vi "TLB Native Dynamic Events ver 0.27.vi"() -> ()   [LabVIEW 2018]
uses:
  TLB Type Definitions/Intruction Type Definitions.ctl
  TLB Type Definitions/State Type Definitions, for 0.26g versions and later 3.ctl
  <vilib>/Studica/Studica Toolkit/NavX/TypeDefs/Flags/Z900_navX_Flags_OpStatusTypeDef.ctl
  <vilib>/Studica/Studica Toolkit/NavX/TypeDefs/Flags/Z900_navX_Flags_CalibrationStatusTypeDef.ctl
  TLB Type Definitions/Vision cluster.ctl
  TLB Type Definitions/PING CLUSTER.ctl
  TLB Type Definitions/Encoder cluster.ctl
  TLB Type Definitions/Stepper cluster.ctl
  TLB Type Definitions/Yaw Cluster.ctl
  TLB Type Definitions/IR Sensor Type Def.ctl
  TLB Type Definitions/Line Sensor Cluster.ctl
  TLB Type Definitions/Time cluster.ctl
  TLB Type Definitions/Box Colour Detection Cluster (0.26d and above).ctl
  Underlying VI's/FGV's/Box FGV/Box Colour FGV Colours.ctl
  <vilib>/Studica/Studica Toolkit/Background/DIO Channel.ctl
  TLB Type Definitions/Y Stepper cluster.ctl
  TLB Type Definitions/Motor Speed Cluster.ctl
  <vilib>/Studica/Studica Toolkit/Background/PWM Channel.ctl
  Underlying VI's/NavX VI/navX type def.ctl
  <vilib>/Studica/Studica Toolkit/Background/I2C Channel.ctl
  Underlying VI's/I2C Master VI/Arduino_Interfacing.ctl
  Labview Training Phase 2/Enum Controls/States for Action Engine.ctl
  Underlying VI's/Motor Control VI with PID/MOTOR CONTROL WITH PID AE DATA MODE TYPE DEF.ctl
  Underlying VI's/Motor Control VI with PID/MOTOR CONTROL WITH PID AE DIRECTION TYPE DEF.ctl
  Experimental VI's/Archived VI's/MOTOR CONTROL NO PID Type Def.ctl
  <vilib>/myRIO/Common/Instrument Driver Framework/myRIO v1.0/AI/typedefs/AI Channels List.ctl
  <vilib>/myRIO/Common/Instrument Driver Framework/myRIO v1.0/AI/typedefs/AI Channels Enum.ctl
  Underlying VI's/Line Sensor AE/Line Sensor AE Type Def.ctl
  Underlying VI's/I2C Master VI/I2C MASTER Type Def.ctl
  Underlying VI's/Elasped Timer/Elapsed timer control.ctl
  Underlying VI's/IMAQ Create Reference AE/IMAQ Reference AE.ctl
  Underlying VI's/FGV's/Box FGV/Box Colour FGV States.ctl
  Underlying VI's/I2C Master VI/I2C_MASTER_WRITE_NEW Type Def.ctl
  Underlying VI's/FGV's/Servo State FGV/Servo States FGV Enum.ctl
  Underlying VI's/Modified webcam FGV/Webcam AE.ctl
  <vilib>/userdefined/High Color/IMAQdx.ctl
  <vilib>/Studica/Studica Toolkit/NavX/NavX.lvlib
  <vilib>/NI_Real-Time Target Support.lvlib
panel:
  out "Distance to move":dbl
  out "Same colour?":bool
  out "Box Colour Detection":T1
  out "Errors detected":bool
  out "Robot ready":bool
  out "Time cluster":T3
  out "Table IR obstruct":bool
  out "Front IR obstruct":bool
  out "CPU 1 Usage":dbl
  out "CPU 0 Usage":dbl
  out "Line sensors":T4
  out "IR Sensors":T5
  out "NAVX Values":T6
  out "Stepper position values":T7
  out "Encoder values":T8
  out "Ultrasonic sensors":T9
  out "Selected Task":T10=enum."Start Task 9"
  out "Object recognition mode":enum16{"Ball", "Soap", "Gel", "Pipe", "None"}(ring)
  out "Image Processing Error":errorcluster
  out "Object Detection":T11
  out "Status":T14 {"OP Status" items=["INITIALIZING", "SELFTEST_IN_PROGRESS", "ERROR", "IMU_AUTOCAL_IN_PROGRESS", "NORMAL"]; "Calibration Status" items=["IMU_CAL_STATE_MASK"=3, "IMU_CAL_STATE_INPROGRESS"=0, "IMU_CAL_STATE_ACCUMULATE"=1, "IMU_CAL_STATE_COMPLETE"=2]}
  out "General Errors":errorcluster
  in  "Red LED":bool
  out "Front Ultrasonic obstruct":bool
  out "Speed & distance":T15
  out "Task selection":u8
  out "NavX Readings":T16
  out "Arduino Data":T17
  out "TASK ENABLE":bool
  out "Rising Edge":bool
  in  "Green LED":bool
  out "State Logic":T18=enum."Startup"
  out "elements":T10[](array[typedef])
  in  "STOP TASK":bool
  in  "OK Button":bool
  in  "STOP":bool
  out "Queue Errors":errorcluster
  out "Action Queue Items":i32
  out "State Logic Queue Items":i32
  out "Action Queues items":string[](array[string])=["Hardware reset", "Software reset", ""]
  out "Action State":string
  # "VISION"
  # "TLB FRAMEWORK STATUS"
  # "System Health Status Update"
  # "Test Programme written by Calvin Loke    Dated: 28 Aug 2019\nTest Programme revised by Dr Alex See   Dated 30 Aug 2019\n\nRevision date: 20/03/2020\nProgramme version:   TLB Native Dynamic Events ver 0.19a"
  # "0: Task 1\n1: Task 2\n2: Task 3\n3: Task 4\n4: Task 5\n5: Task 6\n6: Task 7\n7: Task 8 Ball\n8: Task 8 Soap\n9: Task 8 Gel\n10: Task 8 Pipe\n11: Task 9 Blue\n12: Task 9 Black\n13: Task 9 Green\n14: Task 9 Red\n15: Task 9 Yellow"
  # "Ball: Right\nSoap: Left\nGel: Reverse\nPipe: Forward"
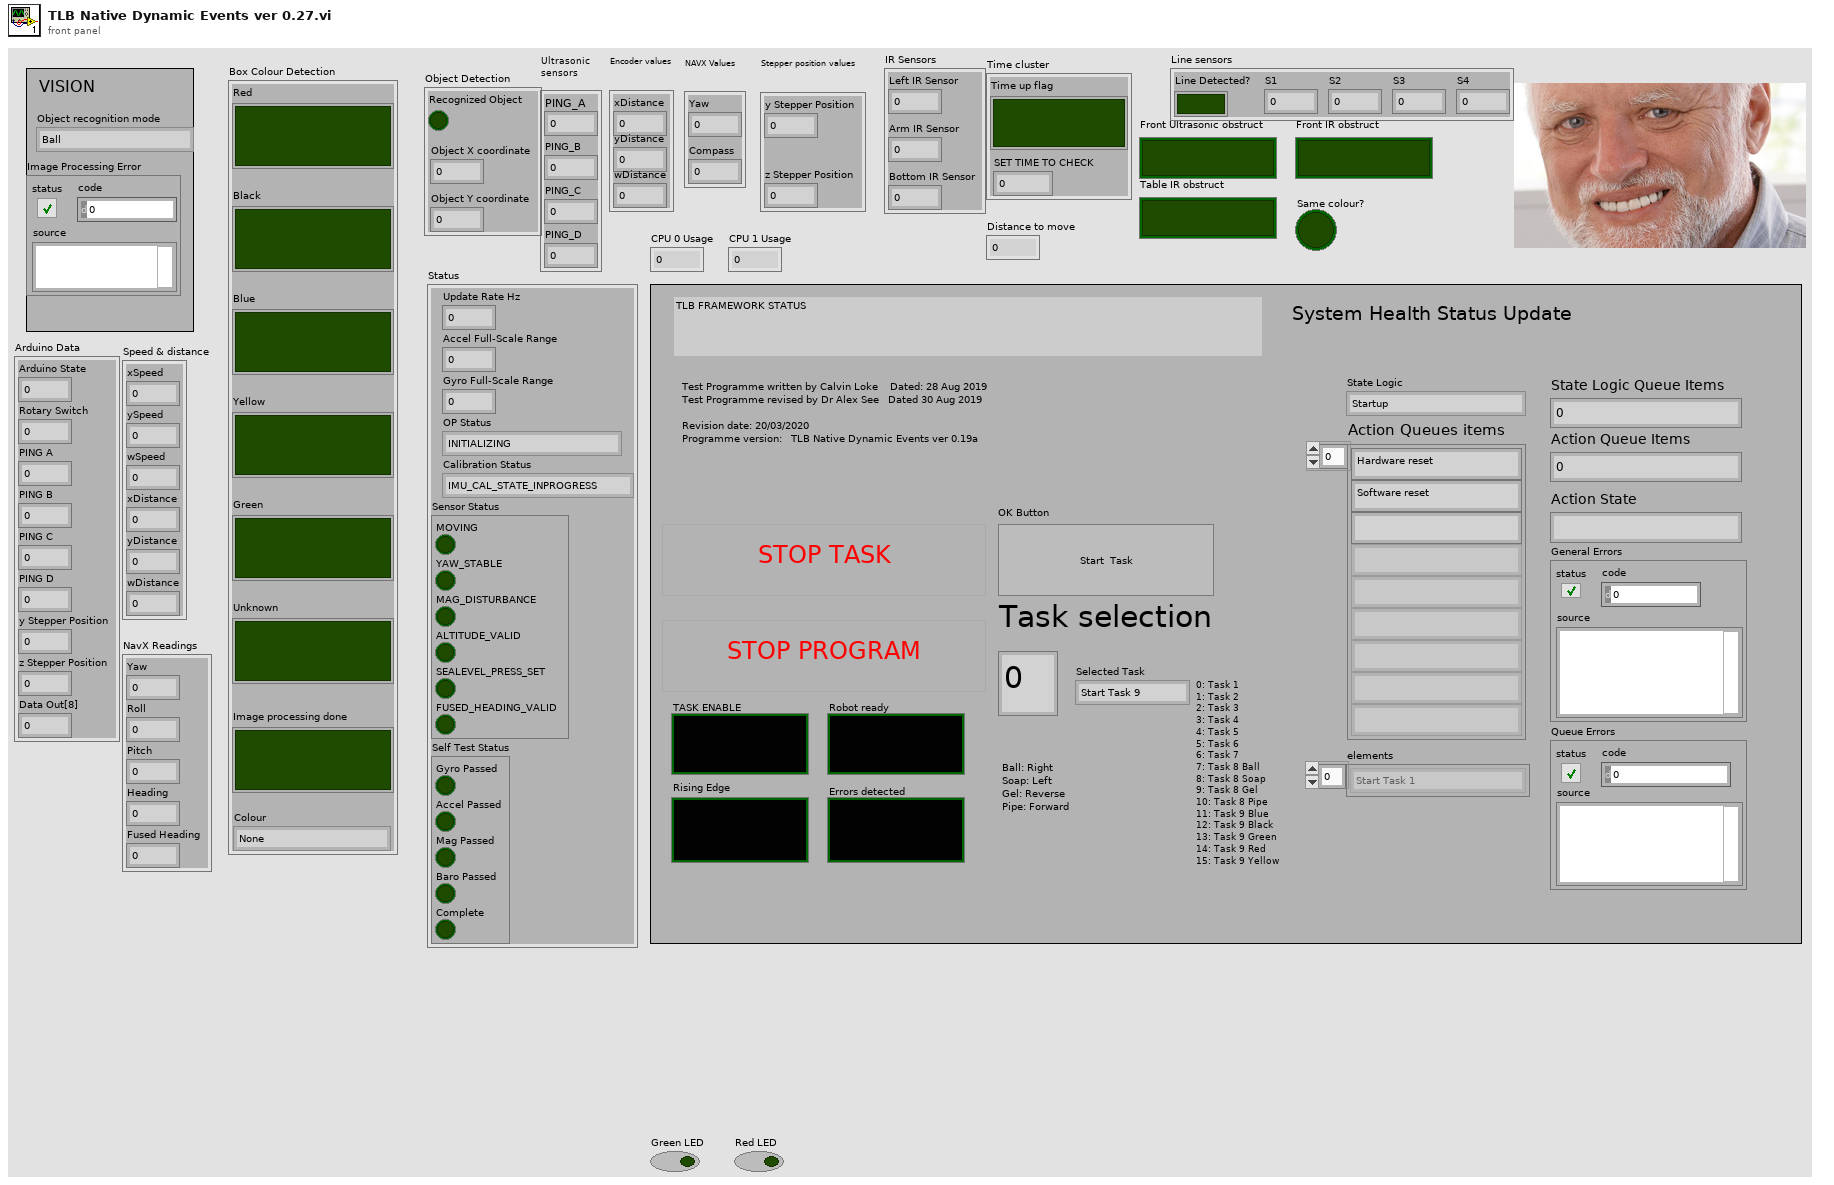
[diagram p1: front panel]
types:
  T1 = typedef "Box Colour Detection Cluster (0.26d and above).ctl" = cluster{"Red":bool, "Black":bool, "Blue":bool, "Yellow":bool, "Green":bool, "Unknown":bool, "Image processing done":bool, "Colour":T2}
  T2 = typedef "Box Colour FGV Colours.ctl" = enum16{"None", "Black", "Blue", "Green", "Red", "Yellow"}
  T3 = typedef "Time cluster.ctl" = cluster{"Time up flag":bool, "SET TIME TO CHECK":dbl}
  T4 = typedef "Line Sensor Cluster.ctl" = cluster{"Line Detected?":bool, "S1":dbl, "S2":dbl, "S3":dbl, "S4":dbl}
  T5 = typedef "IR Sensor Type Def.ctl" = cluster{"Left IR Sensor":dbl, "Arm IR Sensor":dbl, "Bottom IR Sensor":dbl}
  T6 = typedef "Yaw Cluster.ctl" = cluster{"Yaw":dbl, "Compass":dbl}
  T7 = typedef "Stepper cluster.ctl" = cluster{"y Stepper Position":u8, "z Stepper Position":u8}
  T8 = typedef "Encoder cluster.ctl" = cluster{"xDistance":dbl, "yDistance":dbl, "wDistance":dbl}
  T9 = typedef "PING CLUSTER.ctl" = cluster{"PING_A":u8, "PING_B":u8, "PING_C":u8, "PING_D":u8}
  T10 = typedef "Intruction Type Definitions.ctl" = enum16{"None", "Start Task 1", "Start Task 2", "Start Task 3", "Start Task 4", "Start Task 5", "Start Task 6", "Start Task 7", "Start Task 8 - BALL", "Start Task 8 - Gel", "Start Task 8 - Pipe", "Start Task 8 - Soap", "Start Task 9", "Start Task A", "Start Task B", "Exit"}
  T11 = typedef "Vision cluster.ctl" = cluster{"Recognized Object":bool, "Object X coordinate":dbl, "Object Y coordinate":dbl}
  T12 = typedef "NavX.lvlib/Z900_navX_Flags_OpStatusTypeDef.ctl" = u8
  T13 = typedef "NavX.lvlib/Z900_navX_Flags_CalibrationStatusTypeDef.ctl" = u8
  T14 = cluster{"Update Rate Hz":u8, "Accel Full-Scale Range":u8, "Gyro Full-Scale Range":u16, "OP Status":T12, "Calibration Status":T13, "Sensor Status":cluster{"MOVING":bool, "YAW_STABLE":bool, "MAG_DISTURBANCE":bool, "ALTITUDE_VALID":bool, "SEALEVEL_PRESS_SET":bool, "FUSED_HEADING_VALID":bool}, "Self Test Status":cluster{"Gyro Passed":bool, "Accel Passed":bool, "Mag Passed":bool, "Baro Passed":bool, "Complete":bool}}
  T15 = cluster{"xSpeed":dbl, "ySpeed":dbl, "wSpeed":dbl, "xDistance":dbl, "yDistance":dbl, "wDistance":dbl}
  T16 = cluster{"Yaw":dbl, "Roll":dbl, "Pitch":dbl, "Heading":dbl, "Fused Heading":dbl}
  T17 = cluster{"Arduino State":u8, "Rotary Switch":u8, "PING A":u8, "PING B":u8, "PING C":u8, "PING D":u8, "y Stepper Position":u8, "z Stepper Position":u8, "Data Out[8]":u8}
  T18 = typedef "State Type Definitions, for 0.26g versions and later 3.ctl" = enum16{"None", "Startup", "Move to Angle", "True Stop", "Idle", "Shutdown", "Task 1A", "Task 1B", "Task 2:Raise Arm", "Task 2:Sensor Mode", "Task 2:Reverse Mode", "Task 3", "Task 4_A", "Task 4_B", "Task 4_C", "Task 4_D", "Task 5A: RAISING ARM", "Task 5B: STILL WAITING", "Task 5C: GOING DOWN", "Task 5D: GRAB", "Task 5E: GOING UP", "Task 5F: ARM GRAB HEIGHT", "Task 5G: CLOSE CLAW", "Task 5H: RAISE ARM", "Task 6A: RAISE ARM", "Task 6B: CAM BURST", "Task 6C: PROCESS IMAGE", "Task 6D: BALL BUSTER", "Task 6E: STILL WAITING", "Task 6F: CAM BURST 2", "Task 6G: PROCESS IMAGE 2", "Task 6H: SKADI SOAPS", "Task 6I: STILL WAITING 2", "Task 6J: CAM BURST 3", "Task 6K: PROCESS IMAGE 3", "Task 6L: JAM IT IN", "Task 6M: STILL WAITING 3", "Task 6N: CAM BURST 4", "Task 6O: PROCESS IMAGE 4", "Task 6P: PIPE BOMB", "Task 7", "Task 8A: RAISE ARM", "Task 8B: MOVE TO BOX", "Task 8C: CAM BURST", "Task 8D: PROCESS IMAGE", "Task 8E: ROBOT ADJUST", "Task 8F: CAM BURST 2", "Task 8G: PROCESS IMAGE 2", "Task 8H: ARM ADJUST", "Task 8I: ARM GRAB HEIGHT", "Task 8J: CLOSE CLAW", "Task 8K: RAISE MY SWORD", "Task 8I: STILL WAITING", "Task 8L: Return to position", "Task 9A: Raise Arm", "Task 9B: Rotate to Angle", "Task 9C: Detect Box", "Task 9D: MOVE FORWARD", "Task 9E: MOVE LEFT", "Task 9E2: MOVE RIGHT", "Task 9F: SCAN BOX", "Task 9G: MOVE RIGHT", "Task 9H: SCAN BOX 2", "Task 9I: ROTATE 90 CW", "Task 9J: FORWARD", "Task 9K: RAM WALL", "Task 9L: MOVE RIGHT", "Task 9M: SCAN BOX 3", "Task 9N: MOVE RIGHT", "Task 9O: SCAN BOX 4", "Task A1: RAISE ARM", "Task A2: ROTATE TO ANGLE", "Task A3: MOVE TO BL BOX", "Task A4: MOVE FORWARD", "Task A5: ROTATE CW 90"}
  T19 = typedef "PWM Channel.ctl" = enum16{"Not Connected", "A/PWM0", "A/PWM1", "A/PWM2", "A/PWM3", "A/PWM4", "B/PWM0", "B/PWM1", "B/PWM2", "B/PWM3", "B/PWM4", "C/PWM0", "C/PWM1"}
  T20 = typedef "Motor Speed Cluster.ctl" = cluster{"ySpeed":dbl, "xSpeed":dbl, "wSpeed":dbl}
  T21 = typedef "Y Stepper cluster.ctl" = cluster{"yStepper desired":u8}
  T22 = typedef "DIO Channel.ctl" = enum16{"Not Connected", "A/DIO1", "A/DIO2", "A/DIO3", "A/DIO4", "A/DIO5", "A/DIO6", "A/DIO7", "A/DIO13", "B/DIO1", "B/DIO2", "B/DIO3", "B/DIO4", "B/DIO5", "B/DIO6", "B/DIO7", "B/DIO13", "C/DIO0", "C/DIO1", "C/DIO2", "C/DIO3", "C/DIO4", "C/DIO5", "C/DIO6", "C/DIO7"}
  T23 = cluster{"PWM Channel":T19, "FPGA VI Reference Out":refnum<k20>}
  T24 = cluster{"DIO Channel":T22, "FPGA VI Reference Out":refnum<k20>}
  T25 = typedef "States for Action Engine.ctl" = enum16{"Initialize", "Write", "Read"}
  T26 = typedef "NI_Real-Time Target Support.lvlib/RT CPU Load.ctl" = cluster{"Total (%)":dbl, "Time Critical (%)":dbl, "Timed Structures (%)":dbl, "High (%)":dbl, "Above Normal (%)":dbl, "Normal (%)":dbl, "Background (%)":dbl, "Idle (%)":dbl, "ISR (%)":dbl}
  T27 = cluster{"CPU loads[0]":T26, "CPU loads[1]":T26, "CPU loads[2]":T26, "CPU loads[3]":T26, "CPU loads[4]":T26, "CPU loads[5]":T26, "CPU loads[6]":T26, "CPU loads[7]":T26, "CPU loads[8]":T26}
  T28 = typedef "navX type def.ctl" = enum16{"Get i2C reference", "Read Values", "Zero Yaw"}
  T29 = typedef "Arduino_Interfacing.ctl" = enum16{"Initialize", "Write to Arduino", "Read From Arduino"}
  T30 = typedef "I2C Channel.ctl" = enum16{"Not Connected", "A", "B"}
  T31 = cluster{"I2C Ref Out":cluster{"I2C Channel":T30, "FPGA VI Reference Out":refnum<k20>}, "Connected":bool, "Slave Address (7-bit)":u8, "Registry":u8[]}
  T32 = typedef "Box Colour FGV States.ctl" = enum16{"Initialize", "Read", "Write"}
  T33 = typedef "MOTOR CONTROL WITH PID AE DIRECTION TYPE DEF.ctl" = enum16{"y-axis movement", "x-axis movement", "rotation", "stop", "reset encoders"}
  T34 = typedef "MOTOR CONTROL WITH PID AE DATA MODE TYPE DEF.ctl" = enum16{"Init AE", "Write to AE", "Read from AE"}
  T35 = typedef "Line Sensor AE Type Def.ctl" = enum16{"INIT AE", "READ FROM LINE SENSORS"}
  T36 = typedef "IMAQ Reference AE.ctl" = enum16{"Initialize AE", "Get IMAQ Reference", "Dispose Processing Buffer"}
  T37 = typedef "Elapsed timer control.ctl" = enum16{"Start", "Pause", "Initialize"}
  T38 = typedef "I2C_MASTER_WRITE_NEW Type Def.ctl" = enum16{"Ultrasonic sensors", "Stepper origin", "zStepper 13.3k", "zStepper 13k", "zStepper 12k", "zStepper 11k", "zStepper 10k", "zStepper 9k", "zStepper 8k", "zStepper 7k", "zStepper 6k", "zStepper 5k", "zStepper 4k", "zStepper 3k", "zStepper 2k", "zStepper 1k", "zStepper 900", "zStepper 800", "zStepper 700", "zStepper 600", "zStepper 500", "zStepper 400", "zStepper 300", "zStepper 200", "zStepper 100", "zStepper 0", "yStepper control", "Open Claw", "Close Claw", "Soft Reset"}
  T39 = typedef "Servo States FGV Enum.ctl" = enum16{"Open Claw", "Close claw"}
  T40 = typedef "Webcam AE.ctl" = enum16{"Initialize Camera", "Open Camera", "Continuous Acquisition", "Close Camera", "Retrieve Image", "Dispose Camera Image Buffer"}
  T41 = typedef "IMAQdx.ctl" = refnum<k21>
  T42 = typedef "MOTOR CONTROL NO PID Type Def.ctl" = enum16{"Init", "Front Back", "Left Right", "Rotate", "Stop", "Latch"}
  T43 = typedef "AI Channels List.ctl" = T44[]
  T44 = typedef "AI Channels Enum.ctl" = enum16{"Not Connected", "AudioIn/Left", "AudioIn/Right", "C/AI0", "C/AI1", "A/AI0", "A/AI1", "A/AI2", "A/AI3", "A/AI4", "A/AI5", "A/AI6", "A/AI7", "B/AI0", "B/AI1", "B/AI2", "B/AI3", "B/AI4", "B/AI5", "B/AI6", "B/AI7", "AI/AI0", "AI/AI1", "AI/AI2", "AI/AI3", "A/AI0 (DIFF)", "A/AI1 (DIFF)", "A/AI2 (DIFF)", "A/AI3 (DIFF)", "B/AI0 (DIFF)", "B/AI1 (DIFF)", "B/AI2 (DIFF)", "B/AI3 (DIFF)"}
  T45 = cluster{"S1":dbl, "S2":dbl, "S3":dbl, "S4":dbl, "Array[4]":dbl, "Array[5]":dbl, "Array[6]":dbl, "Array[7]":dbl, "Array[8]":dbl}
  T46 = typedef "I2C MASTER Type Def.ctl" = enum16{"Last State", "Mode 0", "Mode 1", "Mode 2", "Mode 3", "Mode 4", "Mode 5", "Mode 6", "Mode 7", "Mode 8", "Mode 9", "Mode 10"}
  T47 = typedef "IMAQ Image.ctl" = refnum<image>
  T48 = cluster{"Number of Matches":i32, "Object detected?":bool}
  T49 = cluster{"Red":bool, "Black":bool, "Blue":bool, "Yellow":bool, "Green":bool, "No recognizable coolour":bool}
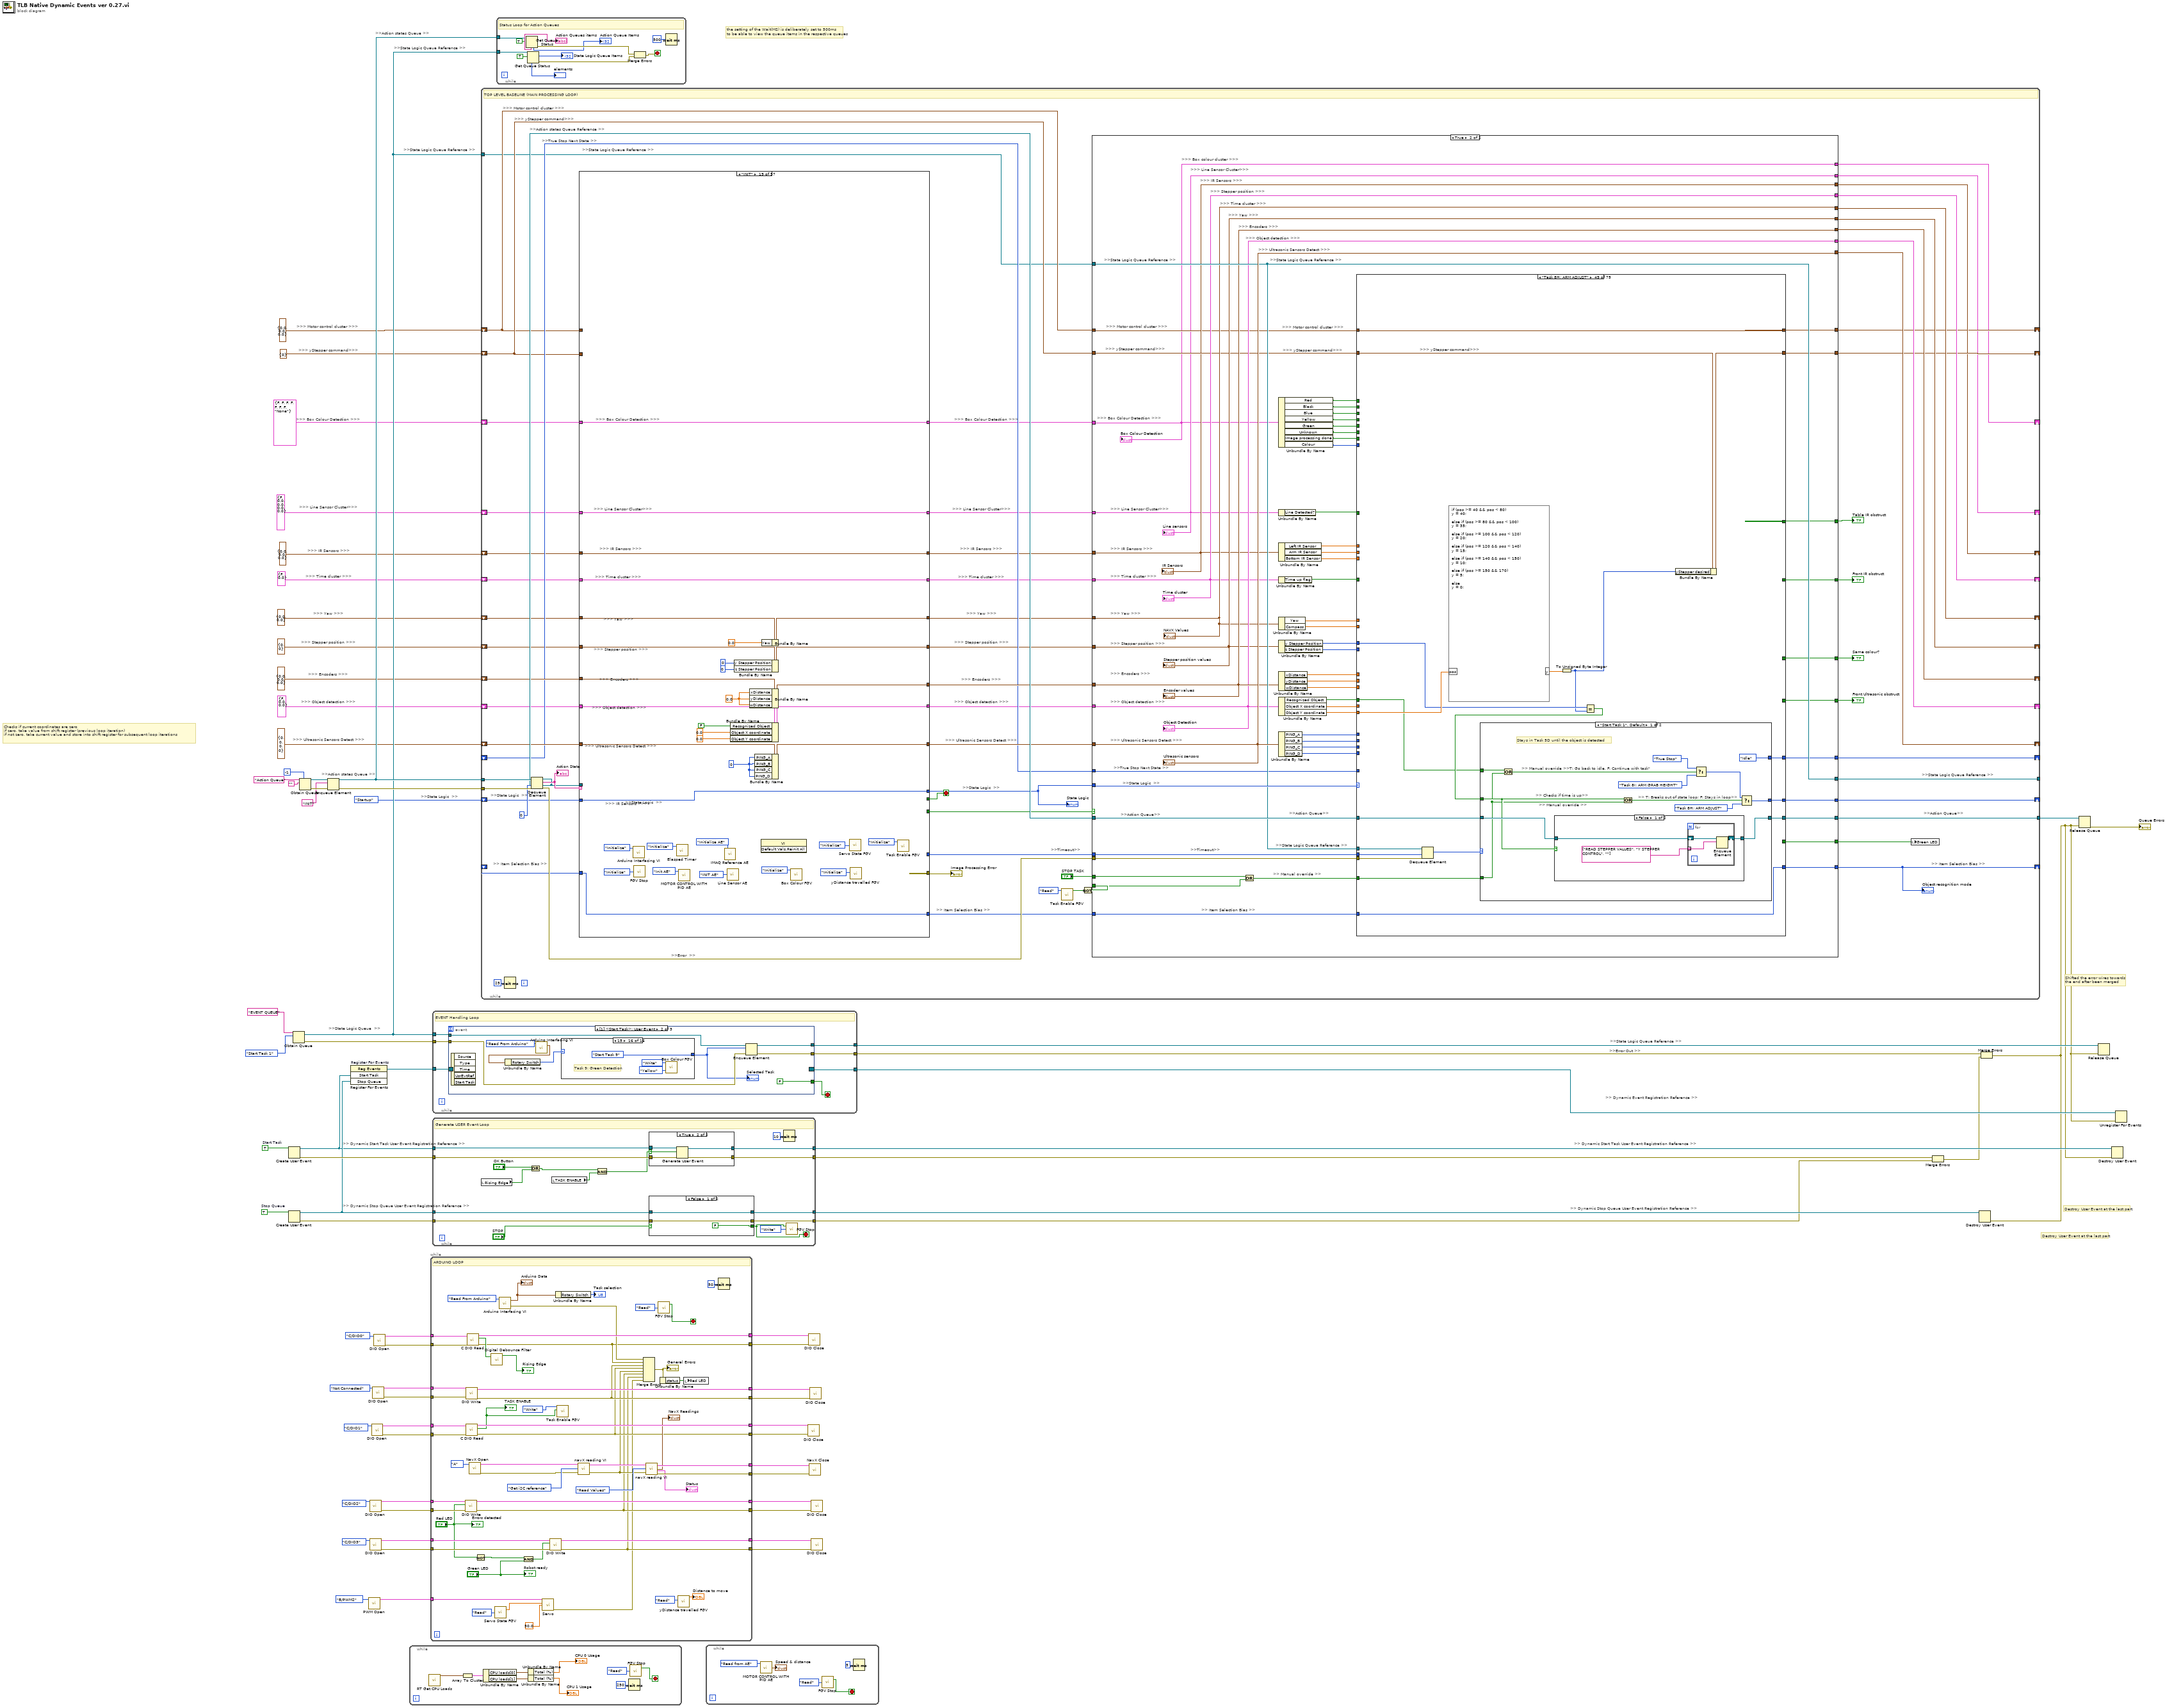
[diagram p0: block diagram]
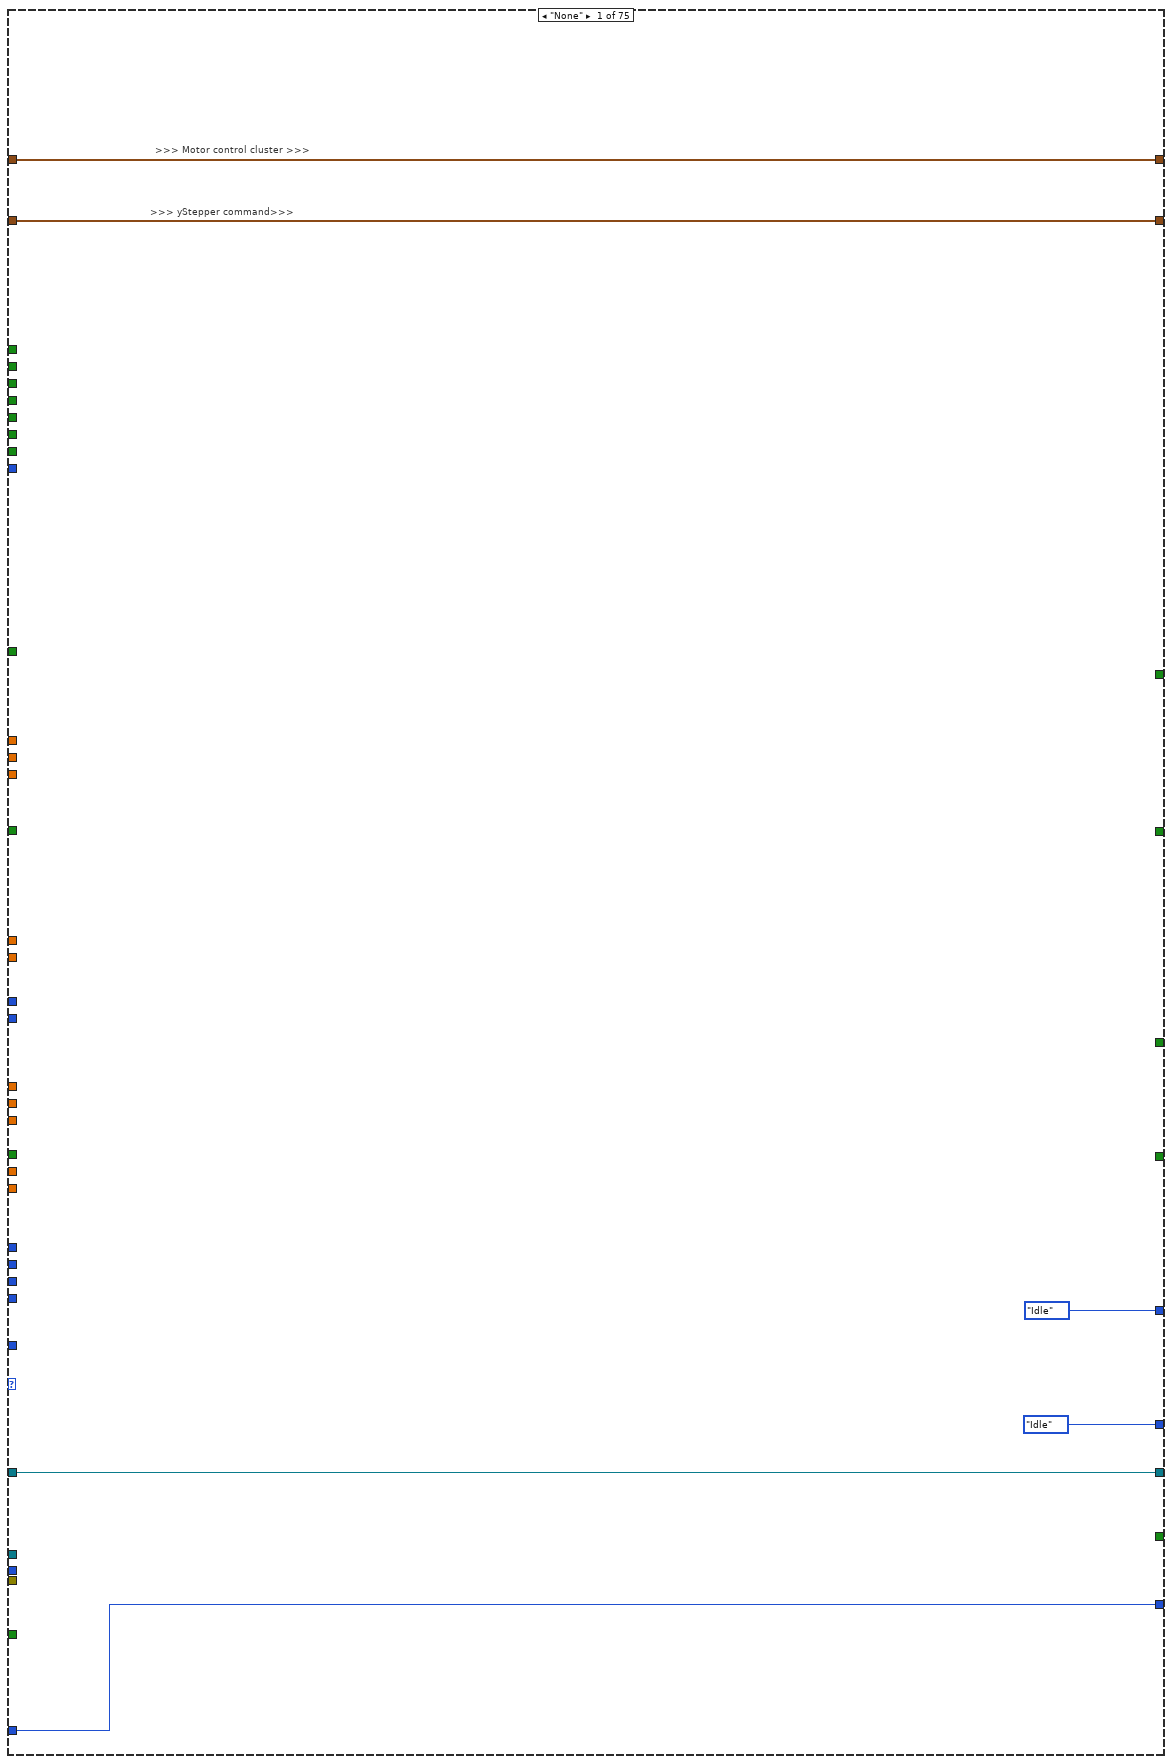
[diagram p3: hidden frame]
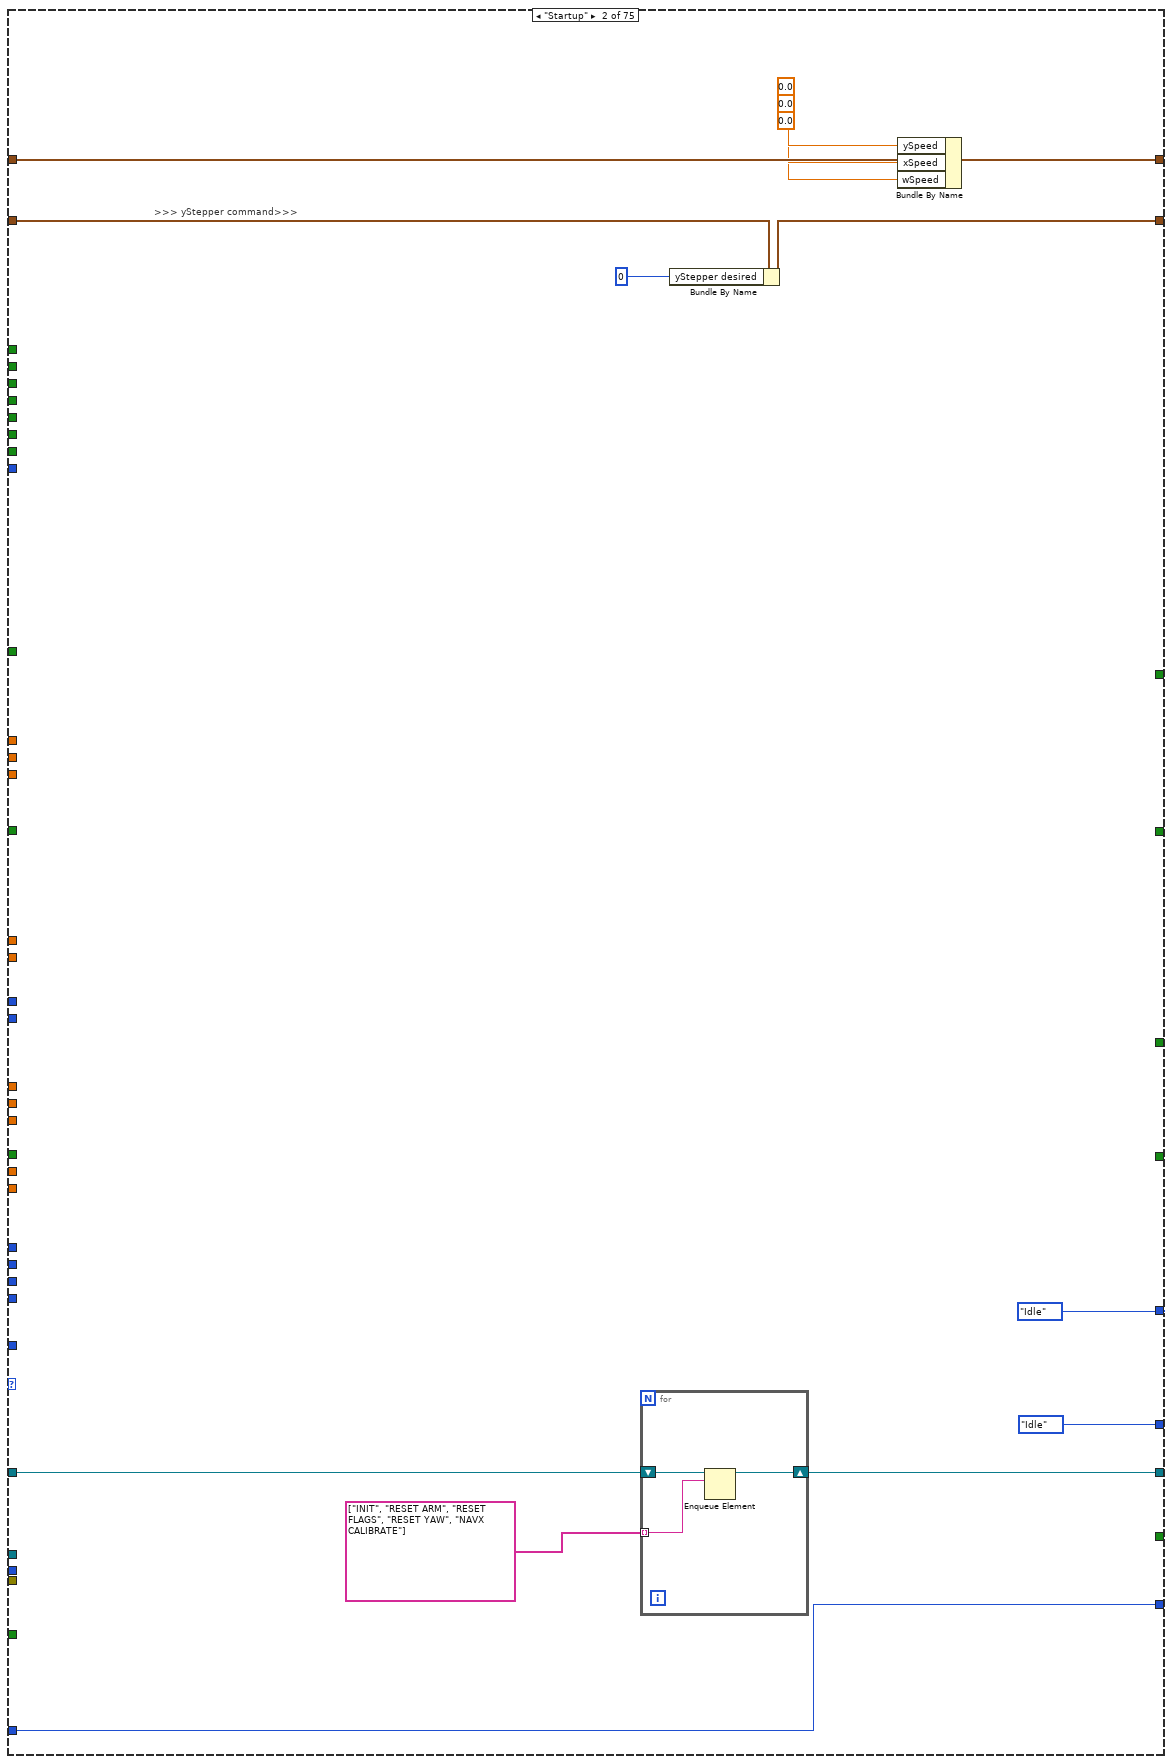
[diagram p4: hidden frame]
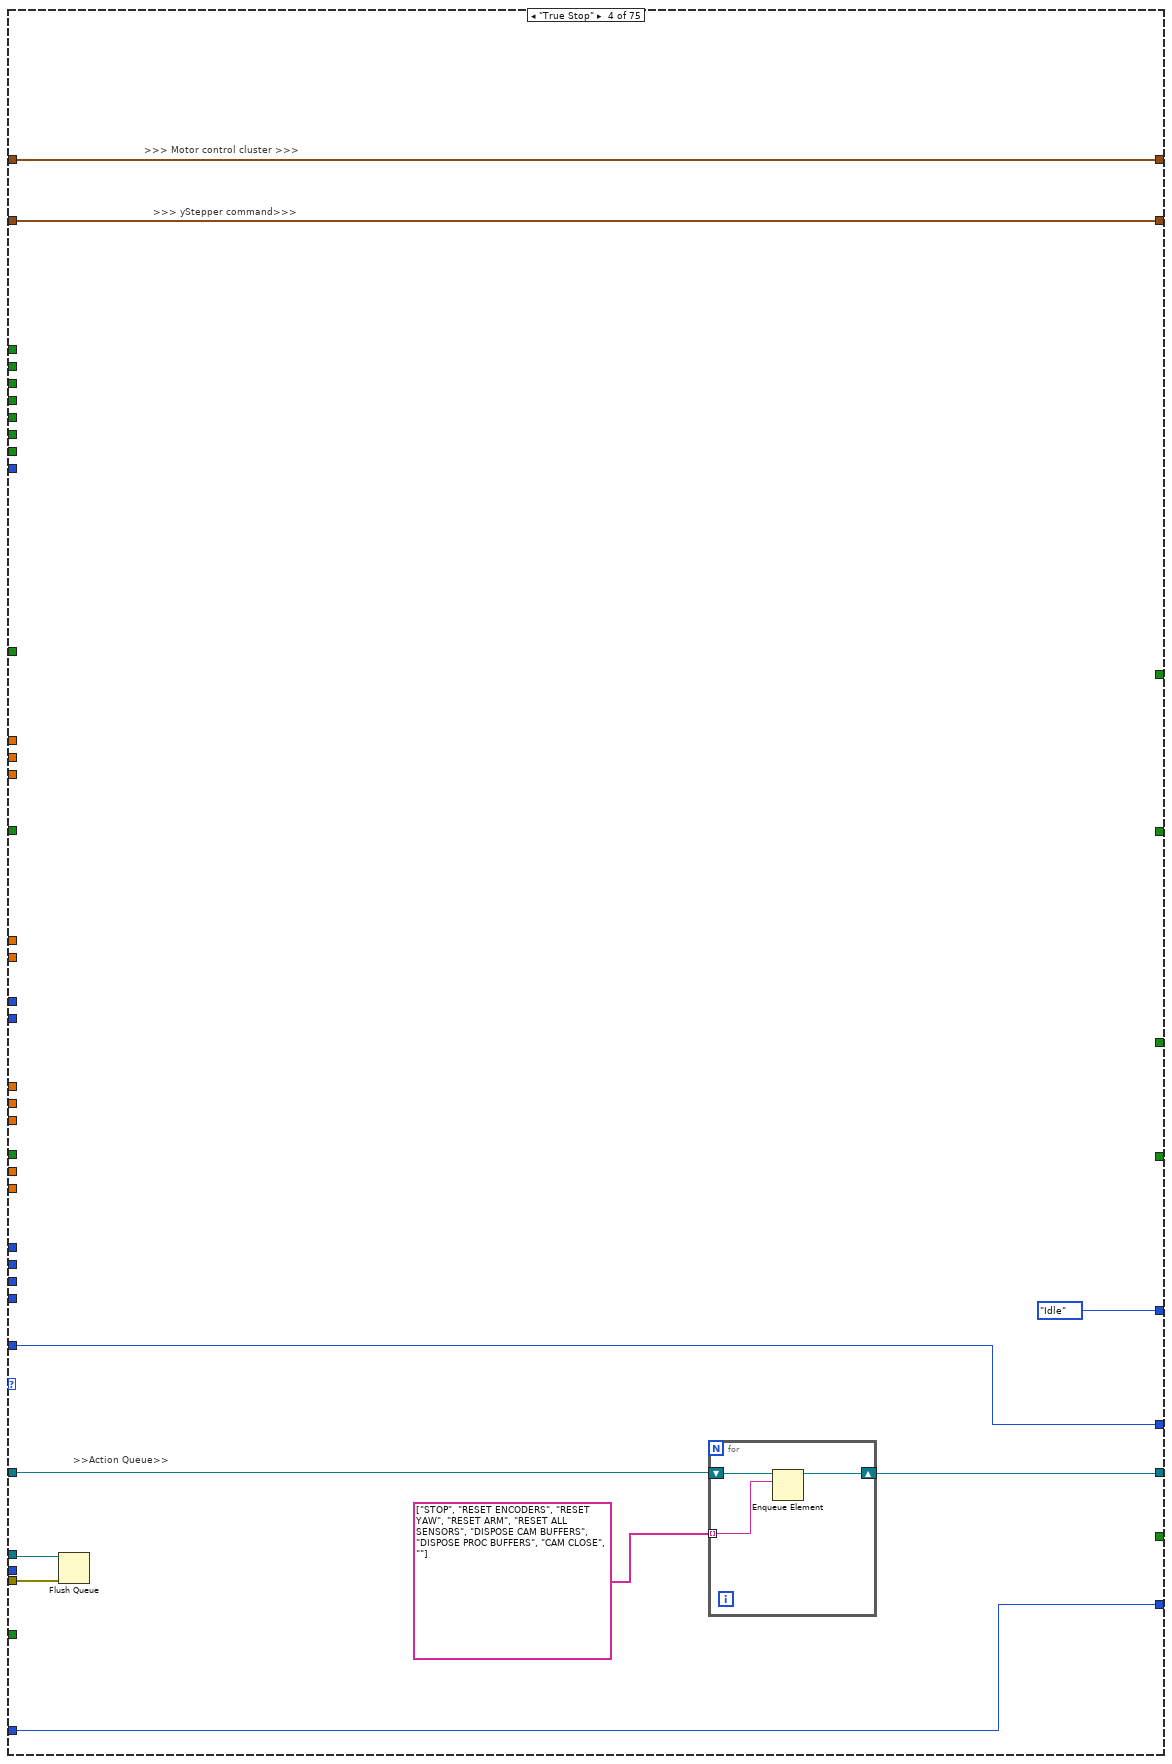
[diagram p6: hidden frame]
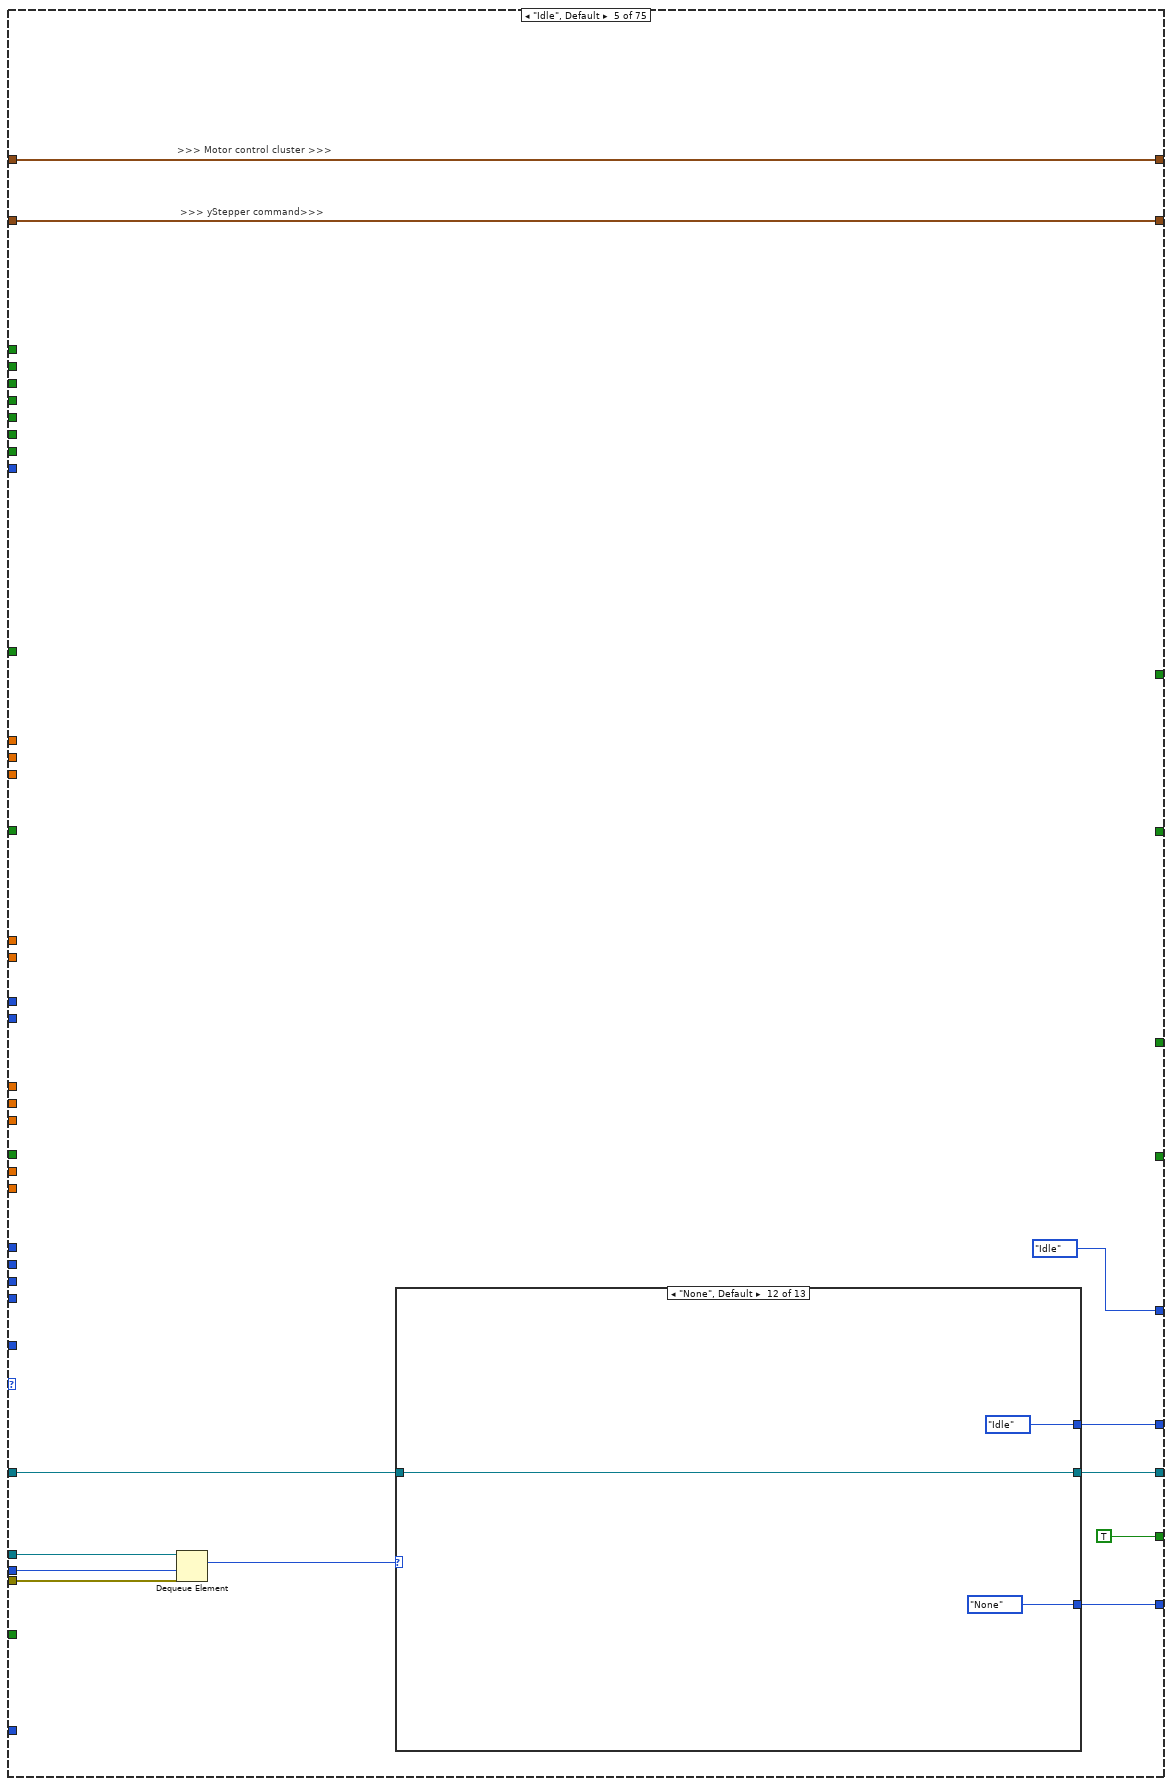
[diagram p7: hidden frame]
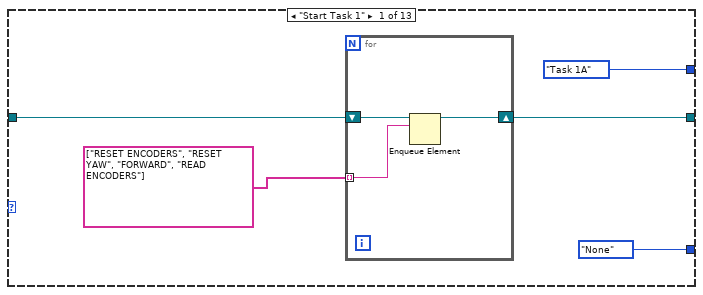
[diagram p8: hidden frame]
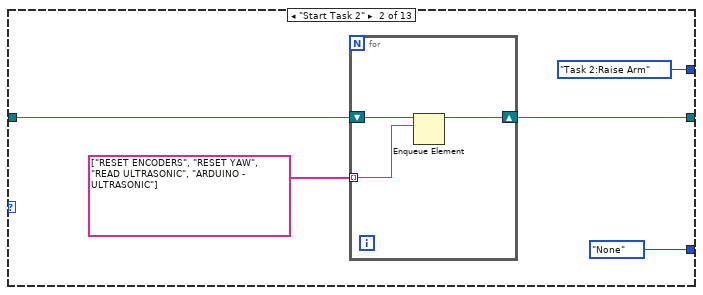
[diagram p9: hidden frame]
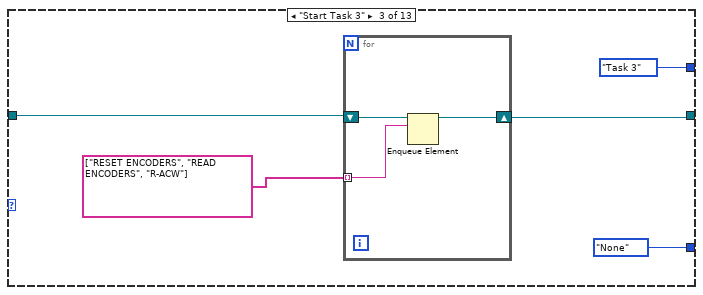
[diagram p10: hidden frame]
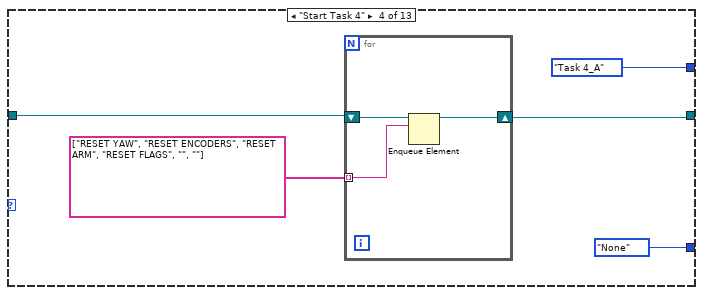
[diagram p11: hidden frame]
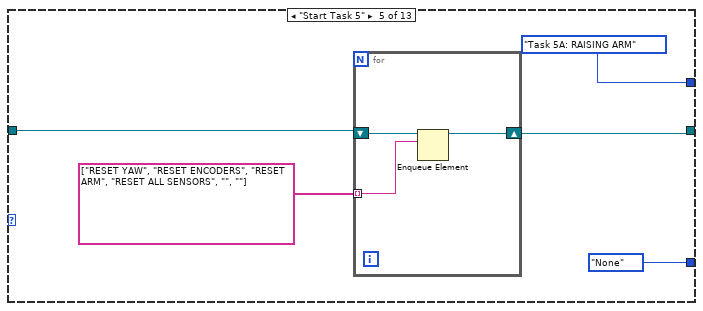
[diagram p12: hidden frame]
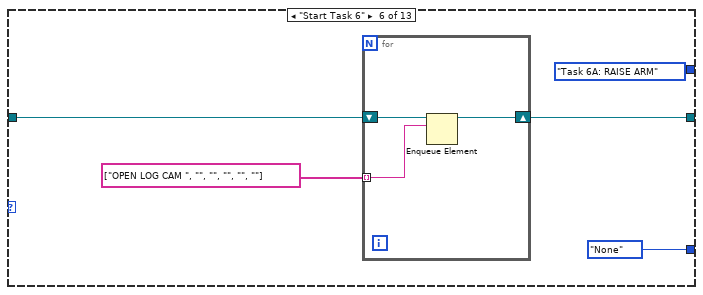
[diagram p13: hidden frame]
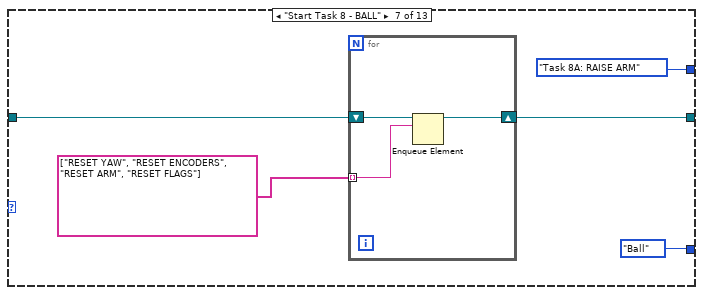
[diagram p14: hidden frame]
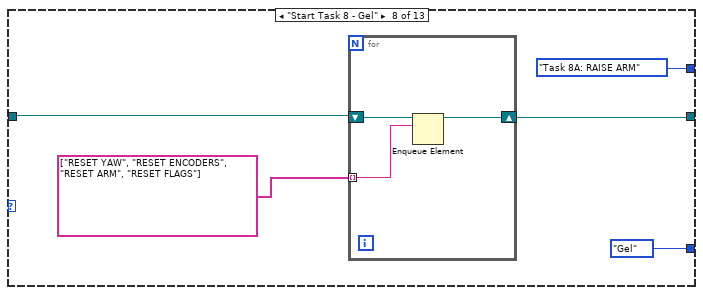
[diagram p15: hidden frame]
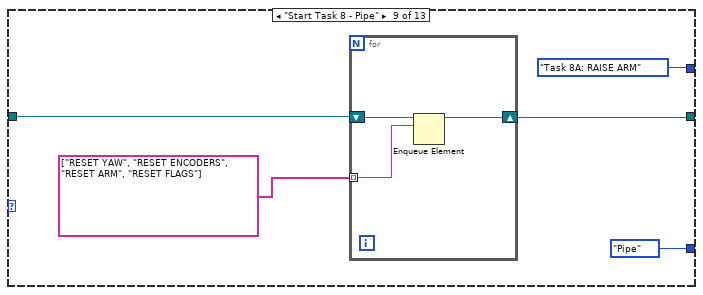
[diagram p16: hidden frame]
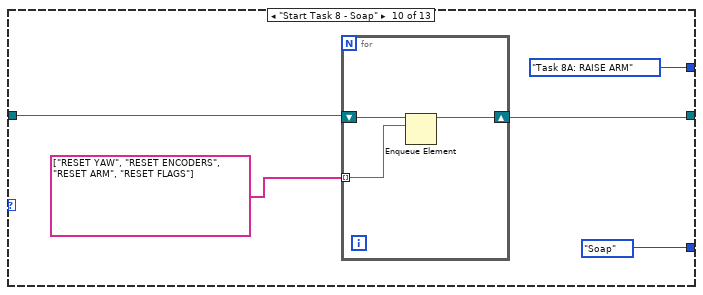
[diagram p17: hidden frame]
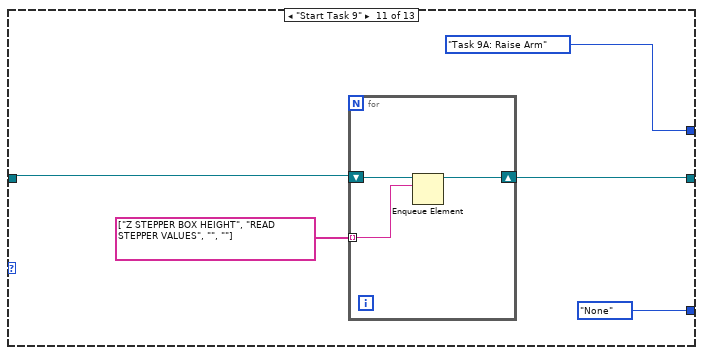
[diagram p18: hidden frame]
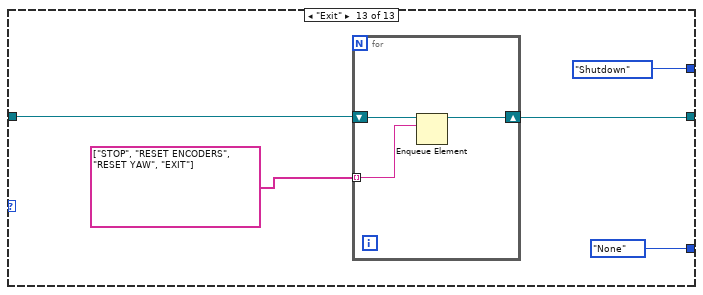
[diagram p19: hidden frame]
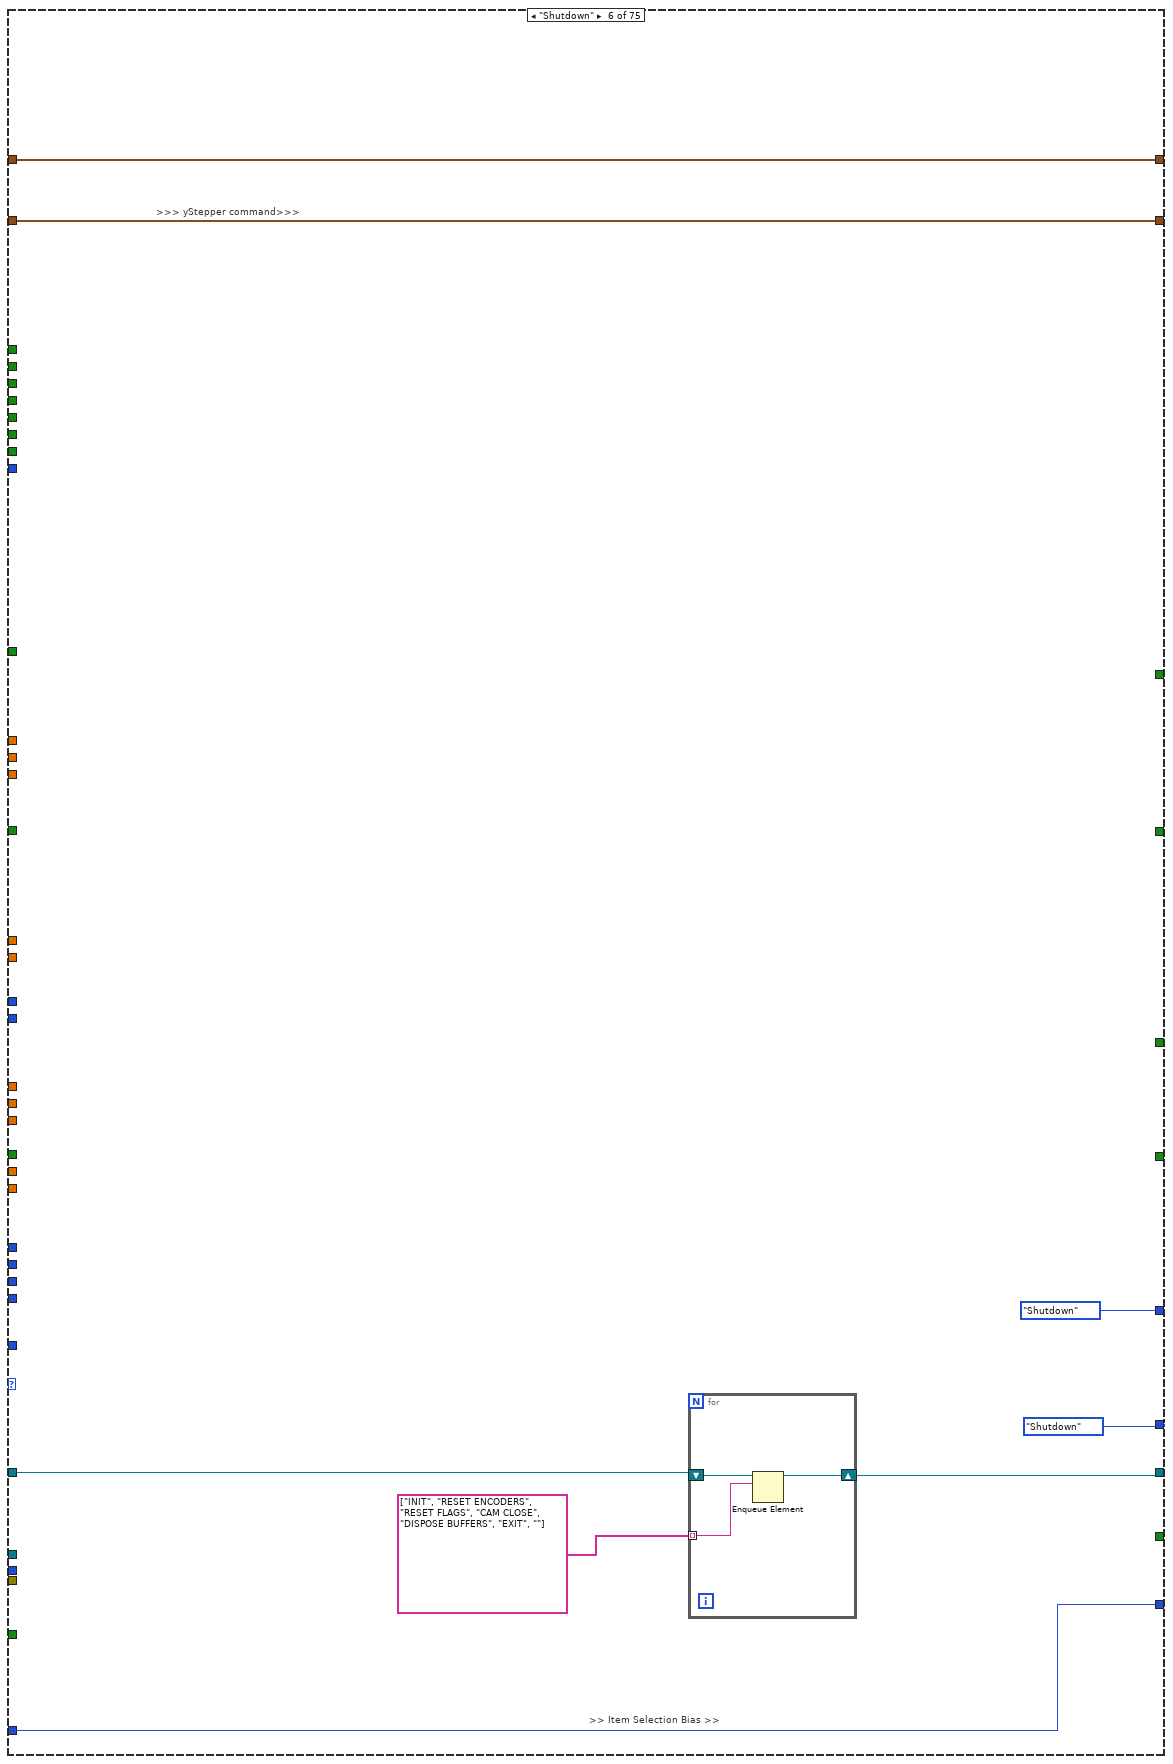
[diagram p20: hidden frame]
diagram:
  w71 = TRUE  # Stop Queue
  w70 = TRUE  # Start Task
  # ">>State Logic Queue Reference >>"
  # ">>Action states Queue >>"
  # ">>> Box Colour Detection >>>"
  # ">>State Logic Queue Reference >>"
  # ">>State Logic  >>"
  # ">>> Line Sensor Cluster>>>"
  # ">>> Motor control cluster >>>"
  # ">>> IR Sensors >>>"
  # "Checks if current coordinates are zero\nif zero, take value from shift register (previous loop iteration)\nif not zero, take current value and store into shift register for subsequent loop iterations"
  # ">>> yStepper command>>>"
  # ">>> Time cluster >>>"
  # ">>> Yaw >>>"
  # ">>> Stepper position >>>"
  # ">>> Encoders >>>"
  # ">>> Object detection >>>"
  # ">>> Ultrasonic Sensors Detect >>>"
  # "the setting of the Wait(MS) is deliberately set to 500ms\nto be able to view the queue items in the respective queues"
  # ">>Error Out >>"
  # ">> Dynamic Stop Queue User Event Registration Reference >>"
  # ">> Dynamic Start Task User Event Registration Reference >>"
  # ">> Dynamic Stop Queue User Event Registration Reference >>"
  # ">> Dynamic Start Task User Event Registration Reference >>"
  # ">> Dynamic Event Registration Reference >>"
  # ">>Action states Queue >>"
  # ">>State Logic Queue  >>"
  # ">>State Logic Queue Reference >>"
  # "Destroy User Event at the last part"
  # "Destroy User Event at the last part"
  # "Shifted the error wires towards\nthe end after been merged"
  n1 = Create User Event(user event datatype=w70) -> (user event=w62:refnum<user-event>, error out=w67:errorcluster)  [unwired: 1 in]
  n2 = Create User Event(user event datatype=w71) -> (user event=w63:refnum<user-event>, error out=w66:errorcluster)  [unwired: 1 in]
  n3 = Obtain Queue(name (unnamed)="EVENT QUEUE", element data type=Intruction_Type_Definitions."Start Task 1" ("Enum")) -> (queue out=w48:refnum<queue>, error out=w54:errorcluster)  [unwired: 3 in, 1 out]
  n4 = Obtain Queue(max queue size (-1, unlimited)=-1, name (unnamed)="Action Queue", element data type="") -> (queue out=w57:refnum<queue>, error out=w53:errorcluster)  [unwired: 2 in, 1 out]
  n5 = Enqueue Element(queue=w57, element="INIT", error in (no error)=w53) -> (queue out=w49:refnum<queue>, error out=w52:errorcluster)  [unwired: 1 in, 1 out]
  n6 = register-events "Register For Events"(w62, w63) -> (reference out=w61:refnum<event-registration>)  [unwired: 2 in, 1 out]
  n7 = call <vilib>:"PWM Open.vi"("PWM Channel"=PWM_Channel."B/PWM2") -> ("PWM Info Out"=w1:T23)  [unwired: 9 in, 1 out]
  n8 = call <vilib>:"DIO Open.vi"("DIO Channel"=DIO_Channel."C/DIO2") -> ("error out"=w21:errorcluster, "DIO Info Out"=w22:T24)  [unwired: 9 in]
  n9 = call <vilib>:"DIO Open.vi"("DIO Channel"=DIO_Channel."C/DIO3") -> ("error out"=w16:errorcluster, "DIO Info Out"=w17:T24)  [unwired: 9 in]
  n10 = call <vilib>:"DIO Open.vi"("DIO Channel"=DIO_Channel."C/DIO1") -> ("error out"=w26:errorcluster, "DIO Info Out"=w27:T24)  [unwired: 9 in]
  n11 = call <vilib>:"DIO Open.vi"("DIO Channel"=DIO_Channel."Not Connected") -> ("error out"=w31:errorcluster, "DIO Info Out"=w33:T24)  [unwired: 9 in]
  n12 = call <vilib>:"DIO Open.vi"("DIO Channel"=DIO_Channel."C/DIO0") -> ("error out"=w36:errorcluster, "DIO Info Out"=w39:T24)  [unwired: 9 in]
  n13 = while {
    stop <- w78 stop-if-true
    n14 = call <vilib>:"RT Get CPU Loads.vi"() -> ("CPU loads"=w77:T26[])  [unwired: 10 in, 1 out]
    n15 = Array To Cluster(array=w77) -> (cluster=w76:T27)
    n16 = Unbundle By Name(w76) -> ("CPU loads[0]"=w75:T26, "CPU loads[1]"=w74:T26)
    n17 = Unbundle By Name(w75) -> ("Total (%)"=→"CPU 0 Usage":dbl)
    n18 = Unbundle By Name(w74) -> ("Total (%)"=→"CPU 1 Usage":dbl)
    n19 = Wait (ms)(milliseconds to wait=u32 250) -> ()  [unwired: 1 out]
    n20 = call "FGV Stop.vi"("Init/Read/Write State"=States_for_Action_Engine."Read") -> ("Output node"=w78:bool)  [unwired: 2 in, 1 out]
  }
  n21 = while {
    tunnel: w39 -> [w132]
    tunnel: [w131] -> w37
    tunnel: w36 -> [w130]
    tunnel: [w102] -> w35
    tunnel: w33 -> [w127]
    tunnel: [w126] -> w32
    tunnel: w31 -> [w125]
    tunnel: [w101] -> w30
    tunnel: [w124] -> w28
    tunnel: w27 -> [w123]
    tunnel: w26 -> [w122]
    tunnel: [w100] -> w25
    tunnel: w22 -> [w117]
    tunnel: w21 -> [w116]
    tunnel: [w115] -> w20
    tunnel: [w98] -> w19
    tunnel: w17 -> [w114]
    tunnel: w16 -> [w113]
    tunnel: [w112] -> w15
    tunnel: [w97] -> w14
    tunnel: [w109] -> w11
    tunnel: [w108] -> w12
    tunnel: w1 -> [w89]
    stop <- w134 stop-if-true
    # "ARDUINO LOOP"
    n22 = call <vilib>:"DIO Write.vi"("error in (no error)"=w116, "Input"="Red LED", "DIO Info In"=w117) -> ("error out"=w98:errorcluster, "DIO Info Out"=w115:T24)  [unwired: 7 in]
    n23 = call <vilib>:"DIO Write.vi"("error in (no error)"=w125, "DIO Info In"=w127) -> ("error out"=w101:errorcluster, "DIO Info Out"=w126:T24)  [unwired: 8 in]
    n24 = call <vilib>:"C DIO Read.vi"("error in (no error)"=w122, "DIO Info In in"=w123) -> ("error out"=w100:errorcluster, "IN"=w81:bool, "DIO Info In out"=w124:T24)  [unwired: 7 in]
    "TASK ENABLE" <- w81
    n25 = call <vilib>:"C DIO Read.vi"("error in (no error)"=w130, "DIO Info In in"=w132) -> ("error out"=w102:errorcluster, "IN"=w129:bool, "DIO Info In out"=w131:T24)  [unwired: 7 in]
    n26 = call <vilib>:"NavX Open.vi"("I2C Channel"=I2C_Channel."A") -> ("error out"=w119:errorcluster, "NavX Info"=w121:T31)  [unwired: 9 in]
    n27 = Not(x="Red LED") -> (.not. x?=w92:bool)
    n28 = call "Digital Debounce Filter.vi"("Boolean input"=w129) -> ("Rising Edge"=→"Rising Edge":bool)  [unwired: 1 in, 2 out]
    n29 = call "Servo State FGV.vi"("Init/Read/Write State"=States_for_Action_Engine."Read") -> ("Output"=w85:dbl)  [unwired: 2 in, 1 out]
    n30 = call "Arduino Interfacing VI.vi"("AE Mode"=Arduino_Interfacing."Read From Arduino") -> ("error out"=w103:errorcluster, "Arduino Data"=w105:T17)  [unwired: 3 in]
    "Arduino Data" <- w105
    n31 = And(x=w92, y="Green LED") -> (x .and. y?=w94:bool)
    n32 = call <vilib>:"Servo.vi"("PWM Info In"=w89, "Position"=w85, "Frequency [Hz]"=50.0) -> ("error out"=w88:errorcluster)  [unwired: 11 in, 1 out]
    n33 = call <vilib>:"DIO Write.vi"("error in (no error)"=w113, "Input"=w94, "DIO Info In"=w114) -> ("error out"=w97:errorcluster, "DIO Info Out"=w112:T24)  [unwired: 7 in]
    n34 = Unbundle By Name(w105) -> ("Rotary Switch"=→"Task selection":u8)
    n35 = call "Task Enable FGV.vi"("Task Enable Input"=w81, "Init/Read/Write State"=States_for_Action_Engine."Write") -> ()  [unwired: 8 in, 2 out]
    n36 = call "navX reading VI.vi"("NavX Info In"=w121, "Mode"=navX_type_def."Get i2C reference", "error in (no error)"=w119) -> ("NavX Info Out"=w110:T31, "Error Out"=w99:errorcluster)  [unwired: 2 out]
    n37 = Merge Errors(w103, w102, w101, w100, w99, w98, w97, w88) -> (w95:errorcluster)
    "General Errors" <- w95
    n38 = call "navX reading VI.vi"("NavX Info In"=w110, "Mode"=navX_type_def."Read Values", "error in (no error)"=w99) -> ("NavX Info Out"=w109:T31, "NavX Readings"=→"NavX Readings":T16, "Status"=→"Status":T14, "Error Out"=w108:errorcluster)
    n39 = call "FGV Stop.vi"("Init/Read/Write State"=States_for_Action_Engine."Read") -> ("Output node"=w134:bool)  [unwired: 2 in, 1 out]
    n40 = Unbundle By Name(w95) -> ("status"=w93:bool)
    n41 = call "yDistance travelled FGV.vi"("Init/Read/Write State"=States_for_Action_Engine."Read") -> ("Output"=→"Distance to move":dbl)  [unwired: 9 in, 1 out]
    n42 = local write "Red LED"(w93) -> ()
    n43 = Wait (ms)(milliseconds to wait=u32 50) -> ()  [unwired: 1 out]
    "Robot ready" <- "Green LED"
    "Errors detected" <- "Red LED"
  }
  n44 = while {
    tunnel: w62 -> [w152]
    tunnel: w63 -> [w151]
    tunnel: [w150] -> w69
    tunnel: [w149] -> w68
    tunnel: w67 -> [w148]
    tunnel: [w147] -> w65
    tunnel: w66 -> [w146]
    tunnel: [w145] -> w64
    stop <- w143 stop-if-true
    # "Generate USER Event Loop"
    n45 = local read "Rising Edge"() -> (w140:bool)
    n46 = Or(x="OK Button", y=w140) -> (x .or. y?=w139:bool)
    n47 = local read "TASK ENABLE"() -> (w138:bool)
    n48 = And(x=w139, y=w138) -> (x .and. y?=w137:bool)
    n49 = case shown="True" w137 {
      selector: w137 -> [_ w163]
      tunnel: w152 -> [w162 w167]
      tunnel: [w162 w166] -> w149
      tunnel: w148 -> [w161 w165]
      tunnel: [w161 w164] -> w147
      frame False {
      }
      frame True {
        n50 = Generate User Event(user event=w167, event data cluster=w163, error in=w165) -> (user event out=w166:refnum<user-event>, error out=w164:errorcluster)  [unwired: 1 in]
      }
    }
    n51 = case shown="False" "STOP" {
      selector: "STOP" -> [_ w156]
      tunnel: w151 -> [w155 w160]
      tunnel: [w155 w159] -> w150
      tunnel: w146 -> [w154 w158]
      tunnel: [w154 w157] -> w145
      tunnel: [FALSE w156] -> w143
      frame False {
      }
      frame True {
        n52 = Generate User Event(user event=w160, event data cluster=w156, error in=w158) -> (user event out=w159:refnum<user-event>, error out=w157:errorcluster)  [unwired: 1 in]
      }
    }
    n53 = Wait (ms)(milliseconds to wait=u32 10) -> ()  [unwired: 1 out]
    n54 = call "FGV Stop.vi"("Init/Read/Write State"=States_for_Action_Engine."Write", "Input Node"=w143) -> ()  [unwired: 1 in, 2 out]
  }
  n55 = while {
    tunnel: w61 -> [w174]
    tunnel: [w173] -> w60
    tunnel: w48 -> [w171]
    tunnel: [w170] -> w59
    tunnel: w54 -> [w169]
    tunnel: [w168] -> w51
    stop <- w172 stop-if-true
    # "EVENT Handling Loop"
    n56 = event shown="[1] <Start Task>: User Event" {
      selector: w174 -> [_ _ _]
      dyn-events: [_ _ _] -> w173
      timeout: _ -> [_ _ _]
      tunnel: [FALSE FALSE w221] -> w172
      tunnel: w171 -> [w179 w188 w219]
      tunnel: [w178 w187 w220] -> w170
      tunnel: w169 -> [w177 w186 w218]
      tunnel: [w176 w185 w217] -> w168
      event Timeout {
        n57 = event-data() -> ()  [unwired: 1 in, 3 out]
        n58 = Enqueue Element(queue=w179, element=Intruction_Type_Definitions."Start Task 1" ("Enum"), error in (no error)=w177) -> (queue out=w178:refnum<queue>, error out=w176:errorcluster)  [unwired: 1 in, 1 out]
      }
      event User Event {
        n59 = event-data() -> ()  [unwired: 1 in, 5 out]
        n60 = call "Arduino Interfacing VI.vi"("AE Mode"=Arduino_Interfacing."Read From Arduino") -> ("Arduino Data"=w182:T17)  [unwired: 3 in, 1 out]
        n61 = Unbundle By Name(w182) -> ("Rotary Switch"=w181:u8)
        n62 = case shown="15" w181 {
          tunnel: [Intruction_Type_Definitions."Start Task 1" ("Enum") Intruction_Type_Definitions."Start Task 2" ("Enum") Intruction_Type_Definitions."Start Task 3" ("Enum") Intruction_Type_Definitions."Start Task 4" ("Enum") Intruction_Type_Definitions."Start Task 5" ("Enum") Intruction_Type_Definitions."Start Task 6" ("Enum") Intruction_Type_Definitions."Start Task 7" ("Enum") Intruction_Type_Definitions."Start Task 8 - BALL" ("Enum") Intruction_Type_Definitions."Start Task 8 - Soap" ("Enum") Intruction_Type_Definitions."Start Task 8 - Gel" ("Enum") Intruction_Type_Definitions."Start Task 8 - Pipe" ("Enum") Intruction_Type_Definitions."Start Task 9" ("Enum") Intruction_Type_Definitions."Start Task 9" ("Enum") Intruction_Type_Definitions."Start Task 9" ("Enum") Intruction_Type_Definitions."Start Task 9" ("Enum") Intruction_Type_Definitions."Start Task 9" ("Enum")] -> w184
          frame 0, Default {
          }
          frame 1 {
          }
          frame 2 {
          }
          frame 3 {
          }
          frame 4 {
          }
          frame 5 {
          }
          frame 6 {
          }
          frame 7 {
          }
          frame 8 {
          }
          frame 9 {
          }
          frame 10 {
          }
          frame 11 {
            # "Task 9: Red Detection"
            n63 = call "Box Colour FGV.vi"("Colour to detect"=Box_Colour_FGV_Colours."Blue", "Init/R/W State"=Box_Colour_FGV_States."Write") -> ()  [unwired: 8 in, 2 out]
          }
          frame 12 {
            # "Task 9: Black Detection"
            n64 = call "Box Colour FGV.vi"("Colour to detect"=Box_Colour_FGV_Colours."Black", "Init/R/W State"=Box_Colour_FGV_States."Write") -> ()  [unwired: 8 in, 2 out]
          }
          frame 13 {
            # "Task 9: Blue Detection"
            n65 = call "Box Colour FGV.vi"("Colour to detect"=Box_Colour_FGV_Colours."Green", "Init/R/W State"=Box_Colour_FGV_States."Write") -> ()  [unwired: 8 in, 2 out]
          }
          frame 14 {
            # "Task 9: Yellow Detection"
            n66 = call "Box Colour FGV.vi"("Colour to detect"=Box_Colour_FGV_Colours."Red", "Init/R/W State"=Box_Colour_FGV_States."Write") -> ()  [unwired: 8 in, 2 out]
          }
          frame 15 {
            # "Task 9: Green Detection"
            n67 = call "Box Colour FGV.vi"("Colour to detect"=Box_Colour_FGV_Colours."Yellow", "Init/R/W State"=Box_Colour_FGV_States."Write") -> ()  [unwired: 8 in, 2 out]
          }
        }
        "Selected Task" <- w184
        n68 = Enqueue Element(queue=w188, element=w184, error in (no error)=w186) -> (queue out=w187:refnum<queue>, error out=w185:errorcluster)  [unwired: 1 in, 1 out]
      }
      event User Event {
        n69 = event-data() -> ("Stop Queue"=w221:bool)  [unwired: 1 in, 4 out]
        n70 = Enqueue Element At Opposite End(queue=w219, element=Intruction_Type_Definitions."Exit" ("Enum"), error in (no error)=w218) -> (queue out=w220:refnum<queue>, error out=w217:errorcluster)  [unwired: 1 in, 1 out]
      }
    }
  }
  n71 = while {
    tunnel: w48 -> [w226]
    tunnel: w49 -> [w283]
    tunnel: w52 -> [w281]
    tunnel: [w280] -> _
    tunnel: [w279] -> w42
    shift-right: [w272] -> _
    shift-left: T9 {"PING_A"=0, "PING_B"=0, "PING_C"=0, "PING_D"=0} -> [w274]
    shift-right: [w266] -> _
    shift-left: State_Type_Definitions,_for_0.26g_versions_and_later_3."Startup" ("Enum") -> [w269]
    shift-right: [w262] -> _
    shift-left: T8 {"xDistance"=0.0, "yDistance"=0.0, "wDistance"=0.0} -> [w264]
    shift-right: [w260] -> _
    shift-left: _ -> [w259]
    shift-right: [w256] -> _
    shift-left: T11 {"Recognized Object"=FALSE, "Object X coordinate"=0.0, "Object Y coordinate"=0.0} -> [w258]
    shift-right: [w253] -> _
    shift-left: T7 {"y Stepper Position"=0, "z Stepper Position"=0} -> [w255]
    shift-right: [w250] -> _
    shift-left: T6 {"Yaw"=0.0, "Compass"=0.0} -> [w252]
    shift-right: [w247] -> _
    shift-left: T3 {"Time up flag"=FALSE, "SET TIME TO CHECK"=0.0} -> [w249]
    shift-right: [w245] -> _
    shift-left: T21 {"yStepper desired"=0} -> [w246]
    shift-right: [w241] -> _
    shift-left: T5 {"Left IR Sensor"=0.0, "Arm IR Sensor"=0.0, "Bottom IR Sensor"=0.0} -> [w243]
    shift-right: [w239] -> _
    shift-left: T20 {"ySpeed"=0.0, "xSpeed"=0.0, "wSpeed"=0.0} -> [w240]
    shift-right: [w236] -> _
    shift-left: T4 {"Line Detected?"=FALSE, "S1"=0.0, "S2"=0.0, "S3"=0.0, "S4"=0.0} -> [w238]
    shift-right: [w234] -> _
    shift-left: _ -> [w233]
    shift-right: [w225] -> _
    shift-left: T1 {"Red"=FALSE, "Black"=FALSE, "Blue"=FALSE, "Yellow"=FALSE, "Green"=FALSE, "Unknown"=FALSE, "Image processing done"=FALSE, "Colour"=enum."None"} -> [w228]
    stop <- w271 stop-if-true
    # ">>> Box Colour Detection >>>"
    # ">>State Logic Queue Reference >>"
    # ">>Action Queue>>"
    # ">>State Logic Queue Reference >>"
    # ">>> Line Sensor Cluster>>>"
    # ">>> IR Sensors >>>"
    # ">>> Time cluster >>>"
    # ">>> Object detection >>>"
    # ">>> Yaw >>>"
    # ">>> Ultrasonic Sensors Detect >>>"
    # ">>> Encoders >>>"
    # ">>> Stepper position >>>"
    # ">>State Logic  >>"
    # ">> Item Selection Bias >>"
    # ">> Item Selection Bias >>"
    # ">> Item Selection Bias >>"
    # ">>State Logic  >>"
    # ">>> Motor control cluster >>>"
    # ">>> yStepper command>>>"
    # ">>True Stop Next State >>"
    # ">>Error  >>"
    # ">>Timeout>>"
    # ">>Action states Queue Reference >>"
    # "TOP LEVEL BASELINE (MAIN PROCESSING LOOP)"
    n72 = Wait (ms)(milliseconds to wait=u32 25) -> ()  [unwired: 1 out]
    n73 = Dequeue Element(queue=w283, timeout in ms (-1)=0, error in (no error)=w281) -> (queue out=w275:refnum<queue>, element=w282:string, error out=w276:errorcluster)  [unwired: 1 out]
    "Action State" <- w282
    n74 = case shown="\"INIT\"" w282 {
      tunnel: [_ _ _ _ _ _ _ _ _ _ _ _ _ _ _ _ _ _ _ _ 0 w3856 _ _ _ _ _ _ _ _ _ _ _ _ _ _ _ _ _ _ _ _ _ _ _ _ _ _ _ _ _ _ _ _ _ _ _] -> w278
      tunnel: w275 -> [_ _ _ _ _ _ _ _ _ _ _ _ _ _ _ _ _ _ _ _ _ _ _ _ _ _ _ _ _ _ _ _ _ _ _ _ _ _ _ _ _ _ _ _ _ _ _ _ _ _ _ _ _ _ _ _ _]
      tunnel: w274 -> [w3525 w3537 w3552 w3566 w3586 w3601 w3615 w3629 w3645 w3660 w3674 w3684 w3702 w3719 w3734 w3749 w3773 w3783 w3817 w3830 w3844 w3857 w3869 w3882 w3902 w3937 w3974 w3988 w4001 w4013 w4026 w4041 w4057 w4069 w4081 w4101 w4124 w4135 w4151 w4182 w4192 w4205 w4218 w4231 w4241 w4259 w4269 w4288 w4297 w4313 w4329 w4345 w4361 w4377 w4391 w4406 w4426]
      tunnel: [w3525 w3537 w3552 w3566 w3586 w3601 w3615 w3629 w3645 w3660 w3674 w3684 w3702 w3720 w3734 w3749 w3773 w3783 w3818 w3830 w3844 w3857 w3869 w3882 w3902 w3936 w3973 w3988 w4001 w4013 w4026 w4041 w4057 w4069 w4081 w4101 w4124 w4135 w4151 w4182 w4192 w4205 w4218 w4231 w4241 w4259 w4269 w4288 w4297 w4313 w4329 w4345 w4361 w4377 w4391 w4406 w4426] -> w273
      tunnel: [TRUE TRUE _ _ _ _ _ _ _ _ _ _ _ _ _ _ _ _ _ _ _ _ _ _ _ _ _ _ _ _ _ _ _ _ _ _ _ _ _ _ _ _ _ _ _ _ _ _ _ _ _ _ _ _ _ _ _] -> w271
      tunnel: w269 -> [w3523 w3535 w3551 w3565 w3585 w3600 w3614 w3628 w3644 w3659 w3673 w3683 w3701 w3718 w3733 w3747 w3766 w3782 w3816 w3829 w3841 w3854 w3868 w3881 w3901 w3935 w3972 w3987 w4000 w4012 w4018 w4040 w4056 w4068 w4080 w4100 w4123 w4134 w4145 w4176 w4191 w4204 w4217 w4230 w4240 w4250 w4268 w4287 w4296 w4312 w4328 w4344 w4360 w4376 w4390 w4396 w4414]
      tunnel: [_ _ _ _ _ _ _ _ _ _ _ _ _ _ _ _ _ _ _ _ _ TRUE _ _ _ _ _ _ _ _ _ _ _ _ _ _ _ _ _ _ _ _ _ _ _ _ _ _ _ _ _ _ _ _ _ _ _] -> w268
      tunnel: [w3523 w3535 w3551 w3565 w3585 w3600 w3614 w3628 w3644 w3659 w3673 w3683 w3701 w3718 w3733 w3747 w3766 w3782 w3816 w3829 w3841 w3854 w3868 w3881 w3901 w3935 w3972 w3987 w4000 w4012 w4018 w4040 w4056 w4068 w4080 w4100 w4123 w4134 w4145 w4176 w4191 w4204 w4217 w4230 w4240 w4250 w4268 w4287 w4296 w4312 w4328 w4344 w4360 w4376 w4390 w4396 w4414] -> w267
      tunnel: w264 -> [w3522 w3534 w3550 w3568 w3584 w3599 w3613 w3627 w3643 w3658 w3672 w3685 w3700 w3717 w3735 w3751 w3768 w3784 w3815 w3831 w3840 w3853 w3870 w3883 w3897 w3926 w3962 w3986 w4003 w4014 w4023 w4042 w4058 w4070 w4082 w4102 w4125 w4137 w4149 w4180 w4194 w4207 w4220 w4233 w4243 w4254 w4271 w4290 w4299 w4315 w4331 w4347 w4363 w4379 w4393 w4398 w4419]
      tunnel: [w3522 w3534 w3550 w3568 w3584 w3599 w3613 w3627 w3643 w3658 w3672 w3685 w3699 w3717 w3735 w3751 w3768 w3784 w3814 w3831 w3840 w3853 w3870 w3883 w3897 w3925 w3961 w3986 w4003 w4014 w4023 w4042 w4058 w4070 w4082 w4102 w4125 w4137 w4149 w4180 w4194 w4207 w4220 w4233 w4243 w4254 w4271 w4290 w4299 w4315 w4331 w4347 w4363 w4379 w4393 w4398 w4419] -> w263
      tunnel: w258 -> [w3521 w3533 w3549 w3567 w3583 w3598 w3612 w3626 w3642 w3657 w3670 w3682 w3698 w3716 w3728 w3750 w3767 w3781 w3806 w3828 w3839 w3852 w3867 w3880 w3900 w3930 w3967 w3984 w4002 w4011 w4024 w4039 w4055 w4064 w4079 w4098 w4118 w4136 w4150 w4181 w4193 w4206 w4219 w4232 w4242 w4253 w4270 w4289 w4298 w4314 w4330 w4346 w4362 w4378 w4392 w4397 w4418]
      tunnel: [w3521 w3533 w3549 w3567 w3583 w3598 w3612 w3626 w3642 w3657 w3670 w3682 w3698 w3716 w3728 w3750 w3767 w3781 w3805 w3828 w3839 w3852 w3867 w3880 w3899 w3929 w3966 w3984 w4002 w4011 w4024 w4039 w4055 w4064 w4079 w4097 w4118 w4136 w4150 w4181 w4193 w4206 w4219 w4232 w4242 w4253 w4270 w4289 w4298 w4314 w4330 w4346 w4362 w4378 w4392 w4397 w4418] -> w257
      tunnel: w255 -> [w3520 w3532 w3548 w3569 w3582 w3597 w3611 w3625 w3641 w3656 w3669 w3681 w3697 w3715 w3736 w3752 w3769 w3780 w3811 w3827 w3838 w3851 w3866 w3879 w3896 w3921 w3957 w3983 w3999 w4010 w4022 w4038 w4054 w4067 w4078 w4103 w4126 w4138 w4148 w4179 w4190 w4203 w4216 w4229 w4244 w4255 w4272 w4286 w4300 w4316 w4332 w4348 w4364 w4380 w4394 w4399 w4420]
      tunnel: [w3520 w3532 w3548 w3569 w3582 w3597 w3611 w3625 w3641 w3656 w3669 w3681 w3697 w3715 w3736 w3752 w3769 w3780 w3810 w3827 w3838 w3851 w3866 w3879 w3896 w3920 w3956 w3983 w3999 w4010 w4022 w4038 w4054 w4067 w4078 w4103 w4126 w4138 w4148 w4179 w4190 w4203 w4216 w4229 w4244 w4255 w4272 w4285 w4300 w4316 w4332 w4348 w4364 w4380 w4394 w4399 w4420] -> w254
      tunnel: w252 -> [w3519 w3531 w3546 w3570 w3580 w3595 w3609 w3624 w3639 w3654 w3668 w3680 w3696 w3708 w3731 w3753 w3770 w3779 w3801 w3826 w3837 w3850 w3865 w3878 w3895 w3917 w3953 w3982 w3996 w4009 w4021 w4037 w4053 w4066 w4077 w4104 w4127 w4139 w4147 w4178 w4189 w4202 w4215 w4226 w4245 w4256 w4273 w4280 w4301 w4317 w4333 w4349 w4365 w4381 w4395 w4400 w4421]
      tunnel: [w3519 w3531 w3546 w3570 w3580 w3595 w3609 w3624 w3639 w3654 w3668 w3680 w3696 w3708 w3730 w3753 w3770 w3779 w3800 w3826 w3837 w3850 w3865 w3878 w3895 w3916 w3952 w3982 w3996 w4009 w4021 w4037 w4053 w4066 w4077 w4104 w4127 w4139 w4147 w4178 w4189 w4202 w4215 w4226 w4245 w4256 w4273 w4280 w4301 w4317 w4333 w4349 w4365 w4381 w4395 w4400 w4421] -> w251
      tunnel: w249 -> [w3517 w3530 w3547 w3571 w3581 w3596 w3610 w3623 w3640 w3655 w3667 w3679 w3695 w3707 w3727 w3754 w3771 w3778 w3797 w3823 w3836 w3849 w3864 w3877 w3894 w3914 w3950 w3980 w3995 w4008 w4020 w4036 w4052 w4065 w4076 w4105 w4128 w4140 w4146 w4177 w4188 w4201 w4214 w4225 w4246 w4257 w4274 w4279 w4295 w4311 w4327 w4343 w4359 w4375 w4389 w4401 w4422]
      tunnel: [w3517 w3530 w3547 w3571 w3581 w3596 w3610 w3623 w3640 w3655 w3667 w3679 w3695 w3707 w3727 w3754 w3771 w3778 w3797 w3823 w3836 w3849 w3864 w3877 w3893 w3913 w3949 w3980 w3995 w4008 w4020 w4036 w4052 w4065 w4076 w4105 w4128 w4140 w4146 w4177 w4188 w4201 w4214 w4225 w4246 w4257 w4274 w4279 w4295 w4309 w4325 w4341 w4357 w4374 w4388 w4401 w4422] -> w248
      tunnel: w246 -> [_ _ _ _ _ _ _ _ _ _ _ _ _ _ _ _ _ _ _ _ _ _ _ _ _ _ _ _ _ _ _ _ _ _ _ _ _ _ _ _ _ _ _ _ _ _ w4265 _ _ _ _ _ _ _ _ _ _]
      tunnel: [w3516 w3529 w3541 w3561 w3575 w3590 w3605 w3619 w3635 w3649 w3664 w3678 w3689 w3706 w3724 w3745 w3772 w3777 w3794 w3822 w3835 w3848 w3863 w3874 w3887 w3907 w3941 w3979 w3994 w4007 w4025 w4030 w4046 w4062 w4074 w4093 w4121 w4132 w4152 w4183 w4187 w4200 w4213 w4224 w4237 w4258 w4263 w4278 w4294 w4307 w4323 w4339 w4355 w4372 w4385 w4405 w4425] -> w242
      tunnel: w243 -> [w3516 w3529 w3541 w3561 w3575 w3590 w3605 w3619 w3635 w3649 w3664 w3678 w3689 w3706 w3724 w3746 w3772 w3777 w3794 w3822 w3835 w3848 w3863 w3874 w3887 w3908 w3942 w3979 w3994 w4007 w4025 w4030 w4046 w4062 w4074 w4093 w4121 w4132 w4152 w4183 w4187 w4200 w4213 w4224 w4237 w4258 w4263 w4278 w4294 w4307 w4323 w4339 w4355 w4372 w4385 w4405 w4425]
      tunnel: w240 -> [_ _ _ _ _ _ _ _ w3634 _ _ _ _ _ _ _ _ _ _ _ _ _ _ _ _ _ _ _ _ _ _ _ _ _ _ _ _ _ _ _ _ _ _ _ _ _ _ _ _ _ _ _ _ _ _ _ _]
      tunnel: w238 -> [w3515 w3528 w3540 w3555 w3574 w3589 w3604 w3618 w3632 w3648 w3663 w3677 w3688 w3705 w3723 w3741 w3765 w3776 w3792 w3821 w3834 w3847 w3862 w3873 w3890 w3910 w3945 w3978 w3993 w4006 w4017 w4029 w4045 w4061 w4073 w4091 w4120 w4131 w4143 w4175 w4186 w4199 w4212 w4223 w4236 w4249 w4262 w4277 w4293 w4306 w4322 w4338 w4354 w4371 w4384 w4404 w4424]
      tunnel: [w3515 w3528 w3540 w3555 w3574 w3589 w3604 w3618 w3632 w3648 w3663 w3677 w3688 w3705 w3723 w3741 w3764 w3776 w3792 w3821 w3834 w3847 w3862 w3873 w3889 w3909 w3944 w3978 w3993 w4006 w4017 w4029 w4045 w4061 w4073 w4091 w4120 w4131 w4143 w4175 w4186 w4199 w4212 w4223 w4236 w4249 w4262 w4277 w4293 w4306 w4322 w4338 w4354 w4371 w4384 w4404 w4424] -> w237
      tunnel: [_ _ _ _ _ _ _ _ _ _ _ _ _ _ _ _ _ _ _ _ _ _ _ _ _ _ _ _ _ _ _ _ _ _ _ w4085 w4115 _ _ _ _ _ _ _ _ _ _ _ _ _ _ _ _ _ _ _ _] -> w235
      tunnel: w233 -> [w3514 w3527 w3539 w3554 w3573 w3588 w3603 w3617 w3631 w3647 w3662 w3676 w3687 w3704 w3722 w3740 w3756 w3775 w3790 w3820 w3833 w3846 w3861 w3872 w3891 w3911 w3946 w3977 w3992 w4005 w4016 w4028 w4044 w4060 w4072 w4087 w4119 w4130 w4142 w4174 w4185 w4198 w4211 w4222 w4235 w4248 w4261 w4276 w4292 w4305 w4321 w4337 w4353 w4370 w4383 w4403 w4423]
      tunnel: [w3514 w3527 w3539 w3554 w3573 w3588 w3603 w3617 w3631 w3647 w3662 w3676 w3687 w3704 w3722 w3740 w3756 w3775 w3790 w3820 w3833 w3846 w3861 w3872 w3891 w3911 w3946 w3977 w3992 w4005 w4016 w4028 w4044 w4060 w4072 w4087 w4119 w4130 w4142 w4174 w4185 w4198 w4211 w4222 w4235 w4248 w4261 w4276 w4292 w4305 w4321 w4337 w4353 w4370 w4383 w4403 w4423] -> w232
      tunnel: w228 -> [w3513 w3526 w3538 w3553 w3572 w3587 w3602 w3616 w3630 w3646 w3661 w3675 w3686 w3703 w3721 w3737 w3755 w3774 w3789 w3819 w3832 w3845 w3860 w3871 w3886 w3904 w3940 w3976 w3991 w4004 w4015 w4027 w4043 w4059 w4071 w4090 w4113 w4129 w4141 w4173 w4184 w4197 w4210 w4221 w4234 w4247 w4260 w4275 w4291 w4304 w4320 w4336 w4352 w4369 w4382 w4402 w4417]
      tunnel: [w3513 w3526 w3538 w3553 w3572 w3587 w3602 w3616 w3630 w3646 w3661 w3675 w3686 w3703 w3721 w3737 w3755 w3774 w3789 w3819 w3832 w3845 w3860 w3871 w3885 w3904 w3940 w3976 w3991 w4004 w4015 w4027 w4043 w4059 w4071 w4090 w4106 w4129 w4141 w4172 w4184 w4197 w4210 w4221 w4234 w4247 w4260 w4275 w4291 w4304 w4320 w4336 w4352 w4369 w4382 w4402 w4416] -> w227
      frame "Exit" {
        # ">>State Logic  >>"
        # ">>> Time cluster >>>"
        # ">>> Yaw >>>"
        # ">>> Stepper position >>>"
        # ">>> Encoders >>>"
        # ">>> Object detection >>>"
        # ">>> Ultrasonic Sensors Detect >>>"
        n75 = call "Imaq Dispose"("All Images? (No)"=TRUE) -> ()  [unwired: 5 in, 1 out]
      }
      frame "----Movement States----" {
        # ">>State Logic  >>"
        # ">>> Time cluster >>>"
        # ">>> Yaw >>>"
        # ">>> Stepper position >>>"
        # ">>> Encoders >>>"
        # ">>> Object detection >>>"
        # ">>> Ultrasonic Sensors Detect >>>"
      }
      frame "FORWARD" {
        # "High voltage values: 30\nMid voltage values: 40\nLow voltage values: 50"
        # ">>State Logic  >>"
        # ">>> Time cluster >>>"
        # ">>> Yaw >>>"
        # ">>> Stepper position >>>"
        # ">>> Encoders >>>"
        # ">>> Object detection >>>"
        # ">>> Ultrasonic Sensors Detect >>>"
        n76 = Unbundle By Name(w3546) -> ("Yaw"=w3542:dbl)
        n77 = call "MOTOR CONTROL WITH PID AE.vi"("Yaw"=w3542, "Speed"=30.0, "Direction"=MOTOR_CONTROL_WITH_PID_AE_DIRECTION_TYPE_DEF."y-axis movement", "AE Mode"=MOTOR_CONTROL_WITH_PID_AE_DATA_MODE_TYPE_DEF."Write to AE") -> ()  [unwired: 1 out]
      }
      frame "FORWARD - IR ASSIST" {
        # "Algorithm sensitivity"
        # "Distance to maintain from wall"
        # ">>State Logic  >>"
        # ">>> Time cluster >>>"
        # ">>> Yaw >>>"
        # ">>> Stepper position >>>"
        # ">>> Encoders >>>"
        # ">>> Object detection >>>"
        # ">>> Ultrasonic Sensors Detect >>>"
        n78 = Unbundle By Name(w3561) -> ("Left IR Sensor"=w3560:dbl)
        n79 = Subtract(x=w3560, y=25.0) -> (x-y=w3558:dbl)
        n80 = Multiply(x=w3558, y=0.2) -> (x*y=w3556:dbl)
        n81 = call "MOTOR CONTROL WITH PID AE.vi"("Yaw"=w3556, "Speed"=35.0, "Direction"=MOTOR_CONTROL_WITH_PID_AE_DIRECTION_TYPE_DEF."y-axis movement", "AE Mode"=MOTOR_CONTROL_WITH_PID_AE_DATA_MODE_TYPE_DEF."Write to AE") -> ()  [unwired: 1 out]
      }
      frame "LEFT" {
        # ">>State Logic  >>"
        # ">>> Time cluster >>>"
        # ">>> Yaw >>>"
        # ">>> Stepper position >>>"
        # ">>> Encoders >>>"
        # ">>> Object detection >>>"
        # ">>> Ultrasonic Sensors Detect >>>"
        n82 = Unbundle By Name(w3580) -> ("Yaw"=w3577:dbl)
        n83 = call "MOTOR CONTROL WITH PID AE.vi"("Yaw"=w3577, "Speed"=-25.0, "Direction"=MOTOR_CONTROL_WITH_PID_AE_DIRECTION_TYPE_DEF."x-axis movement", "AE Mode"=MOTOR_CONTROL_WITH_PID_AE_DATA_MODE_TYPE_DEF."Write to AE") -> ()  [unwired: 1 out]
      }
      frame "RIGHT" {
        # ">>> Time cluster >>>"
        # ">>> Yaw >>>"
        # ">>> Stepper position >>>"
        # ">>> Encoders >>>"
        # ">>> Object detection >>>"
        # ">>> Ultrasonic Sensors Detect >>>"
        n84 = Unbundle By Name(w3595) -> ("Yaw"=w3591:dbl)
        n85 = call "MOTOR CONTROL WITH PID AE.vi"("Yaw"=w3591, "Speed"=25.0, "Direction"=MOTOR_CONTROL_WITH_PID_AE_DIRECTION_TYPE_DEF."x-axis movement", "AE Mode"=MOTOR_CONTROL_WITH_PID_AE_DATA_MODE_TYPE_DEF."Write to AE") -> ()  [unwired: 1 out]
      }
      frame "R-ACW" {
        # ">>> IR Sensors >>>"
        # ">>> Time cluster >>>"
        # ">>> Yaw >>>"
        # ">>> Stepper position >>>"
        # ">>> Encoders >>>"
        # ">>> Object detection >>>"
        # ">>> Ultrasonic Sensors Detect >>>"
        n86 = call "MOTOR CONTROL WITH PID AE.vi"("Speed"=10.0, "Direction"=MOTOR_CONTROL_WITH_PID_AE_DIRECTION_TYPE_DEF."rotation", "AE Mode"=MOTOR_CONTROL_WITH_PID_AE_DATA_MODE_TYPE_DEF."Write to AE") -> ()  [unwired: 1 in, 1 out]
      }
      frame "R-CW" {
        (unwired) -0.2 ("Speed")
        # ">>> Time cluster >>>"
        # ">>> Yaw >>>"
        # ">>> Stepper position >>>"
        # ">>> Encoders >>>"
        # ">>> Object detection >>>"
        # ">>> Ultrasonic Sensors Detect >>>"
        n87 = call "MOTOR CONTROL WITH PID AE.vi"("Speed"=-10.0, "Direction"=MOTOR_CONTROL_WITH_PID_AE_DIRECTION_TYPE_DEF."rotation", "AE Mode"=MOTOR_CONTROL_WITH_PID_AE_DATA_MODE_TYPE_DEF."Write to AE") -> ()  [unwired: 1 in, 1 out]
      }
      frame "X AXIS - SLOW" {
        # ">>> Line Sensor Cluster>>>"
        # ">>> IR Sensors >>>"
        # ">>> Time cluster >>>"
        # ">>> Yaw >>>"
        # ">>> Stepper position >>>"
        # ">>> Encoders >>>"
        # ">>> Object detection >>>"
        # ">>> Ultrasonic Sensors Detect >>>"
        n88 = Unbundle By Name(w3634) -> ("xSpeed"=w3633:dbl)
        n89 = Unbundle By Name(w3639) -> ("Yaw"=w3636:dbl)
        n90 = call "MOTOR CONTROL WITH PID AE.vi"("Yaw"=w3636, "Speed"=w3633, "Direction"=MOTOR_CONTROL_WITH_PID_AE_DIRECTION_TYPE_DEF."x-axis movement", "AE Mode"=MOTOR_CONTROL_WITH_PID_AE_DATA_MODE_TYPE_DEF."Write to AE") -> ()  [unwired: 1 out]
      }
      frame "REVERSE" {
        # ">>> Time cluster >>>"
        # ">>> Yaw >>>"
        # ">>> Stepper position >>>"
        # ">>> Encoders >>>"
        # ">>> Object detection >>>"
        # ">>> Ultrasonic Sensors Detect >>>"
        n91 = Unbundle By Name(w3654) -> ("Yaw"=w3650:dbl)
        n92 = call "MOTOR CONTROL WITH PID AE.vi"("Yaw"=w3650, "Speed"=-40.0, "Direction"=MOTOR_CONTROL_WITH_PID_AE_DIRECTION_TYPE_DEF."y-axis movement", "AE Mode"=MOTOR_CONTROL_WITH_PID_AE_DATA_MODE_TYPE_DEF."Write to AE") -> ()  [unwired: 1 out]
      }
      frame "STOP" {
        n93 = Wait (ms)(milliseconds to wait=u32 100) -> ()  [unwired: 1 out]
        n94 = call "MOTOR CONTROL WITH PID AE.vi"("Direction"=MOTOR_CONTROL_WITH_PID_AE_DIRECTION_TYPE_DEF."stop", "AE Mode"=MOTOR_CONTROL_WITH_PID_AE_DATA_MODE_TYPE_DEF."Write to AE") -> ()  [unwired: 2 in, 1 out]
      }
      frame "----SENSOR READING---- " {
      }
      frame "READ ENCODERS" {
        # ">>> Time cluster >>>"
        # ">>> Yaw >>>"
        # ">>> Stepper position >>>"
        # ">>> Object detection >>>"
        # ">>> Current encoder distance >>>"
        # ">>> Ultrasonic Sensors Detect >>>"
        n95 = call "MOTOR CONTROL WITH PID AE.vi"("AE Mode"=MOTOR_CONTROL_WITH_PID_AE_DATA_MODE_TYPE_DEF."Read from AE") -> ("Speed & distance"=w3693:T15)  [unwired: 3 in]
        n96 = Unbundle By Name(w3693) -> ("xDistance"=w3692:dbl, "yDistance"=w3691:dbl, "wDistance"=w3690:dbl)
        n97 = Bundle By Name(cluster=w3700, "xDistance"=w3692, "yDistance"=w3691, "wDistance"=w3690) -> (w3699:T8)
      }
      frame "READ ULTRASONIC" {
        (unwired) navX_type_def."Read Values" ("Mode")
        (unwired) MOTOR_CONTROL_NO_PID_Type_Def."Latch" ("Direction")
        # ">>> Line Sensor Cluster>>>"
        # ">>> IR Sensors >>>"
        # ">>State Logic  >>"
        # ">>> Time cluster >>>"
        # ">>> Ultrasonic Sensors Detect >>>"
        # ">>> Object detection >>>"
        # ">>> Encoders >>>"
        # ">>> Stepper position >>>"
        # ">>> Yaw >>>"
        n98 = call "Arduino Interfacing VI.vi"("AE Mode"=Arduino_Interfacing."Read From Arduino") -> ("Arduino Data"=w3713:T17)  [unwired: 3 in, 1 out]
        n99 = Unbundle By Name(w3713) -> ("PING A"=w3712:u8, "PING B"=w3711:u8, "PING C"=w3710:u8, "PING D"=w3709:u8)
        n100 = Bundle By Name(cluster=w3719, "PING_A"=w3712, "PING_B"=w3711, "PING_C"=w3710, "PING_D"=w3709) -> (w3720:T9)
      }
      frame "READ NAVX" {
        # ">> Item Selection Bias >>"
        # ">>State Logic  >>"
        # ">>> Line Sensor Cluster>>>"
        # ">>> IR Sensors >>>"
        # ">>> Time cluster >>>"
        # ">>> Yaw >>>"
        # ">>> Ultrasonic Sensors Detect >>>"
        # ">>> Object detection >>>"
        # ">>> Encoders >>>"
        # ">>> Stepper position >>>"
        n101 = call "navX reading VI.vi"("Mode"=navX_type_def."Read Values") -> ("NavX Readings"=w3726:T16)  [unwired: 2 in, 3 out]
        n102 = Unbundle By Name(w3726) -> ("Heading"=w3725:dbl)
        n103 = Unbundle By Name(w3726) -> ("Yaw"=w3729:dbl)
        n104 = Bundle By Name(cluster=w3731, "Yaw"=w3729, "Compass"=w3725) -> (w3730:T6)
      }
      frame "READ IR" {
        w3739 = T43 [enum."B/AI2"] items=["Not Connected", "AudioIn/Left", "AudioIn/Right", "C/AI0", "C/AI1", "A/AI0", "A/AI1", "A/AI2", "A/AI3", "A/AI4", "A/AI5", "A/AI6", "A/AI7", "B/AI0", "B/AI1", "B/AI2", "B/AI3", "B/AI4", "B/AI5", "B/AI6", "B/AI7", "AI/AI0", "AI/AI1", "AI/AI2", "AI/AI3", "A/AI0 (DIFF)", "A/AI1 (DIFF)", "A/AI2 (DIFF)", "A/AI3 (DIFF)", "B/AI0 (DIFF)", "B/AI1 (DIFF)", "B/AI2 (DIFF)", "B/AI3 (DIFF)"] ("AI Channel")
        w3743 = T43 [enum."B/AI1"] items=["Not Connected", "AudioIn/Left", "AudioIn/Right", "C/AI0", "C/AI1", "A/AI0", "A/AI1", "A/AI2", "A/AI3", "A/AI4", "A/AI5", "A/AI6", "A/AI7", "B/AI0", "B/AI1", "B/AI2", "B/AI3", "B/AI4", "B/AI5", "B/AI6", "B/AI7", "AI/AI0", "AI/AI1", "AI/AI2", "AI/AI3", "A/AI0 (DIFF)", "A/AI1 (DIFF)", "A/AI2 (DIFF)", "A/AI3 (DIFF)", "B/AI0 (DIFF)", "B/AI1 (DIFF)", "B/AI2 (DIFF)", "B/AI3 (DIFF)"] ("AI Channel")
        w3748 = T43 [enum."B/AI0"] items=["Not Connected", "AudioIn/Left", "AudioIn/Right", "C/AI0", "C/AI1", "A/AI0", "A/AI1", "A/AI2", "A/AI3", "A/AI4", "A/AI5", "A/AI6", "A/AI7", "B/AI0", "B/AI1", "B/AI2", "B/AI3", "B/AI4", "B/AI5", "B/AI6", "B/AI7", "AI/AI0", "AI/AI1", "AI/AI2", "AI/AI3", "A/AI0 (DIFF)", "A/AI1 (DIFF)", "A/AI2 (DIFF)", "A/AI3 (DIFF)", "B/AI0 (DIFF)", "B/AI1 (DIFF)", "B/AI2 (DIFF)", "B/AI3 (DIFF)"] ("AI Channel")
        # ">>> Line Sensor Cluster>>>"
        # ">>> IR Sensors >>>"
        # ">>State Logic  >>"
        # ">>> Time cluster >>>"
        # ">>> Ultrasonic Sensors Detect >>>"
        # ">>> Object detection >>>"
        # ">>> Encoders >>>"
        # ">>> Stepper position >>>"
        # ">>> Yaw >>>"
        n105 = call <vilib>:"Sharp IR.vi"("AI Channel"=w3748) -> ("Sharp IR Distance"=w3744:dbl)  [unwired: 8 in, 2 out]
        n106 = call <vilib>:"Sharp IR.vi"("AI Channel"=w3743) -> ("Sharp IR Distance"=w3742:dbl)  [unwired: 8 in, 2 out]
        n107 = call <vilib>:"Sharp IR.vi"("AI Channel"=w3739) -> ("Sharp IR Distance"=w3738:dbl)  [unwired: 8 in, 2 out]
        n108 = Bundle By Name(cluster=w3746, "Left IR Sensor"=w3744, "Arm IR Sensor"=w3742, "Bottom IR Sensor"=w3738) -> (w3745:T5)
      }
      frame "READ LINE SENSOR" {
        # ">>> IR Sensors >>>"
        # ">>> Line Sensor Cluster>>>"
        # ">>State Logic  >>"
        # ">>> Time cluster >>>"
        # ">>> Object detection >>>"
        # ">>> Yaw >>>"
        # ">>> Ultrasonic Sensors Detect >>>"
        # ">>> Encoders >>>"
        # ">>> Stepper position >>>"
        n109 = call "Line Sensor AE.vi"("AE State"=Line_Sensor_AE_Type_Def."READ FROM LINE SENSORS") -> ("Line Detected?"=w3762:bool, "Line Sensor Raw Values"=w3761:T45)
        n110 = Unbundle By Name(w3761) -> ("S1"=w3760:dbl, "S2"=w3759:dbl, "S3"=w3758:dbl, "S4"=w3757:dbl)
        n111 = Bundle By Name(cluster=w3765, "Line Detected?"=w3762, "S1"=w3760, "S2"=w3759, "S3"=w3758, "S4"=w3757) -> (w3764:T4)
      }
      frame "----SYSTEM MODES----" {
        (unwired) I2C_MASTER_Type_Def."Last State" ("Arduino Mode")
        # ">>> Object detection >>>"
        # ">>> Yaw >>>"
        # ">>> Ultrasonic Sensors Detect >>>"
        # ">>> Encoders >>>"
        # ">>> Stepper position >>>"
      }
      frame "INIT" {
        w3812 = u8 0
        w3813 = 0.0
        # ">>> Box Colour Detection >>>"
        # ">>> IR Sensors >>>"
        # ">>> IR Sensors >>>"
        # ">>> Line Sensor Cluster>>>"
        # ">>> Time cluster >>>"
        # ">>> Object detection >>>"
        # ">>> Yaw >>>"
        # ">>> Ultrasonic Sensors Detect >>>"
        # ">>> Encoders >>>"
        # ">>> Stepper position >>>"
        # ">>State Logic  >>"
        n112 = call "Arduino Interfacing VI.vi"("AE Mode"=Arduino_Interfacing."Initialize") -> ()  [unwired: 3 in, 2 out]
        n113 = call "FGV Stop.vi"("Init/Read/Write State"=States_for_Action_Engine."Initialize") -> ()  [unwired: 2 in, 2 out]
        n114 = call "Elasped Timer.vi"("Action"=Elapsed_timer_control."Initialize") -> ()  [unwired: 7 in, 4 out]
        n115 = call "MOTOR CONTROL WITH PID AE.vi"("AE Mode"=MOTOR_CONTROL_WITH_PID_AE_DATA_MODE_TYPE_DEF."Init AE") -> ()  [unwired: 3 in, 1 out]
        n116 = call "IMAQ Reference AE.vi"("IMAQ AE States"=IMAQ_Reference_AE."Initialize AE") -> ()  [unwired: 1 in, 2 out]
        n117 = call "Line Sensor AE.vi"("AE State"=Line_Sensor_AE_Type_Def."INIT AE") -> ()  [unwired: 2 out]
        n118 = Bundle By Name(cluster=w3806, "Recognized Object"=FALSE, "Object X coordinate"=0.0, "Object Y coordinate"=0.0) -> (w3805:T11)
        n119 = Bundle By Name(cluster=w3811, "y Stepper Position"=u8 0, "z Stepper Position"=u8 0) -> (w3810:T7)
        n120 = Bundle By Name(cluster=w3815, "xDistance"=w3813, "yDistance"=w3813, "wDistance"=w3813) -> (w3814:T8)
        n121 = Bundle By Name(cluster=w3817, "PING_A"=w3812, "PING_B"=w3812, "PING_C"=w3812, "PING_D"=w3812) -> (w3818:T9)
        n122 = invoke class="VI" method="Default Vals.Reinit All"() -> ()  [unwired: 3 in, 3 out]
        n123 = Bundle By Name(cluster=w3801, "Yaw"=0.0) -> (w3800:T6)
        n124 = call "Box Colour FGV.vi"("Init/R/W State"=Box_Colour_FGV_States."Initialize") -> ()  [unwired: 9 in, 2 out]
        n125 = call "Servo State FGV.vi"("Init/Read/Write State"=States_for_Action_Engine."Initialize") -> ()  [unwired: 2 in, 2 out]
        n126 = call "yDistance travelled FGV.vi"("Init/Read/Write State"=States_for_Action_Engine."Initialize") -> ()  [unwired: 9 in, 2 out]
        n127 = call "Task Enable FGV.vi"("Init/Read/Write State"=States_for_Action_Engine."Initialize") -> ()  [unwired: 9 in, 2 out]
      }
      frame "ARDUINO - ULTRASONIC" {
        # ">>> Time cluster >>>"
        # ">>> Line Sensor Cluster>>>"
        # ">>> Object detection >>>"
        # ">>> Yaw >>>"
        # ">>> Ultrasonic Sensors Detect >>>"
        # ">>> Encoders >>>"
        # ">>> Stepper position >>>"
        # ">>State Logic  >>"
        n128 = call "Arduino Interfacing VI.vi"("Data to Write"=I2C_MASTER_WRITE_NEW_Type_Def."Ultrasonic sensors", "AE Mode"=Arduino_Interfacing."Write to Arduino") -> ()  [unwired: 2 in, 2 out]
      }
      frame "NAVX CALIBRATE" {
        # ">>> Object detection >>>"
        # ">>> Yaw >>>"
        # ">>> Ultrasonic Sensors Detect >>>"
        # ">>> Encoders >>>"
        # ">>> Stepper position >>>"
        # ">>State Logic  >>"
        # "Adds a 15 second delay to the startup process \nfor the NavX to calibrate"
        n129 = Wait (ms)(milliseconds to wait=u32 1000) -> ()  [unwired: 1 out]
      }
      frame "NO ACTION", Default {
        (unwired) u8 0 ("y Stepper value")
        (unwired) TRUE ("Latch")
        (unwired) navX_type_def."Read Values" ("Mode")
        (unwired) MOTOR_CONTROL_NO_PID_Type_Def."Latch" ("Direction")
        # ">>> Object detection >>>"
        # ">>> Yaw >>>"
        # ">>> Ultrasonic Sensors Detect >>>"
        # ">>> Encoders >>>"
        # ">>> Stepper position >>>"
        # ">>State Logic  >>"
        n130 = case shown="\"Idle\"" w3854 {
          tunnel: [0 100] -> w3856
          frame "Startup", Default {
          }
          frame "Idle" {
          }
        }
      }
      frame "----RESET CASES----" {
        (unwired) I2C_MASTER_Type_Def."Last State" ("Arduino Mode")
        # ">>> Object detection >>>"
        # ">>> Yaw >>>"
        # ">>> Ultrasonic Sensors Detect >>>"
        # ">>> Encoders >>>"
        # ">>> Stepper position >>>"
        # ">>State Logic  >>"
      }
      frame "RESET ENCODERS" {
        # ">>> Object detection >>>"
        # ">>> Yaw >>>"
        # ">>> Ultrasonic Sensors Detect >>>"
        # ">>> Encoders >>>"
        # ">>> Stepper position >>>"
        # ">>State Logic  >>"
        n131 = call "MOTOR CONTROL WITH PID AE.vi"("Direction"=MOTOR_CONTROL_WITH_PID_AE_DIRECTION_TYPE_DEF."reset encoders", "AE Mode"=MOTOR_CONTROL_WITH_PID_AE_DATA_MODE_TYPE_DEF."Write to AE") -> ()  [unwired: 2 in, 1 out]
      }
      frame "RESET FLAGS" {
        w3884 = FALSE ("Line Detected?")
        # ">>> Line Sensor Cluster>>>"
        # ">>> IR Sensors >>>"
        # ">>> Time cluster >>>"
        # ">>> Object detection >>>"
        # ">>> Yaw >>>"
        # ">>> Ultrasonic Sensors Detect >>>"
        # ">>> Encoders >>>"
        # ">>> Stepper position >>>"
        # ">>> Line Sensor Cluster>>>"
        # ">>> IR Sensors >>>"
        # ">>> Time cluster >>>"
        # ">>> Object detection >>>"
        # ">>> Yaw >>>"
        # ">>> Ultrasonic Sensors Detect >>>"
        # ">>> Encoders >>>"
        # ">>> Stepper position >>>"
        # "Resets BOOLEAN FLAGS only"
        n132 = Wait (ms)(milliseconds to wait=u32 20) -> ()  [unwired: 1 out]
        n133 = Bundle By Name(cluster=w3900, "Recognized Object"=FALSE) -> (w3899:T11)
        n134 = Bundle By Name(cluster=w3890, "Line Detected?"=FALSE) -> (w3889:T4)
        n135 = Bundle By Name(cluster=w3894, "Time up flag"=FALSE) -> (w3893:T3)
        n136 = Bundle By Name(cluster=w3886, "Red"=w3884, "Black"=w3884, "Blue"=w3884, "Yellow"=w3884, "Green"=w3884, "Unknown"=w3884, "Image processing done"=w3884) -> (w3885:T1)
      }
      frame "RESET SENSOR VALUES" {
        w3905 = 0.0 ("S4")
        w3906 = 0.0 ("S4")
        # "Resets SENSOR VALUES only"
        # ">>> Line Sensor Cluster>>>"
        # ">>> IR Sensors >>>"
        # ">>> Time cluster >>>"
        # ">>> Object detection >>>"
        # ">>> Yaw >>>"
        # ">>> Ultrasonic Sensors Detect >>>"
        # ">>> Encoders >>>"
        # ">>> Stepper position >>>"
        # ">>> Line Sensor Cluster>>>"
        # ">>> IR Sensors >>>"
        # ">>> Time cluster >>>"
        # ">>> Object detection >>>"
        # ">>> Yaw >>>"
        # ">>> Ultrasonic Sensors Detect >>>"
        # ">>> Encoders >>>"
        # ">>> Stepper position >>>"
        # "Resets any software variables\nand/or non-critical states"
        n137 = Wait (ms)(milliseconds to wait=u32 20) -> ()  [unwired: 1 out]
        n138 = Bundle By Name(cluster=w3914, "SET TIME TO CHECK"=0.0) -> (w3913:T3)
        n139 = Bundle By Name(cluster=w3930, "Object X coordinate"=0.0, "Object Y coordinate"=0.0) -> (w3929:T11)
        n140 = Bundle By Name(cluster=w3921, "y Stepper Position"=u8 0, "z Stepper Position"=u8 0) -> (w3920:T7)
        n141 = Bundle By Name(cluster=w3908, "Left IR Sensor"=w3905, "Arm IR Sensor"=w3905) -> (w3907:T5)
        n142 = Bundle By Name(cluster=w3926, "xDistance"=0.0, "yDistance"=0.0, "wDistance"=0.0) -> (w3925:T8)
        n143 = Bundle By Name(cluster=w3937, "PING_A"=u8 0, "PING_B"=u8 0, "PING_C"=u8 0, "PING_D"=u8 0) -> (w3936:T9)
        n144 = Bundle By Name(cluster=w3917, "Yaw"=0.0) -> (w3916:T6)
        n145 = Bundle By Name(cluster=w3910, "S1"=w3906, "S2"=w3906, "S3"=w3906, "S4"=w3906) -> (w3909:T4)
      }
      frame "RESET ALL SENSORS" {
        w3939 = 0.0 ("SET TIME TO CHECK")
        # ">>> Line Sensor Cluster>>>"
        # ">>> IR Sensors >>>"
        # ">>> Time cluster >>>"
        # ">>> Object detection >>>"
        # ">>> Yaw >>>"
        # ">>> Ultrasonic Sensors Detect >>>"
        # ">>> Encoders >>>"
        # ">>> Stepper position >>>"
        # ">>> Line Sensor Cluster>>>"
        # ">>> IR Sensors >>>"
        # ">>> Time cluster >>>"
        # ">>> Object detection >>>"
        # ">>> Yaw >>>"
        # ">>> Ultrasonic Sensors Detect >>>"
        # ">>> Encoders >>>"
        # ">>> Stepper position >>>"
        # "Resets ALL SENSOR PARAMTERS"
        n146 = Wait (ms)(milliseconds to wait=u32 20) -> ()  [unwired: 1 out]
        n147 = Bundle By Name(cluster=w3950, "Time up flag"=FALSE, "SET TIME TO CHECK"=0.0) -> (w3949:T3)
        n148 = Bundle By Name(cluster=w3967, "Recognized Object"=FALSE, "Object X coordinate"=0.0, "Object Y coordinate"=0.0) -> (w3966:T11)
        n149 = Bundle By Name(cluster=w3957, "y Stepper Position"=u8 0, "z Stepper Position"=u8 0) -> (w3956:T7)
        n150 = Bundle By Name(cluster=w3942, "Left IR Sensor"=w3939, "Arm IR Sensor"=w3939, "Bottom IR Sensor"=w3939) -> (w3941:T5)
        n151 = Bundle By Name(cluster=w3945, "Line Detected?"=FALSE) -> (w3944:T4)
        n152 = Bundle By Name(cluster=w3962, "xDistance"=0.0, "yDistance"=0.0, "wDistance"=0.0) -> (w3961:T8)
        n153 = Bundle By Name(cluster=w3974, "PING_A"=u8 0, "PING_B"=u8 0, "PING_C"=u8 0, "PING_D"=u8 0) -> (w3973:T9)
        n154 = Bundle By Name(cluster=w3953, "Yaw"=0.0) -> (w3952:T6)
      }
      frame "RESET YAW" {
        n155 = Wait (ms)(milliseconds to wait=u32 100) -> ()  [unwired: 1 out]
        n156 = call "navX reading VI.vi"("Mode"=navX_type_def."Zero Yaw") -> ()  [unwired: 2 in, 4 out]
      }
      frame "RESET ARM" {
        n157 = call "Arduino Interfacing VI.vi"("Data to Write"=I2C_MASTER_WRITE_NEW_Type_Def."Soft Reset", "AE Mode"=Arduino_Interfacing."Write to Arduino") -> ()  [unwired: 2 in, 2 out]
        n158 = call "Servo State FGV.vi"("Init/Read/Write State"=States_for_Action_Engine."Write", "Servo State"=Servo_States_FGV_Enum."Open Claw") -> ()  [unwired: 1 in, 2 out]
      }
      frame "--------CAM STATES-------" {
      }
      frame "OPEN IMAQ REF" {
        # ">>> Line Sensor Cluster>>>"
        # ">>State Logic  >>"
        # ">>> Time cluster >>>"
        # ">>> Object detection >>>"
        # ">>> Yaw >>>"
        # ">>> Ultrasonic Sensors Detect >>>"
        # ">>> Encoders >>>"
        # ">>> Stepper position >>>"
        # ">>> IR Sensors >>>"
        n159 = call "IMAQ Reference AE.vi"("IMAQ AE States"=IMAQ_Reference_AE."Initialize AE") -> ()  [unwired: 1 in, 2 out]
      }
      frame "OPEN LOG CAM" {
        n160 = call "Webcam AE.vi"("Session In"=T41 "cam0", "Camera states"=Webcam_AE."Initialize Camera") -> ("error out"=w4033:errorcluster, "Session Out"=w4032:T41)  [unwired: 1 in, 1 out]
        n161 = call "Webcam AE.vi"("error in (no error)"=w4033, "Session In"=w4032, "Camera states"=Webcam_AE."Open Camera") -> ()  [unwired: 3 out]
      }
      frame "OPEN LIFE CAM" {
        n162 = call "Webcam AE.vi"("Session In"=T41 "cam1", "Camera states"=Webcam_AE."Initialize Camera") -> ("error out"=w4049:errorcluster, "Session Out"=w4048:T41)  [unwired: 1 in, 1 out]
        n163 = call "Webcam AE.vi"("error in (no error)"=w4049, "Session In"=w4048, "Camera states"=Webcam_AE."Open Camera") -> ()  [unwired: 3 out]
      }
      frame "CAM ACQ" {
        # ">>State Logic  >>"
        # ">>> Time cluster >>>"
        # ">>> Yaw >>>"
        # ">>> Stepper position >>>"
        # ">>> Encoders >>>"
        # ">>> Object detection >>>"
        # ">>> Ultrasonic Sensors Detect >>>"
        n164 = call "Webcam AE.vi"("Camera states"=Webcam_AE."Continuous Acquisition") -> ()  [unwired: 2 in, 3 out]
      }
      frame "CAM CLOSE" {
        # ">>> Box Colour Detection >>>"
        # ">>> Line Sensor Cluster>>>"
        # ">>> IR Sensors >>>"
        # ">>State Logic  >>"
        # ">>> Time cluster >>>"
        # ">>> Yaw >>>"
        # ">>> Stepper position >>>"
        # ">>> Encoders >>>"
        # ">>> Object detection >>>"
        # ">>> Ultrasonic Sensors Detect >>>"
        n165 = call "Webcam AE.vi"("Camera states"=Webcam_AE."Close Camera") -> ()  [unwired: 2 in, 3 out]
      }
      frame "PROCESS IMAGE" {
        # ">>> Line Sensor Cluster>>>"
        # ">>> IR Sensors >>>"
        # ">> Item Selection Bias >>"
        # ">> Item Selection Bias >>"
        # ">>State Logic  >>"
        # ">>> Time cluster >>>"
        # ">>> Yaw >>>"
        # ">>> Stepper position >>>"
        # ">>> Encoders >>>"
        # ">>> Object detection >>>"
        # ">>> Ultrasonic Sensors Detect >>>"
        n166 = call "Webcam AE.vi"("Camera states"=Webcam_AE."Retrieve Image") -> ("error out"=w4086:errorcluster, "Image Out"=w4089:T47)  [unwired: 2 in, 1 out]
        n167 = call "IMAQ Reference AE.vi"("IMAQ AE States"=IMAQ_Reference_AE."Get IMAQ Reference") -> ("Image Out"=w4088:T47)  [unwired: 1 in, 1 out]
        n168 = call "Object Detection SubVI v2.vi"("Error In"=w4086, "Mode"=w4087, "Image Dest"=w4088, "Image in"=w4089) -> ("Error out"=w4085:errorcluster, "Object Center Coordinates"=w4084:cluster{"x":sgl, "y":sgl}, "Object detection cluster"=w4083:T48)  [unwired: 1 out]
        n169 = Unbundle By Name(w4083) -> ("Object detected?"=w4094:bool)
        n170 = Unbundle By Name(w4084) -> ("x"=w4096:sgl, "y"=w4095:sgl)
        n171 = Bundle By Name(cluster=w4098, "Recognized Object"=w4094, "Object X coordinate"=w4096, "Object Y coordinate"=w4095) -> (w4097:T11)
      }
      frame "COLOUR PROCESSING" {
        # ">>> Box Colour Detection >>>"
        # ">>> Box Colour Detection >>>"
        # ">>> Line Sensor Cluster>>>"
        # ">>> IR Sensors >>>"
        # ">> Item Selection Bias >>"
        # ">> Item Selection Bias >>"
        # ">>State Logic  >>"
        # ">>> Time cluster >>>"
        # ">>> Yaw >>>"
        # ">>> Stepper position >>>"
        # ">>> Encoders >>>"
        # ">>> Object detection >>>"
        # ">>> Ultrasonic Sensors Detect >>>"
        n172 = call "Webcam AE.vi"("Camera states"=Webcam_AE."Retrieve Image") -> ("error out"=w4116:errorcluster, "Image Out"=w4117:T47)  [unwired: 2 in, 1 out]
        n173 = call "Box Colour Detection SubVI.vi"("Image In"=w4117, "Error In"=w4116) -> ("Colour output boolean cluster"=w4114:T49, "Error out"=w4115:errorcluster)  [unwired: 1 out]
        n174 = Unbundle By Name(w4114) -> ("Red"=w4112:bool, "Black"=w4111:bool, "Blue"=w4110:bool, "Yellow"=w4109:bool, "Green"=w4108:bool, "No recognizable coolour"=w4107:bool)
        n175 = Bundle By Name(cluster=w4113, "Red"=w4112, "Black"=w4111, "Blue"=w4110, "Yellow"=w4109, "Green"=w4108, "Unknown"=w4107) -> (w4106:T1)
      }
      frame "DISPOSE CAM BUFFERS" {
        # ">> Item Selection Bias >>"
        # ">>> Line Sensor Cluster>>>"
        # ">>> IR Sensors >>>"
        # ">>State Logic  >>"
        # ">>> Time cluster >>>"
        # ">>> Yaw >>>"
        # ">>> Stepper position >>>"
        # ">>> Encoders >>>"
        # ">>> Object detection >>>"
        # ">>> Ultrasonic Sensors Detect >>>"
        n176 = call "Webcam AE.vi"("Camera states"=Webcam_AE."Dispose Camera Image Buffer") -> ()  [unwired: 2 in, 3 out]
      }
      frame "DISPOSE PROC BUFFERS" {
        # ">>> Box Colour Detection >>>"
        # ">>> Line Sensor Cluster>>>"
        # ">>State Logic  >>"
        # ">>> IR Sensors >>>"
        # ">>> Time cluster >>>"
        # ">>> Object detection >>>"
        # ">>> Yaw >>>"
        # ">>> Ultrasonic Sensors Detect >>>"
        # ">>> Encoders >>>"
        # ">>> Stepper position >>>"
        n177 = call "IMAQ Reference AE.vi"("IMAQ AE States"=IMAQ_Reference_AE."Dispose Processing Buffer") -> ()  [unwired: 1 in, 2 out]
      }
      frame "BOX COLOUR" {
        # ">>> Box Colour Detection >>>"
        # ">>> Line Sensor Cluster>>>"
        # ">>State Logic  >>"
        # ">>> IR Sensors >>>"
        # ">>> Time cluster >>>"
        # ">>> Object detection >>>"
        # ">>> Yaw >>>"
        # ">>> Ultrasonic Sensors Detect >>>"
        # ">>> Encoders >>>"
        # ">>> Stepper position >>>"
        n178 = call "Box Colour Detection Sequence.vi"() -> ("Colour scan time out?"=w4169:bool, "Colour output boolean cluster"=w4171:T49)  [unwired: 9 in, 1 out]
        n179 = Unbundle By Name(w4171) -> ("Red"=w4168:bool, "Black"=w4164:bool, "Blue"=w4161:bool, "Yellow"=w4160:bool, "Green"=w4157:bool, "No recognizable coolour"=w4170:bool)
        n180 = Select(t=Box_Colour_FGV_Colours."Green" ("Colour"), s=w4157, f=Box_Colour_FGV_Colours."None" ("Colour")) -> (s? t:f=w4155:T2)
        n181 = Select(t=Box_Colour_FGV_Colours."Yellow" ("Colour"), s=w4160, f=w4155) -> (s? t:f=w4154:T2)
        n182 = Select(t=Box_Colour_FGV_Colours."Blue" ("Colour"), s=w4161, f=w4154) -> (s? t:f=w4163:T2)
        n183 = Select(t=Box_Colour_FGV_Colours."Black" ("Colour"), s=w4164, f=w4163) -> (s? t:f=w4166:T2)
        n184 = Select(t=Box_Colour_FGV_Colours."Red" ("Colour"), s=w4168, f=w4166) -> (s? t:f=w4153:T2)
        n185 = Bundle By Name(cluster=w4173, "Red"=w4168, "Black"=w4164, "Blue"=w4161, "Yellow"=w4160, "Green"=w4157, "Unknown"=w4170, "Image processing done"=w4169, "Colour"=w4153) -> (w4172:T1)
      }
      frame "-----ARM ACTIONS-----" {
      }
      frame "CLOSE CLAW" {
        n186 = call "Servo State FGV.vi"("Init/Read/Write State"=States_for_Action_Engine."Write", "Servo State"=Servo_States_FGV_Enum."Close claw") -> ()  [unwired: 1 in, 2 out]
      }
      frame "OPEN CLAW" {
        n187 = call "Servo State FGV.vi"("Init/Read/Write State"=States_for_Action_Engine."Write", "Servo State"=Servo_States_FGV_Enum."Open Claw") -> ()  [unwired: 1 in, 2 out]
      }
      frame "Z STEPPER CAM HEIGHT" {
        n188 = call "Arduino Interfacing VI.vi"("Data to Write"=I2C_MASTER_WRITE_NEW_Type_Def."zStepper 6k", "AE Mode"=Arduino_Interfacing."Write to Arduino") -> ()  [unwired: 2 in, 2 out]
      }
      frame "Z STEPPER GRAB HEIGHT" {
        # ">>State Logic  >>"
        # ">>> Time cluster >>>"
        # ">>> Yaw >>>"
        # ">>> Stepper position >>>"
        # ">>> Encoders >>>"
        # ">>> Object detection >>>"
        # ">>> Ultrasonic Sensors Detect >>>"
        n189 = call "Arduino Interfacing VI.vi"("Data to Write"=I2C_MASTER_WRITE_NEW_Type_Def."zStepper 100", "AE Mode"=Arduino_Interfacing."Write to Arduino") -> ()  [unwired: 2 in, 2 out]
      }
      frame "Z STEPPER BOX HEIGHT" {
        # ">>> IR Sensors >>>"
        # ">>> Time cluster >>>"
        # ">>> Yaw >>>"
        # ">>> Stepper position >>>"
        # ">>> Encoders >>>"
        # ">>> Object detection >>>"
        # ">>> Ultrasonic Sensors Detect >>>"
        n190 = call "Arduino Interfacing VI.vi"("Data to Write"=I2C_MASTER_WRITE_NEW_Type_Def."zStepper 5k", "AE Mode"=Arduino_Interfacing."Write to Arduino") -> ()  [unwired: 2 in, 2 out]
      }
      frame "Y STEPPER CONTROL" {
        # ">>State Logic  >>"
        # ">>> yStepper command>>>"
        # ">>> Time cluster >>>"
        # ">>> Yaw >>>"
        # ">>> Stepper position >>>"
        # ">>> Encoders >>>"
        # ">>> Object detection >>>"
        # ">>> Ultrasonic Sensors Detect >>>"
        n191 = Unbundle By Name(w4265) -> ("yStepper desired"=w4264:u8)
        n192 = call "Arduino Interfacing VI.vi"("y Stepper value"=w4264, "Data to Write"=I2C_MASTER_WRITE_NEW_Type_Def."yStepper control", "AE Mode"=Arduino_Interfacing."Write to Arduino") -> ()  [unwired: 1 in, 2 out]
      }
      frame "READ STEPPER VALUES" {
        # ">>State Logic  >>"
        # ">>> Time cluster >>>"
        # ">>> Yaw >>>"
        # ">>> Stepper position >>>"
        # ">>> Encoders >>>"
        # ">>> Object detection >>>"
        # ">>> Ultrasonic Sensors Detect >>>"
        n193 = call "Arduino Interfacing VI.vi"("AE Mode"=Arduino_Interfacing."Read From Arduino") -> ("Arduino Data"=w4283:T17)  [unwired: 3 in, 1 out]
        n194 = Unbundle By Name(w4283) -> ("y Stepper Position"=w4282:u8, "z Stepper Position"=w4281:u8)
        n195 = Bundle By Name(cluster=w4286, "y Stepper Position"=w4282, "z Stepper Position"=w4281) -> (w4285:T7)
      }
      frame " -----TIMING-----" {
        # ">>State Logic  >>"
        # ">>> Time cluster >>>"
        # ">>> Yaw >>>"
        # ">>> Stepper position >>>"
        # ">>> Encoders >>>"
        # ">>> Object detection >>>"
        # ">>> Ultrasonic Sensors Detect >>>"
      }
      frame "SET TIMER 1" {
        w4302 = 1.0 ("Time Setting")
        # ">>State Logic  >>"
        # ">>> Time cluster >>>"
        # ">>> Yaw >>>"
        # ">>> Stepper position >>>"
        # ">>> Encoders >>>"
        # ">>> Object detection >>>"
        # ">>> Ultrasonic Sensors Detect >>>"
        n196 = Wait (ms)(milliseconds to wait=u32 250) -> ()  [unwired: 1 out]
        n197 = call "Elasped Timer.vi"("Time Setting"=w4302, "Action"=Elapsed_timer_control."Initialize") -> ()  [unwired: 6 in, 4 out]
        n198 = Bundle By Name(cluster=w4311, "Time up flag"=FALSE, "SET TIME TO CHECK"=w4302) -> (w4309:T3)
      }
      frame "SET TIMER 2" {
        w4318 = 2.0 ("Time Setting")
        # ">>State Logic  >>"
        # ">>> Time cluster >>>"
        # ">>> Yaw >>>"
        # ">>> Stepper position >>>"
        # ">>> Encoders >>>"
        # ">>> Object detection >>>"
        # ">>> Ultrasonic Sensors Detect >>>"
        n199 = Wait (ms)(milliseconds to wait=u32 250) -> ()  [unwired: 1 out]
        n200 = call "Elasped Timer.vi"("Time Setting"=w4318, "Action"=Elapsed_timer_control."Initialize") -> ()  [unwired: 6 in, 4 out]
        n201 = Bundle By Name(cluster=w4327, "Time up flag"=FALSE, "SET TIME TO CHECK"=w4318) -> (w4325:T3)
      }
      frame "SET TIMER 3" {
        w4334 = 3.0 ("Time Setting")
        # ">>State Logic  >>"
        # ">>> Time cluster >>>"
        # ">>> Yaw >>>"
        # ">>> Stepper position >>>"
        # ">>> Encoders >>>"
        # ">>> Object detection >>>"
        # ">>> Ultrasonic Sensors Detect >>>"
        n202 = Wait (ms)(milliseconds to wait=u32 250) -> ()  [unwired: 1 out]
        n203 = call "Elasped Timer.vi"("Time Setting"=w4334, "Action"=Elapsed_timer_control."Initialize") -> ()  [unwired: 6 in, 4 out]
        n204 = Bundle By Name(cluster=w4343, "Time up flag"=FALSE, "SET TIME TO CHECK"=w4334) -> (w4341:T3)
      }
      frame "SET TIMER 4" {
        w4350 = 4.0 ("Time Setting")
        # ">>State Logic  >>"
        # ">>> Time cluster >>>"
        # ">>> Yaw >>>"
        # ">>> Stepper position >>>"
        # ">>> Encoders >>>"
        # ">>> Object detection >>>"
        # ">>> Ultrasonic Sensors Detect >>>"
        n205 = call "Elasped Timer.vi"("Time Setting"=w4350, "Action"=Elapsed_timer_control."Initialize") -> ()  [unwired: 6 in, 4 out]
        n206 = Wait (ms)(milliseconds to wait=u32 250) -> ()  [unwired: 1 out]
        n207 = Bundle By Name(cluster=w4359, "Time up flag"=FALSE, "SET TIME TO CHECK"=w4350) -> (w4357:T3)
      }
      frame "SET TIMER 5" {
        w4367 = 5.0 ("Time Setting")
        # ">>State Logic  >>"
        # ">>> Time cluster >>>"
        # ">>> Yaw >>>"
        # ">>> Stepper position >>>"
        # ">>> Encoders >>>"
        # ">>> Object detection >>>"
        # ">>> Ultrasonic Sensors Detect >>>"
        n208 = call "Elasped Timer.vi"("Time Setting"=w4367, "Action"=Elapsed_timer_control."Initialize") -> ("Time Out?!"=w4366:bool)  [unwired: 6 in, 3 out]
        n209 = Wait (ms)(milliseconds to wait=u32 250) -> ()  [unwired: 1 out]
        n210 = Bundle By Name(cluster=w4375, "Time up flag"=w4366, "SET TIME TO CHECK"=w4367) -> (w4374:T3)
      }
      frame "START TIMER" {
        # ">>State Logic  >>"
        # ">>> Time cluster >>>"
        # ">>> Yaw >>>"
        # ">>> Stepper position >>>"
        # ">>> Encoders >>>"
        # ">>> Object detection >>>"
        # ">>> Ultrasonic Sensors Detect >>>"
        n211 = call "Elasped Timer.vi"("Action"=Elapsed_timer_control."Start") -> ("Time Out?!"=w4386:bool)  [unwired: 7 in, 3 out]
        n212 = Bundle By Name(cluster=w4389, "Time up flag"=w4386) -> (w4388:T3)
      }
      frame "-----MISC-----" {
        # ">>> Box Colour Detection >>>"
        # ">>> Line Sensor Cluster>>>"
        # ">>> IR Sensors >>>"
        # ">>> Time cluster >>>"
        # ">>> Object detection >>>"
        # ">>> Yaw >>>"
        # ">>> Ultrasonic Sensors Detect >>>"
        # ">>> Encoders >>>"
        # ">>> Stepper position >>>"
      }
      frame "Task 9" {
        # ">>> Box Colour Detection >>>"
        # ">>> Line Sensor Cluster>>>"
        # ">>> IR Sensors >>>"
        # ">>> Time cluster >>>"
        # ">>> Object detection >>>"
        # ">>> Yaw >>>"
        # ">>> Ultrasonic Sensors Detect >>>"
        # ">>> Encoders >>>"
        # ">>> Stepper position >>>"
        n213 = call "Colour Processing Test Env.vi"() -> ("Colour scan time out?"=w4415:bool, "Colour output boolean cluster"=w4413:T49)  [unwired: 10 in]
        n214 = Unbundle By Name(w4413) -> ("Red"=w4407:bool, "Black"=w4408:bool, "Blue"=w4409:bool, "Yellow"=w4410:bool, "Green"=w4411:bool, "No recognizable coolour"=w4412:bool)
        n215 = Bundle By Name(cluster=w4417, "Red"=w4407, "Black"=w4408, "Blue"=w4409, "Yellow"=w4410, "Green"=w4411, "Unknown"=w4412, "Image processing done"=w4415) -> (w4416:T1)
      }
    }
    "State Logic" <- w267
    "Image Processing Error" <- w235
    n216 = call "Task Enable FGV.vi"("Init/Read/Write State"=States_for_Action_Engine."Read") -> ("Output node"=w222:bool)  [unwired: 9 in, 1 out]
    n217 = Not(x=w222) -> (.not. x?=w261:bool)
    n218 = case shown="True" w268 {
      tunnel: w226 -> [w299 w353]
      tunnel: w275 -> [w295 w355]
      tunnel: [w299 w353] -> w280
      tunnel: [w295 w356] -> w279
      tunnel: w276 -> [_ w351]
      tunnel: w278 -> [_ w352]
      tunnel: w273 -> [w298 w358]
      tunnel: [w298 w358] -> w272
      tunnel: "STOP TASK" -> [_ w341]
      tunnel: w267 -> [w297 w357]
      tunnel: [w297 w354] -> w266
      tunnel: w263 -> [w296 w347]
      tunnel: [w296 w347] -> w262
      tunnel: w261 -> [_ w342]
      tunnel: [w294 w339] -> w260
      tunnel: w259 -> [w294 w338]
      tunnel: w257 -> [w293 w335]
      tunnel: [w293 w335] -> w256
      tunnel: w254 -> [w292 w331]
      tunnel: [w292 w331] -> w253
      tunnel: w251 -> [w291 w329]
      tunnel: [w291 w329] -> w250
      tunnel: w248 -> [w290 w327]
      tunnel: [w290 w327] -> w247
      tunnel: w246 -> [w289 w326]
      tunnel: [w289 w325] -> w245
      tunnel: [_ w323] -> w244
      tunnel: w242 -> [w288 w321]
      tunnel: [w288 w321] -> w241
      tunnel: w240 -> [w287 w320]
      tunnel: [w287 w319] -> w239
      tunnel: w237 -> [w286 w316]
      tunnel: [w286 w316] -> w236
      tunnel: [w285 w315] -> w234
      tunnel: w232 -> [w285 w314]
      tunnel: [_ w312] -> w231
      tunnel: [_ w311] -> w230
      tunnel: [_ w310] -> w229
      tunnel: w227 -> [w284 w309]
      tunnel: [w284 w309] -> w225
      tunnel: [_ w300] -> w224
      frame False {
        # ">>> Box Colour Detection >>>"
        # ">>> Line Sensor Cluster>>>"
        # ">> Item Selection Bias >>"
        # ">>State Logic Queue Reference >>"
        # ">>Action states Queue Reference >>"
        # ">>True Stop Next State >>"
        # ">>State Logic  >>"
        # ">>> IR Sensors >>>"
        # ">>> Line Sensor Cluster>>>"
        # ">>> Line Sensor Cluster>>>"
        # ">>> Motor control cluster >>>"
        # ">>> yStepper command>>>"
        # ">>> Motor control cluster >>>"
        # ">>> yStepper command>>>"
        # ">>> Motor control cluster >>>"
        # ">>> IR Sensors >>>"
        # ">>> IR Sensors >>>"
        # ">>> yStepper command>>>"
        # ">>> Time cluster >>>"
        # ">>> Yaw >>>"
        # ">>> Stepper position >>>"
        # ">>> Encoders >>>"
        # ">>> Object detection >>>"
        # ">>> Ultrasonic Sensors Detect >>>"
        # ">>> Time cluster >>>"
        # ">>> Yaw >>>"
        # ">>> Stepper position >>>"
        # ">>> Encoders >>>"
        # ">>> Object detection >>>"
        # ">>> Ultrasonic Sensors Detect >>>"
      }
      frame True {
        # ">>> Box colour cluster >>>"
        # ">>State Logic Queue Reference >>"
        # ">>> Box Colour Detection >>>"
        # ">> Item Selection Bias >>"
        # ">>> IR Sensors >>>"
        # ">>> Line Sensor Cluster>>>"
        # ">>> Line Sensor Cluster>>>"
        # ">>> Motor control cluster >>>"
        # ">>> yStepper command>>>"
        # ">>> IR Sensors >>>"
        # ">>> Motor control cluster >>>"
        # ">>State Logic Queue Reference >>"
        # ">>Timeout>>"
        # ">>> yStepper command>>>"
        # ">>> Time cluster >>>"
        # ">>> Object detection >>>"
        # ">>> Yaw >>>"
        # ">>> Ultrasonic Sensors Detect >>>"
        # ">>> Encoders >>>"
        # ">>> Stepper position >>>"
        # ">>State Logic  >>"
        # ">>True Stop Next State >>"
        # ">>Action Queue>>"
        # ">> Manual override >>"
        # ">>> Time cluster >>>"
        # ">>> Yaw >>>"
        # ">>> Stepper position >>>"
        # ">>> Encoders >>>"
        # ">>> Object detection >>>"
        # ">>> Ultrasonic Sensors Detect >>>"
        # ">>Action Queue>>"
        # ">>State Logic Queue Reference >>"
        n219 = Or(x=w341, y=w342) -> (x .or. y?=w340:bool)
        n220 = Unbundle By Name(w309) -> ("Red"=w308:bool, "Black"=w307:bool, "Blue"=w306:bool, "Yellow"=w305:bool, "Green"=w304:bool, "Unknown"=w303:bool, "Image processing done"=w302:bool, "Colour"=w301:T2)
        n221 = Unbundle By Name(w316) -> ("Line Detected?"=w317:bool)
        n222 = Unbundle By Name(w321) -> ("Left IR Sensor"=w322:dbl, "Arm IR Sensor"=w318:dbl, "Bottom IR Sensor"=w313:dbl)
        n223 = Unbundle By Name(w327) -> ("Time up flag"=w328:bool)
        n224 = Unbundle By Name(w329) -> ("Yaw"=w330:dbl, "Compass"=w324:dbl)
        n225 = Unbundle By Name(w331) -> ("y Stepper Position"=w333:u8, "z Stepper Position"=w332:u8)
        n226 = Unbundle By Name(w347) -> ("xDistance"=w344:dbl, "yDistance"=w345:dbl, "wDistance"=w346:dbl)
        n227 = Unbundle By Name(w335) -> ("Recognized Object"=w334:bool, "Object X coordinate"=w337:dbl, "Object Y coordinate"=w336:dbl)
        n228 = Unbundle By Name(w358) -> ("PING_A"=w350:u8, "PING_B"=w349:u8, "PING_C"=w348:u8, "PING_D"=w343:u8)
        n229 = case shown="\"Task 8H: ARM ADJUST\"" w357 {
          tunnel: [w363 w375 w385 w393 w404 w514 w531 w577 w615 w669 w711 w760 w803 w858 w906 w950 w1010 w1051 w1094 w1143 w1183 w1236 w1274 w1326 w1372 w1418 w1459 w1508 w1552 w1598 w1639 w1688 w1732 w1778 w1819 w1868 w1912 w1958 w1999 w2048 w2083 w2101 w2149 w2190 w2240 w2297 w2336 w2385 w2429 w2484 w2522 w2574 w2617 w2662 w2697 w2745 w2788 w2838 w2882 w2935 w2976 w3032 w3073 w3125 w3173 w3218 w3262 w3310 w3361 w3404 w3463 w3500 w3504 w3508 w3512] -> w356
          tunnel: w355 -> [w363 w378 w385 w394 w407 w516 w532 w578 w624 w667 w715 w761 w809 w851 w909 w957 w1000 w1054 w1100 w1142 w1186 w1226 w1280 w1316 w1367 w1410 w1458 w1507 w1551 w1590 w1638 w1687 w1731 w1770 w1818 w1867 w1911 w1950 w1998 w2047 w2083 w2091 w2152 w2196 w2239 w2296 w2342 w2384 w2432 w2474 w2528 w2564 w2610 w2655 w2701 w2752 w2793 w2843 w2888 w2933 w2977 w3030 w3074 w3126 w3175 w3224 w3269 w3315 w3360 w3400 w3461 w3500 w3504 w3508 w3512]
          tunnel: [State_Type_Definitions,_for_0.26g_versions_and_later_3."Idle" ("Enum") State_Type_Definitions,_for_0.26g_versions_and_later_3."Idle" ("Enum") _ w389 w406 State_Type_Definitions,_for_0.26g_versions_and_later_3."Shutdown" ("Enum") w533 w579 w622 w670 w712 w759 w804 w857 w907 w952 w1009 w1052 w1101 w1144 w1185 w1235 w1281 w1325 w1373 w1411 w1460 w1509 w1553 w1591 w1640 w1689 w1733 w1771 w1820 w1869 w1913 w1951 w2000 w2049 State_Type_Definitions,_for_0.26g_versions_and_later_3."Idle" ("Enum") w2100 w2150 w2197 w2241 w2298 w2343 w2386 w2431 w2483 w2529 w2573 w2616 w2661 w2698 w2746 w2789 w2839 w2881 w2936 w2975 w3033 w3072 w3124 w3174 w3217 w3264 w3316 w3362 w3403 w3464 _ _ _ _] -> w354
          tunnel: w353 -> [_ _ _ w392 w410 _ w537 w584 w618 w666 w716 w767 w808 w855 w910 w956 w1007 w1049 w1099 w1140 w1187 w1233 w1279 w1323 w1370 w1417 w1456 w1505 w1549 w1597 w1636 w1685 w1729 w1777 w1816 w1865 w1909 w1957 w1996 w2045 _ w2098 w2147 w2195 w2237 w2294 w2341 w2382 w2433 w2481 w2527 w2571 w2614 w2659 w2705 w2751 w2796 w2846 w2887 w2932 w2985 w3029 w3075 w3119 w3176 w3223 w3268 w3314 w3359 w3409 w3460 _ _ _ _]
          tunnel: w352 -> [_ _ _ _ w409 _ w536 w583 w617 w665 w717 w766 w807 w854 w903 w955 w1006 w1048 w1098 w1139 w1188 w1232 w1278 w1322 w1369 w1415 w1455 w1504 w1548 w1595 w1635 w1684 w1728 w1775 w1815 w1864 w1908 w1955 w1995 w2044 _ w2097 w2146 w2194 w2236 w2293 w2340 w2381 w2434 w2480 w2526 w2570 w2613 w2658 w2700 w2750 w2795 w2845 w2886 w2931 w2983 w3028 w3076 w3120 w3177 w3222 w3267 w3313 w3358 w3408 w3459 _ _ _ _]
          tunnel: w351 -> [_ _ _ w391 w405 _ w535 w582 w616 w664 w718 w765 w806 w853 w902 w954 w1008 w1050 w1097 w1138 w1189 w1234 w1277 w1324 w1368 w1416 w1454 w1503 w1547 w1596 w1634 w1683 w1727 w1776 w1814 w1863 w1907 w1956 w1994 w2043 _ w2099 w2148 w2193 w2235 w2292 w2339 w2380 w2435 w2482 w2525 w2572 w2615 w2660 w2704 w2749 w2794 w2844 w2885 w2930 w2984 w3027 w3077 w3121 w3178 w3221 w3266 w3312 w3357 w3407 w3458 _ _ _ _]
          tunnel: w340 -> [_ _ _ _ _ _ w522 w576 w623 w663 w719 w762 w802 w856 w908 w958 w1001 w1055 w1095 w1141 w1190 w1227 w1275 w1317 w1371 w1413 w1457 w1506 w1550 w1593 w1637 w1686 w1730 w1773 w1817 w1866 w1910 w1953 w1997 w2046 _ w2092 w2153 w2191 w2238 w2295 w2337 w2383 w2436 w2475 w2523 w2565 w2611 w2656 w2703 w2744 w2792 w2842 w2884 w2929 w2979 w3026 w3078 w3122 w3179 w3220 w3265 w3311 w3356 w3406 w3457 _ _ _ _]
          tunnel: w350 -> [_ _ _ _ _ _ _ _ _ _ _ _ _ _ _ _ _ _ _ _ _ _ _ _ _ _ _ _ _ _ _ _ _ _ _ _ _ _ _ _ _ _ _ _ _ _ _ _ _ _ _ _ _ _ _ _ _ _ _ _ _ _ _ _ _ _ _ _ _ _ _ _ _ _ _]
          tunnel: w349 -> [_ _ _ _ _ _ _ _ _ w662 _ _ _ w847 w891 w948 _ _ _ _ _ _ _ _ _ _ _ _ _ _ _ _ _ _ _ _ _ _ _ _ _ _ w2139 _ _ _ _ _ _ _ _ _ _ _ _ _ _ _ _ _ _ _ _ _ _ _ _ _ _ _ _ _ _ _ _]
          tunnel: w348 -> [_ _ _ _ _ _ _ _ _ w661 _ _ _ w848 w892 w949 _ _ _ _ _ _ _ _ _ _ _ _ _ _ _ _ _ _ _ _ _ _ _ _ _ _ w2140 _ _ _ _ _ _ _ _ _ _ _ _ _ _ _ _ _ _ _ _ _ _ _ _ _ _ _ _ _ _ _ _]
          tunnel: w346 -> [_ _ _ _ _ _ _ _ _ _ _ w764 _ _ _ _ _ _ _ _ _ _ _ _ _ _ _ _ _ _ _ _ _ _ _ _ _ _ _ _ _ _ _ _ _ _ _ _ _ _ _ _ _ _ _ _ _ _ _ _ _ _ _ w3118 _ _ _ _ _ _ _ _ _ _ _]
          tunnel: w345 -> [_ _ _ _ _ _ w530 w575 _ _ w710 _ _ _ _ w953 _ _ _ _ _ _ _ _ _ _ _ _ _ _ _ _ _ _ _ w1856 _ _ _ w2036 _ _ _ _ _ _ _ _ _ _ _ _ _ _ _ _ _ _ _ _ _ _ _ _ _ _ _ _ _ _ _ _ _ _ _]
          tunnel: w344 -> [_ _ _ _ _ _ _ _ _ _ _ _ _ _ w897 _ _ _ _ _ _ _ _ _ _ _ _ w1496 _ _ _ w1676 _ _ _ _ _ _ _ _ _ _ _ _ _ w2283 _ _ _ _ _ _ _ w2648 _ _ _ _ _ _ _ w3019 _ _ _ _ _ _ _ _ w3450 _ _ _ _]
          tunnel: w343 -> [_ _ _ _ _ _ _ _ _ _ _ _ _ _ _ _ _ _ _ _ _ _ _ _ _ _ _ _ _ _ _ _ _ _ _ _ _ _ _ _ _ _ _ _ _ _ _ _ _ _ _ _ _ _ _ _ _ _ _ _ _ _ _ _ _ _ _ _ _ _ _ _ _ _ _]
          tunnel: [State_Type_Definitions,_for_0.26g_versions_and_later_3."Idle" ("Enum") State_Type_Definitions,_for_0.26g_versions_and_later_3."Idle" ("Enum") _ State_Type_Definitions,_for_0.26g_versions_and_later_3."Idle" ("Enum") State_Type_Definitions,_for_0.26g_versions_and_later_3."Idle" ("Enum") State_Type_Definitions,_for_0.26g_versions_and_later_3."Shutdown" ("Enum") w528 w573 w621 w668 w713 w756 w801 w850 w905 w951 w1011 w1053 w1093 w1145 w1184 w1237 w1273 w1327 w1374 w1412 w1461 w1510 w1554 w1592 w1641 w1690 w1734 w1772 w1821 w1870 w1914 w1952 w2001 w2050 w2085 w2102 w2151 w2189 w2242 w2299 w2335 w2387 w2430 w2485 w2521 w2575 w2618 w2663 w2699 w2747 w2791 w2841 w2880 w2934 w2974 w3031 w3071 w3123 w3172 w3216 w3263 w3317 w3363 w3402 w3462 _ _ _ _] -> w339
          tunnel: w338 -> [_ _ _ w389 _ _ _ _ _ _ _ _ _ _ _ _ _ _ _ _ _ _ _ _ _ _ _ _ _ _ _ _ _ _ _ _ _ _ _ _ w2085 _ _ _ _ _ _ _ _ _ _ _ _ _ _ _ _ _ _ _ _ _ _ _ _ _ _ _ _ _ _ _ _ _ _]
          tunnel: w334 -> [_ _ _ _ _ _ _ _ _ _ _ _ _ _ _ _ _ _ _ _ _ _ _ _ _ _ w1448 _ _ _ w1628 _ _ _ w1808 _ _ _ w1988 _ _ _ _ _ w2230 _ _ _ w2419 _ _ _ _ _ _ _ _ _ _ _ _ _ _ _ _ _ _ _ _ _ _ _ _ _ _]
          tunnel: w337 -> [_ _ _ _ _ _ _ _ _ _ _ _ _ _ _ _ _ _ _ _ _ _ _ _ _ _ _ _ _ _ _ _ _ _ _ _ _ _ _ _ _ _ _ _ _ w2289 _ _ _ _ _ _ _ _ _ _ _ _ _ _ _ _ _ _ _ _ _ _ _ _ _ _ _ _ _]
          tunnel: w336 -> [_ _ _ _ _ _ _ _ _ _ _ _ _ _ _ _ _ _ _ _ _ _ _ _ _ _ _ _ _ _ _ _ _ _ _ _ _ _ _ _ _ _ _ _ _ _ _ _ w2425 _ _ _ _ _ _ _ _ _ _ _ _ _ _ _ _ _ _ _ _ _ _ _ _ _ _]
          tunnel: w333 -> [_ _ _ _ _ _ _ _ _ _ _ _ _ _ _ _ _ _ _ _ _ _ _ _ _ _ _ _ _ _ _ _ _ _ _ _ _ _ _ _ _ _ _ _ _ _ _ _ w2424 _ _ _ _ _ _ _ _ _ _ _ _ _ _ _ _ _ _ _ _ _ _ _ _ _ _]
          tunnel: w332 -> [_ _ _ _ _ _ _ _ w620 _ _ _ w799 _ _ _ w1004 _ w1089 _ w1179 w1230 _ w1320 w1366 _ _ _ _ _ _ _ _ _ _ _ _ _ _ _ _ w2095 _ _ _ _ _ _ _ w2478 _ w2568 _ _ w2702 _ _ _ _ _ _ _ _ _ _ _ _ _ _ _ _ _ _ _ _]
          tunnel: w330 -> [_ _ _ _ _ _ _ _ _ _ _ _ _ _ _ _ _ _ _ _ _ _ _ _ _ _ _ _ _ _ _ _ _ _ _ _ _ _ _ _ _ _ _ _ _ _ _ _ _ _ _ _ _ _ _ _ _ _ _ _ _ _ _ _ _ _ _ _ _ _ _ _ _ _ _]
          tunnel: w328 -> [_ _ _ _ _ _ _ _ _ _ _ _ _ _ _ _ _ _ _ w1135 _ _ w1271 _ _ w1406 w1449 _ _ w1586 w1629 _ _ w1766 w1809 _ _ w1946 w1989 _ _ _ _ w2187 w2229 _ w2333 w2377 _ _ w2519 _ _ _ _ _ _ _ _ _ _ _ _ _ _ _ _ _ _ _ _ _ _ _ _]
          tunnel: w326 -> [w361 w373 w384 w388 w402 w512 w527 w572 w619 w660 w714 w755 w800 w849 w901 w947 w999 w1046 w1092 w1136 w1180 w1225 w1272 w1315 w1364 w1409 w1452 w1501 w1545 w1589 w1632 w1681 w1725 w1769 w1812 w1861 w1905 w1949 w1992 w2041 w2086 w2090 w2144 w2188 w2233 w2290 w2334 w2378 w2427 w2473 w2520 w2563 w2609 w2654 w2696 w2748 w2790 w2840 w2892 w2928 w2982 w3025 w3080 w3128 w3181 w3228 w3271 w3319 w3365 w3414 w3456 w3499 w3503 w3507 w3511]
          tunnel: [w361 w372 w384 w388 w402 w512 w527 w572 w619 w660 w714 w755 w800 w849 w901 w947 w999 w1046 w1092 w1136 w1180 w1225 w1272 w1315 w1364 w1409 w1452 w1501 w1545 w1589 w1632 w1681 w1725 w1769 w1812 w1861 w1905 w1949 w1992 w2041 w2086 w2090 w2144 w2188 w2233 w2290 w2334 w2378 w2426 w2473 w2520 w2563 w2609 w2654 w2696 w2748 w2790 w2840 w2892 w2928 w2982 w3025 w3080 w3128 w3181 w3228 w3271 w3319 w3365 w3414 w3456 w3499 w3503 w3507 w3511] -> w325
          tunnel: w324 -> [_ _ _ _ _ _ _ _ _ _ _ _ _ _ _ _ _ _ _ _ _ _ _ _ _ _ _ _ _ _ _ _ _ _ _ _ _ _ _ _ _ _ _ _ _ _ _ _ _ _ _ _ _ _ _ w2743 _ _ _ _ _ _ _ _ _ _ _ _ _ _ _ _ _ _ _]
          tunnel: [_ _ _ _ TRUE _ w521 w569 w612 w657 w706 w752 w795 _ _ _ _ _ _ _ _ _ _ _ w1360 _ w1449 _ _ _ w1629 _ _ _ w1809 _ _ _ w1989 _ _ _ _ _ w2229 w2279 _ _ _ _ _ _ _ _ w2693 w2738 w2785 w2829 _ w2925 w2969 w3018 w3066 w3116 w3163 _ _ _ w3355 w3399 w3449 _ _ _ _] -> w323
          tunnel: w322 -> [_ _ _ _ _ _ _ _ _ _ _ _ _ _ _ _ _ _ _ _ _ _ _ _ _ _ _ _ _ _ _ _ _ _ _ _ _ _ _ _ _ _ _ _ _ _ _ _ _ _ _ _ _ _ _ _ _ _ w2879 _ _ _ _ _ _ w3215 _ _ _ _ _ _ _ _ _]
          tunnel: w320 -> [w360 w370 w383 w387 w400 w511 w526 w571 w614 w659 w708 w754 w797 w842 w890 w946 w998 w1045 w1091 w1134 w1182 w1224 w1270 w1314 w1363 w1408 w1451 w1500 w1544 w1588 w1631 w1680 w1724 w1768 w1811 w1860 w1904 w1948 w1991 w2040 w2087 w2089 w2138 w2186 w2232 w2286 w2332 w2376 w2421 w2472 w2518 w2562 w2608 w2653 w2695 w2740 w2787 w2837 w2893 w2927 w2981 w3024 w3082 w3130 w3183 w3229 w3273 w3321 w3367 w3415 w3455 w3498 w3502 w3506 w3510]
          tunnel: [w360 w369 w383 w387 w400 w511 w526 w571 w614 w659 w708 w754 w797 w842 w890 w946 w998 w1045 w1091 w1134 w1182 w1224 w1270 w1314 w1363 w1408 w1451 w1500 w1544 w1588 w1631 w1680 w1724 w1768 w1811 w1860 w1904 w1948 w1991 w2040 w2087 w2089 w2138 w2186 w2232 w2285 w2332 w2376 w2421 w2472 w2518 w2562 w2608 w2653 w2695 w2740 w2787 w2837 w2893 w2927 w2981 w3024 w3082 w3130 w3183 w3229 w3273 w3321 w3367 w3415 w3455 w3498 w3502 w3506 w3510] -> w319
          tunnel: w318 -> [_ _ _ _ _ _ _ _ _ _ _ _ _ _ _ _ _ _ _ _ _ _ _ _ _ _ _ _ _ _ _ _ _ _ _ _ _ _ _ _ _ _ _ _ _ _ _ _ _ _ _ _ _ _ _ _ _ w2835 _ _ _ _ _ _ w3170 _ _ _ _ _ _ _ _ _ _]
          tunnel: w317 -> [_ _ _ _ _ _ w523 _ _ _ _ _ _ _ _ w944 _ _ _ _ _ _ _ _ _ _ _ _ _ _ _ _ _ _ _ _ _ _ _ _ _ _ _ _ _ _ _ _ _ _ _ _ _ _ _ _ w2785 _ _ w2925 _ w3020 _ _ _ _ w3261 _ w3355 _ w3451 _ _ _ _]
          tunnel: [w359 w365 w382 w386 w399 w510 w525 w570 w613 w658 w707 w753 w796 w841 w889 w945 w997 w1044 w1090 w1133 w1181 w1223 w1269 w1313 w1362 enum16{"Ball", "Soap", "Gel", "Pipe", "None"}."Ball" ("Object recognition mode") w1450 w1499 enum16{"Ball", "Soap", "Gel", "Pipe", "None"}."Soap" ("Object recognition mode") enum16{"Ball", "Soap", "Gel", "Pipe", "None"}."Soap" ("Object recognition mode") w1630 w1679 enum16{"Ball", "Soap", "Gel", "Pipe", "None"}."Gel" ("Object recognition mode") enum16{"Ball", "Soap", "Gel", "Pipe", "None"}."Gel" ("Object recognition mode") w1810 w1859 enum16{"Ball", "Soap", "Gel", "Pipe", "None"}."Pipe" ("Object recognition mode") enum16{"Ball", "Soap", "Gel", "Pipe", "None"}."Pipe" ("Object recognition mode") w1990 w2039 w2082 w2088 w2137 w2185 w2231 w2280 w2331 w2375 w2420 w2471 w2517 w2561 w2607 w2652 w2694 w2739 w2786 w2834 w2883 w2926 w2980 w3023 w3081 w3129 w3182 w3219 w3272 w3320 w3366 w3405 w3454 w3497 w3501 w3505 w3509] -> w315
          tunnel: w314 -> [w359 w365 w382 w386 _ w510 w525 w570 w613 w658 w707 w753 w796 w841 w889 w945 w997 w1044 w1090 w1133 w1181 w1223 w1269 w1313 w1362 _ w1450 w1499 _ _ w1630 w1679 _ _ w1810 w1859 _ _ w1990 w2039 w2082 w2088 w2137 w2185 w2231 w2280 w2331 w2375 w2420 w2471 w2517 w2561 w2607 w2652 w2694 w2739 w2786 w2834 w2883 w2926 w2980 w3023 w3081 w3129 w3182 w3219 w3272 w3320 w3366 w3405 w3454 w3497 w3501 w3505 w3509]
          tunnel: w313 -> [_ _ _ _ _ _ _ _ _ _ _ _ _ _ _ _ _ _ _ _ _ _ _ _ _ _ _ _ _ _ _ _ _ _ _ _ _ _ _ _ _ _ w2136 _ _ _ _ _ _ _ _ _ _ _ _ _ _ w2833 _ _ _ _ _ _ w3164 _ _ _ _ _ _ _ _ _ _]
          tunnel: [_ _ _ _ _ _ _ _ _ w657 _ _ _ _ _ _ _ _ _ _ _ _ _ _ _ _ _ _ _ _ _ _ _ _ _ _ _ _ _ _ _ _ _ _ _ _ _ _ _ _ _ _ _ _ _ _ _ _ _ _ _ _ _ _ _ _ _ _ _ _ _ _ _ _ _] -> w312
          tunnel: [_ _ _ _ _ _ _ _ _ _ _ _ _ _ _ _ _ _ _ _ _ _ _ _ _ _ _ _ _ _ _ _ _ _ _ _ _ _ _ _ _ _ _ _ _ _ _ _ _ _ _ _ _ _ _ _ _ w2831 _ _ _ _ _ _ w3162 _ _ _ _ _ _ _ _ _ _] -> w311
          tunnel: [_ _ _ _ _ _ _ _ _ _ _ _ _ _ _ _ _ _ _ _ _ _ _ _ _ _ _ _ _ _ _ _ _ _ _ _ _ _ _ _ _ _ _ _ _ _ _ _ _ _ _ _ _ _ _ _ _ w2830 _ _ _ _ _ _ w3162 _ _ _ _ _ _ _ _ _ _] -> w310
          tunnel: w308 -> [_ _ _ _ _ _ _ _ _ _ _ _ _ _ _ _ _ _ _ _ _ _ _ _ _ _ _ _ _ _ _ _ _ _ _ _ _ _ _ _ _ _ _ _ _ _ _ _ _ _ _ _ _ _ _ _ _ _ _ _ _ _ _ _ _ _ _ _ _ _ _ _ _ _ _]
          tunnel: w307 -> [_ _ _ _ _ _ _ _ _ _ _ _ _ _ _ _ _ _ _ _ _ _ _ _ _ _ _ _ _ _ _ _ _ _ _ _ _ _ _ _ _ _ _ _ _ _ _ _ _ _ _ _ _ _ _ _ _ _ _ _ _ _ _ _ _ _ _ _ _ _ _ _ _ _ _]
          tunnel: w306 -> [_ _ _ _ _ _ _ _ _ _ _ _ _ _ _ _ _ _ _ _ _ _ _ _ _ _ _ _ _ _ _ _ _ _ _ _ _ _ _ _ _ _ _ _ _ _ _ _ _ _ _ _ _ _ _ _ _ _ _ _ _ _ _ _ _ _ _ _ _ _ _ _ _ _ _]
          tunnel: w305 -> [_ _ _ _ _ _ _ _ _ _ _ _ _ _ _ _ _ _ _ _ _ _ _ _ _ _ _ _ _ _ _ _ _ _ _ _ _ _ _ _ _ _ _ _ _ _ _ _ _ _ _ _ _ _ _ _ _ _ _ _ _ _ _ _ _ _ _ _ _ _ _ _ _ _ _]
          tunnel: w304 -> [_ _ _ _ _ _ _ _ _ _ _ _ _ _ _ _ _ _ _ _ _ _ _ _ _ _ _ _ _ _ _ _ _ _ _ _ _ _ _ _ _ _ _ _ _ _ _ _ _ _ _ _ _ _ _ _ _ _ _ _ _ _ _ _ _ _ _ _ _ _ _ _ _ _ _]
          tunnel: w303 -> [_ _ _ _ _ _ _ _ _ _ _ _ _ _ _ _ _ _ _ _ _ _ _ _ _ _ _ _ _ _ _ _ _ _ _ _ _ _ _ _ _ _ _ _ _ _ _ _ _ _ _ _ _ _ _ _ _ _ _ _ _ _ _ _ _ _ _ _ _ _ _ _ _ _ _]
          tunnel: w302 -> [_ _ _ _ _ _ _ _ _ _ _ _ _ _ _ _ _ _ _ _ _ _ _ _ _ _ _ _ _ _ _ _ _ _ _ _ _ _ _ _ _ _ _ _ _ _ _ _ _ _ _ _ _ _ _ _ _ _ _ _ w2969 _ w3066 _ _ _ _ w3305 _ w3399 _ _ _ _ _]
          tunnel: w301 -> [_ _ _ _ _ _ _ _ _ _ _ _ _ _ _ _ _ _ _ _ _ _ _ _ _ _ _ _ _ _ _ _ _ _ _ _ _ _ _ _ _ _ _ _ _ _ _ _ _ _ _ _ _ _ _ _ _ _ _ _ w2972 _ w3068 _ _ _ _ w3307 _ w3401 _ _ _ _ _]
          tunnel: [_ _ _ _ _ _ _ _ _ _ _ _ _ _ _ _ _ _ _ _ _ _ _ _ _ _ _ _ _ _ _ _ _ _ _ _ _ _ _ _ _ _ _ _ _ _ _ _ _ _ _ _ _ _ _ _ _ _ _ _ w2970 _ w3067 _ _ _ _ _ _ _ _ _ _ _ _] -> w300
          frame "None" {
            # ">>> Motor control cluster >>>"
            # ">>> yStepper command>>>"
          }
          frame "Startup" {
            # ">>> yStepper command>>>"
            n230 = for {
              shift-right: [w381] -> w375
              shift-left: w378 -> [w380]
              tunnel: string[] ["INIT", "RESET ARM", "RESET FLAGS", "RESET YAW", "NAVX CALIBRATE"] -> [w379] mode=indexing
              n231 = Enqueue Element(queue=w380, element=w379) -> (queue out=w381:refnum<queue>)  [unwired: 2 in, 2 out]
            }
            n232 = Bundle By Name(cluster=w373, "yStepper desired"=u8 0) -> (w372:T21)
            n233 = Bundle By Name(cluster=w370, "ySpeed"=0.0, "xSpeed"=0.0, "wSpeed"=0.0) -> (w369:T20)
          }
          frame "Move to Angle" {
          }
          frame "True Stop" {
            # ">>Action Queue>>"
            # ">>> Motor control cluster >>>"
            # ">>> yStepper command>>>"
            n234 = Flush Queue(queue=w392, error in (no error)=w391) -> ()  [unwired: 3 out]
            n235 = for {
              shift-right: [w398] -> w393
              shift-left: w394 -> [w397]
              tunnel: string[] ["STOP", "RESET ENCODERS", "RESET YAW", "RESET ARM", "RESET ALL SENSORS", "DISPOSE CAM BUFFERS", "DISPOSE PROC BUFFERS", "CAM CLOSE", ""] -> [w396] mode=indexing
              n236 = Enqueue Element(queue=w397, element=w396) -> (queue out=w398:refnum<queue>)  [unwired: 2 in, 2 out]
            }
          }
          frame "Idle", Default {
            # ">>> Motor control cluster >>>"
            # ">>> yStepper command>>>"
            n237 = Dequeue Element(queue=w410, timeout in ms (-1)=w409, error in (no error)=w405) -> (element=w408:T10)  [unwired: 3 out]
            n238 = case shown="\"None\", Default" w408 {
              tunnel: [w413 w421 w429 w437 w445 w453 w461 w469 w477 w484 w494 w501 w504] -> w404
              tunnel: w407 -> [w414 w422 w430 w438 w446 w454 w462 w470 w478 w485 w493 w501 w505]
              tunnel: [State_Type_Definitions,_for_0.26g_versions_and_later_3."Task 1A" ("Enum") State_Type_Definitions,_for_0.26g_versions_and_later_3."Task 2:Raise Arm" ("Enum") State_Type_Definitions,_for_0.26g_versions_and_later_3."Task 3" ("Enum") State_Type_Definitions,_for_0.26g_versions_and_later_3."Task 4_A" ("Enum") State_Type_Definitions,_for_0.26g_versions_and_later_3."Task 5A: RAISING ARM" ("Enum") State_Type_Definitions,_for_0.26g_versions_and_later_3."Task 6A: RAISE ARM" ("Enum") State_Type_Definitions,_for_0.26g_versions_and_later_3."Task 8A: RAISE ARM" ("Enum") State_Type_Definitions,_for_0.26g_versions_and_later_3."Task 8A: RAISE ARM" ("Enum") State_Type_Definitions,_for_0.26g_versions_and_later_3."Task 8A: RAISE ARM" ("Enum") State_Type_Definitions,_for_0.26g_versions_and_later_3."Task 8A: RAISE ARM" ("Enum") State_Type_Definitions,_for_0.26g_versions_and_later_3."Task 9A: Raise Arm" ("Enum") State_Type_Definitions,_for_0.26g_versions_and_later_3."Idle" ("Enum") State_Type_Definitions,_for_0.26g_versions_and_later_3."Shutdown" ("Enum")] -> w406
              tunnel: [enum16{"Ball", "Soap", "Gel", "Pipe", "None"}."None" ("Object recognition mode") enum16{"Ball", "Soap", "Gel", "Pipe", "None"}."None" ("Object recognition mode") enum16{"Ball", "Soap", "Gel", "Pipe", "None"}."None" ("Object recognition mode") enum16{"Ball", "Soap", "Gel", "Pipe", "None"}."None" ("Object recognition mode") enum16{"Ball", "Soap", "Gel", "Pipe", "None"}."None" ("Object recognition mode") enum16{"Ball", "Soap", "Gel", "Pipe", "None"}."None" ("Object recognition mode") enum16{"Ball", "Soap", "Gel", "Pipe", "None"}."Ball" ("Object recognition mode") enum16{"Ball", "Soap", "Gel", "Pipe", "None"}."Gel" ("Object recognition mode") enum16{"Ball", "Soap", "Gel", "Pipe", "None"}."Pipe" ("Object recognition mode") enum16{"Ball", "Soap", "Gel", "Pipe", "None"}."Soap" ("Object recognition mode") enum16{"Ball", "Soap", "Gel", "Pipe", "None"}."None" ("Object recognition mode") enum16{"Ball", "Soap", "Gel", "Pipe", "None"}."None" ("Object recognition mode") enum16{"Ball", "Soap", "Gel", "Pipe", "None"}."None" ("Object recognition mode")] -> w399
              frame "Start Task 1" {
                n239 = for {
                  shift-right: [w418] -> w413
                  shift-left: w414 -> [w417]
                  tunnel: string[] ["RESET ENCODERS", "RESET YAW", "FORWARD", "READ ENCODERS"] -> [w416] mode=indexing
                  n240 = Enqueue Element(queue=w417, element=w416) -> (queue out=w418:refnum<queue>)  [unwired: 2 in, 2 out]
                }
              }
              frame "Start Task 2" {
                n241 = for {
                  shift-right: [w426] -> w421
                  shift-left: w422 -> [w425]
                  tunnel: string[] ["RESET ENCODERS", "RESET YAW", "READ ULTRASONIC", "ARDUINO - ULTRASONIC"] -> [w424] mode=indexing
                  n242 = Enqueue Element(queue=w425, element=w424) -> (queue out=w426:refnum<queue>)  [unwired: 2 in, 2 out]
                }
              }
              frame "Start Task 3" {
                n243 = for {
                  shift-right: [w434] -> w429
                  shift-left: w430 -> [w433]
                  tunnel: string[] ["RESET ENCODERS", "READ ENCODERS", "R-ACW"] -> [w432] mode=indexing
                  n244 = Enqueue Element(queue=w433, element=w432) -> (queue out=w434:refnum<queue>)  [unwired: 2 in, 2 out]
                }
              }
              frame "Start Task 4" {
                n245 = for {
                  shift-right: [w442] -> w437
                  shift-left: w438 -> [w441]
                  tunnel: string[] ["RESET YAW", "RESET ENCODERS", "RESET ARM", "RESET FLAGS", "", ""] -> [w440] mode=indexing
                  n246 = Enqueue Element(queue=w441, element=w440) -> (queue out=w442:refnum<queue>)  [unwired: 2 in, 2 out]
                }
              }
              frame "Start Task 5" {
                n247 = for {
                  shift-right: [w450] -> w445
                  shift-left: w446 -> [w449]
                  tunnel: string[] ["RESET YAW", "RESET ENCODERS", "RESET ARM", "RESET ALL SENSORS", "", ""] -> [w448] mode=indexing
                  n248 = Enqueue Element(queue=w449, element=w448) -> (queue out=w450:refnum<queue>)  [unwired: 2 in, 2 out]
                }
              }
              frame "Start Task 6" {
                n249 = for {
                  shift-right: [w458] -> w453
                  shift-left: w454 -> [w457]
                  tunnel: string[] ["OPEN LOG CAM ", "", "", "", "", ""] -> [w456] mode=indexing
                  n250 = Enqueue Element(queue=w457, element=w456) -> (queue out=w458:refnum<queue>)  [unwired: 2 in, 2 out]
                }
              }
              frame "Start Task 8 - BALL" {
                n251 = for {
                  shift-right: [w466] -> w461
                  shift-left: w462 -> [w465]
                  tunnel: string[] ["RESET YAW", "RESET ENCODERS", "RESET ARM", "RESET FLAGS"] -> [w464] mode=indexing
                  n252 = Enqueue Element(queue=w465, element=w464) -> (queue out=w466:refnum<queue>)  [unwired: 2 in, 2 out]
                }
              }
              frame "Start Task 8 - Gel" {
                n253 = for {
                  shift-right: [w474] -> w469
                  shift-left: w470 -> [w473]
                  tunnel: string[] ["RESET YAW", "RESET ENCODERS", "RESET ARM", "RESET FLAGS"] -> [w472] mode=indexing
                  n254 = Enqueue Element(queue=w473, element=w472) -> (queue out=w474:refnum<queue>)  [unwired: 2 in, 2 out]
                }
              }
              frame "Start Task 8 - Pipe" {
                n255 = for {
                  shift-right: [w482] -> w477
                  shift-left: w478 -> [w481]
                  tunnel: string[] ["RESET YAW", "RESET ENCODERS", "RESET ARM", "RESET FLAGS"] -> [w480] mode=indexing
                  n256 = Enqueue Element(queue=w481, element=w480) -> (queue out=w482:refnum<queue>)  [unwired: 2 in, 2 out]
                }
              }
              frame "Start Task 8 - Soap" {
                n257 = for {
                  shift-right: [w490] -> w484
                  shift-left: w485 -> [w489]
                  tunnel: string[] ["RESET YAW", "RESET ENCODERS", "RESET ARM", "RESET FLAGS"] -> [w488] mode=indexing
                  n258 = Enqueue Element(queue=w489, element=w488) -> (queue out=w490:refnum<queue>)  [unwired: 2 in, 2 out]
                }
              }
              frame "Start Task 9" {
                n259 = for {
                  shift-right: [w498] -> w494
                  shift-left: w493 -> [w497]
                  tunnel: string[] ["Z STEPPER BOX HEIGHT", "READ STEPPER VALUES", "", ""] -> [w496] mode=indexing
                  n260 = Enqueue Element(queue=w497, element=w496) -> (queue out=w498:refnum<queue>)  [unwired: 2 in, 2 out]
                }
              }
              frame "None", Default {
              }
              frame "Exit" {
                n261 = for {
                  shift-right: [w509] -> w504
                  shift-left: w505 -> [w508]
                  tunnel: string[] ["STOP", "RESET ENCODERS", "RESET YAW", "EXIT"] -> [w507] mode=indexing
                  n262 = Enqueue Element(queue=w508, element=w507) -> (queue out=w509:refnum<queue>)  [unwired: 2 in, 2 out]
                }
              }
            }
          }
          frame "Shutdown" {
            # ">> Item Selection Bias >>"
            # ">>> yStepper command>>>"
            n263 = for {
              shift-right: [w520] -> w514
              shift-left: w516 -> [w519]
              tunnel: string[] ["INIT", "RESET ENCODERS", "RESET FLAGS", "CAM CLOSE", "DISPOSE BUFFERS", "EXIT", ""] -> [w518] mode=indexing
              n264 = Enqueue Element(queue=w519, element=w518) -> (queue out=w520:refnum<queue>)  [unwired: 2 in, 2 out]
            }
          }
          frame "Task 1A" {
            # ">>> Motor control cluster >>>"
            # ">> Line detection >>"
            # ">> Checks if 1 metre moved >>"
            # ">>> yStepper command>>>"
            # "Use 250"
            n265 = Greater?(x=w530, y=265.0) -> (0:w524:bool)
            n266 = Dequeue Element(queue=w537, timeout in ms (-1)=w536, error in (no error)=w535) -> (element=w534:T10)  [unwired: 3 out]
            n267 = And(x=w523, y=w524) -> (x .and. y?=w521:bool)
            n268 = case shown="\"Start Task 1\", Default" w534 {
              tunnel: w522 -> [w538 _]
              tunnel: [w548 State_Type_Definitions,_for_0.26g_versions_and_later_3."True Stop" ("Enum")] -> w533
              tunnel: w532 -> [w546 w563]
              tunnel: [w545 w562] -> w531
              tunnel: [State_Type_Definitions,_for_0.26g_versions_and_later_3."Idle" ("Enum") State_Type_Definitions,_for_0.26g_versions_and_later_3."Shutdown" ("Enum")] -> w528
              tunnel: w521 -> [w539 _]
              frame "Start Task 1", Default {
                n269 = Or(x=w539, y=w538) -> (x .or. y?=w540:bool)
                n270 = case shown="True" w540 {
                  tunnel: w546 -> [w551 w557]
                  tunnel: [w550 w555] -> w545
                  frame False {
                    n271 = for {
                      shift-right: [w553] -> w550
                      shift-left: w551 -> [w554]
                      tunnel: string[] ["READ ENCODERS", "READ NAVX", "FORWARD", "READ LINE SENSOR"] ("element") -> [w552] mode=indexing
                      n272 = Enqueue Element(queue=w554, element=w552) -> (queue out=w553:refnum<queue>)  [unwired: 2 in, 2 out]
                    }
                  }
                  frame True {
                    n273 = for {
                      shift-right: [w559] -> w555
                      shift-left: w557 -> [w560]
                      tunnel: string[] ["RESET YAW", "RESET ENCODERS", "STOP", ""] -> [w558] mode=indexing
                      n274 = Enqueue Element(queue=w560, element=w558) -> (queue out=w559:refnum<queue>)  [unwired: 2 in, 2 out]
                    }
                  }
                }
                n275 = Select(t=State_Type_Definitions,_for_0.26g_versions_and_later_3."True Stop" ("Enum"), s=w538, f=State_Type_Definitions,_for_0.26g_versions_and_later_3."Task 1B" ("Enum")) -> (s? t:f=w543:T18)
                n276 = Select(t=w543, s=w539, f=State_Type_Definitions,_for_0.26g_versions_and_later_3."Task 1A" ("Enum")) -> (s? t:f=w548:T18)
              }
              frame "Exit" {
                n277 = for {
                  shift-right: [w567] -> w562
                  shift-left: w563 -> [w568]
                  tunnel: string[] ["STOP", "RESET ENCODERS", "RESET YAW", ""] -> [w566] mode=indexing
                  n278 = Enqueue Element(queue=w568, element=w566) -> (queue out=w567:refnum<queue>)  [unwired: 2 in, 2 out]
                }
              }
            }
          }
          frame "Task 1B" {
            # ">>> Motor control cluster >>>"
            # ">> Line detection >>"
            # ">> Adds small distance overhead after 1M >>"
            # ">>> yStepper command>>>"
            n279 = Greater?(x=w575, y=50.0) -> (0:w569:bool)
            n280 = Dequeue Element(queue=w584, timeout in ms (-1)=w583, error in (no error)=w582) -> (element=w581:T10)  [unwired: 3 out]
            n281 = Or(x=w569, y=w576) -> (x .or. y?=w580:bool)
            n282 = case shown="\"Start Task 1\", Default" w581 {
              tunnel: w580 -> [w587 _]
              tunnel: [w591 State_Type_Definitions,_for_0.26g_versions_and_later_3."True Stop" ("Enum")] -> w579
              tunnel: w578 -> [w588 w606]
              tunnel: [w586 w605] -> w577
              tunnel: [State_Type_Definitions,_for_0.26g_versions_and_later_3."Idle" ("Enum") State_Type_Definitions,_for_0.26g_versions_and_later_3."Shutdown" ("Enum")] -> w573
              frame "Start Task 1", Default {
                n283 = case shown="True" w587 {
                  tunnel: w588 -> [w594 w600]
                  tunnel: [w593 w598] -> w586
                  frame False {
                    n284 = for {
                      shift-right: [w596] -> w593
                      shift-left: w594 -> [w597]
                      tunnel: string[] ["READ ENCODERS", "READ NAVX", "FORWARD", "READ LINE SENSOR"] ("element") -> [w595] mode=indexing
                      n285 = Enqueue Element(queue=w597, element=w595) -> (queue out=w596:refnum<queue>)  [unwired: 2 in, 2 out]
                    }
                  }
                  frame True {
                    n286 = for {
                      shift-right: [w602] -> w598
                      shift-left: w600 -> [w603]
                      tunnel: string[] ["RESET YAW", "RESET ENCODERS", "STOP", ""] -> [w601] mode=indexing
                      n287 = Enqueue Element(queue=w603, element=w601) -> (queue out=w602:refnum<queue>)  [unwired: 2 in, 2 out]
                    }
                  }
                }
                n288 = Select(t=State_Type_Definitions,_for_0.26g_versions_and_later_3."True Stop" ("Enum"), s=w587, f=State_Type_Definitions,_for_0.26g_versions_and_later_3."Task 1B" ("Enum")) -> (s? t:f=w591:T18)
              }
              frame "Exit" {
                n289 = for {
                  shift-right: [w610] -> w605
                  shift-left: w606 -> [w611]
                  tunnel: string[] ["STOP", "RESET ENCODERS", "RESET YAW", ""] -> [w609] mode=indexing
                  n290 = Enqueue Element(queue=w611, element=w609) -> (queue out=w610:refnum<queue>)  [unwired: 2 in, 2 out]
                }
              }
            }
          }
          frame "Task 2:Raise Arm" {
            # ">> Stepper height reeached >>"
            # ">>> yStepper command>>>"
            # ">> Manual override >>"
            n291 = Dequeue Element(queue=w618, timeout in ms (-1)=w617, error in (no error)=w616) -> (element=w626:T10)  [unwired: 3 out]
            n292 = Equal?(x=w620, y=u8 60) -> (x = y?=w612:bool)
            n293 = case shown="\"Start Task 1\", Default" w626 {
              tunnel: [w637 State_Type_Definitions,_for_0.26g_versions_and_later_3."True Stop" ("Enum")] -> w622
              tunnel: [w635 w652] -> w615
              tunnel: w624 -> [w634 _]
              tunnel: w623 -> [w628 _]
              tunnel: [State_Type_Definitions,_for_0.26g_versions_and_later_3."Idle" ("Enum") State_Type_Definitions,_for_0.26g_versions_and_later_3."Shutdown" ("Enum")] -> w621
              tunnel: w612 -> [w627 _]
              frame "Start Task 1", Default {
                # ">> WIill proceed to part ii if not manual override >>"
                # ">>If ENABLE or Trigger is set to true>>"
                n294 = Or(x=w627, y=w628) -> (x .or. y?=w629:bool)
                n295 = case shown="True" w627 {
                  tunnel: [w640 w646] -> w635
                  tunnel: w634 -> [w639 w645]
                  frame False {
                    n296 = for {
                      shift-right: [w642] -> w640
                      shift-left: w639 -> [w643]
                      tunnel: string[] ["Z STEPPER CAM HEIGHT", "READ STEPPER VALUES"] ("element") -> [w641] mode=indexing
                      n297 = Enqueue Element(queue=w643, element=w641) -> (queue out=w642:refnum<queue>)  [unwired: 2 in, 2 out]
                    }
                  }
                  frame True {
                    n298 = for {
                      shift-right: [w648] -> w646
                      shift-left: w645 -> [w649]
                      tunnel: string[] ["ARDUINO - ULTRASONIC", "READ ULTRASONIC", "", "", "", ""] -> [w647] mode=indexing
                      n299 = Enqueue Element(queue=w649, element=w647) -> (queue out=w648:refnum<queue>)  [unwired: 2 in, 2 out]
                    }
                  }
                }
                n300 = Select(t=State_Type_Definitions,_for_0.26g_versions_and_later_3."True Stop" ("Enum"), s=w628, f=State_Type_Definitions,_for_0.26g_versions_and_later_3."Task 2:Sensor Mode" ("Enum")) -> (s? t:f=w631:T18)
                n301 = Select(t=w631, s=w629, f=State_Type_Definitions,_for_0.26g_versions_and_later_3."Task 2:Raise Arm" ("Enum")) -> (s? t:f=w637:T18)
              }
              frame "Exit" {
                n302 = for {
                  shift-right: [w655] -> w652
                  shift-left: _ -> [w656]
                  tunnel: string[] ["STOP", "RESET ENCODERS", "RESET YAW", ""] -> [w654] mode=indexing
                  n303 = Enqueue Element(queue=w656, element=w654) -> (queue out=w655:refnum<queue>)  [unwired: 2 in, 2 out]
                }
              }
            }
          }
          frame "Task 2:Sensor Mode" {
            w673 = u8 20 ("y")
            # ">>> yStepper command>>>"
            # ">>Object detected>>"
            n304 = Dequeue Element(queue=w666, timeout in ms (-1)=w665, error in (no error)=w664) -> (element=w674:T10)  [unwired: 3 out]
            n305 = Less?(x=w662, y=w673) -> (x < y?=w672:bool)
            n306 = Less?(x=w661, y=w673) -> (x < y?=w671:bool)
            n307 = Or(x=w672, y=w671) -> (x .or. y?=w657:bool)
            n308 = case shown="\"Start Task 1\", Default" w674 {
              tunnel: w657 -> [w677 _]
              tunnel: [w684 State_Type_Definitions,_for_0.26g_versions_and_later_3."True Stop" ("Enum")] -> w670
              tunnel: w663 -> [w676 _]
              tunnel: w667 -> [w683 w700]
              tunnel: [w682 w701] -> w669
              tunnel: [State_Type_Definitions,_for_0.26g_versions_and_later_3."Idle" ("Enum") State_Type_Definitions,_for_0.26g_versions_and_later_3."Shutdown" ("Enum")] -> w668
              frame "Start Task 1", Default {
                n309 = case shown="False" w677 {
                  tunnel: w683 -> [w687 w694]
                  tunnel: [w688 w693] -> w682
                  frame False {
                    n310 = for {
                      tunnel: string[] ["READ ULTRASONIC", "STOP"] ("element") -> [w689] mode=indexing
                      shift-right: [w691] -> w688
                      shift-left: w687 -> [w690]
                      n311 = Enqueue Element(queue=w690, element=w689) -> (queue out=w691:refnum<queue>)  [unwired: 2 in, 2 out]
                    }
                  }
                  frame True {
                    n312 = for {
                      shift-right: [w696] -> w693
                      shift-left: w694 -> [w697]
                      tunnel: string[] ["RESET ENCODERS", "READ NAVX", "READ ENCODERS"] -> [w695] mode=indexing
                      n313 = Enqueue Element(queue=w697, element=w695) -> (queue out=w696:refnum<queue>)  [unwired: 2 in, 2 out]
                    }
                  }
                }
                n314 = Or(x=w677, y=w676) -> (x .or. y?=w675:bool)
                n315 = Select(t=State_Type_Definitions,_for_0.26g_versions_and_later_3."True Stop" ("Enum"), s=w676, f=State_Type_Definitions,_for_0.26g_versions_and_later_3."Task 2:Reverse Mode" ("Enum")) -> (s? t:f=w678:T18)
                n316 = Select(t=w678, s=w675, f=State_Type_Definitions,_for_0.26g_versions_and_later_3."Task 2:Sensor Mode" ("Enum")) -> (s? t:f=w684:T18)
              }
              frame "Exit" {
                n317 = for {
                  shift-right: [w704] -> w701
                  shift-left: w700 -> [w705]
                  tunnel: string[] ["STOP", "RESET ENCODERS", "RESET YAW", "ARDUINO MODE 0"] -> [w703] mode=indexing
                  n318 = Enqueue Element(queue=w705, element=w703) -> (queue out=w704:refnum<queue>)  [unwired: 2 in, 2 out]
                }
              }
            }
          }
          frame "Task 2:Reverse Mode" {
            # ">>> yStepper command>>>"
            n319 = Dequeue Element(queue=w716, timeout in ms (-1)=w717, error in (no error)=w718) -> (element=w720:T10)  [unwired: 3 out]
            n320 = Less?(x=w710, y=-30.0) -> (x < y?=w706:bool)
            n321 = case shown="\"Start Task 1\", Default" w720 {
              tunnel: [w730 State_Type_Definitions,_for_0.26g_versions_and_later_3."True Stop" ("Enum")] -> w712
              tunnel: w719 -> [w723 _]
              tunnel: w715 -> [w729 w746]
              tunnel: [w728 w747] -> w711
              tunnel: [State_Type_Definitions,_for_0.26g_versions_and_later_3."Idle" ("Enum") State_Type_Definitions,_for_0.26g_versions_and_later_3."Shutdown" ("Enum")] -> w713
              tunnel: w706 -> [w721 _]
              frame "Start Task 1", Default {
                n322 = case shown="True" w721 {
                  tunnel: w729 -> [w733 w740]
                  tunnel: [w734 w739] -> w728
                  frame False {
                    n323 = for {
                      tunnel: string[] ["READ ENCODERS", "REVERSE", "READ NAVX"] ("element") -> [w735] mode=indexing
                      shift-right: [w737] -> w734
                      shift-left: w733 -> [w736]
                      n324 = Enqueue Element(queue=w736, element=w735) -> (queue out=w737:refnum<queue>)  [unwired: 2 in, 2 out]
                    }
                  }
                  frame True {
                    n325 = for {
                      shift-right: [w742] -> w739
                      shift-left: w740 -> [w743]
                      tunnel: string[] ["STOP", "ARDUINO - ULTRASONIC", "READ ULTRASONIC", "RESET ENCODERS"] -> [w741] mode=indexing
                      n326 = Enqueue Element(queue=w743, element=w741) -> (queue out=w742:refnum<queue>)  [unwired: 2 in, 2 out]
                    }
                  }
                }
                n327 = Or(x=w721, y=w723) -> (x .or. y?=w722:bool)
                n328 = Select(t=State_Type_Definitions,_for_0.26g_versions_and_later_3."True Stop" ("Enum"), s=w723, f=State_Type_Definitions,_for_0.26g_versions_and_later_3."Task 2:Sensor Mode" ("Enum")) -> (s? t:f=w724:T18)
                n329 = Select(t=w724, s=w722, f=State_Type_Definitions,_for_0.26g_versions_and_later_3."Task 2:Reverse Mode" ("Enum")) -> (s? t:f=w730:T18)
              }
              frame "Exit" {
                n330 = for {
                  shift-right: [w750] -> w747
                  shift-left: w746 -> [w751]
                  tunnel: string[] ["STOP", "RESET ENCODERS", "RESET YAW", "ARDUINO MODE 0"] -> [w749] mode=indexing
                  n331 = Enqueue Element(queue=w751, element=w749) -> (queue out=w750:refnum<queue>)  [unwired: 2 in, 2 out]
                }
              }
            }
          }
          frame "Task 3" {
            # ">>> Motor control cluster >>>"
            # ">>> yStepper command>>>"
            n332 = Dequeue Element(queue=w767, timeout in ms (-1)=w766, error in (no error)=w765) -> (element=w757:T10)  [unwired: 3 out]
            n333 = Less?(x=w764, y=-160.0) -> (x < y?=w752:bool)
            n334 = Or(x=w752, y=w762) -> (x .or. y?=w758:bool)
            n335 = case shown="\"Start Task 1\", Default" w757 {
              tunnel: w758 -> [w770 _]
              tunnel: [w774 State_Type_Definitions,_for_0.26g_versions_and_later_3."True Stop" ("Enum")] -> w759
              tunnel: w761 -> [w771 w790]
              tunnel: [w769 w789] -> w760
              tunnel: [State_Type_Definitions,_for_0.26g_versions_and_later_3."Idle" ("Enum") State_Type_Definitions,_for_0.26g_versions_and_later_3."Shutdown" ("Enum")] -> w756
              frame "Start Task 1", Default {
                n336 = case shown="False" w770 {
                  tunnel: w771 -> [w777 w783]
                  tunnel: [w776 w781] -> w769
                  frame False {
                    n337 = for {
                      shift-right: [w779] -> w776
                      shift-left: w777 -> [w780]
                      tunnel: string[] ["READ ENCODERS", "R-CW"] ("element") -> [w778] mode=indexing
                      n338 = Enqueue Element(queue=w780, element=w778) -> (queue out=w779:refnum<queue>)  [unwired: 2 in, 2 out]
                    }
                  }
                  frame True {
                    n339 = for {
                      shift-right: [w785] -> w781
                      shift-left: w783 -> [w786]
                      tunnel: string[] ["RESET YAW", "RESET ENCODERS", "STOP", "ARDUINO MODE 0"] -> [w784] mode=indexing
                      n340 = Enqueue Element(queue=w786, element=w784) -> (queue out=w785:refnum<queue>)  [unwired: 2 in, 2 out]
                    }
                  }
                }
                n341 = Select(t=State_Type_Definitions,_for_0.26g_versions_and_later_3."True Stop" ("Enum"), s=w770, f=State_Type_Definitions,_for_0.26g_versions_and_later_3."Task 3" ("Enum")) -> (s? t:f=w774:T18)
              }
              frame "Exit" {
                n342 = for {
                  shift-right: [w793] -> w789
                  shift-left: w790 -> [w794]
                  tunnel: string[] ["STOP", "RESET ENCODERS", "RESET YAW", ""] -> [w792] mode=indexing
                  n343 = Enqueue Element(queue=w794, element=w792) -> (queue out=w793:refnum<queue>)  [unwired: 2 in, 2 out]
                }
              }
            }
          }
          frame "Task 4_A" {
            # ">> Stepper height reeached >>"
            # ">>> yStepper command>>>"
            # ">> Manual override >>"
            n344 = Dequeue Element(queue=w808, timeout in ms (-1)=w807, error in (no error)=w806) -> (element=w805:T10)  [unwired: 3 out]
            n345 = Equal?(x=w799, y=u8 60) -> (x = y?=w795:bool)
            n346 = case shown="\"Start Task 1\", Default" w805 {
              tunnel: [w820 State_Type_Definitions,_for_0.26g_versions_and_later_3."True Stop" ("Enum")] -> w804
              tunnel: [w818 w836] -> w803
              tunnel: w809 -> [w817 w833]
              tunnel: w802 -> [w811 _]
              tunnel: [State_Type_Definitions,_for_0.26g_versions_and_later_3."Idle" ("Enum") State_Type_Definitions,_for_0.26g_versions_and_later_3."Shutdown" ("Enum")] -> w801
              tunnel: w795 -> [w810 _]
              frame "Start Task 1", Default {
                # ">> WIill proceed to part ii if not manual override >>"
                # ">>If ENABLE or Trigger is set to true>>"
                n347 = Or(x=w810, y=w811) -> (x .or. y?=w812:bool)
                n348 = case shown="False" w810 {
                  tunnel: [w823 w829] -> w818
                  tunnel: w817 -> [w822 w828]
                  frame False {
                    n349 = for {
                      shift-right: [w825] -> w823
                      shift-left: w822 -> [w826]
                      tunnel: string[] ["Z STEPPER CAM HEIGHT", "READ STEPPER VALUES"] ("element") -> [w824] mode=indexing
                      n350 = Enqueue Element(queue=w826, element=w824) -> (queue out=w825:refnum<queue>)  [unwired: 2 in, 2 out]
                    }
                  }
                  frame True {
                    n351 = for {
                      shift-right: [w831] -> w829
                      shift-left: w828 -> [w832]
                      tunnel: string[] ["ARDUINO - ULTRASONIC", "READ ULTRASONIC", "FORWARD", "", "", ""] -> [w830] mode=indexing
                      n352 = Enqueue Element(queue=w832, element=w830) -> (queue out=w831:refnum<queue>)  [unwired: 2 in, 2 out]
                    }
                  }
                }
                n353 = Select(t=State_Type_Definitions,_for_0.26g_versions_and_later_3."True Stop" ("Enum"), s=w811, f=State_Type_Definitions,_for_0.26g_versions_and_later_3."Task 4_B" ("Enum")) -> (s? t:f=w814:T18)
                n354 = Select(t=w814, s=w812, f=State_Type_Definitions,_for_0.26g_versions_and_later_3."Task 4_A" ("Enum")) -> (s? t:f=w820:T18)
              }
              frame "Exit" {
                n355 = for {
                  shift-right: [w839] -> w836
                  shift-left: w833 -> [w840]
                  tunnel: string[] ["STOP", "RESET ENCODERS", "RESET YAW", ""] -> [w838] mode=indexing
                  n356 = Enqueue Element(queue=w840, element=w838) -> (queue out=w839:refnum<queue>)  [unwired: 2 in, 2 out]
                }
              }
            }
          }
          frame "Task 4_B" {
            w846 = u8 20
            # ">> Path blocked >>"
            # ">>> yStepper command>>>"
            # ">> Manual override >>"
            n357 = Dequeue Element(queue=w855, timeout in ms (-1)=w854, error in (no error)=w853) -> (element=w852:T10)  [unwired: 3 out]
            n358 = Less?(x=w848, y=w846) -> (x < y?=w843:bool)
            n359 = Less?(x=w847, y=w846) -> (x < y?=w844:bool)
            n360 = And(x=w844, y=w843) -> (x .and. y?=w845:bool)
            n361 = case shown="\"Start Task 1\", Default" w852 {
              tunnel: [w869 State_Type_Definitions,_for_0.26g_versions_and_later_3."True Stop" ("Enum")] -> w857
              tunnel: [w867 w884] -> w858
              tunnel: w851 -> [w866 _]
              tunnel: w856 -> [w860 _]
              tunnel: [State_Type_Definitions,_for_0.26g_versions_and_later_3."Idle" ("Enum") State_Type_Definitions,_for_0.26g_versions_and_later_3."Shutdown" ("Enum")] -> w850
              tunnel: w845 -> [w859 _]
              frame "Start Task 1", Default {
                # ">> Manual override forces program to true stop >>"
                # ">>If ENABLE or Trigger is set to true>>"
                n362 = Or(x=w859, y=w860) -> (x .or. y?=w865:bool)
                n363 = case shown="False" w859 {
                  tunnel: [w872 w877] -> w867
                  tunnel: w866 -> [w871 w876]
                  frame False {
                    n364 = for {
                      shift-right: [w874] -> w872
                      shift-left: w871 -> [w875]
                      tunnel: string[] ["FORWARD", "READ ULTRASONIC", "READ NAVX"] ("element") -> [w873] mode=indexing
                      n365 = Enqueue Element(queue=w875, element=w873) -> (queue out=w874:refnum<queue>)  [unwired: 2 in, 2 out]
                    }
                  }
                  frame True {
                    n366 = for {
                      shift-right: [w880] -> w877
                      shift-left: w876 -> [w881]
                      tunnel: string[] ["STOP", "RESET YAW", "RESET ENCODERS", "RESET FLAGS"] -> [w879] mode=indexing
                      n367 = Enqueue Element(queue=w881, element=w879) -> (queue out=w880:refnum<queue>)  [unwired: 2 in, 2 out]
                    }
                  }
                }
                n368 = Select(t=State_Type_Definitions,_for_0.26g_versions_and_later_3."True Stop" ("Enum"), s=w860, f=State_Type_Definitions,_for_0.26g_versions_and_later_3."Task 4_C" ("Enum")) -> (s? t:f=w862:T18)
                n369 = Select(t=w862, s=w865, f=State_Type_Definitions,_for_0.26g_versions_and_later_3."Task 4_B" ("Enum")) -> (s? t:f=w869:T18)
              }
              frame "Exit" {
                n370 = for {
                  shift-right: [w887] -> w884
                  shift-left: _ -> [w888]
                  tunnel: string[] ["STOP", "RESET ENCODERS", "RESET YAW", ""] -> [w886] mode=indexing
                  n371 = Enqueue Element(queue=w888, element=w886) -> (queue out=w887:refnum<queue>)  [unwired: 2 in, 2 out]
                }
              }
            }
          }
          frame "Task 4_C" {
            w900 = u8 20
            # ">> xDistance travelled>>"
            # ">> Path NOT blocked >>"
            # ">>> yStepper command>>>"
            # ">> Manual override >>"
            n372 = Dequeue Element(queue=w910, timeout in ms (-1)=w903, error in (no error)=w902) -> (element=w904:T10)  [unwired: 3 out]
            n373 = Greater?(x=w892, y=w900) -> (0:w898:bool)
            n374 = Greater?(x=w897, y=80.0) -> (0:w895:bool)
            n375 = Greater?(x=w891, y=w900) -> (0:w899:bool)
            n376 = And(x=w899, y=w898) -> (x .and. y?=w894:bool)
            n377 = And(x=w895, y=w894) -> (x .and. y?=w893:bool)
            n378 = case shown="\"Start Task 1\", Default" w904 {
              tunnel: [w921 State_Type_Definitions,_for_0.26g_versions_and_later_3."True Stop" ("Enum")] -> w907
              tunnel: [w919 w937] -> w906
              tunnel: w909 -> [w918 w934]
              tunnel: w908 -> [w912 _]
              tunnel: [State_Type_Definitions,_for_0.26g_versions_and_later_3."Idle" ("t") State_Type_Definitions,_for_0.26g_versions_and_later_3."Shutdown" ("Enum")] -> w905
              tunnel: w893 -> [w911 _]
              frame "Start Task 1", Default {
                # ">> Manual override forces program to true stop >>"
                # ">>If ENABLE or Trigger is set to true>>"
                n379 = Or(x=w911, y=w912) -> (x .or. y?=w917:bool)
                n380 = case shown="False" w911 {
                  tunnel: [w924 w929] -> w919
                  tunnel: w918 -> [w922 w928]
                  frame False {
                    n381 = for {
                      shift-right: [w926] -> w924
                      shift-left: w922 -> [w927]
                      tunnel: string[] ["RIGHT", "READ NAVX", "READ ENCODERS", "READ ULTRASONIC"] ("element") -> [w925] mode=indexing
                      n382 = Enqueue Element(queue=w927, element=w925) -> (queue out=w926:refnum<queue>)  [unwired: 2 in, 2 out]
                    }
                  }
                  frame True {
                    n383 = for {
                      shift-right: [w932] -> w929
                      shift-left: w928 -> [w933]
                      tunnel: string[] ["STOP", "RESET YAW", "RESET ENCODERS", "ARDUINO - ULTRASONIC"] -> [w931] mode=indexing
                      n384 = Enqueue Element(queue=w933, element=w931) -> (queue out=w932:refnum<queue>)  [unwired: 2 in, 2 out]
                    }
                  }
                }
                n385 = Select(t=State_Type_Definitions,_for_0.26g_versions_and_later_3."True Stop" ("Enum"), s=w912, f=State_Type_Definitions,_for_0.26g_versions_and_later_3."Task 4_D" ("Enum")) -> (s? t:f=w913:T18)
                n386 = Select(t=w913, s=w917, f=State_Type_Definitions,_for_0.26g_versions_and_later_3."Task 4_C" ("Enum")) -> (s? t:f=w921:T18)
              }
              frame "Exit" {
                n387 = for {
                  shift-right: [w940] -> w937
                  shift-left: w934 -> [w941]
                  tunnel: string[] ["STOP", "RESET ENCODERS", "RESET YAW", ""] -> [w939] mode=indexing
                  n388 = Enqueue Element(queue=w941, element=w939) -> (queue out=w940:refnum<queue>)  [unwired: 2 in, 2 out]
                }
              }
            }
          }
          frame "Task 4_D" {
            w964 = u8 20
            # ">>> Motor control cluster >>>"
            # ">> Line detected >>"
            # ">> yDistance travelled>>"
            # ">> Path blocked >>"
            # ">>> yStepper command>>>"
            # ">> Manual override >>"
            n389 = Less?(x=w949, y=w964) -> (x < y?=w962:bool)
            n390 = Greater?(x=w953, y=200.0) -> (0:w960:bool)
            n391 = Less?(x=w948, y=w964) -> (x < y?=w963:bool)
            n392 = And(x=w963, y=w962) -> (x .and. y?=w959:bool)
            n393 = Dequeue Element(queue=w956, timeout in ms (-1)=w955, error in (no error)=w954) -> (element=w965:T10)  [unwired: 3 out]
            n394 = Or(x=w960, y=w959) -> (x .or. y?=w943:bool)
            n395 = And(x=w944, y=w943) -> (x .and. y?=w942:bool)
            n396 = case shown="\"Start Task 1\", Default" w965 {
              tunnel: [w976 State_Type_Definitions,_for_0.26g_versions_and_later_3."True Stop" ("Enum")] -> w952
              tunnel: [w974 w992] -> w950
              tunnel: w957 -> [w973 w989]
              tunnel: w958 -> [w967 _]
              tunnel: [State_Type_Definitions,_for_0.26g_versions_and_later_3."Idle" ("t") State_Type_Definitions,_for_0.26g_versions_and_later_3."Shutdown" ("Enum")] -> w951
              tunnel: w942 -> [w966 _]
              frame "Start Task 1", Default {
                # ">> Manual override forces program to true stop >>"
                # ">>If ENABLE or Trigger is set to true>>"
                n397 = Or(x=w966, y=w967) -> (x .or. y?=w972:bool)
                n398 = case shown="False" w966 {
                  tunnel: [w979 w984] -> w974
                  tunnel: w973 -> [w977 w983]
                  frame False {
                    n399 = for {
                      shift-right: [w981] -> w979
                      shift-left: w977 -> [w982]
                      tunnel: string[] ["FORWARD", "READ NAVX", "READ ENCODERS", "READ ULTRASONIC", "READ LINE SENSOR"] ("element") -> [w980] mode=indexing
                      n400 = Enqueue Element(queue=w982, element=w980) -> (queue out=w981:refnum<queue>)  [unwired: 2 in, 2 out]
                    }
                  }
                  frame True {
                    n401 = for {
                      shift-right: [w987] -> w984
                      shift-left: w983 -> [w988]
                      tunnel: string[] ["STOP", "RESET YAW", "RESET ENCODERS", "RESET FLAGS"] -> [w986] mode=indexing
                      n402 = Enqueue Element(queue=w988, element=w986) -> (queue out=w987:refnum<queue>)  [unwired: 2 in, 2 out]
                    }
                  }
                }
                n403 = Select(t=State_Type_Definitions,_for_0.26g_versions_and_later_3."True Stop" ("Enum"), s=w967, f=State_Type_Definitions,_for_0.26g_versions_and_later_3."True Stop" ("Enum")) -> (s? t:f=w968:T18)
                n404 = Select(t=w968, s=w972, f=State_Type_Definitions,_for_0.26g_versions_and_later_3."Task 4_D" ("Enum")) -> (s? t:f=w976:T18)
              }
              frame "Exit" {
                n405 = for {
                  shift-right: [w995] -> w992
                  shift-left: w989 -> [w996]
                  tunnel: string[] ["STOP", "RESET ENCODERS", "RESET YAW", ""] -> [w994] mode=indexing
                  n406 = Enqueue Element(queue=w996, element=w994) -> (queue out=w995:refnum<queue>)  [unwired: 2 in, 2 out]
                }
              }
            }
          }
          frame "Task 5A: RAISING ARM" {
            # "Stays in Task 5_A until stepper reaches desired \nheight"
            # ">>> Motor control cluster >>>"
            # ">>> yStepper command>>>"
            # ">> Manual override >>"
            n407 = Dequeue Element(queue=w1007, timeout in ms (-1)=w1006, error in (no error)=w1008) -> (element=w1005:T10)  [unwired: 3 out]
            n408 = Equal?(x=w1004, y=u8 60) -> (x = y?=w1002:bool)
            n409 = case shown="\"Start Task 1\", Default" w1005 {
              tunnel: [w1018 State_Type_Definitions,_for_0.26g_versions_and_later_3."True Stop" ("Enum")] -> w1009
              tunnel: [w1021 w1038] -> w1010
              tunnel: [State_Type_Definitions,_for_0.26g_versions_and_later_3."Idle" ("Enum") State_Type_Definitions,_for_0.26g_versions_and_later_3."Shutdown" ("Enum")] -> w1011
              tunnel: w1002 -> [w1017 _]
              tunnel: w1001 -> [w1016 _]
              tunnel: w1000 -> [w1012 w1035]
              frame "Start Task 1", Default {
                # "T: Go back to idle, F: Continue with task\""
                # ">> Manual override >>"
                n410 = case shown="False" w1017 {
                  tunnel: [w1025 w1031] -> w1021
                  tunnel: w1012 -> [w1023 w1029]
                  frame False {
                    n411 = for {
                      tunnel: string[] ["Z STEPPER CAM HEIGHT", "READ STEPPER VALUES"] ("element") -> [w1026] mode=indexing
                      shift-right: [w1028] -> w1025
                      shift-left: w1023 -> [w1027]
                      n412 = Enqueue Element(queue=w1027, element=w1026) -> (queue out=w1028:refnum<queue>)  [unwired: 2 in, 2 out]
                    }
                  }
                  frame True {
                    n413 = for {
                      shift-right: [w1033] -> w1031
                      shift-left: w1029 -> [w1034]
                      tunnel: string[] ["RESET FLAGS", "RESET YAW", "RESET ENCODERS"] -> [w1032] mode=indexing
                      n414 = Enqueue Element(queue=w1034, element=w1032) -> (queue out=w1033:refnum<queue>)  [unwired: 2 in, 2 out]
                    }
                  }
                }
                n415 = Or(x=w1017, y=w1016) -> (x .or. y?=w1019:bool)
                n416 = Select(t=State_Type_Definitions,_for_0.26g_versions_and_later_3."True Stop" ("Enum"), s=w1016, f=State_Type_Definitions,_for_0.26g_versions_and_later_3."Task 5B: STILL WAITING" ("Enum")) -> (s? t:f=w1013:T18)
                n417 = Select(t=w1013, s=w1019, f=State_Type_Definitions,_for_0.26g_versions_and_later_3."Task 5A: RAISING ARM" ("Enum")) -> (s? t:f=w1018:T18)
              }
              frame "Exit" {
                n418 = for {
                  shift-right: [w1041] -> w1038
                  shift-left: w1035 -> [w1042]
                  tunnel: string[] ["STOP", "RESET ENCODERS", "RESET YAW", "ARDUINO MODE 0"] -> [w1040] mode=indexing
                  n419 = Enqueue Element(queue=w1042, element=w1040) -> (queue out=w1041:refnum<queue>)  [unwired: 2 in, 2 out]
                }
              }
            }
          }
          frame "Task 5B: STILL WAITING" {
            # ">>> yStepper command>>>"
            n420 = Dequeue Element(queue=w1049, timeout in ms (-1)=w1048, error in (no error)=w1050) -> (element=w1047:T10)  [unwired: 3 out]
            n421 = local read "Rising Edge"() -> (w1043:bool)
            n422 = case shown="\"Start Task 1\", Default" w1047 {
              tunnel: [w1062 State_Type_Definitions,_for_0.26g_versions_and_later_3."True Stop" ("Enum")] -> w1052
              tunnel: [w1065 w1082] -> w1051
              tunnel: [State_Type_Definitions,_for_0.26g_versions_and_later_3."Idle" ("Enum") State_Type_Definitions,_for_0.26g_versions_and_later_3."Shutdown" ("Enum")] -> w1053
              tunnel: w1055 -> [w1061 _]
              tunnel: w1054 -> [w1057 w1079]
              tunnel: w1043 -> [w1056 _]
              frame "Start Task 1", Default {
                # "T: Go back to idle, F: Continue with task\""
                # ">> Manual override >>"
                n423 = case shown="False" w1056 {
                  tunnel: [w1069 w1075] -> w1065
                  tunnel: w1057 -> [w1067 w1073]
                  frame False {
                    n424 = for {
                      tunnel: string[] ["READ IR", "READ NAVX", ""] ("element") -> [w1070] mode=indexing
                      shift-right: [w1072] -> w1069
                      shift-left: w1067 -> [w1071]
                      n425 = Enqueue Element(queue=w1071, element=w1070) -> (queue out=w1072:refnum<queue>)  [unwired: 2 in, 2 out]
                    }
                  }
                  frame True {
                    n426 = for {
                      shift-right: [w1077] -> w1075
                      shift-left: w1073 -> [w1078]
                      tunnel: string[] ["Z STEPPER GRAB HEIGHT", "READ STEPPER VALUES", "", ""] -> [w1076] mode=indexing
                      n427 = Enqueue Element(queue=w1078, element=w1076) -> (queue out=w1077:refnum<queue>)  [unwired: 2 in, 2 out]
                    }
                  }
                }
                n428 = Or(x=w1056, y=w1061) -> (x .or. y?=w1063:bool)
                n429 = Select(t=State_Type_Definitions,_for_0.26g_versions_and_later_3."True Stop" ("Enum"), s=w1061, f=State_Type_Definitions,_for_0.26g_versions_and_later_3."Task 5C: GOING DOWN" ("Enum")) -> (s? t:f=w1058:T18)
                n430 = Select(t=w1058, s=w1063, f=State_Type_Definitions,_for_0.26g_versions_and_later_3."Task 5B: STILL WAITING" ("Enum")) -> (s? t:f=w1062:T18)
              }
              frame "Exit" {
                n431 = for {
                  shift-right: [w1085] -> w1082
                  shift-left: w1079 -> [w1086]
                  tunnel: string[] ["STOP", "RESET ENCODERS", "RESET YAW", "ARDUINO MODE 0"] -> [w1084] mode=indexing
                  n432 = Enqueue Element(queue=w1086, element=w1084) -> (queue out=w1085:refnum<queue>)  [unwired: 2 in, 2 out]
                }
              }
            }
          }
          frame "Task 5C: GOING DOWN" {
            # ">>> Motor control cluster >>>"
            # ">>> yStepper command>>>"
            # ">> Manual override >>"
            n433 = Equal?(x=w1089, y=u8 1) -> (x = y?=w1087:bool)
            n434 = Dequeue Element(queue=w1099, timeout in ms (-1)=w1098, error in (no error)=w1097) -> (element=w1096:T10)  [unwired: 3 out]
            n435 = case shown="\"Start Task 1\", Default" w1096 {
              tunnel: [w1108 State_Type_Definitions,_for_0.26g_versions_and_later_3."True Stop" ("Enum")] -> w1101
              tunnel: [w1111 w1128] -> w1094
              tunnel: [State_Type_Definitions,_for_0.26g_versions_and_later_3."Idle" ("Enum") State_Type_Definitions,_for_0.26g_versions_and_later_3."Shutdown" ("Enum")] -> w1093
              tunnel: w1095 -> [w1102 _]
              tunnel: w1100 -> [w1107 w1125]
              tunnel: w1087 -> [w1106 _]
              frame "Start Task 1", Default {
                # ">> Is time up? >>"
                # "Determines if object is in range to pick up"
                # ">> Manual override >>"
                n436 = case shown="False" w1106 {
                  tunnel: [w1115 w1121] -> w1111
                  tunnel: w1107 -> [w1114 w1119]
                  frame False {
                    n437 = for {
                      tunnel: string[] ["READ STEPPER VALUES", "Z STEPPER GRAB HEIGHT", "", ""] -> [w1116] mode=indexing
                      shift-right: [w1118] -> w1115
                      shift-left: w1114 -> [w1117]
                      n438 = Enqueue Element(queue=w1117, element=w1116) -> (queue out=w1118:refnum<queue>)  [unwired: 2 in, 2 out]
                    }
                  }
                  frame True {
                    n439 = for {
                      shift-right: [w1123] -> w1121
                      shift-left: w1119 -> [w1124]
                      tunnel: string[] ["RESET FLAGS", "RESET YAW", "SET TIMER 5"] -> [w1122] mode=indexing
                      n440 = Enqueue Element(queue=w1124, element=w1122) -> (queue out=w1123:refnum<queue>)  [unwired: 2 in, 2 out]
                    }
                  }
                }
                n441 = Or(x=w1106, y=w1102) -> (x .or. y?=w1109:bool)
                n442 = Select(t=State_Type_Definitions,_for_0.26g_versions_and_later_3."True Stop" ("Enum"), s=w1102, f=State_Type_Definitions,_for_0.26g_versions_and_later_3."Task 5D: GRAB" ("Enum")) -> (s? t:f=w1104:T18)
                n443 = Select(t=w1104, s=w1109, f=State_Type_Definitions,_for_0.26g_versions_and_later_3."Task 5C: GOING DOWN" ("Enum")) -> (s? t:f=w1108:T18)
              }
              frame "Exit" {
                n444 = for {
                  shift-right: [w1131] -> w1128
                  shift-left: w1125 -> [w1132]
                  tunnel: string[] ["STOP", "RESET ENCODERS", "RESET YAW", "ARDUINO MODE 0"] -> [w1130] mode=indexing
                  n445 = Enqueue Element(queue=w1132, element=w1130) -> (queue out=w1131:refnum<queue>)  [unwired: 2 in, 2 out]
                }
              }
            }
          }
          frame "Task 5D: GRAB" {
            # ">>> Motor control cluster >>>"
            # ">>> yStepper command>>>"
            n446 = Dequeue Element(queue=w1140, timeout in ms (-1)=w1139, error in (no error)=w1138) -> (element=w1137:T10)  [unwired: 3 out]
            n447 = case shown="\"Start Task 1\", Default" w1137 {
              tunnel: [w1152 State_Type_Definitions,_for_0.26g_versions_and_later_3."True Stop" ("Enum")] -> w1144
              tunnel: [w1155 w1172] -> w1143
              tunnel: [State_Type_Definitions,_for_0.26g_versions_and_later_3."Idle" ("Enum") State_Type_Definitions,_for_0.26g_versions_and_later_3."Shutdown" ("Enum")] -> w1145
              tunnel: w1141 -> [w1151 _]
              tunnel: w1142 -> [w1147 w1169]
              tunnel: w1135 -> [w1146 _]
              frame "Start Task 1", Default {
                # ">> T: Breaks out of state loop; F: Stays in loop>>"
                # ">> Manual override >>"
                # ">> Checks if time is up>>"
                # "Stays in Task 5D until the object is detected"
                # "T: Go back to idle, F: Continue with task\""
                # ">> Manual override >>"
                n448 = case shown="True" w1146 {
                  tunnel: [w1159 w1165] -> w1155
                  tunnel: w1147 -> [w1157 w1163]
                  frame False {
                    n449 = for {
                      tunnel: string[] ["START TIMER", "CLOSE CLAW", ""] ("element") -> [w1160] mode=indexing
                      shift-right: [w1162] -> w1159
                      shift-left: w1157 -> [w1161]
                      n450 = Enqueue Element(queue=w1161, element=w1160) -> (queue out=w1162:refnum<queue>)  [unwired: 2 in, 2 out]
                    }
                  }
                  frame True {
                    n451 = for {
                      shift-right: [w1167] -> w1165
                      shift-left: w1163 -> [w1168]
                      tunnel: string[] ["READ STEPPER VALUES", "ZSTEPPER BOX HEIGHT", ""] -> [w1166] mode=indexing
                      n452 = Enqueue Element(queue=w1168, element=w1166) -> (queue out=w1167:refnum<queue>)  [unwired: 2 in, 2 out]
                    }
                  }
                }
                n453 = Or(x=w1146, y=w1151) -> (x .or. y?=w1153:bool)
                n454 = Select(t=State_Type_Definitions,_for_0.26g_versions_and_later_3."True Stop" ("Enum"), s=w1151, f=State_Type_Definitions,_for_0.26g_versions_and_later_3."Task 5E: GOING UP" ("Enum")) -> (s? t:f=w1148:T18)
                n455 = Select(t=w1148, s=w1153, f=State_Type_Definitions,_for_0.26g_versions_and_later_3."Task 5D: GRAB" ("Enum")) -> (s? t:f=w1152:T18)
              }
              frame "Exit" {
                n456 = for {
                  shift-right: [w1175] -> w1172
                  shift-left: w1169 -> [w1176]
                  tunnel: string[] ["STOP", "RESET ENCODERS", "RESET YAW", "ARDUINO MODE 0"] -> [w1174] mode=indexing
                  n457 = Enqueue Element(queue=w1176, element=w1174) -> (queue out=w1175:refnum<queue>)  [unwired: 2 in, 2 out]
                }
              }
            }
          }
          frame "Task 5E: GOING UP" {
            # ">>> Motor control cluster >>>"
            # ">>> yStepper command>>>"
            n458 = Equal?(x=w1179, y=u8 50) -> (x = y?=w1177:bool)
            n459 = Dequeue Element(queue=w1187, timeout in ms (-1)=w1188, error in (no error)=w1189) -> (element=w1191:T10)  [unwired: 3 out]
            n460 = case shown="\"Start Task 1\", Default" w1191 {
              tunnel: [w1199 State_Type_Definitions,_for_0.26g_versions_and_later_3."True Stop" ("Enum")] -> w1185
              tunnel: [w1201 w1218] -> w1183
              tunnel: [State_Type_Definitions,_for_0.26g_versions_and_later_3."Idle" ("Enum") State_Type_Definitions,_for_0.26g_versions_and_later_3."Shutdown" ("Enum")] -> w1184
              tunnel: w1190 -> [w1198 _]
              tunnel: w1186 -> [w1194 w1215]
              tunnel: w1177 -> [w1193 _]
              frame "Start Task 1", Default {
                # ">> T: Breaks out of state loop; F: Stays in loop>>"
                # ">> Manual override >>"
                # ">> Checks if time is up>>"
                # "Stays in Task 5D until the object is detected"
                # "T: Go back to idle, F: Continue with task\""
                # ">> Manual override >>"
                n461 = Or(x=w1193, y=w1198) -> (x .or. y?=w1192:bool)
                n462 = case shown="False" w1192 {
                  tunnel: [w1205 w1211] -> w1201
                  tunnel: w1194 -> [w1203 w1209]
                  frame False {
                    n463 = for {
                      tunnel: string[] ["READ STEPPER VALUES", "ZSTEPPER BOX HEIGHT", ""] ("element") -> [w1206] mode=indexing
                      shift-right: [w1208] -> w1205
                      shift-left: w1203 -> [w1207]
                      n464 = Enqueue Element(queue=w1207, element=w1206) -> (queue out=w1208:refnum<queue>)  [unwired: 2 in, 2 out]
                    }
                  }
                  frame True {
                    n465 = for {
                      shift-right: [w1213] -> w1211
                      shift-left: w1209 -> [w1214]
                      tunnel: string[] ["CAM CLOSE", "DISPOSE BUFFERS", ""] -> [w1212] mode=indexing
                      n466 = Enqueue Element(queue=w1214, element=w1212) -> (queue out=w1213:refnum<queue>)  [unwired: 2 in, 2 out]
                    }
                  }
                }
                n467 = Select(t=State_Type_Definitions,_for_0.26g_versions_and_later_3."True Stop" ("Enum"), s=w1198, f=State_Type_Definitions,_for_0.26g_versions_and_later_3."True Stop" ("Enum")) -> (s? t:f=w1195:T18)
                n468 = Select(t=w1195, s=w1192, f=State_Type_Definitions,_for_0.26g_versions_and_later_3."Task 5E: GOING UP" ("Enum")) -> (s? t:f=w1199:T18)
              }
              frame "Exit" {
                n469 = for {
                  shift-right: [w1221] -> w1218
                  shift-left: w1215 -> [w1222]
                  tunnel: string[] ["STOP", "RESET ENCODERS", "RESET YAW", "ARDUINO MODE 0"] -> [w1220] mode=indexing
                  n470 = Enqueue Element(queue=w1222, element=w1220) -> (queue out=w1221:refnum<queue>)  [unwired: 2 in, 2 out]
                }
              }
            }
          }
          frame "Task 5F: ARM GRAB HEIGHT" {
            # ">>> Motor control cluster >>>"
            # ">>> yStepper command>>>"
            # ">> Manual override >>"
            n471 = Dequeue Element(queue=w1233, timeout in ms (-1)=w1232, error in (no error)=w1234) -> (element=w1231:T10)  [unwired: 3 out]
            n472 = Equal?(x=w1230, y=u8 1) -> (x = y?=w1228:bool)
            n473 = case shown="\"Start Task 1\", Default" w1231 {
              tunnel: [w1244 State_Type_Definitions,_for_0.26g_versions_and_later_3."True Stop" ("Enum")] -> w1235
              tunnel: [w1247 w1264] -> w1236
              tunnel: [State_Type_Definitions,_for_0.26g_versions_and_later_3."Idle" ("Enum") State_Type_Definitions,_for_0.26g_versions_and_later_3."Shutdown" ("Enum")] -> w1237
              tunnel: w1228 -> [w1243 _]
              tunnel: w1227 -> [w1242 _]
              tunnel: w1226 -> [w1238 w1261]
              frame "Start Task 1", Default {
                # "Stays in Task 5F until stepper reaches desired \nheight"
                # "T: Go back to idle, F: Continue with task\""
                # ">> Manual override >>"
                n474 = case shown="True" w1243 {
                  tunnel: [w1251 w1257] -> w1247
                  tunnel: w1238 -> [w1249 w1255]
                  frame False {
                    n475 = for {
                      tunnel: string[] ["Z STEPPER GRAB HEIGHT", "READ STEPPER VALUES"] ("element") -> [w1252] mode=indexing
                      shift-right: [w1254] -> w1251
                      shift-left: w1249 -> [w1253]
                      n476 = Enqueue Element(queue=w1253, element=w1252) -> (queue out=w1254:refnum<queue>)  [unwired: 2 in, 2 out]
                    }
                  }
                  frame True {
                    n477 = for {
                      shift-right: [w1259] -> w1257
                      shift-left: w1255 -> [w1260]
                      tunnel: string[] ["RESET YAW", "RESET ENCODERS", "RESET FLAGS"] -> [w1258] mode=indexing
                      n478 = Enqueue Element(queue=w1260, element=w1258) -> (queue out=w1259:refnum<queue>)  [unwired: 2 in, 2 out]
                    }
                  }
                }
                n479 = Or(x=w1243, y=w1242) -> (x .or. y?=w1245:bool)
                n480 = Select(t=State_Type_Definitions,_for_0.26g_versions_and_later_3."True Stop" ("Enum"), s=w1242, f=State_Type_Definitions,_for_0.26g_versions_and_later_3."True Stop" ("Enum")) -> (s? t:f=w1239:T18)
                n481 = Select(t=w1239, s=w1245, f=State_Type_Definitions,_for_0.26g_versions_and_later_3."Task 5F: ARM GRAB HEIGHT" ("Enum")) -> (s? t:f=w1244:T18)
              }
              frame "Exit" {
                n482 = for {
                  shift-right: [w1267] -> w1264
                  shift-left: w1261 -> [w1268]
                  tunnel: string[] ["STOP", "RESET ENCODERS", "RESET YAW", "ARDUINO MODE 0"] -> [w1266] mode=indexing
                  n483 = Enqueue Element(queue=w1268, element=w1266) -> (queue out=w1267:refnum<queue>)  [unwired: 2 in, 2 out]
                }
              }
            }
          }
          frame "Task 5G: CLOSE CLAW" {
            # ">>> yStepper command>>>"
            # ">> Manual override >>"
            n484 = Dequeue Element(queue=w1279, timeout in ms (-1)=w1278, error in (no error)=w1277) -> (element=w1276:T10)  [unwired: 3 out]
            n485 = case shown="\"Start Task 1\", Default" w1276 {
              tunnel: [w1288 State_Type_Definitions,_for_0.26g_versions_and_later_3."True Stop" ("Enum")] -> w1281
              tunnel: [w1291 w1308] -> w1274
              tunnel: [State_Type_Definitions,_for_0.26g_versions_and_later_3."Idle" ("Enum") State_Type_Definitions,_for_0.26g_versions_and_later_3."Shutdown" ("Enum")] -> w1273
              tunnel: w1275 -> [w1282 _]
              tunnel: w1280 -> [w1287 w1305]
              tunnel: w1271 -> [w1286 _]
              frame "Start Task 1", Default {
                # ">> Is time up? >>"
                # "Determines if object is in range to pick up"
                # ">> Manual override >>"
                n486 = case shown="True" w1286 {
                  tunnel: [w1295 w1301] -> w1291
                  tunnel: w1287 -> [w1293 w1299]
                  frame False {
                    n487 = for {
                      tunnel: string[] ["CLOSE CLAW", "START TIMER"] ("element") -> [w1296] mode=indexing
                      shift-right: [w1298] -> w1295
                      shift-left: w1293 -> [w1297]
                      n488 = Enqueue Element(queue=w1297, element=w1296) -> (queue out=w1298:refnum<queue>)  [unwired: 2 in, 2 out]
                    }
                  }
                  frame True {
                    n489 = for {
                      shift-right: [w1303] -> w1301
                      shift-left: w1299 -> [w1304]
                      tunnel: string[] ["READ STEPPER VALUES", "", ""] -> [w1302] mode=indexing
                      n490 = Enqueue Element(queue=w1304, element=w1302) -> (queue out=w1303:refnum<queue>)  [unwired: 2 in, 2 out]
                    }
                  }
                }
                n491 = Or(x=w1286, y=w1282) -> (x .or. y?=w1289:bool)
                n492 = Select(t=State_Type_Definitions,_for_0.26g_versions_and_later_3."True Stop" ("Enum"), s=w1282, f=State_Type_Definitions,_for_0.26g_versions_and_later_3."Task 5H: RAISE ARM" ("Enum")) -> (s? t:f=w1284:T18)
                n493 = Select(t=w1284, s=w1289, f=State_Type_Definitions,_for_0.26g_versions_and_later_3."Task 5G: CLOSE CLAW" ("Enum")) -> (s? t:f=w1288:T18)
              }
              frame "Exit" {
                n494 = for {
                  shift-right: [w1311] -> w1308
                  shift-left: w1305 -> [w1312]
                  tunnel: string[] ["STOP", "RESET ENCODERS", "RESET YAW", "ARDUINO MODE 0"] -> [w1310] mode=indexing
                  n495 = Enqueue Element(queue=w1312, element=w1310) -> (queue out=w1311:refnum<queue>)  [unwired: 2 in, 2 out]
                }
              }
            }
          }
          frame "Task 5H: RAISE ARM" {
            # ">>> yStepper command>>>"
            # ">> Manual override >>"
            n496 = Dequeue Element(queue=w1323, timeout in ms (-1)=w1322, error in (no error)=w1324) -> (element=w1321:T10)  [unwired: 3 out]
            n497 = Equal?(x=w1320, y=u8 60) -> (x = y?=w1318:bool)
            n498 = case shown="\"Start Task 1\", Default" w1321 {
              tunnel: [w1334 State_Type_Definitions,_for_0.26g_versions_and_later_3."True Stop" ("Enum")] -> w1325
              tunnel: [w1337 w1354] -> w1326
              tunnel: [State_Type_Definitions,_for_0.26g_versions_and_later_3."Idle" ("Enum") State_Type_Definitions,_for_0.26g_versions_and_later_3."Shutdown" ("Enum")] -> w1327
              tunnel: w1318 -> [w1333 _]
              tunnel: w1317 -> [w1332 _]
              tunnel: w1316 -> [w1328 w1351]
              frame "Start Task 1", Default {
                # "Stays in Task 5_A until stepper reaches desired \nheight"
                # "T: Go back to idle, F: Continue with task\""
                # ">> Manual override >>"
                n499 = case shown="False" w1333 {
                  tunnel: [w1341 w1347] -> w1337
                  tunnel: w1328 -> [w1339 w1345]
                  frame False {
                    n500 = for {
                      tunnel: string[] ["Z STEPPER CAM HEIGHT", "READ STEPPER VALUES"] ("element") -> [w1342] mode=indexing
                      shift-right: [w1344] -> w1341
                      shift-left: w1339 -> [w1343]
                      n501 = Enqueue Element(queue=w1343, element=w1342) -> (queue out=w1344:refnum<queue>)  [unwired: 2 in, 2 out]
                    }
                  }
                  frame True {
                    n502 = for {
                      shift-right: [w1349] -> w1347
                      shift-left: w1345 -> [w1350]
                      tunnel: string[] ["ARDUINO - ULTRASONIC", "READ ULTRASONIC", ""] -> [w1348] mode=indexing
                      n503 = Enqueue Element(queue=w1350, element=w1348) -> (queue out=w1349:refnum<queue>)  [unwired: 2 in, 2 out]
                    }
                  }
                }
                n504 = Or(x=w1333, y=w1332) -> (x .or. y?=w1335:bool)
                n505 = Select(t=State_Type_Definitions,_for_0.26g_versions_and_later_3."True Stop" ("Enum"), s=w1332, f=State_Type_Definitions,_for_0.26g_versions_and_later_3."True Stop" ("Enum")) -> (s? t:f=w1329:T18)
                n506 = Select(t=w1329, s=w1335, f=State_Type_Definitions,_for_0.26g_versions_and_later_3."Task 5H: RAISE ARM" ("Enum")) -> (s? t:f=w1334:T18)
              }
              frame "Exit" {
                n507 = for {
                  shift-right: [w1357] -> w1354
                  shift-left: w1351 -> [w1358]
                  tunnel: string[] ["STOP", "RESET ENCODERS", "RESET YAW", "ARDUINO MODE 0"] -> [w1356] mode=indexing
                  n508 = Enqueue Element(queue=w1358, element=w1356) -> (queue out=w1357:refnum<queue>)  [unwired: 2 in, 2 out]
                }
              }
            }
          }
          frame "Task 6A: RAISE ARM" {
            # ">>> Motor control cluster >>>"
            # ">>> yStepper command>>>"
            n509 = Equal?(x=w1366, y=u8 60) -> (x = y?=w1360:bool)
            n510 = Dequeue Element(queue=w1370, timeout in ms (-1)=w1369, error in (no error)=w1368) -> (element=w1375:T10)  [unwired: 3 out]
            n511 = local read "Rising Edge"() -> (w1361:bool)
            n512 = And(x=w1361, y=w1360) -> (x .and. y?=w1359:bool)
            n513 = case shown="\"Start Task 1\", Default" w1375 {
              tunnel: [w1385 State_Type_Definitions,_for_0.26g_versions_and_later_3."True Stop" ("Enum")] -> w1373
              tunnel: [w1384 w1401] -> w1372
              tunnel: [State_Type_Definitions,_for_0.26g_versions_and_later_3."Idle" ("Enum") State_Type_Definitions,_for_0.26g_versions_and_later_3."Shutdown" ("Enum")] -> w1374
              tunnel: w1371 -> [w1381 _]
              tunnel: w1367 -> [w1382 _]
              tunnel: w1359 -> [w1379 _]
              frame "Start Task 1", Default {
                n514 = Or(x=w1379, y=w1381) -> (x .or. y?=w1376:bool)
                n515 = case shown="False" w1376 {
                  tunnel: [w1389 w1395] -> w1384
                  tunnel: w1382 -> [w1387 w1394]
                  frame False {
                    n516 = for {
                      tunnel: string[] ["Z STEPPER CAM HEIGHT", "READ STEPPER VALUES"] ("element") -> [w1390] mode=indexing
                      shift-right: [w1392] -> w1389
                      shift-left: w1387 -> [w1391]
                      n517 = Enqueue Element(queue=w1391, element=w1390) -> (queue out=w1392:refnum<queue>)  [unwired: 2 in, 2 out]
                    }
                  }
                  frame True {
                    n518 = for {
                      shift-right: [w1397] -> w1395
                      shift-left: w1394 -> [w1398]
                      tunnel: string[] ["OPEN LOG CAM", "SET TIMER 2", "OPEN IMAQ REF", "", ""] -> [w1396] mode=indexing
                      n519 = Enqueue Element(queue=w1398, element=w1396) -> (queue out=w1397:refnum<queue>)  [unwired: 2 in, 2 out]
                    }
                  }
                }
                n520 = Select(t=State_Type_Definitions,_for_0.26g_versions_and_later_3."Task 6B: CAM BURST" ("Enum"), s=w1379, f=State_Type_Definitions,_for_0.26g_versions_and_later_3."True Stop" ("Enum")) -> (s? t:f=w1377:T18)
                n521 = Select(t=w1377, s=w1376, f=State_Type_Definitions,_for_0.26g_versions_and_later_3."Task 6A: RAISE ARM" ("Enum")) -> (s? t:f=w1385:T18)
              }
              frame "Exit" {
                n522 = for {
                  shift-right: [w1404] -> w1401
                  shift-left: _ -> [w1405]
                  tunnel: string[] ["STOP", "RESET ENCODERS", "RESET YAW", "ARDUINO MODE 0"] -> [w1403] mode=indexing
                  n523 = Enqueue Element(queue=w1405, element=w1403) -> (queue out=w1404:refnum<queue>)  [unwired: 2 in, 2 out]
                }
              }
            }
          }
          frame "Task 6B: CAM BURST" {
            # ">> Manual override >>"
            # ">>> Motor control cluster >>>"
            # ">>> yStepper command>>>"
            n524 = Dequeue Element(queue=w1417, timeout in ms (-1)=w1415, error in (no error)=w1416) -> (element=w1414:T10)  [unwired: 3 out]
            n525 = case shown="\"Start Task 1\", Default" w1414 {
              tunnel: [w1425 State_Type_Definitions,_for_0.26g_versions_and_later_3."True Stop" ("Enum")] -> w1411
              tunnel: [w1423 w1443] -> w1418
              tunnel: [State_Type_Definitions,_for_0.26g_versions_and_later_3."Idle" ("Enum") State_Type_Definitions,_for_0.26g_versions_and_later_3."Shutdown" ("Enum")] -> w1412
              tunnel: w1413 -> [w1421 _]
              tunnel: w1410 -> [w1422 w1440]
              tunnel: w1406 -> [w1419 _]
              frame "Start Task 1", Default {
                n526 = Or(x=w1419, y=w1421) -> (x .or. y?=w1420:bool)
                n527 = case shown="True" w1420 {
                  tunnel: [w1430 w1436] -> w1423
                  tunnel: w1422 -> [w1428 w1434]
                  frame False {
                    n528 = for {
                      tunnel: string[] ["CAM ACQ", "START TIMER"] ("element") -> [w1431] mode=indexing
                      shift-right: [w1433] -> w1430
                      shift-left: w1428 -> [w1432]
                      n529 = Enqueue Element(queue=w1432, element=w1431) -> (queue out=w1433:refnum<queue>)  [unwired: 2 in, 2 out]
                    }
                  }
                  frame True {
                    n530 = for {
                      shift-right: [w1438] -> w1436
                      shift-left: w1434 -> [w1439]
                      tunnel: string[] ["CAM CLOSE", "PROCESS IMAGE", "SET TIMER 2", "RESET ENCODERS"] -> [w1437] mode=indexing
                      n531 = Enqueue Element(queue=w1439, element=w1437) -> (queue out=w1438:refnum<queue>)  [unwired: 2 in, 2 out]
                    }
                  }
                }
                n532 = Select(t=State_Type_Definitions,_for_0.26g_versions_and_later_3."Task 6C: PROCESS IMAGE" ("Enum"), s=w1420, f=State_Type_Definitions,_for_0.26g_versions_and_later_3."Task 6B: CAM BURST" ("Enum")) -> (s? t:f=w1425:T18)
              }
              frame "Exit" {
                # ">> State after true stop >>"
                # ">> Goes to true stop >>"
                n533 = for {
                  shift-right: [w1446] -> w1443
                  shift-left: w1440 -> [w1447]
                  tunnel: string[] ["STOP", "RESET ENCODERS", "RESET YAW", ""] -> [w1445] mode=indexing
                  n534 = Enqueue Element(queue=w1447, element=w1445) -> (queue out=w1446:refnum<queue>)  [unwired: 2 in, 2 out]
                }
              }
            }
          }
          frame "Task 6C: PROCESS IMAGE" {
            # "Ball > Soap > Gel > Pipe"
            # ">>> Motor control cluster >>>"
            # ">>> yStepper command>>>"
            n535 = Dequeue Element(queue=w1456, timeout in ms (-1)=w1455, error in (no error)=w1454) -> (element=w1453:T10)  [unwired: 3 out]
            n536 = case shown="\"Start Task 1\", Default" w1453 {
              tunnel: [w1472 State_Type_Definitions,_for_0.26g_versions_and_later_3."True Stop" ("Enum")] -> w1460
              tunnel: [w1474 w1491] -> w1459
              tunnel: [State_Type_Definitions,_for_0.26g_versions_and_later_3."Idle" ("Enum") State_Type_Definitions,_for_0.26g_versions_and_later_3."Shutdown" ("Enum")] -> w1461
              tunnel: w1457 -> [w1463 _]
              tunnel: w1458 -> [w1469 w1488]
              tunnel: w1449 -> [w1467 _]
              tunnel: w1448 -> [w1468 _]
              frame "Start Task 1", Default {
                # "Stays in Task 5D until the object is detected"
                n537 = Or(x=w1467, y=w1463) -> (x .or. y?=w1466:bool)
                n538 = case shown="True" w1466 {
                  tunnel: [w1478 w1484] -> w1474
                  tunnel: w1469 -> [w1476 w1482]
                  frame False {
                    n539 = for {
                      tunnel: string[] ["START TIMER", "PROCESS IMAGE", ""] ("element") -> [w1479] mode=indexing
                      shift-right: [w1481] -> w1478
                      shift-left: w1476 -> [w1480]
                      n540 = Enqueue Element(queue=w1480, element=w1479) -> (queue out=w1481:refnum<queue>)  [unwired: 2 in, 2 out]
                    }
                  }
                  frame True {
                    n541 = for {
                      shift-right: [w1486] -> w1484
                      shift-left: w1482 -> [w1487]
                      tunnel: string[] ["RESET ENCODERS", "RESET YAW", ""] -> [w1485] mode=indexing
                      n542 = Enqueue Element(queue=w1487, element=w1485) -> (queue out=w1486:refnum<queue>)  [unwired: 2 in, 2 out]
                    }
                  }
                }
                n543 = Select(t=State_Type_Definitions,_for_0.26g_versions_and_later_3."Task 6D: BALL BUSTER" ("Enum"), s=w1468, f=State_Type_Definitions,_for_0.26g_versions_and_later_3."Task 6F: CAM BURST 2" ("Enum")) -> (s? t:f=w1464:T18)
                n544 = Select(t=State_Type_Definitions,_for_0.26g_versions_and_later_3."True Stop" ("Enum"), s=w1463, f=w1464) -> (s? t:f=w1470:T18)
                n545 = Select(t=w1470, s=w1466, f=State_Type_Definitions,_for_0.26g_versions_and_later_3."Task 6C: PROCESS IMAGE" ("Enum")) -> (s? t:f=w1472:T18)
              }
              frame "Exit" {
                n546 = for {
                  shift-right: [w1494] -> w1491
                  shift-left: w1488 -> [w1495]
                  tunnel: string[] ["STOP", "RESET ENCODERS", "RESET YAW", "ARDUINO MODE 0"] -> [w1493] mode=indexing
                  n547 = Enqueue Element(queue=w1495, element=w1493) -> (queue out=w1494:refnum<queue>)  [unwired: 2 in, 2 out]
                }
              }
            }
          }
          frame "Task 6D: BALL BUSTER" {
            # "Ball > Soap > Gel > Pipe"
            # ">>> Motor control cluster >>>"
            # ">>> yStepper command>>>"
            n548 = Greater Or Equal?(x=w1496, y=20.0) -> (x >= y?=w1497:bool)
            n549 = Dequeue Element(queue=w1505, timeout in ms (-1)=w1504, error in (no error)=w1503) -> (element=w1502:T10)  [unwired: 3 out]
            n550 = case shown="\"Start Task 1\", Default" w1502 {
              tunnel: [w1518 State_Type_Definitions,_for_0.26g_versions_and_later_3."True Stop" ("Enum")] -> w1509
              tunnel: [w1520 w1537] -> w1508
              tunnel: [State_Type_Definitions,_for_0.26g_versions_and_later_3."Idle" ("Enum") State_Type_Definitions,_for_0.26g_versions_and_later_3."Shutdown" ("Enum")] -> w1510
              tunnel: w1506 -> [w1513 _]
              tunnel: w1507 -> [w1515 w1534]
              tunnel: w1497 -> [w1512 _]
              frame "Start Task 1", Default {
                # "Stays in Task 5D until the object is detected"
                n551 = Or(x=w1512, y=w1513) -> (x .or. y?=w1514:bool)
                n552 = case shown="False" w1514 {
                  tunnel: [w1524 w1530] -> w1520
                  tunnel: w1515 -> [w1522 w1528]
                  frame False {
                    n553 = for {
                      tunnel: string[] ["RIGHT", "READ NAVX", "READ ENCODERS"] ("element") -> [w1525] mode=indexing
                      shift-right: [w1527] -> w1524
                      shift-left: w1522 -> [w1526]
                      n554 = Enqueue Element(queue=w1526, element=w1525) -> (queue out=w1527:refnum<queue>)  [unwired: 2 in, 2 out]
                    }
                  }
                  frame True {
                    n555 = for {
                      shift-right: [w1532] -> w1530
                      shift-left: w1528 -> [w1533]
                      tunnel: string[] ["RESET ENCODERS", "RESET YAW", "RESET FLAGS"] -> [w1531] mode=indexing
                      n556 = Enqueue Element(queue=w1533, element=w1531) -> (queue out=w1532:refnum<queue>)  [unwired: 2 in, 2 out]
                    }
                  }
                }
                n557 = Select(t=State_Type_Definitions,_for_0.26g_versions_and_later_3."True Stop" ("Enum"), s=w1513, f=State_Type_Definitions,_for_0.26g_versions_and_later_3."Task 6E: STILL WAITING" ("Enum")) -> (s? t:f=w1516:T18)
                n558 = Select(t=w1516, s=w1514, f=State_Type_Definitions,_for_0.26g_versions_and_later_3."Task 6D: BALL BUSTER" ("Enum")) -> (s? t:f=w1518:T18)
              }
              frame "Exit" {
                n559 = for {
                  shift-right: [w1540] -> w1537
                  shift-left: w1534 -> [w1541]
                  tunnel: string[] ["STOP", "RESET ENCODERS", "RESET YAW", "ARDUINO MODE 0"] -> [w1539] mode=indexing
                  n560 = Enqueue Element(queue=w1541, element=w1539) -> (queue out=w1540:refnum<queue>)  [unwired: 2 in, 2 out]
                }
              }
            }
          }
          frame "Task 6E: STILL WAITING" {
            # "Ball > Soap > Gel > Pipe"
            # ">>> Motor control cluster >>>"
            # ">>> yStepper command>>>"
            n561 = local read "Rising Edge"() -> (w1543:bool)
            n562 = Dequeue Element(queue=w1549, timeout in ms (-1)=w1548, error in (no error)=w1547) -> (element=w1546:T10)  [unwired: 3 out]
            n563 = case shown="\"Start Task 1\", Default" w1546 {
              tunnel: [w1563 State_Type_Definitions,_for_0.26g_versions_and_later_3."True Stop" ("Enum")] -> w1553
              tunnel: [w1556 w1581] -> w1552
              tunnel: [State_Type_Definitions,_for_0.26g_versions_and_later_3."Idle" ("Enum") State_Type_Definitions,_for_0.26g_versions_and_later_3."Shutdown" ("Enum")] -> w1554
              tunnel: w1550 -> [w1560 _]
              tunnel: w1551 -> [w1557 w1578]
              tunnel: w1543 -> [w1558 _]
              frame "Start Task 1", Default {
                # "Stays in Task 5D until the object is detected"
                n564 = Or(x=w1558, y=w1560) -> (x .or. y?=w1555:bool)
                n565 = case shown="False" w1555 {
                  tunnel: [w1568 w1574] -> w1556
                  tunnel: w1557 -> [w1566 w1573]
                  frame False {
                    n566 = for {
                      tunnel: string[] ["Z STEPPER CAM HEIGHT", "READ STEPPER VALUES"] ("element") -> [w1569] mode=indexing
                      shift-right: [w1571] -> w1568
                      shift-left: w1566 -> [w1570]
                      n567 = Enqueue Element(queue=w1570, element=w1569) -> (queue out=w1571:refnum<queue>)  [unwired: 2 in, 2 out]
                    }
                  }
                  frame True {
                    n568 = for {
                      shift-right: [w1576] -> w1574
                      shift-left: w1573 -> [w1577]
                      tunnel: string[] ["OPEN LOG CAM", "SET TIMER 2", "OPEN IMAQ REF", "", ""] -> [w1575] mode=indexing
                      n569 = Enqueue Element(queue=w1577, element=w1575) -> (queue out=w1576:refnum<queue>)  [unwired: 2 in, 2 out]
                    }
                  }
                }
                n570 = Select(t=State_Type_Definitions,_for_0.26g_versions_and_later_3."True Stop" ("Enum"), s=w1560, f=State_Type_Definitions,_for_0.26g_versions_and_later_3."Task 6F: CAM BURST 2" ("Enum")) -> (s? t:f=w1561:T18)
                n571 = Select(t=w1561, s=w1555, f=State_Type_Definitions,_for_0.26g_versions_and_later_3."Task 6E: STILL WAITING" ("Enum")) -> (s? t:f=w1563:T18)
              }
              frame "Exit" {
                n572 = for {
                  shift-right: [w1584] -> w1581
                  shift-left: w1578 -> [w1585]
                  tunnel: string[] ["STOP", "RESET ENCODERS", "RESET YAW", "ARDUINO MODE 0"] -> [w1583] mode=indexing
                  n573 = Enqueue Element(queue=w1585, element=w1583) -> (queue out=w1584:refnum<queue>)  [unwired: 2 in, 2 out]
                }
              }
            }
          }
          frame "Task 6F: CAM BURST 2" {
            # ">> Manual override >>"
            # ">>> Motor control cluster >>>"
            # ">>> yStepper command>>>"
            n574 = Dequeue Element(queue=w1597, timeout in ms (-1)=w1595, error in (no error)=w1596) -> (element=w1594:T10)  [unwired: 3 out]
            n575 = case shown="\"Start Task 1\", Default" w1594 {
              tunnel: [w1605 State_Type_Definitions,_for_0.26g_versions_and_later_3."True Stop" ("Enum")] -> w1591
              tunnel: [w1603 w1623] -> w1598
              tunnel: [State_Type_Definitions,_for_0.26g_versions_and_later_3."Idle" ("Enum") State_Type_Definitions,_for_0.26g_versions_and_later_3."Shutdown" ("Enum")] -> w1592
              tunnel: w1593 -> [w1601 _]
              tunnel: w1590 -> [w1602 w1620]
              tunnel: w1586 -> [w1599 _]
              frame "Start Task 1", Default {
                n576 = Or(x=w1599, y=w1601) -> (x .or. y?=w1600:bool)
                n577 = case shown="True" w1600 {
                  tunnel: [w1610 w1616] -> w1603
                  tunnel: w1602 -> [w1608 w1614]
                  frame False {
                    n578 = for {
                      tunnel: string[] ["CAM ACQ", "START TIMER"] ("element") -> [w1611] mode=indexing
                      shift-right: [w1613] -> w1610
                      shift-left: w1608 -> [w1612]
                      n579 = Enqueue Element(queue=w1612, element=w1611) -> (queue out=w1613:refnum<queue>)  [unwired: 2 in, 2 out]
                    }
                  }
                  frame True {
                    n580 = for {
                      shift-right: [w1618] -> w1616
                      shift-left: w1614 -> [w1619]
                      tunnel: string[] ["CAM CLOSE", "PROCESS IMAGE", "SET TIMER 2", "RESET ENCODERS"] -> [w1617] mode=indexing
                      n581 = Enqueue Element(queue=w1619, element=w1617) -> (queue out=w1618:refnum<queue>)  [unwired: 2 in, 2 out]
                    }
                  }
                }
                n582 = Select(t=State_Type_Definitions,_for_0.26g_versions_and_later_3."Task 6G: PROCESS IMAGE 2" ("Enum"), s=w1600, f=State_Type_Definitions,_for_0.26g_versions_and_later_3."Task 6F: CAM BURST 2" ("Enum")) -> (s? t:f=w1605:T18)
              }
              frame "Exit" {
                # ">> State after true stop >>"
                # ">> Goes to true stop >>"
                n583 = for {
                  shift-right: [w1626] -> w1623
                  shift-left: w1620 -> [w1627]
                  tunnel: string[] ["STOP", "RESET ENCODERS", "RESET YAW", ""] -> [w1625] mode=indexing
                  n584 = Enqueue Element(queue=w1627, element=w1625) -> (queue out=w1626:refnum<queue>)  [unwired: 2 in, 2 out]
                }
              }
            }
          }
          frame "Task 6G: PROCESS IMAGE 2" {
            # "Ball > Soap > Gel > Pipe"
            # ">>> Motor control cluster >>>"
            # ">>> yStepper command>>>"
            n585 = Dequeue Element(queue=w1636, timeout in ms (-1)=w1635, error in (no error)=w1634) -> (element=w1633:T10)  [unwired: 3 out]
            n586 = case shown="\"Start Task 1\", Default" w1633 {
              tunnel: [w1652 State_Type_Definitions,_for_0.26g_versions_and_later_3."True Stop" ("Enum")] -> w1640
              tunnel: [w1654 w1671] -> w1639
              tunnel: [State_Type_Definitions,_for_0.26g_versions_and_later_3."Idle" ("Enum") State_Type_Definitions,_for_0.26g_versions_and_later_3."Shutdown" ("Enum")] -> w1641
              tunnel: w1637 -> [w1643 _]
              tunnel: w1638 -> [w1649 w1668]
              tunnel: w1629 -> [w1647 _]
              tunnel: w1628 -> [w1648 _]
              frame "Start Task 1", Default {
                # "Stays in Task 5D until the object is detected"
                n587 = Or(x=w1647, y=w1643) -> (x .or. y?=w1646:bool)
                n588 = case shown="True" w1646 {
                  tunnel: [w1658 w1664] -> w1654
                  tunnel: w1649 -> [w1656 w1662]
                  frame False {
                    n589 = for {
                      tunnel: string[] ["START TIMER", "PROCESS IMAGE", ""] ("element") -> [w1659] mode=indexing
                      shift-right: [w1661] -> w1658
                      shift-left: w1656 -> [w1660]
                      n590 = Enqueue Element(queue=w1660, element=w1659) -> (queue out=w1661:refnum<queue>)  [unwired: 2 in, 2 out]
                    }
                  }
                  frame True {
                    n591 = for {
                      shift-right: [w1666] -> w1664
                      shift-left: w1662 -> [w1667]
                      tunnel: string[] ["RESET ENCODERS", "RESET YAW", ""] -> [w1665] mode=indexing
                      n592 = Enqueue Element(queue=w1667, element=w1665) -> (queue out=w1666:refnum<queue>)  [unwired: 2 in, 2 out]
                    }
                  }
                }
                n593 = Select(t=State_Type_Definitions,_for_0.26g_versions_and_later_3."Task 6H: SKADI SOAPS" ("Enum"), s=w1648, f=State_Type_Definitions,_for_0.26g_versions_and_later_3."Task 6J: CAM BURST 3" ("Enum")) -> (s? t:f=w1644:T18)
                n594 = Select(t=State_Type_Definitions,_for_0.26g_versions_and_later_3."True Stop" ("Enum"), s=w1643, f=w1644) -> (s? t:f=w1650:T18)
                n595 = Select(t=w1650, s=w1646, f=State_Type_Definitions,_for_0.26g_versions_and_later_3."Task 6G: PROCESS IMAGE 2" ("Enum")) -> (s? t:f=w1652:T18)
              }
              frame "Exit" {
                n596 = for {
                  shift-right: [w1674] -> w1671
                  shift-left: w1668 -> [w1675]
                  tunnel: string[] ["STOP", "RESET ENCODERS", "RESET YAW", "ARDUINO MODE 0"] -> [w1673] mode=indexing
                  n597 = Enqueue Element(queue=w1675, element=w1673) -> (queue out=w1674:refnum<queue>)  [unwired: 2 in, 2 out]
                }
              }
            }
          }
          frame "Task 6H: SKADI SOAPS" {
            # "Ball > Soap > Gel > Pipe"
            # ">>> Motor control cluster >>>"
            # ">>> yStepper command>>>"
            n598 = Less Or Equal?(x=w1676, y=-20.0) -> (x <= y?=w1677:bool)
            n599 = Dequeue Element(queue=w1685, timeout in ms (-1)=w1684, error in (no error)=w1683) -> (element=w1682:T10)  [unwired: 3 out]
            n600 = case shown="\"Start Task 1\", Default" w1682 {
              tunnel: [w1698 State_Type_Definitions,_for_0.26g_versions_and_later_3."True Stop" ("Enum")] -> w1689
              tunnel: [w1700 w1717] -> w1688
              tunnel: [State_Type_Definitions,_for_0.26g_versions_and_later_3."Idle" ("Enum") State_Type_Definitions,_for_0.26g_versions_and_later_3."Shutdown" ("Enum")] -> w1690
              tunnel: w1686 -> [w1693 _]
              tunnel: w1687 -> [w1695 w1714]
              tunnel: w1677 -> [w1692 _]
              frame "Start Task 1", Default {
                # "Stays in Task 5D until the object is detected"
                n601 = Or(x=w1692, y=w1693) -> (x .or. y?=w1694:bool)
                n602 = case shown="False" w1694 {
                  tunnel: [w1704 w1710] -> w1700
                  tunnel: w1695 -> [w1702 w1708]
                  frame False {
                    n603 = for {
                      tunnel: string[] ["LEFT", "READ NAVX", "READ ENCODERS"] ("element") -> [w1705] mode=indexing
                      shift-right: [w1707] -> w1704
                      shift-left: w1702 -> [w1706]
                      n604 = Enqueue Element(queue=w1706, element=w1705) -> (queue out=w1707:refnum<queue>)  [unwired: 2 in, 2 out]
                    }
                  }
                  frame True {
                    n605 = for {
                      shift-right: [w1712] -> w1710
                      shift-left: w1708 -> [w1713]
                      tunnel: string[] ["RESET ENCODERS", "RESET YAW", "RESET FLAGS"] -> [w1711] mode=indexing
                      n606 = Enqueue Element(queue=w1713, element=w1711) -> (queue out=w1712:refnum<queue>)  [unwired: 2 in, 2 out]
                    }
                  }
                }
                n607 = Select(t=State_Type_Definitions,_for_0.26g_versions_and_later_3."True Stop" ("Enum"), s=w1693, f=State_Type_Definitions,_for_0.26g_versions_and_later_3."Task 6I: STILL WAITING 2" ("Enum")) -> (s? t:f=w1696:T18)
                n608 = Select(t=w1696, s=w1694, f=State_Type_Definitions,_for_0.26g_versions_and_later_3."Task 6H: SKADI SOAPS" ("Enum")) -> (s? t:f=w1698:T18)
              }
              frame "Exit" {
                n609 = for {
                  shift-right: [w1720] -> w1717
                  shift-left: w1714 -> [w1721]
                  tunnel: string[] ["STOP", "RESET ENCODERS", "RESET YAW", "ARDUINO MODE 0"] -> [w1719] mode=indexing
                  n610 = Enqueue Element(queue=w1721, element=w1719) -> (queue out=w1720:refnum<queue>)  [unwired: 2 in, 2 out]
                }
              }
            }
          }
          frame "Task 6I: STILL WAITING 2" {
            # "Ball > Soap > Gel > Pipe"
            # ">>> Motor control cluster >>>"
            # ">>> yStepper command>>>"
            n611 = local read "Rising Edge"() -> (w1723:bool)
            n612 = Dequeue Element(queue=w1729, timeout in ms (-1)=w1728, error in (no error)=w1727) -> (element=w1726:T10)  [unwired: 3 out]
            n613 = case shown="\"Start Task 1\", Default" w1726 {
              tunnel: [w1743 State_Type_Definitions,_for_0.26g_versions_and_later_3."True Stop" ("Enum")] -> w1733
              tunnel: [w1736 w1761] -> w1732
              tunnel: [State_Type_Definitions,_for_0.26g_versions_and_later_3."Idle" ("Enum") State_Type_Definitions,_for_0.26g_versions_and_later_3."Shutdown" ("Enum")] -> w1734
              tunnel: w1730 -> [w1740 _]
              tunnel: w1731 -> [w1737 w1758]
              tunnel: w1723 -> [w1738 _]
              frame "Start Task 1", Default {
                # "Stays in Task 5D until the object is detected"
                n614 = Or(x=w1738, y=w1740) -> (x .or. y?=w1735:bool)
                n615 = case shown="False" w1735 {
                  tunnel: [w1748 w1754] -> w1736
                  tunnel: w1737 -> [w1746 w1753]
                  frame False {
                    n616 = for {
                      tunnel: string[] ["Z STEPPER CAM HEIGHT", "READ STEPPER VALUES"] ("element") -> [w1749] mode=indexing
                      shift-right: [w1751] -> w1748
                      shift-left: w1746 -> [w1750]
                      n617 = Enqueue Element(queue=w1750, element=w1749) -> (queue out=w1751:refnum<queue>)  [unwired: 2 in, 2 out]
                    }
                  }
                  frame True {
                    n618 = for {
                      shift-right: [w1756] -> w1754
                      shift-left: w1753 -> [w1757]
                      tunnel: string[] ["OPEN LOG CAM", "SET TIMER 2", "OPEN IMAQ REF", "", ""] -> [w1755] mode=indexing
                      n619 = Enqueue Element(queue=w1757, element=w1755) -> (queue out=w1756:refnum<queue>)  [unwired: 2 in, 2 out]
                    }
                  }
                }
                n620 = Select(t=State_Type_Definitions,_for_0.26g_versions_and_later_3."True Stop" ("Enum"), s=w1740, f=State_Type_Definitions,_for_0.26g_versions_and_later_3."Task 6J: CAM BURST 3" ("Enum")) -> (s? t:f=w1741:T18)
                n621 = Select(t=w1741, s=w1735, f=State_Type_Definitions,_for_0.26g_versions_and_later_3."Task 6I: STILL WAITING 2" ("Enum")) -> (s? t:f=w1743:T18)
              }
              frame "Exit" {
                n622 = for {
                  shift-right: [w1764] -> w1761
                  shift-left: w1758 -> [w1765]
                  tunnel: string[] ["STOP", "RESET ENCODERS", "RESET YAW", "ARDUINO MODE 0"] -> [w1763] mode=indexing
                  n623 = Enqueue Element(queue=w1765, element=w1763) -> (queue out=w1764:refnum<queue>)  [unwired: 2 in, 2 out]
                }
              }
            }
          }
          frame "Task 6J: CAM BURST 3" {
            # ">> Manual override >>"
            # ">>> Motor control cluster >>>"
            # ">>> yStepper command>>>"
            n624 = Dequeue Element(queue=w1777, timeout in ms (-1)=w1775, error in (no error)=w1776) -> (element=w1774:T10)  [unwired: 3 out]
            n625 = case shown="\"Start Task 1\", Default" w1774 {
              tunnel: [w1785 State_Type_Definitions,_for_0.26g_versions_and_later_3."True Stop" ("Enum")] -> w1771
              tunnel: [w1783 w1803] -> w1778
              tunnel: [State_Type_Definitions,_for_0.26g_versions_and_later_3."Idle" ("Enum") State_Type_Definitions,_for_0.26g_versions_and_later_3."Shutdown" ("Enum")] -> w1772
              tunnel: w1773 -> [w1781 _]
              tunnel: w1770 -> [w1782 w1800]
              tunnel: w1766 -> [w1779 _]
              frame "Start Task 1", Default {
                n626 = Or(x=w1779, y=w1781) -> (x .or. y?=w1780:bool)
                n627 = case shown="True" w1780 {
                  tunnel: [w1790 w1796] -> w1783
                  tunnel: w1782 -> [w1788 w1794]
                  frame False {
                    n628 = for {
                      tunnel: string[] ["CAM ACQ", "START TIMER"] ("element") -> [w1791] mode=indexing
                      shift-right: [w1793] -> w1790
                      shift-left: w1788 -> [w1792]
                      n629 = Enqueue Element(queue=w1792, element=w1791) -> (queue out=w1793:refnum<queue>)  [unwired: 2 in, 2 out]
                    }
                  }
                  frame True {
                    n630 = for {
                      shift-right: [w1798] -> w1796
                      shift-left: w1794 -> [w1799]
                      tunnel: string[] ["CAM CLOSE", "PROCESS IMAGE", "SET TIMER 2", "RESET ENCODERS"] -> [w1797] mode=indexing
                      n631 = Enqueue Element(queue=w1799, element=w1797) -> (queue out=w1798:refnum<queue>)  [unwired: 2 in, 2 out]
                    }
                  }
                }
                n632 = Select(t=State_Type_Definitions,_for_0.26g_versions_and_later_3."Task 6K: PROCESS IMAGE 3" ("Enum"), s=w1780, f=State_Type_Definitions,_for_0.26g_versions_and_later_3."Task 6J: CAM BURST 3" ("Enum")) -> (s? t:f=w1785:T18)
              }
              frame "Exit" {
                # ">> State after true stop >>"
                # ">> Goes to true stop >>"
                n633 = for {
                  shift-right: [w1806] -> w1803
                  shift-left: w1800 -> [w1807]
                  tunnel: string[] ["STOP", "RESET ENCODERS", "RESET YAW", ""] -> [w1805] mode=indexing
                  n634 = Enqueue Element(queue=w1807, element=w1805) -> (queue out=w1806:refnum<queue>)  [unwired: 2 in, 2 out]
                }
              }
            }
          }
          frame "Task 6K: PROCESS IMAGE 3" {
            # "Ball > Soap > Gel > Pipe"
            # ">>> Motor control cluster >>>"
            # ">>> yStepper command>>>"
            n635 = Dequeue Element(queue=w1816, timeout in ms (-1)=w1815, error in (no error)=w1814) -> (element=w1813:T10)  [unwired: 3 out]
            n636 = case shown="\"Start Task 1\", Default" w1813 {
              tunnel: [w1832 State_Type_Definitions,_for_0.26g_versions_and_later_3."True Stop" ("Enum")] -> w1820
              tunnel: [w1834 w1851] -> w1819
              tunnel: [State_Type_Definitions,_for_0.26g_versions_and_later_3."Idle" ("Enum") State_Type_Definitions,_for_0.26g_versions_and_later_3."Shutdown" ("Enum")] -> w1821
              tunnel: w1817 -> [w1823 _]
              tunnel: w1818 -> [w1829 w1848]
              tunnel: w1809 -> [w1827 _]
              tunnel: w1808 -> [w1828 _]
              frame "Start Task 1", Default {
                # "Stays in Task 5D until the object is detected"
                n637 = Or(x=w1827, y=w1823) -> (x .or. y?=w1826:bool)
                n638 = case shown="True" w1826 {
                  tunnel: [w1838 w1844] -> w1834
                  tunnel: w1829 -> [w1836 w1842]
                  frame False {
                    n639 = for {
                      tunnel: string[] ["START TIMER", "PROCESS IMAGE", ""] ("element") -> [w1839] mode=indexing
                      shift-right: [w1841] -> w1838
                      shift-left: w1836 -> [w1840]
                      n640 = Enqueue Element(queue=w1840, element=w1839) -> (queue out=w1841:refnum<queue>)  [unwired: 2 in, 2 out]
                    }
                  }
                  frame True {
                    n641 = for {
                      shift-right: [w1846] -> w1844
                      shift-left: w1842 -> [w1847]
                      tunnel: string[] ["RESET ENCODERS", "RESET YAW", ""] -> [w1845] mode=indexing
                      n642 = Enqueue Element(queue=w1847, element=w1845) -> (queue out=w1846:refnum<queue>)  [unwired: 2 in, 2 out]
                    }
                  }
                }
                n643 = Select(t=State_Type_Definitions,_for_0.26g_versions_and_later_3."Task 6L: JAM IT IN" ("Enum"), s=w1828, f=State_Type_Definitions,_for_0.26g_versions_and_later_3."Task 6N: CAM BURST 4" ("Enum")) -> (s? t:f=w1824:T18)
                n644 = Select(t=State_Type_Definitions,_for_0.26g_versions_and_later_3."True Stop" ("Enum"), s=w1823, f=w1824) -> (s? t:f=w1830:T18)
                n645 = Select(t=w1830, s=w1826, f=State_Type_Definitions,_for_0.26g_versions_and_later_3."Task 6K: PROCESS IMAGE 3" ("Enum")) -> (s? t:f=w1832:T18)
              }
              frame "Exit" {
                n646 = for {
                  shift-right: [w1854] -> w1851
                  shift-left: w1848 -> [w1855]
                  tunnel: string[] ["STOP", "RESET ENCODERS", "RESET YAW", "ARDUINO MODE 0"] -> [w1853] mode=indexing
                  n647 = Enqueue Element(queue=w1855, element=w1853) -> (queue out=w1854:refnum<queue>)  [unwired: 2 in, 2 out]
                }
              }
            }
          }
          frame "Task 6L: JAM IT IN" {
            # "Ball > Soap > Gel > Pipe"
            # ">>> Motor control cluster >>>"
            # ">>> yStepper command>>>"
            n648 = Less Or Equal?(x=w1856, y=-20.0) -> (x <= y?=w1857:bool)
            n649 = Dequeue Element(queue=w1865, timeout in ms (-1)=w1864, error in (no error)=w1863) -> (element=w1862:T10)  [unwired: 3 out]
            n650 = case shown="\"Start Task 1\", Default" w1862 {
              tunnel: [w1878 State_Type_Definitions,_for_0.26g_versions_and_later_3."True Stop" ("Enum")] -> w1869
              tunnel: [w1880 w1897] -> w1868
              tunnel: [State_Type_Definitions,_for_0.26g_versions_and_later_3."Idle" ("Enum") State_Type_Definitions,_for_0.26g_versions_and_later_3."Shutdown" ("Enum")] -> w1870
              tunnel: w1866 -> [w1873 _]
              tunnel: w1867 -> [w1875 w1894]
              tunnel: w1857 -> [w1872 _]
              frame "Start Task 1", Default {
                # "Stays in Task 5D until the object is detected"
                n651 = Or(x=w1872, y=w1873) -> (x .or. y?=w1874:bool)
                n652 = case shown="False" w1874 {
                  tunnel: [w1884 w1890] -> w1880
                  tunnel: w1875 -> [w1882 w1888]
                  frame False {
                    n653 = for {
                      tunnel: string[] ["REVERSE", "READ NAVX", "READ ENCODERS"] ("element") -> [w1885] mode=indexing
                      shift-right: [w1887] -> w1884
                      shift-left: w1882 -> [w1886]
                      n654 = Enqueue Element(queue=w1886, element=w1885) -> (queue out=w1887:refnum<queue>)  [unwired: 2 in, 2 out]
                    }
                  }
                  frame True {
                    n655 = for {
                      shift-right: [w1892] -> w1890
                      shift-left: w1888 -> [w1893]
                      tunnel: string[] ["RESET ENCODERS", "RESET YAW", "RESET FLAGS"] -> [w1891] mode=indexing
                      n656 = Enqueue Element(queue=w1893, element=w1891) -> (queue out=w1892:refnum<queue>)  [unwired: 2 in, 2 out]
                    }
                  }
                }
                n657 = Select(t=State_Type_Definitions,_for_0.26g_versions_and_later_3."True Stop" ("Enum"), s=w1873, f=State_Type_Definitions,_for_0.26g_versions_and_later_3."Task 6M: STILL WAITING 3" ("Enum")) -> (s? t:f=w1876:T18)
                n658 = Select(t=w1876, s=w1874, f=State_Type_Definitions,_for_0.26g_versions_and_later_3."Task 6L: JAM IT IN" ("Enum")) -> (s? t:f=w1878:T18)
              }
              frame "Exit" {
                n659 = for {
                  shift-right: [w1900] -> w1897
                  shift-left: w1894 -> [w1901]
                  tunnel: string[] ["STOP", "RESET ENCODERS", "RESET YAW", "ARDUINO MODE 0"] -> [w1899] mode=indexing
                  n660 = Enqueue Element(queue=w1901, element=w1899) -> (queue out=w1900:refnum<queue>)  [unwired: 2 in, 2 out]
                }
              }
            }
          }
          frame "Task 6M: STILL WAITING 3" {
            # "Ball > Soap > Gel > Pipe"
            # ">>> Motor control cluster >>>"
            # ">>> yStepper command>>>"
            n661 = local read "Rising Edge"() -> (w1903:bool)
            n662 = Dequeue Element(queue=w1909, timeout in ms (-1)=w1908, error in (no error)=w1907) -> (element=w1906:T10)  [unwired: 3 out]
            n663 = case shown="\"Start Task 1\", Default" w1906 {
              tunnel: [w1923 State_Type_Definitions,_for_0.26g_versions_and_later_3."True Stop" ("Enum")] -> w1913
              tunnel: [w1916 w1941] -> w1912
              tunnel: [State_Type_Definitions,_for_0.26g_versions_and_later_3."Idle" ("Enum") State_Type_Definitions,_for_0.26g_versions_and_later_3."Shutdown" ("Enum")] -> w1914
              tunnel: w1910 -> [w1920 _]
              tunnel: w1911 -> [w1917 w1938]
              tunnel: w1903 -> [w1918 _]
              frame "Start Task 1", Default {
                # "Stays in Task 5D until the object is detected"
                n664 = Or(x=w1918, y=w1920) -> (x .or. y?=w1915:bool)
                n665 = case shown="False" w1915 {
                  tunnel: [w1928 w1934] -> w1916
                  tunnel: w1917 -> [w1926 w1933]
                  frame False {
                    n666 = for {
                      tunnel: string[] ["Z STEPPER CAM HEIGHT", "READ STEPPER VALUES"] ("element") -> [w1929] mode=indexing
                      shift-right: [w1931] -> w1928
                      shift-left: w1926 -> [w1930]
                      n667 = Enqueue Element(queue=w1930, element=w1929) -> (queue out=w1931:refnum<queue>)  [unwired: 2 in, 2 out]
                    }
                  }
                  frame True {
                    n668 = for {
                      shift-right: [w1936] -> w1934
                      shift-left: w1933 -> [w1937]
                      tunnel: string[] ["OPEN LOG CAM", "SET TIMER 2", "OPEN IMAQ REF", "", ""] -> [w1935] mode=indexing
                      n669 = Enqueue Element(queue=w1937, element=w1935) -> (queue out=w1936:refnum<queue>)  [unwired: 2 in, 2 out]
                    }
                  }
                }
                n670 = Select(t=State_Type_Definitions,_for_0.26g_versions_and_later_3."True Stop" ("Enum"), s=w1920, f=State_Type_Definitions,_for_0.26g_versions_and_later_3."Task 6N: CAM BURST 4" ("Enum")) -> (s? t:f=w1921:T18)
                n671 = Select(t=w1921, s=w1915, f=State_Type_Definitions,_for_0.26g_versions_and_later_3."Task 6M: STILL WAITING 3" ("Enum")) -> (s? t:f=w1923:T18)
              }
              frame "Exit" {
                n672 = for {
                  shift-right: [w1944] -> w1941
                  shift-left: w1938 -> [w1945]
                  tunnel: string[] ["STOP", "RESET ENCODERS", "RESET YAW", "ARDUINO MODE 0"] -> [w1943] mode=indexing
                  n673 = Enqueue Element(queue=w1945, element=w1943) -> (queue out=w1944:refnum<queue>)  [unwired: 2 in, 2 out]
                }
              }
            }
          }
          frame "Task 6N: CAM BURST 4" {
            # ">> Manual override >>"
            # ">>> Motor control cluster >>>"
            # ">>> yStepper command>>>"
            n674 = Dequeue Element(queue=w1957, timeout in ms (-1)=w1955, error in (no error)=w1956) -> (element=w1954:T10)  [unwired: 3 out]
            n675 = case shown="\"Start Task 1\", Default" w1954 {
              tunnel: [w1965 State_Type_Definitions,_for_0.26g_versions_and_later_3."True Stop" ("Enum")] -> w1951
              tunnel: [w1963 w1983] -> w1958
              tunnel: [State_Type_Definitions,_for_0.26g_versions_and_later_3."Idle" ("Enum") State_Type_Definitions,_for_0.26g_versions_and_later_3."Shutdown" ("Enum")] -> w1952
              tunnel: w1953 -> [w1961 _]
              tunnel: w1950 -> [w1962 w1980]
              tunnel: w1946 -> [w1959 _]
              frame "Start Task 1", Default {
                n676 = Or(x=w1959, y=w1961) -> (x .or. y?=w1960:bool)
                n677 = case shown="True" w1960 {
                  tunnel: [w1970 w1976] -> w1963
                  tunnel: w1962 -> [w1968 w1974]
                  frame False {
                    n678 = for {
                      tunnel: string[] ["CAM ACQ", "START TIMER"] ("element") -> [w1971] mode=indexing
                      shift-right: [w1973] -> w1970
                      shift-left: w1968 -> [w1972]
                      n679 = Enqueue Element(queue=w1972, element=w1971) -> (queue out=w1973:refnum<queue>)  [unwired: 2 in, 2 out]
                    }
                  }
                  frame True {
                    n680 = for {
                      shift-right: [w1978] -> w1976
                      shift-left: w1974 -> [w1979]
                      tunnel: string[] ["CAM CLOSE", "PROCESS IMAGE", "SET TIMER 2", "RESET ENCODERS"] -> [w1977] mode=indexing
                      n681 = Enqueue Element(queue=w1979, element=w1977) -> (queue out=w1978:refnum<queue>)  [unwired: 2 in, 2 out]
                    }
                  }
                }
                n682 = Select(t=State_Type_Definitions,_for_0.26g_versions_and_later_3."Task 6O: PROCESS IMAGE 4" ("Enum"), s=w1960, f=State_Type_Definitions,_for_0.26g_versions_and_later_3."Task 6N: CAM BURST 4" ("Enum")) -> (s? t:f=w1965:T18)
              }
              frame "Exit" {
                # ">> State after true stop >>"
                # ">> Goes to true stop >>"
                n683 = for {
                  shift-right: [w1986] -> w1983
                  shift-left: w1980 -> [w1987]
                  tunnel: string[] ["STOP", "RESET ENCODERS", "RESET YAW", ""] -> [w1985] mode=indexing
                  n684 = Enqueue Element(queue=w1987, element=w1985) -> (queue out=w1986:refnum<queue>)  [unwired: 2 in, 2 out]
                }
              }
            }
          }
          frame "Task 6O: PROCESS IMAGE 4" {
            # "Ball > Soap > Gel > Pipe"
            # ">>> Motor control cluster >>>"
            # ">>> yStepper command>>>"
            n685 = Dequeue Element(queue=w1996, timeout in ms (-1)=w1995, error in (no error)=w1994) -> (element=w1993:T10)  [unwired: 3 out]
            n686 = case shown="\"Start Task 1\", Default" w1993 {
              tunnel: [w2012 State_Type_Definitions,_for_0.26g_versions_and_later_3."True Stop" ("Enum")] -> w2000
              tunnel: [w2014 w2031] -> w1999
              tunnel: [State_Type_Definitions,_for_0.26g_versions_and_later_3."Idle" ("Enum") State_Type_Definitions,_for_0.26g_versions_and_later_3."Shutdown" ("Enum")] -> w2001
              tunnel: w1997 -> [w2003 _]
              tunnel: w1998 -> [w2009 w2028]
              tunnel: w1989 -> [w2007 _]
              tunnel: w1988 -> [w2008 _]
              frame "Start Task 1", Default {
                # "Stays in Task 5D until the object is detected"
                n687 = Or(x=w2007, y=w2003) -> (x .or. y?=w2006:bool)
                n688 = case shown="True" w2006 {
                  tunnel: [w2018 w2024] -> w2014
                  tunnel: w2009 -> [w2016 w2022]
                  frame False {
                    n689 = for {
                      tunnel: string[] ["START TIMER", "PROCESS IMAGE", ""] ("element") -> [w2019] mode=indexing
                      shift-right: [w2021] -> w2018
                      shift-left: w2016 -> [w2020]
                      n690 = Enqueue Element(queue=w2020, element=w2019) -> (queue out=w2021:refnum<queue>)  [unwired: 2 in, 2 out]
                    }
                  }
                  frame True {
                    n691 = for {
                      shift-right: [w2026] -> w2024
                      shift-left: w2022 -> [w2027]
                      tunnel: string[] ["RESET ENCODERS", "RESET YAW", ""] -> [w2025] mode=indexing
                      n692 = Enqueue Element(queue=w2027, element=w2025) -> (queue out=w2026:refnum<queue>)  [unwired: 2 in, 2 out]
                    }
                  }
                }
                n693 = Select(t=State_Type_Definitions,_for_0.26g_versions_and_later_3."Task 6P: PIPE BOMB" ("Enum"), s=w2008, f=State_Type_Definitions,_for_0.26g_versions_and_later_3."Task 6B: CAM BURST" ("Enum")) -> (s? t:f=w2004:T18)
                n694 = Select(t=State_Type_Definitions,_for_0.26g_versions_and_later_3."True Stop" ("Enum"), s=w2003, f=w2004) -> (s? t:f=w2010:T18)
                n695 = Select(t=w2010, s=w2006, f=State_Type_Definitions,_for_0.26g_versions_and_later_3."Task 6O: PROCESS IMAGE 4" ("Enum")) -> (s? t:f=w2012:T18)
              }
              frame "Exit" {
                n696 = for {
                  shift-right: [w2034] -> w2031
                  shift-left: w2028 -> [w2035]
                  tunnel: string[] ["STOP", "RESET ENCODERS", "RESET YAW", "ARDUINO MODE 0"] -> [w2033] mode=indexing
                  n697 = Enqueue Element(queue=w2035, element=w2033) -> (queue out=w2034:refnum<queue>)  [unwired: 2 in, 2 out]
                }
              }
            }
          }
          frame "Task 6P: PIPE BOMB" {
            # "Ball > Soap > Gel > Pipe"
            # ">>> Motor control cluster >>>"
            # ">>> yStepper command>>>"
            n698 = Greater Or Equal?(x=w2036, y=20.0) -> (x >= y?=w2037:bool)
            n699 = Dequeue Element(queue=w2045, timeout in ms (-1)=w2044, error in (no error)=w2043) -> (element=w2042:T10)  [unwired: 3 out]
            n700 = case shown="\"Start Task 1\", Default" w2042 {
              tunnel: [w2058 State_Type_Definitions,_for_0.26g_versions_and_later_3."True Stop" ("Enum")] -> w2049
              tunnel: [w2060 w2077] -> w2048
              tunnel: [State_Type_Definitions,_for_0.26g_versions_and_later_3."Idle" ("Enum") State_Type_Definitions,_for_0.26g_versions_and_later_3."Shutdown" ("Enum")] -> w2050
              tunnel: w2046 -> [w2053 _]
              tunnel: w2047 -> [w2055 w2074]
              tunnel: w2037 -> [w2052 _]
              frame "Start Task 1", Default {
                # "Stays in Task 5D until the object is detected"
                n701 = Or(x=w2052, y=w2053) -> (x .or. y?=w2054:bool)
                n702 = case shown="False" w2054 {
                  tunnel: [w2064 w2070] -> w2060
                  tunnel: w2055 -> [w2062 w2068]
                  frame False {
                    n703 = for {
                      tunnel: string[] ["FORWARD", "READ NAVX", "READ ENCODERS"] ("element") -> [w2065] mode=indexing
                      shift-right: [w2067] -> w2064
                      shift-left: w2062 -> [w2066]
                      n704 = Enqueue Element(queue=w2066, element=w2065) -> (queue out=w2067:refnum<queue>)  [unwired: 2 in, 2 out]
                    }
                  }
                  frame True {
                    n705 = for {
                      shift-right: [w2072] -> w2070
                      shift-left: w2068 -> [w2073]
                      tunnel: string[] ["RESET ENCODERS", "RESET YAW", "RESET FLAGS"] -> [w2071] mode=indexing
                      n706 = Enqueue Element(queue=w2073, element=w2071) -> (queue out=w2072:refnum<queue>)  [unwired: 2 in, 2 out]
                    }
                  }
                }
                n707 = Select(t=State_Type_Definitions,_for_0.26g_versions_and_later_3."True Stop" ("Enum"), s=w2053, f=State_Type_Definitions,_for_0.26g_versions_and_later_3."Task 5F: ARM GRAB HEIGHT" ("Enum")) -> (s? t:f=w2056:T18)
                n708 = Select(t=w2056, s=w2054, f=State_Type_Definitions,_for_0.26g_versions_and_later_3."Task 6P: PIPE BOMB" ("Enum")) -> (s? t:f=w2058:T18)
              }
              frame "Exit" {
                n709 = for {
                  shift-right: [w2080] -> w2077
                  shift-left: w2074 -> [w2081]
                  tunnel: string[] ["STOP", "RESET ENCODERS", "RESET YAW", "ARDUINO MODE 0"] -> [w2079] mode=indexing
                  n710 = Enqueue Element(queue=w2081, element=w2079) -> (queue out=w2080:refnum<queue>)  [unwired: 2 in, 2 out]
                }
              }
            }
          }
          frame "Task 7" {
          }
          frame "Task 8A: RAISE ARM" {
            # ">>> Motor control cluster >>>"
            # ">>> yStepper command>>>"
            # ">> Manual override >>"
            n711 = Dequeue Element(queue=w2098, timeout in ms (-1)=w2097, error in (no error)=w2099) -> (element=w2096:T10)  [unwired: 3 out]
            n712 = Equal?(x=w2095, y=u8 60) -> (x = y?=w2093:bool)
            n713 = case shown="\"Start Task 1\", Default" w2096 {
              tunnel: [w2109 State_Type_Definitions,_for_0.26g_versions_and_later_3."True Stop" ("Enum")] -> w2100
              tunnel: [w2112 w2129] -> w2101
              tunnel: [State_Type_Definitions,_for_0.26g_versions_and_later_3."Idle" ("Enum") State_Type_Definitions,_for_0.26g_versions_and_later_3."Shutdown" ("Enum")] -> w2102
              tunnel: w2093 -> [w2108 _]
              tunnel: w2092 -> [w2107 _]
              tunnel: w2091 -> [w2103 w2126]
              frame "Start Task 1", Default {
                # "Stays in Task 5_A until stepper reaches desired \nheight"
                # "T: Go back to idle, F: Continue with task\""
                # ">> Manual override >>"
                n714 = case shown="False" w2108 {
                  tunnel: [w2116 w2122] -> w2112
                  tunnel: w2103 -> [w2114 w2120]
                  frame False {
                    n715 = for {
                      tunnel: string[] ["Z STEPPER CAM HEIGHT", "READ STEPPER VALUES", "READ IR"] ("element") -> [w2117] mode=indexing
                      shift-right: [w2119] -> w2116
                      shift-left: w2114 -> [w2118]
                      n716 = Enqueue Element(queue=w2118, element=w2117) -> (queue out=w2119:refnum<queue>)  [unwired: 2 in, 2 out]
                    }
                  }
                  frame True {
                    n717 = for {
                      shift-right: [w2124] -> w2122
                      shift-left: w2120 -> [w2125]
                      tunnel: string[] ["RESET YAW", "RESET ENCODERS", "READ IR"] -> [w2123] mode=indexing
                      n718 = Enqueue Element(queue=w2125, element=w2123) -> (queue out=w2124:refnum<queue>)  [unwired: 2 in, 2 out]
                    }
                  }
                }
                n719 = Or(x=w2108, y=w2107) -> (x .or. y?=w2110:bool)
                n720 = Select(t=State_Type_Definitions,_for_0.26g_versions_and_later_3."True Stop" ("Enum"), s=w2107, f=State_Type_Definitions,_for_0.26g_versions_and_later_3."Task 8B: MOVE TO BOX" ("Enum")) -> (s? t:f=w2104:T18)
                n721 = Select(t=w2104, s=w2110, f=State_Type_Definitions,_for_0.26g_versions_and_later_3."Task 8A: RAISE ARM" ("Enum")) -> (s? t:f=w2109:T18)
              }
              frame "Exit" {
                n722 = for {
                  shift-right: [w2132] -> w2129
                  shift-left: w2126 -> [w2133]
                  tunnel: string[] ["STOP", "RESET ENCODERS", "RESET YAW", "ARDUINO MODE 0"] -> [w2131] mode=indexing
                  n723 = Enqueue Element(queue=w2133, element=w2131) -> (queue out=w2132:refnum<queue>)  [unwired: 2 in, 2 out]
                }
              }
            }
          }
          frame "Task 8B: MOVE TO BOX" {
            w2143 = u8 15 ("y")
            # "High voltage: 70"
            # ">>> yStepper command>>>"
            n724 = Less?(x=w2140, y=w2143) -> (x < y?=w2141:bool)
            n725 = Less?(x=w2139, y=w2143) -> (x < y?=w2142:bool)
            n726 = And(x=w2142, y=w2141) -> ()  [unwired: 1 out]
            n727 = Dequeue Element(queue=w2147, timeout in ms (-1)=w2146, error in (no error)=w2148) -> (element=w2145:T10)  [unwired: 3 out]
            n728 = Less?(x=w2136, y=40.0) -> (x < y?=w2134:bool)
            n729 = case shown="\"Start Task 1\", Default" w2145 {
              tunnel: [w2160 State_Type_Definitions,_for_0.26g_versions_and_later_3."True Stop" ("Enum")] -> w2150
              tunnel: [w2163 w2180] -> w2149
              tunnel: [State_Type_Definitions,_for_0.26g_versions_and_later_3."Idle" ("Enum") State_Type_Definitions,_for_0.26g_versions_and_later_3."Shutdown" ("Enum")] -> w2151
              tunnel: w2153 -> [w2159 _]
              tunnel: w2152 -> [w2155 w2177]
              tunnel: w2134 -> [w2154 _]
              frame "Start Task 1", Default {
                # "Stays in Task 5_B to capture image over 5 seconds"
                # "T: Go back to idle, F: Continue with task\""
                # ">> Manual override >>"
                n730 = case shown="True" w2154 {
                  tunnel: [w2167 w2173] -> w2163
                  tunnel: w2155 -> [w2165 w2171]
                  frame False {
                    n731 = for {
                      tunnel: string[] ["FORWARD", "READ IR", "READ NAVX"] ("element") -> [w2168] mode=indexing
                      shift-right: [w2170] -> w2167
                      shift-left: w2165 -> [w2169]
                      n732 = Enqueue Element(queue=w2169, element=w2168) -> (queue out=w2170:refnum<queue>)  [unwired: 2 in, 2 out]
                    }
                  }
                  frame True {
                    n733 = for {
                      shift-right: [w2175] -> w2173
                      shift-left: w2171 -> [w2176]
                      tunnel: string[] ["STOP", "RESET ENCODERS", "OPEN LOG CAM", "SET TIMER 2", "OPEN IMAQ REF"] -> [w2174] mode=indexing
                      n734 = Enqueue Element(queue=w2176, element=w2174) -> (queue out=w2175:refnum<queue>)  [unwired: 2 in, 2 out]
                    }
                  }
                }
                n735 = Or(x=w2154, y=w2159) -> (x .or. y?=w2161:bool)
                n736 = Select(t=State_Type_Definitions,_for_0.26g_versions_and_later_3."True Stop" ("Enum"), s=w2159, f=State_Type_Definitions,_for_0.26g_versions_and_later_3."Task 8C: CAM BURST" ("Enum")) -> (s? t:f=w2156:T18)
                n737 = Select(t=w2156, s=w2161, f=State_Type_Definitions,_for_0.26g_versions_and_later_3."Task 8B: MOVE TO BOX" ("Enum")) -> (s? t:f=w2160:T18)
              }
              frame "Exit" {
                n738 = for {
                  shift-right: [w2183] -> w2180
                  shift-left: w2177 -> [w2184]
                  tunnel: string[] ["STOP", "RESET ENCODERS", "RESET YAW", "ARDUINO MODE 0"] -> [w2182] mode=indexing
                  n739 = Enqueue Element(queue=w2184, element=w2182) -> (queue out=w2183:refnum<queue>)  [unwired: 2 in, 2 out]
                }
              }
            }
          }
          frame "Task 8C: CAM BURST" {
            # ">>> Motor control cluster >>>"
            # ">>> yStepper command>>>"
            # ">> Manual override >>"
            n740 = Dequeue Element(queue=w2195, timeout in ms (-1)=w2194, error in (no error)=w2193) -> (element=w2192:T10)  [unwired: 3 out]
            n741 = case shown="\"Start Task 1\", Default" w2192 {
              tunnel: [w2204 State_Type_Definitions,_for_0.26g_versions_and_later_3."True Stop" ("Enum")] -> w2197
              tunnel: [w2207 w2224] -> w2190
              tunnel: [State_Type_Definitions,_for_0.26g_versions_and_later_3."Idle" ("Enum") State_Type_Definitions,_for_0.26g_versions_and_later_3."Shutdown" ("Enum")] -> w2189
              tunnel: w2191 -> [w2198 _]
              tunnel: w2196 -> [w2203 w2221]
              tunnel: w2187 -> [w2202 _]
              frame "Start Task 1", Default {
                # ">> Is time up? >>"
                # "Determines if object is in range to pick up"
                # ">> Manual override >>"
                n742 = case shown="True" w2202 {
                  tunnel: [w2211 w2217] -> w2207
                  tunnel: w2203 -> [w2209 w2215]
                  frame False {
                    n743 = for {
                      tunnel: string[] ["CAM ACQ", "START TIMER"] ("element") -> [w2212] mode=indexing
                      shift-right: [w2214] -> w2211
                      shift-left: w2209 -> [w2213]
                      n744 = Enqueue Element(queue=w2213, element=w2212) -> (queue out=w2214:refnum<queue>)  [unwired: 2 in, 2 out]
                    }
                  }
                  frame True {
                    n745 = for {
                      shift-right: [w2219] -> w2217
                      shift-left: w2215 -> [w2220]
                      tunnel: string[] ["CAM CLOSE", "PROCESS IMAGE", "SET TIMER 2"] -> [w2218] mode=indexing
                      n746 = Enqueue Element(queue=w2220, element=w2218) -> (queue out=w2219:refnum<queue>)  [unwired: 2 in, 2 out]
                    }
                  }
                }
                n747 = Or(x=w2202, y=w2198) -> (x .or. y?=w2205:bool)
                n748 = Select(t=State_Type_Definitions,_for_0.26g_versions_and_later_3."True Stop" ("Enum"), s=w2198, f=State_Type_Definitions,_for_0.26g_versions_and_later_3."Task 8D: PROCESS IMAGE" ("Enum")) -> (s? t:f=w2200:T18)
                n749 = Select(t=w2200, s=w2205, f=State_Type_Definitions,_for_0.26g_versions_and_later_3."Task 8C: CAM BURST" ("Enum")) -> (s? t:f=w2204:T18)
              }
              frame "Exit" {
                n750 = for {
                  shift-right: [w2227] -> w2224
                  shift-left: w2221 -> [w2228]
                  tunnel: string[] ["STOP", "RESET ENCODERS", "RESET YAW", "ARDUINO MODE 0"] -> [w2226] mode=indexing
                  n751 = Enqueue Element(queue=w2228, element=w2226) -> (queue out=w2227:refnum<queue>)  [unwired: 2 in, 2 out]
                }
              }
            }
          }
          frame "Task 8D: PROCESS IMAGE" {
            # ">>> Motor control cluster >>>"
            # ">>> yStepper command>>>"
            n752 = Dequeue Element(queue=w2237, timeout in ms (-1)=w2236, error in (no error)=w2235) -> (element=w2234:T10)  [unwired: 3 out]
            n753 = case shown="\"Start Task 1\", Default" w2234 {
              tunnel: [w2252 State_Type_Definitions,_for_0.26g_versions_and_later_3."True Stop" ("Enum")] -> w2241
              tunnel: [w2255 w2272] -> w2240
              tunnel: [State_Type_Definitions,_for_0.26g_versions_and_later_3."Idle" ("Enum") State_Type_Definitions,_for_0.26g_versions_and_later_3."Shutdown" ("Enum")] -> w2242
              tunnel: w2238 -> [w2251 _]
              tunnel: w2239 -> [w2248 w2269]
              tunnel: w2229 -> [w2247 _]
              tunnel: w2230 -> [w2246 _]
              frame "Start Task 1", Default {
                # ">> T: Breaks out of state loop; F: Stays in loop>>"
                # ">> Manual override >>"
                # ">> Checks if time is up>>"
                # "Stays in Task 5D until the object is detected"
                # "T: Go back to idle, F: Continue with task\""
                # ">> Manual override >>"
                n754 = case shown="False" w2247 {
                  tunnel: [w2259 w2265] -> w2255
                  tunnel: w2248 -> [w2257 w2263]
                  frame False {
                    n755 = for {
                      tunnel: string[] ["START TIMER", "PROCESS IMAGE", ""] ("element") -> [w2260] mode=indexing
                      shift-right: [w2262] -> w2259
                      shift-left: w2257 -> [w2261]
                      n756 = Enqueue Element(queue=w2261, element=w2260) -> (queue out=w2262:refnum<queue>)  [unwired: 2 in, 2 out]
                    }
                  }
                  frame True {
                    n757 = for {
                      shift-right: [w2267] -> w2265
                      shift-left: w2263 -> [w2268]
                      tunnel: string[] ["RESET ENCODERS", "", ""] -> [w2266] mode=indexing
                      n758 = Enqueue Element(queue=w2268, element=w2266) -> (queue out=w2267:refnum<queue>)  [unwired: 2 in, 2 out]
                    }
                  }
                }
                n759 = Or(x=w2247, y=w2251) -> (x .or. y?=w2253:bool)
                n760 = Select(t=State_Type_Definitions,_for_0.26g_versions_and_later_3."Task 8E: ROBOT ADJUST" ("Enum"), s=w2246, f=State_Type_Definitions,_for_0.26g_versions_and_later_3."True Stop" ("Enum")) -> (s? t:f=w2243:T18)
                n761 = Select(t=State_Type_Definitions,_for_0.26g_versions_and_later_3."True Stop" ("Enum"), s=w2251, f=w2243) -> (s? t:f=w2249:T18)
                n762 = Select(t=w2249, s=w2253, f=State_Type_Definitions,_for_0.26g_versions_and_later_3."Task 8D: PROCESS IMAGE" ("Enum")) -> (s? t:f=w2252:T18)
              }
              frame "Exit" {
                n763 = for {
                  shift-right: [w2275] -> w2272
                  shift-left: w2269 -> [w2276]
                  tunnel: string[] ["STOP", "RESET ENCODERS", "RESET YAW", "ARDUINO MODE 0"] -> [w2274] mode=indexing
                  n764 = Enqueue Element(queue=w2276, element=w2274) -> (queue out=w2275:refnum<queue>)  [unwired: 2 in, 2 out]
                }
              }
            }
          }
          frame "Task 8E: ROBOT ADJUST" {
            # ">>> Motor control cluster >>>"
            # ">>> yStepper command>>>"
            n765 = Dequeue Element(queue=w2294, timeout in ms (-1)=w2293, error in (no error)=w2292) -> (element=w2291:T10)  [unwired: 3 out]
            n766 = Subtract(x=w2289, y=150.0) -> (x-y=w2287:dbl)
            n767 = formula code="if (error <= -100 && error < -80){\n    distance = -20;\n    xSpeed = -30;\n}\n\nelse if (error <= -80 && error < -60){\n    distance = -18;\n    xSpeed = -30;\n}\n\nelse if (error <= -60 && error < -40){\n    distance = -15;\n    xSpeed = -30;\n}\n\nelse if (error <= -40 && error < -20){\n    distance = -10;\n    xSpeed = -30;\n}\n\nelse if (error <= -20 && error < -10){\n    distance = 5;\n    xSpeed = -30;\n}\n\nelse if (error <= -10 && error <= 10){\n    distance = 0;\n    xSpeed = 0;\n}\n\nelse if (error <= 20 && error < 40){\n    distance = 5;\n    xSpeed = 30;\n}\n\nelse if (error <= 40 && error < 60){\n    distance = 10;\n    xSpeed = 30;\n}\n\nelse if (error <= 60 && error < 80){\n    distance = 15;\n    xSpeed = 30;\n}\n\nelse if (error <= 80 && error < 100){\n    distance = 18;\n    xSpeed = 30;\n}\n\nelse if (error <= 100){\n    distance = 20;\n    xSpeed = 30;\n}\n\nelse {\n    distance = 0;\n    xSpeed = 0;\n}"("error"=w2287) -> ("distance"=w2277:dbl, "xSpeed"=w2284:dbl)
            n768 = formula code="if (target > 0){\nif (current  >= target)\noutput = 1;\n\nelse if (current != target)\noutput = 0;\n}\n\nelse if (target == 0){\nif (current == target)\noutput = 1;\n\nelse if (current != target)\noutput = 0;\n}\n\nelse if (target < 0){\nif (current <= target)\noutput = 1;\n\nelse if (current != target)\noutput = 0;\n}\n\nelse if (current != target)\noutput = 0;"("target"=w2277, "current"=w2283) -> ("output"=w2282:dbl)
            n769 = call "yDistance travelled FGV.vi"("Init/Read/Write State"=States_for_Action_Engine."Write", "yDistance travelled"=w2277) -> ()  [unwired: 8 in, 2 out]
            n770 = Bundle By Name(cluster=w2286, "xSpeed"=w2284) -> (w2285:T20)
            n771 = Equal?(x=w2282, y=1.0) -> (x = y?=w2279:bool)
            n772 = case shown="\"Start Task 1\", Default" w2291 {
              tunnel: [w2306 State_Type_Definitions,_for_0.26g_versions_and_later_3."True Stop" ("Enum")] -> w2298
              tunnel: [w2309 w2326] -> w2297
              tunnel: [State_Type_Definitions,_for_0.26g_versions_and_later_3."Idle" ("Enum") State_Type_Definitions,_for_0.26g_versions_and_later_3."Shutdown" ("Enum")] -> w2299
              tunnel: w2295 -> [w2305 _]
              tunnel: w2296 -> [w2301 w2323]
              tunnel: w2279 -> [w2300 _]
              frame "Start Task 1", Default {
                # ">> T: Breaks out of state loop; F: Stays in loop>>"
                # ">> Manual override >>"
                # ">> Checks if time is up>>"
                # "Stays in Task 5D until the object is detected"
                # "T: Go back to idle, F: Continue with task\""
                # ">> Manual override >>"
                n773 = case shown="True" w2300 {
                  tunnel: [w2313 w2319] -> w2309
                  tunnel: w2301 -> [w2311 w2317]
                  frame False {
                    n774 = for {
                      tunnel: string[] ["X AXIS - SLOW", "READ ENCODERS", "READ NAVX"] ("element") -> [w2314] mode=indexing
                      shift-right: [w2316] -> w2313
                      shift-left: w2311 -> [w2315]
                      n775 = Enqueue Element(queue=w2315, element=w2314) -> (queue out=w2316:refnum<queue>)  [unwired: 2 in, 2 out]
                    }
                  }
                  frame True {
                    n776 = for {
                      shift-right: [w2321] -> w2319
                      shift-left: w2317 -> [w2322]
                      tunnel: string[] ["SET TIMER 2", "STOP", "READ STEPPER VALUES", ""] -> [w2320] mode=indexing
                      n777 = Enqueue Element(queue=w2322, element=w2320) -> (queue out=w2321:refnum<queue>)  [unwired: 2 in, 2 out]
                    }
                  }
                }
                n778 = Or(x=w2300, y=w2305) -> (x .or. y?=w2307:bool)
                n779 = Select(t=State_Type_Definitions,_for_0.26g_versions_and_later_3."True Stop" ("Enum"), s=w2305, f=State_Type_Definitions,_for_0.26g_versions_and_later_3."Task 8H: ARM ADJUST" ("Enum")) -> (s? t:f=w2302:T18)
                n780 = Select(t=w2302, s=w2307, f=State_Type_Definitions,_for_0.26g_versions_and_later_3."Task 8E: ROBOT ADJUST" ("Enum")) -> (s? t:f=w2306:T18)
              }
              frame "Exit" {
                n781 = for {
                  shift-right: [w2329] -> w2326
                  shift-left: w2323 -> [w2330]
                  tunnel: string[] ["STOP", "RESET ENCODERS", "RESET YAW", "ARDUINO MODE 0"] -> [w2328] mode=indexing
                  n782 = Enqueue Element(queue=w2330, element=w2328) -> (queue out=w2329:refnum<queue>)  [unwired: 2 in, 2 out]
                }
              }
            }
          }
          frame "Task 8F: CAM BURST 2" {
            # ">>> Motor control cluster >>>"
            # ">>> yStepper command>>>"
            # ">> Manual override >>"
            n783 = Dequeue Element(queue=w2341, timeout in ms (-1)=w2340, error in (no error)=w2339) -> (element=w2338:T10)  [unwired: 3 out]
            n784 = case shown="\"Start Task 1\", Default" w2338 {
              tunnel: [w2350 State_Type_Definitions,_for_0.26g_versions_and_later_3."True Stop" ("Enum")] -> w2343
              tunnel: [w2353 w2370] -> w2336
              tunnel: [State_Type_Definitions,_for_0.26g_versions_and_later_3."Idle" ("Enum") State_Type_Definitions,_for_0.26g_versions_and_later_3."Shutdown" ("Enum")] -> w2335
              tunnel: w2337 -> [w2344 _]
              tunnel: w2342 -> [w2349 w2367]
              tunnel: w2333 -> [w2348 _]
              frame "Start Task 1", Default {
                # ">> Is time up? >>"
                # "Determines if object is in range to pick up"
                # ">> Manual override >>"
                n785 = case shown="False" w2348 {
                  tunnel: [w2357 w2363] -> w2353
                  tunnel: w2349 -> [w2355 w2361]
                  frame False {
                    n786 = for {
                      tunnel: string[] ["CAM ACQ", "START TIMER"] ("element") -> [w2358] mode=indexing
                      shift-right: [w2360] -> w2357
                      shift-left: w2355 -> [w2359]
                      n787 = Enqueue Element(queue=w2359, element=w2358) -> (queue out=w2360:refnum<queue>)  [unwired: 2 in, 2 out]
                    }
                  }
                  frame True {
                    n788 = for {
                      shift-right: [w2365] -> w2363
                      shift-left: w2361 -> [w2366]
                      tunnel: string[] ["CAM CLOSE", "PROCESS IMAGE", "SET TIMER 3"] -> [w2364] mode=indexing
                      n789 = Enqueue Element(queue=w2366, element=w2364) -> (queue out=w2365:refnum<queue>)  [unwired: 2 in, 2 out]
                    }
                  }
                }
                n790 = Or(x=w2348, y=w2344) -> (x .or. y?=w2351:bool)
                n791 = Select(t=State_Type_Definitions,_for_0.26g_versions_and_later_3."True Stop" ("Enum"), s=w2344, f=State_Type_Definitions,_for_0.26g_versions_and_later_3."Task 8G: PROCESS IMAGE 2" ("Enum")) -> (s? t:f=w2346:T18)
                n792 = Select(t=w2346, s=w2351, f=State_Type_Definitions,_for_0.26g_versions_and_later_3."Task 8F: CAM BURST 2" ("Enum")) -> (s? t:f=w2350:T18)
              }
              frame "Exit" {
                n793 = for {
                  shift-right: [w2373] -> w2370
                  shift-left: w2367 -> [w2374]
                  tunnel: string[] ["STOP", "RESET ENCODERS", "RESET YAW", "ARDUINO MODE 0"] -> [w2372] mode=indexing
                  n794 = Enqueue Element(queue=w2374, element=w2372) -> (queue out=w2373:refnum<queue>)  [unwired: 2 in, 2 out]
                }
              }
            }
          }
          frame "Task 8G: PROCESS IMAGE 2" {
            # ">>> yStepper command>>>"
            n795 = Dequeue Element(queue=w2382, timeout in ms (-1)=w2381, error in (no error)=w2380) -> (element=w2379:T10)  [unwired: 3 out]
            n796 = case shown="\"Start Task 1\", Default" w2379 {
              tunnel: [w2394 State_Type_Definitions,_for_0.26g_versions_and_later_3."True Stop" ("Enum")] -> w2386
              tunnel: [w2397 w2414] -> w2385
              tunnel: [State_Type_Definitions,_for_0.26g_versions_and_later_3."Idle" ("Enum") State_Type_Definitions,_for_0.26g_versions_and_later_3."Shutdown" ("Enum")] -> w2387
              tunnel: w2383 -> [w2393 _]
              tunnel: w2384 -> [w2389 w2411]
              tunnel: w2377 -> [w2388 _]
              frame "Start Task 1", Default {
                # ">> T: Breaks out of state loop; F: Stays in loop>>"
                # ">> Manual override >>"
                # ">> Checks if time is up>>"
                # "Stays in Task 5D until the object is detected"
                # "T: Go back to idle, F: Continue with task\""
                # ">> Manual override >>"
                n797 = case shown="False" w2388 {
                  tunnel: [w2401 w2407] -> w2397
                  tunnel: w2389 -> [w2399 w2405]
                  frame False {
                    n798 = for {
                      tunnel: string[] ["START TIMER", "PROCESS IMAGE", ""] ("element") -> [w2402] mode=indexing
                      shift-right: [w2404] -> w2401
                      shift-left: w2399 -> [w2403]
                      n799 = Enqueue Element(queue=w2403, element=w2402) -> (queue out=w2404:refnum<queue>)  [unwired: 2 in, 2 out]
                    }
                  }
                  frame True {
                    n800 = for {
                      shift-right: [w2409] -> w2407
                      shift-left: w2405 -> [w2410]
                      tunnel: string[] ["READ STEPPER VALUES", "Y STEPPER CONTROL", ""] -> [w2408] mode=indexing
                      n801 = Enqueue Element(queue=w2410, element=w2408) -> (queue out=w2409:refnum<queue>)  [unwired: 2 in, 2 out]
                    }
                  }
                }
                n802 = Or(x=w2388, y=w2393) -> (x .or. y?=w2395:bool)
                n803 = Select(t=State_Type_Definitions,_for_0.26g_versions_and_later_3."True Stop" ("Enum"), s=w2393, f=State_Type_Definitions,_for_0.26g_versions_and_later_3."Task 8H: ARM ADJUST" ("Enum")) -> (s? t:f=w2390:T18)
                n804 = Select(t=w2390, s=w2395, f=State_Type_Definitions,_for_0.26g_versions_and_later_3."Task 8G: PROCESS IMAGE 2" ("Enum")) -> (s? t:f=w2394:T18)
              }
              frame "Exit" {
                n805 = for {
                  shift-right: [w2417] -> w2414
                  shift-left: w2411 -> [w2418]
                  tunnel: string[] ["STOP", "RESET ENCODERS", "RESET YAW", "ARDUINO MODE 0"] -> [w2416] mode=indexing
                  n806 = Enqueue Element(queue=w2418, element=w2416) -> (queue out=w2417:refnum<queue>)  [unwired: 2 in, 2 out]
                }
              }
            }
          }
          frame "Task 8H: ARM ADJUST" {
            # ">>> yStepper command>>>"
            n807 = Dequeue Element(queue=w2433, timeout in ms (-1)=w2434, error in (no error)=w2435) -> (element=w2437:T10)  [unwired: 3 out]
            n808 = formula code="if (pos >= 40 && pos < 80)\ny = 40;\n\nelse if (pos >= 80 && pos < 100)\ny = 35;\n\nelse if (pos >= 100 && pos < 120)\ny = 20;\n\nelse if (pos >= 120 && pos < 140)\ny = 15;\n\nelse if (pos >= 140 && pos < 150)\ny = 10;\n\nelse if (pos >= 150 && 170)\ny = 5;\n\nelse \ny = 0;"("pos"=w2425) -> ("y"=w2428:dbl)
            n809 = To Unsigned Byte Integer(number=w2428) -> (unsigned 8bit integer=w2423:u8)
            n810 = Equal?(x=w2424, y=w2423) -> (x = y?=w2422:bool)
            n811 = case shown="\"Start Task 1\", Default" w2437 {
              tunnel: [w2446 State_Type_Definitions,_for_0.26g_versions_and_later_3."True Stop" ("Enum")] -> w2431
              tunnel: [w2449 w2466] -> w2429
              tunnel: [State_Type_Definitions,_for_0.26g_versions_and_later_3."Idle" ("Enum") State_Type_Definitions,_for_0.26g_versions_and_later_3."Shutdown" ("Enum")] -> w2430
              tunnel: w2436 -> [w2440 _]
              tunnel: w2432 -> [w2442 w2463]
              tunnel: w2422 -> [w2441 _]
              tunnel: w2419 -> [w2439 _]
              frame "Start Task 1", Default {
                # ">> T: Breaks out of state loop; F: Stays in loop>>"
                # ">> Manual override >>"
                # ">> Checks if time is up>>"
                # "Stays in Task 5D until the object is detected"
                # "T: Go back to idle, F: Continue with task\""
                # ">> Manual override >>"
                n812 = Or(x=w2439, y=w2440) -> (x .or. y?=w2438:bool)
                n813 = case shown="False" w2441 {
                  tunnel: [w2453 w2459] -> w2449
                  tunnel: w2442 -> [w2451 w2457]
                  frame False {
                    n814 = for {
                      tunnel: string[] ["READ STEPPER VALUES", "Y STEPPER CONTROL", ""] ("element") -> [w2454] mode=indexing
                      shift-right: [w2456] -> w2453
                      shift-left: w2451 -> [w2455]
                      n815 = Enqueue Element(queue=w2455, element=w2454) -> (queue out=w2456:refnum<queue>)  [unwired: 2 in, 2 out]
                    }
                  }
                  frame True {
                    n816 = for {
                      shift-right: [w2461] -> w2459
                      shift-left: w2457 -> [w2462]
                      tunnel: string[] ["DISPOSE BUFFERS", "READ STEPPER VALUES", ""] -> [w2460] mode=indexing
                      n817 = Enqueue Element(queue=w2462, element=w2460) -> (queue out=w2461:refnum<queue>)  [unwired: 2 in, 2 out]
                    }
                  }
                }
                n818 = Or(x=w2441, y=w2440) -> (x .or. y?=w2447:bool)
                n819 = Select(t=State_Type_Definitions,_for_0.26g_versions_and_later_3."True Stop" ("Enum"), s=w2438, f=State_Type_Definitions,_for_0.26g_versions_and_later_3."Task 8I: ARM GRAB HEIGHT" ("Enum")) -> (s? t:f=w2443:T18)
                n820 = Select(t=w2443, s=w2447, f=State_Type_Definitions,_for_0.26g_versions_and_later_3."Task 8H: ARM ADJUST" ("Enum")) -> (s? t:f=w2446:T18)
              }
              frame "Exit" {
                n821 = for {
                  shift-right: [w2469] -> w2466
                  shift-left: w2463 -> [w2470]
                  tunnel: string[] ["STOP", "RESET ENCODERS", "RESET YAW", "ARDUINO MODE 0"] -> [w2468] mode=indexing
                  n822 = Enqueue Element(queue=w2470, element=w2468) -> (queue out=w2469:refnum<queue>)  [unwired: 2 in, 2 out]
                }
              }
            }
            n823 = Bundle By Name(cluster=w2427, "yStepper desired"=w2423) -> (w2426:T21)
          }
          frame "Task 8I: ARM GRAB HEIGHT" {
            # ">>> Motor control cluster >>>"
            # ">>> yStepper command>>>"
            # ">> Manual override >>"
            n824 = Dequeue Element(queue=w2481, timeout in ms (-1)=w2480, error in (no error)=w2482) -> (element=w2479:T10)  [unwired: 3 out]
            n825 = Equal?(x=w2478, y=u8 1) -> (x = y?=w2476:bool)
            n826 = case shown="\"Start Task 1\", Default" w2479 {
              tunnel: [w2492 State_Type_Definitions,_for_0.26g_versions_and_later_3."True Stop" ("Enum")] -> w2483
              tunnel: [w2495 w2512] -> w2484
              tunnel: [State_Type_Definitions,_for_0.26g_versions_and_later_3."Idle" ("Enum") State_Type_Definitions,_for_0.26g_versions_and_later_3."Shutdown" ("Enum")] -> w2485
              tunnel: w2476 -> [w2491 _]
              tunnel: w2475 -> [w2490 _]
              tunnel: w2474 -> [w2486 w2509]
              frame "Start Task 1", Default {
                # "Stays in Task 5F until stepper reaches desired \nheight"
                # "T: Go back to idle, F: Continue with task\""
                # ">> Manual override >>"
                n827 = case shown="True" w2491 {
                  tunnel: [w2499 w2505] -> w2495
                  tunnel: w2486 -> [w2497 w2503]
                  frame False {
                    n828 = for {
                      tunnel: string[] ["Z STEPPER GRAB HEIGHT", "READ STEPPER VALUES"] ("element") -> [w2500] mode=indexing
                      shift-right: [w2502] -> w2499
                      shift-left: w2497 -> [w2501]
                      n829 = Enqueue Element(queue=w2501, element=w2500) -> (queue out=w2502:refnum<queue>)  [unwired: 2 in, 2 out]
                    }
                  }
                  frame True {
                    n830 = for {
                      shift-right: [w2507] -> w2505
                      shift-left: w2503 -> [w2508]
                      tunnel: string[] ["SET TIMER 2", "CLOSE CLAW", ""] -> [w2506] mode=indexing
                      n831 = Enqueue Element(queue=w2508, element=w2506) -> (queue out=w2507:refnum<queue>)  [unwired: 2 in, 2 out]
                    }
                  }
                }
                n832 = Or(x=w2491, y=w2490) -> (x .or. y?=w2493:bool)
                n833 = Select(t=State_Type_Definitions,_for_0.26g_versions_and_later_3."True Stop" ("Enum"), s=w2490, f=State_Type_Definitions,_for_0.26g_versions_and_later_3."Task 8J: CLOSE CLAW" ("Enum")) -> (s? t:f=w2487:T18)
                n834 = Select(t=w2487, s=w2493, f=State_Type_Definitions,_for_0.26g_versions_and_later_3."Task 8I: ARM GRAB HEIGHT" ("Enum")) -> (s? t:f=w2492:T18)
              }
              frame "Exit" {
                n835 = for {
                  shift-right: [w2515] -> w2512
                  shift-left: w2509 -> [w2516]
                  tunnel: string[] ["STOP", "RESET ENCODERS", "RESET YAW", "ARDUINO MODE 0"] -> [w2514] mode=indexing
                  n836 = Enqueue Element(queue=w2516, element=w2514) -> (queue out=w2515:refnum<queue>)  [unwired: 2 in, 2 out]
                }
              }
            }
          }
          frame "Task 8J: CLOSE CLAW" {
            # ">>> yStepper command>>>"
            # ">> Manual override >>"
            n837 = Dequeue Element(queue=w2527, timeout in ms (-1)=w2526, error in (no error)=w2525) -> (element=w2524:T10)  [unwired: 3 out]
            n838 = case shown="\"Start Task 1\", Default" w2524 {
              tunnel: [w2536 State_Type_Definitions,_for_0.26g_versions_and_later_3."True Stop" ("Enum")] -> w2529
              tunnel: [w2539 w2556] -> w2522
              tunnel: [State_Type_Definitions,_for_0.26g_versions_and_later_3."Idle" ("Enum") State_Type_Definitions,_for_0.26g_versions_and_later_3."Shutdown" ("Enum")] -> w2521
              tunnel: w2523 -> [w2530 _]
              tunnel: w2528 -> [w2535 w2553]
              tunnel: w2519 -> [w2534 _]
              frame "Start Task 1", Default {
                # ">> Is time up? >>"
                # "Determines if object is in range to pick up"
                # ">> Manual override >>"
                n839 = case shown="True" w2534 {
                  tunnel: [w2543 w2549] -> w2539
                  tunnel: w2535 -> [w2541 w2547]
                  frame False {
                    n840 = for {
                      tunnel: string[] ["CLOSE CLAW", "START TIMER"] ("element") -> [w2544] mode=indexing
                      shift-right: [w2546] -> w2543
                      shift-left: w2541 -> [w2545]
                      n841 = Enqueue Element(queue=w2545, element=w2544) -> (queue out=w2546:refnum<queue>)  [unwired: 2 in, 2 out]
                    }
                  }
                  frame True {
                    n842 = for {
                      shift-right: [w2551] -> w2549
                      shift-left: w2547 -> [w2552]
                      tunnel: string[] ["READ STEPPER VALUES", "", ""] -> [w2550] mode=indexing
                      n843 = Enqueue Element(queue=w2552, element=w2550) -> (queue out=w2551:refnum<queue>)  [unwired: 2 in, 2 out]
                    }
                  }
                }
                n844 = Or(x=w2534, y=w2530) -> (x .or. y?=w2537:bool)
                n845 = Select(t=State_Type_Definitions,_for_0.26g_versions_and_later_3."True Stop" ("Enum"), s=w2530, f=State_Type_Definitions,_for_0.26g_versions_and_later_3."Task 8K: RAISE MY SWORD" ("Enum")) -> (s? t:f=w2532:T18)
                n846 = Select(t=w2532, s=w2537, f=State_Type_Definitions,_for_0.26g_versions_and_later_3."Task 8J: CLOSE CLAW" ("Enum")) -> (s? t:f=w2536:T18)
              }
              frame "Exit" {
                n847 = for {
                  shift-right: [w2559] -> w2556
                  shift-left: w2553 -> [w2560]
                  tunnel: string[] ["STOP", "RESET ENCODERS", "RESET YAW", "ARDUINO MODE 0"] -> [w2558] mode=indexing
                  n848 = Enqueue Element(queue=w2560, element=w2558) -> (queue out=w2559:refnum<queue>)  [unwired: 2 in, 2 out]
                }
              }
            }
          }
          frame "Task 8K: RAISE MY SWORD" {
            # ">>> Motor control cluster >>>"
            # ">>> yStepper command>>>"
            # ">> Manual override >>"
            n849 = Dequeue Element(queue=w2571, timeout in ms (-1)=w2570, error in (no error)=w2572) -> (element=w2569:T10)  [unwired: 3 out]
            n850 = Equal?(x=w2568, y=u8 60) -> (x = y?=w2566:bool)
            n851 = case shown="\"Start Task 1\", Default" w2569 {
              tunnel: [w2582 State_Type_Definitions,_for_0.26g_versions_and_later_3."True Stop" ("Enum")] -> w2573
              tunnel: [w2585 w2602] -> w2574
              tunnel: [State_Type_Definitions,_for_0.26g_versions_and_later_3."Idle" ("Enum") State_Type_Definitions,_for_0.26g_versions_and_later_3."Shutdown" ("Enum")] -> w2575
              tunnel: w2566 -> [w2581 _]
              tunnel: w2565 -> [w2580 _]
              tunnel: w2564 -> [w2576 w2599]
              frame "Start Task 1", Default {
                # "Stays in Task 5_A until stepper reaches desired \nheight"
                # "T: Go back to idle, F: Continue with task\""
                # ">> Manual override >>"
                n852 = case shown="True" w2581 {
                  tunnel: [w2589 w2595] -> w2585
                  tunnel: w2576 -> [w2587 w2593]
                  frame False {
                    n853 = for {
                      tunnel: string[] ["Z STEPPER CAM HEIGHT", "READ STEPPER VALUES"] ("element") -> [w2590] mode=indexing
                      shift-right: [w2592] -> w2589
                      shift-left: w2587 -> [w2591]
                      n854 = Enqueue Element(queue=w2591, element=w2590) -> (queue out=w2592:refnum<queue>)  [unwired: 2 in, 2 out]
                    }
                  }
                  frame True {
                    n855 = for {
                      shift-right: [w2597] -> w2595
                      shift-left: w2593 -> [w2598]
                      tunnel: string[] ["CAM CLOSE", "DISPOSE CAM BUFFERS", "DISPOSE PROC BUFFERS", "RESET FLAGS"] -> [w2596] mode=indexing
                      n856 = Enqueue Element(queue=w2598, element=w2596) -> (queue out=w2597:refnum<queue>)  [unwired: 2 in, 2 out]
                    }
                  }
                }
                n857 = Or(x=w2581, y=w2580) -> (x .or. y?=w2583:bool)
                n858 = Select(t=State_Type_Definitions,_for_0.26g_versions_and_later_3."True Stop" ("Enum"), s=w2580, f=State_Type_Definitions,_for_0.26g_versions_and_later_3."Task 8I: STILL WAITING" ("Enum")) -> (s? t:f=w2577:T18)
                n859 = Select(t=w2577, s=w2583, f=State_Type_Definitions,_for_0.26g_versions_and_later_3."Task 8K: RAISE MY SWORD" ("Enum")) -> (s? t:f=w2582:T18)
              }
              frame "Exit" {
                n860 = for {
                  shift-right: [w2605] -> w2602
                  shift-left: w2599 -> [w2606]
                  tunnel: string[] ["STOP", "RESET ENCODERS", "RESET YAW", "ARDUINO MODE 0"] -> [w2604] mode=indexing
                  n861 = Enqueue Element(queue=w2606, element=w2604) -> (queue out=w2605:refnum<queue>)  [unwired: 2 in, 2 out]
                }
              }
            }
          }
          frame "Task 8I: STILL WAITING" {
            # ">>> Motor control cluster >>>"
            # ">>> yStepper command>>>"
            # ">> Manual override >>"
            n862 = Dequeue Element(queue=w2614, timeout in ms (-1)=w2613, error in (no error)=w2615) -> (element=w2612:T10)  [unwired: 3 out]
            n863 = case shown="\"Start Task 1\", Default" w2612 {
              tunnel: [w2622 State_Type_Definitions,_for_0.26g_versions_and_later_3."True Stop" ("Enum")] -> w2616
              tunnel: [w2624 w2641] -> w2617
              tunnel: [State_Type_Definitions,_for_0.26g_versions_and_later_3."Idle" ("Enum") State_Type_Definitions,_for_0.26g_versions_and_later_3."Shutdown" ("Enum")] -> w2618
              tunnel: w2611 -> [w2619 _]
              tunnel: w2610 -> [w2620 w2638]
              frame "Start Task 1", Default {
                # "Stays in Task 5_A until stepper reaches desired \nheight"
                # "T: Go back to idle, F: Continue with task\""
                # ">> Manual override >>"
                n864 = case shown="True" w2619 {
                  tunnel: [w2628 w2634] -> w2624
                  tunnel: w2620 -> [w2626 w2632]
                  frame False {
                    n865 = for {
                      tunnel: string[] ["READ NAVX", "READ IR"] ("element") -> [w2629] mode=indexing
                      shift-right: [w2631] -> w2628
                      shift-left: w2626 -> [w2630]
                      n866 = Enqueue Element(queue=w2630, element=w2629) -> (queue out=w2631:refnum<queue>)  [unwired: 2 in, 2 out]
                    }
                  }
                  frame True {
                    n867 = for {
                      shift-right: [w2636] -> w2634
                      shift-left: w2632 -> [w2637]
                      tunnel: string[] ["RESET ENCODERS", "RESET YAW", "RESET FLAGS", ""] -> [w2635] mode=indexing
                      n868 = Enqueue Element(queue=w2637, element=w2635) -> (queue out=w2636:refnum<queue>)  [unwired: 2 in, 2 out]
                    }
                  }
                }
                n869 = Select(t=State_Type_Definitions,_for_0.26g_versions_and_later_3."True Stop" ("Enum"), s=w2619, f=State_Type_Definitions,_for_0.26g_versions_and_later_3."Task 8I: STILL WAITING" ("Enum")) -> (s? t:f=w2622:T18)
              }
              frame "Exit" {
                n870 = for {
                  shift-right: [w2644] -> w2641
                  shift-left: w2638 -> [w2645]
                  tunnel: string[] ["STOP", "RESET ENCODERS", "RESET YAW", "ARDUINO MODE 0"] -> [w2643] mode=indexing
                  n871 = Enqueue Element(queue=w2645, element=w2643) -> (queue out=w2644:refnum<queue>)  [unwired: 2 in, 2 out]
                }
              }
            }
          }
          frame "Task 8L: Return to position" {
            # ">>> Motor control cluster >>>"
            # ">>> yStepper command>>>"
            # ">> Manual override >>"
            n872 = call "yDistance travelled FGV.vi"("Init/Read/Write State"=States_for_Action_Engine."Read") -> ("Output"=w2650:dbl)  [unwired: 9 in, 1 out]
            n873 = Dequeue Element(queue=w2659, timeout in ms (-1)=w2658, error in (no error)=w2660) -> (element=w2657:T10)  [unwired: 3 out]
            n874 = Multiply(x=w2650, y=-1.0) -> (x*y=w2647:dbl)
            n875 = Less Or Equal?(x=w2648, y=w2647) -> (x <= y?=w2646:bool)
            n876 = case shown="\"Start Task 1\", Default" w2657 {
              tunnel: [w2669 State_Type_Definitions,_for_0.26g_versions_and_later_3."True Stop" ("Enum")] -> w2661
              tunnel: [w2671 w2688] -> w2662
              tunnel: [State_Type_Definitions,_for_0.26g_versions_and_later_3."Idle" ("Enum") State_Type_Definitions,_for_0.26g_versions_and_later_3."Shutdown" ("Enum")] -> w2663
              tunnel: w2656 -> [w2665 _]
              tunnel: w2655 -> [w2667 w2685]
              tunnel: w2646 -> [w2666 _]
              frame "Start Task 1", Default {
                # "Stays in Task 5_A until stepper reaches desired \nheight"
                # "T: Go back to idle, F: Continue with task\""
                # ">> Manual override >>"
                n877 = Or(x=w2666, y=w2665) -> (x .or. y?=w2664:bool)
                n878 = case shown="False" w2664 {
                  tunnel: [w2675 w2681] -> w2671
                  tunnel: w2667 -> [w2673 w2679]
                  frame False {
                    n879 = for {
                      tunnel: string[] ["READ NAVX", "LEFT"] ("element") -> [w2676] mode=indexing
                      shift-right: [w2678] -> w2675
                      shift-left: w2673 -> [w2677]
                      n880 = Enqueue Element(queue=w2677, element=w2676) -> (queue out=w2678:refnum<queue>)  [unwired: 2 in, 2 out]
                    }
                  }
                  frame True {
                    n881 = for {
                      shift-right: [w2683] -> w2681
                      shift-left: w2679 -> [w2684]
                      tunnel: string[] ["RESET ENCODERS", "RESET YAW", "RESET FLAGS", ""] -> [w2682] mode=indexing
                      n882 = Enqueue Element(queue=w2684, element=w2682) -> (queue out=w2683:refnum<queue>)  [unwired: 2 in, 2 out]
                    }
                  }
                }
                n883 = Select(t=State_Type_Definitions,_for_0.26g_versions_and_later_3."True Stop" ("Enum"), s=w2664, f=State_Type_Definitions,_for_0.26g_versions_and_later_3."Task 8L: Return to position" ("Enum")) -> (s? t:f=w2669:T18)
              }
              frame "Exit" {
                n884 = for {
                  shift-right: [w2691] -> w2688
                  shift-left: w2685 -> [w2692]
                  tunnel: string[] ["STOP", "RESET ENCODERS", "RESET YAW", "ARDUINO MODE 0"] -> [w2690] mode=indexing
                  n885 = Enqueue Element(queue=w2692, element=w2690) -> (queue out=w2691:refnum<queue>)  [unwired: 2 in, 2 out]
                }
              }
            }
          }
          frame "Task 9A: Raise Arm" {
            # ">>> Motor control cluster >>>"
            # ">> Stepper height reeached >>"
            # ">>> yStepper command>>>"
            # ">> Manual override >>"
            n886 = Dequeue Element(queue=w2705, timeout in ms (-1)=w2700, error in (no error)=w2704) -> (element=w2707:T10)  [unwired: 3 out]
            n887 = Equal?(x=w2702, y=u8 50) -> (x = y?=w2693:bool)
            n888 = case shown="\"Start Task 1\", Default" w2707 {
              tunnel: [w2718 State_Type_Definitions,_for_0.26g_versions_and_later_3."True Stop" ("Enum")] -> w2698
              tunnel: [w2716 w2733] -> w2697
              tunnel: w2701 -> [w2715 _]
              tunnel: w2703 -> [w2709 _]
              tunnel: [State_Type_Definitions,_for_0.26g_versions_and_later_3."Idle" ("Enum") State_Type_Definitions,_for_0.26g_versions_and_later_3."Shutdown" ("Enum")] -> w2699
              tunnel: w2693 -> [w2708 _]
              frame "Start Task 1", Default {
                # ">> WIill proceed to part ii if not manual override >>"
                # ">>If ENABLE or Trigger is set to true>>"
                n889 = Or(x=w2708, y=w2709) -> (x .or. y?=w2710:bool)
                n890 = case shown="False" w2708 {
                  tunnel: [w2721 w2727] -> w2716
                  tunnel: w2715 -> [w2720 w2726]
                  frame False {
                    n891 = for {
                      shift-right: [w2723] -> w2721
                      shift-left: w2720 -> [w2724]
                      tunnel: string[] ["Z STEPPER BOX HEIGHT", "READ STEPPER VALUES"] ("element") -> [w2722] mode=indexing
                      n892 = Enqueue Element(queue=w2724, element=w2722) -> (queue out=w2723:refnum<queue>)  [unwired: 2 in, 2 out]
                    }
                  }
                  frame True {
                    n893 = for {
                      shift-right: [w2729] -> w2727
                      shift-left: w2726 -> [w2730]
                      tunnel: string[] ["READ NAVX", "RESET FLAGS", "RESET YAW", "", "", ""] -> [w2728] mode=indexing
                      n894 = Enqueue Element(queue=w2730, element=w2728) -> (queue out=w2729:refnum<queue>)  [unwired: 2 in, 2 out]
                    }
                  }
                }
                n895 = Select(t=State_Type_Definitions,_for_0.26g_versions_and_later_3."True Stop" ("Enum"), s=w2709, f=State_Type_Definitions,_for_0.26g_versions_and_later_3."Task 9B: Rotate to Angle" ("Enum")) -> (s? t:f=w2712:T18)
                n896 = Select(t=w2712, s=w2710, f=State_Type_Definitions,_for_0.26g_versions_and_later_3."Task 9A: Raise Arm" ("Enum")) -> (s? t:f=w2718:T18)
              }
              frame "Exit" {
                n897 = for {
                  shift-right: [w2736] -> w2733
                  shift-left: _ -> [w2737]
                  tunnel: string[] ["STOP", "RESET ENCODERS", "RESET YAW", ""] -> [w2735] mode=indexing
                  n898 = Enqueue Element(queue=w2737, element=w2735) -> (queue out=w2736:refnum<queue>)  [unwired: 2 in, 2 out]
                }
              }
            }
          }
          frame "Task 9B: Rotate to Angle" {
            # ">>> Motor control cluster >>>"
            # ">>> yStepper command>>>"
            n899 = Dequeue Element(queue=w2751, timeout in ms (-1)=w2750, error in (no error)=w2749) -> (element=w2753:T10)  [unwired: 3 out]
            n900 = In Range and Coerce(upper limit=65.0, x=w2743, lower limit=58.0) -> (In Range?=w2738:bool)  [unwired: 1 out]
            n901 = case shown="\"Start Task 1\", Default" w2753 {
              tunnel: w2744 -> [w2756 _]
              tunnel: [w2764 State_Type_Definitions,_for_0.26g_versions_and_later_3."True Stop" ("Enum")] -> w2746
              tunnel: w2752 -> [w2762 w2780]
              tunnel: [w2761 w2779] -> w2745
              tunnel: [State_Type_Definitions,_for_0.26g_versions_and_later_3."Idle" ("Enum") State_Type_Definitions,_for_0.26g_versions_and_later_3."Shutdown" ("Enum")] -> w2747
              tunnel: w2738 -> [w2754 _]
              frame "Start Task 1", Default {
                n902 = Or(x=w2754, y=w2756) -> (x .or. y?=w2755:bool)
                n903 = case shown="False" w2754 {
                  tunnel: w2762 -> [w2767 w2773]
                  tunnel: [w2766 w2771] -> w2761
                  frame False {
                    n904 = for {
                      shift-right: [w2769] -> w2766
                      shift-left: w2767 -> [w2770]
                      tunnel: string[] ["READ NAVX", "R-CW", ""] ("element") -> [w2768] mode=indexing
                      n905 = Enqueue Element(queue=w2770, element=w2768) -> (queue out=w2769:refnum<queue>)  [unwired: 2 in, 2 out]
                    }
                  }
                  frame True {
                    n906 = for {
                      shift-right: [w2775] -> w2771
                      shift-left: w2773 -> [w2776]
                      tunnel: string[] ["STOP", "RESET ENCODERS", "RESET YAW", "", ""] -> [w2774] mode=indexing
                      n907 = Enqueue Element(queue=w2776, element=w2774) -> (queue out=w2775:refnum<queue>)  [unwired: 2 in, 2 out]
                    }
                  }
                }
                n908 = Select(t=State_Type_Definitions,_for_0.26g_versions_and_later_3."True Stop" ("Enum"), s=w2756, f=State_Type_Definitions,_for_0.26g_versions_and_later_3."Task 9C: Detect Box") -> (s? t:f=w2758:T18)
                n909 = Select(t=w2758, s=w2755, f=State_Type_Definitions,_for_0.26g_versions_and_later_3."Task 9B: Rotate to Angle" ("Enum")) -> (s? t:f=w2764:T18)
              }
              frame "Exit" {
                n910 = for {
                  shift-right: [w2783] -> w2779
                  shift-left: w2780 -> [w2784]
                  tunnel: string[] ["STOP", "RESET ENCODERS", "RESET YAW", ""] -> [w2782] mode=indexing
                  n911 = Enqueue Element(queue=w2784, element=w2782) -> (queue out=w2783:refnum<queue>)  [unwired: 2 in, 2 out]
                }
              }
            }
          }
          frame "Task 9C: Detect Box" {
            # ">>> Motor control cluster >>>"
            # ">>Line Detected>>"
            # ">>Action Queue>>"
            # ">>> yStepper command>>>"
            n912 = Dequeue Element(queue=w2796, timeout in ms (-1)=w2795, error in (no error)=w2794) -> (element=w2797:T10)  [unwired: 3 out]
            n913 = case shown="\"Start Task 1\", Default" w2797 {
              tunnel: w2792 -> [w2798 _]
              tunnel: [w2808 State_Type_Definitions,_for_0.26g_versions_and_later_3."True Stop" ("Enum")] -> w2789
              tunnel: w2793 -> [w2806 w2824]
              tunnel: [w2805 w2823] -> w2788
              tunnel: [State_Type_Definitions,_for_0.26g_versions_and_later_3."Idle" ("Enum") State_Type_Definitions,_for_0.26g_versions_and_later_3."Shutdown" ("Enum")] -> w2791
              tunnel: w2785 -> [w2799 _]
              frame "Start Task 1", Default {
                n914 = Or(x=w2798, y=w2799) -> (x .or. y?=w2800:bool)
                n915 = case shown="False" w2799 {
                  tunnel: w2806 -> [w2811 w2817]
                  tunnel: [w2810 w2815] -> w2805
                  frame False {
                    n916 = for {
                      shift-right: [w2813] -> w2810
                      shift-left: w2811 -> [w2814]
                      tunnel: string[] ["READ IR", "READ LINE SENSOR", "FORWARD - IR ASSIST"] ("element") -> [w2812] mode=indexing
                      n917 = Enqueue Element(queue=w2814, element=w2812) -> (queue out=w2813:refnum<queue>)  [unwired: 2 in, 2 out]
                    }
                  }
                  frame True {
                    n918 = for {
                      shift-right: [w2819] -> w2815
                      shift-left: w2817 -> [w2820]
                      tunnel: string[] ["STOP", "RESET ENCODERS", "RESET YAW", "RESET FLAGS"] -> [w2818] mode=indexing
                      n919 = Enqueue Element(queue=w2820, element=w2818) -> (queue out=w2819:refnum<queue>)  [unwired: 2 in, 2 out]
                    }
                  }
                }
                n920 = Select(t=State_Type_Definitions,_for_0.26g_versions_and_later_3."True Stop" ("Enum"), s=w2798, f=State_Type_Definitions,_for_0.26g_versions_and_later_3."Task 9D: MOVE FORWARD") -> (s? t:f=w2802:T18)
                n921 = Select(t=w2802, s=w2800, f=State_Type_Definitions,_for_0.26g_versions_and_later_3."Task 9C: Detect Box" ("Enum")) -> (s? t:f=w2808:T18)
              }
              frame "Exit" {
                n922 = for {
                  shift-right: [w2827] -> w2823
                  shift-left: w2824 -> [w2828]
                  tunnel: string[] ["STOP", "RESET ENCODERS", "RESET YAW", ""] -> [w2826] mode=indexing
                  n923 = Enqueue Element(queue=w2828, element=w2826) -> (queue out=w2827:refnum<queue>)  [unwired: 2 in, 2 out]
                }
              }
            }
          }
          frame "Task 9D: MOVE FORWARD" {
            (unwired) 50.0 ("y")
            # "Use 20 low voltage\nUse 25 high voltage"
            # ">> Item Selection Bias >>"
            # ">> Wall detected >>"
            # ">> Manual override >>"
            # ">>Table Detected>>"
            # ">>> Motor control cluster >>>"
            # ">>Table or wall detectected>>"
            # ">>Action Queue>>"
            # ">>> yStepper command>>>"
            n924 = Dequeue Element(queue=w2846, timeout in ms (-1)=w2845, error in (no error)=w2844) -> (element=w2847:T10)  [unwired: 3 out]
            n925 = Less Or Equal?(x=w2835, y=25.0) -> (x <= y?=w2830:bool)
            n926 = Less?(x=w2833, y=20.0) -> (x < y?=w2831:bool)
            n927 = Or(x=w2830, y=w2831) -> (x .or. y?=w2829:bool)
            n928 = case shown="\"Start Task 1\", Default" w2847 {
              tunnel: w2842 -> [w2848 _]
              tunnel: [w2858 State_Type_Definitions,_for_0.26g_versions_and_later_3."True Stop" ("Enum")] -> w2839
              tunnel: w2843 -> [w2856 w2874]
              tunnel: [w2855 w2873] -> w2838
              tunnel: [State_Type_Definitions,_for_0.26g_versions_and_later_3."Idle" ("Enum") State_Type_Definitions,_for_0.26g_versions_and_later_3."Shutdown" ("Enum")] -> w2841
              tunnel: w2829 -> [w2849 _]
              frame "Start Task 1", Default {
                n929 = Or(x=w2848, y=w2849) -> (x .or. y?=w2850:bool)
                n930 = case shown="True" w2849 {
                  tunnel: w2856 -> [w2861 w2867]
                  tunnel: [w2860 w2865] -> w2855
                  frame False {
                    n931 = for {
                      shift-right: [w2863] -> w2860
                      shift-left: w2861 -> [w2864]
                      tunnel: string[] ["READ IR", "FORWARD - IR ASSIST", ""] ("element") -> [w2862] mode=indexing
                      n932 = Enqueue Element(queue=w2864, element=w2862) -> (queue out=w2863:refnum<queue>)  [unwired: 2 in, 2 out]
                    }
                  }
                  frame True {
                    n933 = for {
                      shift-right: [w2869] -> w2865
                      shift-left: w2867 -> [w2870]
                      tunnel: string[] ["STOP", "RESET ENCODERS", "RESET YAW", "RESET FLAGS"] -> [w2868] mode=indexing
                      n934 = Enqueue Element(queue=w2870, element=w2868) -> (queue out=w2869:refnum<queue>)  [unwired: 2 in, 2 out]
                    }
                  }
                }
                n935 = Select(t=State_Type_Definitions,_for_0.26g_versions_and_later_3."True Stop" ("Enum"), s=w2848, f=State_Type_Definitions,_for_0.26g_versions_and_later_3."Task 9E: MOVE LEFT") -> (s? t:f=w2852:T18)
                n936 = Select(t=w2852, s=w2850, f=State_Type_Definitions,_for_0.26g_versions_and_later_3."Task 9D: MOVE FORWARD" ("Enum")) -> (s? t:f=w2858:T18)
              }
              frame "Exit" {
                n937 = for {
                  shift-right: [w2877] -> w2873
                  shift-left: w2874 -> [w2878]
                  tunnel: string[] ["STOP", "RESET ENCODERS", "RESET YAW", ""] -> [w2876] mode=indexing
                  n938 = Enqueue Element(queue=w2878, element=w2876) -> (queue out=w2877:refnum<queue>)  [unwired: 2 in, 2 out]
                }
              }
            }
          }
          frame "Task 9E: MOVE LEFT" {
            # "High battery voltage: 15"
            # ">> Item Selection Bias >>"
            # ">>Stops if either table or wall is obstructing >>"
            n939 = Less?(x=w2879, y=15.0) -> (x < y?=w2889:bool)
            n940 = Dequeue Element(queue=w2887, timeout in ms (-1)=w2886, error in (no error)=w2885) -> (element=w2891:T10)  [unwired: 3 out]
            n941 = case shown="\"Start Task 1\", Default" w2891 {
              tunnel: w2889 -> [w2896 _]
              tunnel: [w2903 State_Type_Definitions,_for_0.26g_versions_and_later_3."True Stop" ("Enum")] -> w2881
              tunnel: w2884 -> [w2895 _]
              tunnel: w2888 -> [w2902 w2919]
              tunnel: [w2901 w2920] -> w2882
              tunnel: [State_Type_Definitions,_for_0.26g_versions_and_later_3."Idle" ("Enum") State_Type_Definitions,_for_0.26g_versions_and_later_3."Shutdown" ("Enum")] -> w2880
              frame "Start Task 1", Default {
                n942 = case shown="False" w2896 {
                  tunnel: w2902 -> [w2906 w2913]
                  tunnel: [w2907 w2912] -> w2901
                  frame False {
                    n943 = for {
                      tunnel: string[] ["LEFT", "READ NAVX", "READ IR", ""] ("element") -> [w2908] mode=indexing
                      shift-right: [w2910] -> w2907
                      shift-left: w2906 -> [w2909]
                      n944 = Enqueue Element(queue=w2909, element=w2908) -> (queue out=w2910:refnum<queue>)  [unwired: 2 in, 2 out]
                    }
                  }
                  frame True {
                    n945 = for {
                      shift-right: [w2915] -> w2912
                      shift-left: w2913 -> [w2916]
                      tunnel: string[] ["STOP", "RESET ENCODERS", "RESET FLAGS", "RESET YAW", "READ IR", ""] -> [w2914] mode=indexing
                      n946 = Enqueue Element(queue=w2916, element=w2914) -> (queue out=w2915:refnum<queue>)  [unwired: 2 in, 2 out]
                    }
                  }
                }
                n947 = Or(x=w2896, y=w2895) -> (x .or. y?=w2894:bool)
                n948 = Select(t=State_Type_Definitions,_for_0.26g_versions_and_later_3."True Stop" ("Enum"), s=w2895, f=State_Type_Definitions,_for_0.26g_versions_and_later_3."Task 9E2: MOVE RIGHT" ("Enum")) -> (s? t:f=w2897:T18)
                n949 = Select(t=w2897, s=w2894, f=State_Type_Definitions,_for_0.26g_versions_and_later_3."Task 9E: MOVE LEFT" ("Enum")) -> (s? t:f=w2903:T18)
              }
              frame "Exit" {
                n950 = for {
                  shift-right: [w2923] -> w2920
                  shift-left: w2919 -> [w2924]
                  tunnel: string[] ["STOP", "RESET ENCODERS", "RESET YAW", "ARDUINO MODE 0"] -> [w2922] mode=indexing
                  n951 = Enqueue Element(queue=w2924, element=w2922) -> (queue out=w2923:refnum<queue>)  [unwired: 2 in, 2 out]
                }
              }
            }
          }
          frame "Task 9E2: MOVE RIGHT" {
            # ">>> Motor control cluster >>>"
            # ">>> yStepper command>>>"
            n952 = Dequeue Element(queue=w2932, timeout in ms (-1)=w2931, error in (no error)=w2930) -> (element=w2937:T10)  [unwired: 3 out]
            n953 = case shown="\"Start Task 1\", Default" w2937 {
              tunnel: w2925 -> [w2940 _]
              tunnel: [w2947 State_Type_Definitions,_for_0.26g_versions_and_later_3."True Stop" ("Enum")] -> w2936
              tunnel: w2929 -> [w2939 _]
              tunnel: w2933 -> [w2946 w2963]
              tunnel: [w2945 w2964] -> w2935
              tunnel: [State_Type_Definitions,_for_0.26g_versions_and_later_3."Idle" ("Enum") State_Type_Definitions,_for_0.26g_versions_and_later_3."Shutdown" ("Enum")] -> w2934
              frame "Start Task 1", Default {
                n954 = case shown="True" w2940 {
                  tunnel: w2946 -> [w2950 w2957]
                  tunnel: [w2951 w2956] -> w2945
                  frame False {
                    n955 = for {
                      tunnel: string[] ["READ LINE SENSOR", "READ NAVX", "RIGHT", "READ ENCODERS"] ("element") -> [w2952] mode=indexing
                      shift-right: [w2954] -> w2951
                      shift-left: w2950 -> [w2953]
                      n956 = Enqueue Element(queue=w2953, element=w2952) -> (queue out=w2954:refnum<queue>)  [unwired: 2 in, 2 out]
                    }
                  }
                  frame True {
                    n957 = for {
                      shift-right: [w2959] -> w2956
                      shift-left: w2957 -> [w2960]
                      tunnel: string[] ["RESET ENCODERS", "RESET YAW", "RESET FLAGS", "STOP", "BOX COLOUR"] -> [w2958] mode=indexing
                      n958 = Enqueue Element(queue=w2960, element=w2958) -> (queue out=w2959:refnum<queue>)  [unwired: 2 in, 2 out]
                    }
                  }
                }
                n959 = Or(x=w2940, y=w2939) -> (x .or. y?=w2938:bool)
                n960 = Select(t=State_Type_Definitions,_for_0.26g_versions_and_later_3."True Stop" ("Enum"), s=w2939, f=State_Type_Definitions,_for_0.26g_versions_and_later_3."Task 9F: SCAN BOX" ("Enum")) -> (s? t:f=w2941:T18)
                n961 = Select(t=w2941, s=w2938, f=State_Type_Definitions,_for_0.26g_versions_and_later_3."Task 9E2: MOVE RIGHT" ("Enum")) -> (s? t:f=w2947:T18)
              }
              frame "Exit" {
                n962 = for {
                  shift-right: [w2967] -> w2964
                  shift-left: w2963 -> [w2968]
                  tunnel: string[] ["STOP", "RESET ENCODERS", "RESET YAW", "ARDUINO MODE 0"] -> [w2966] mode=indexing
                  n963 = Enqueue Element(queue=w2968, element=w2966) -> (queue out=w2967:refnum<queue>)  [unwired: 2 in, 2 out]
                }
              }
            }
          }
          frame "Task 9F: SCAN BOX" {
            # ">>> Motor control cluster >>>"
            # ">>Colour detection >>"
            # ">>> yStepper command>>>"
            # ">> Manual override >>"
            n964 = Dequeue Element(queue=w2985, timeout in ms (-1)=w2983, error in (no error)=w2984) -> (element=w2978:T10)  [unwired: 3 out]
            n965 = call "Box Colour FGV.vi"("Init/R/W State"=Box_Colour_FGV_States."Read") -> ("Colour to detect (output)"=w2971:T2)  [unwired: 9 in, 1 out]
            n966 = Equal?(x=w2972, y=w2971) -> (x = y?=w2970:bool)
            n967 = case shown="\"Start Task 1\", Default" w2978 {
              tunnel: [w2998 State_Type_Definitions,_for_0.26g_versions_and_later_3."True Stop" ("Enum")] -> w2975
              tunnel: [w2996 w3013] -> w2976
              tunnel: w2977 -> [w2995 _]
              tunnel: w2979 -> [w2988 _]
              tunnel: [State_Type_Definitions,_for_0.26g_versions_and_later_3."Idle" ("Enum") State_Type_Definitions,_for_0.26g_versions_and_later_3."Shutdown" ("Enum")] -> w2974
              tunnel: w2969 -> [w2989 _]
              tunnel: w2970 -> [w2987 _]
              frame "Start Task 1", Default {
                # ">> Will stop either due to manual override or is same box colour >>"
                # ">> WIill proceed to part ii if not manual override >>"
                # ">>If ENABLE or Trigger is set to true>>"
                n968 = Or(x=w2989, y=w2988) -> (x .or. y?=w2990:bool)
                n969 = case shown="True" w2989 {
                  tunnel: [w3001 w3007] -> w2996
                  tunnel: w2995 -> [w3000 w3006]
                  frame False {
                    n970 = for {
                      shift-right: [w3003] -> w3001
                      shift-left: w3000 -> [w3004]
                      tunnel: string[] ["", ""] ("element") -> [w3002] mode=indexing
                      n971 = Enqueue Element(queue=w3004, element=w3002) -> (queue out=w3003:refnum<queue>)  [unwired: 2 in, 2 out]
                    }
                  }
                  frame True {
                    n972 = for {
                      shift-right: [w3009] -> w3007
                      shift-left: w3006 -> [w3010]
                      tunnel: string[] ["RESET ENCODER", "RESET FLAGS", "RESET YAW", "", "", ""] -> [w3008] mode=indexing
                      n973 = Enqueue Element(queue=w3010, element=w3008) -> (queue out=w3009:refnum<queue>)  [unwired: 2 in, 2 out]
                    }
                  }
                }
                n974 = Or(x=w2988, y=w2987) -> (x .or. y?=w2986:bool)
                n975 = Select(t=State_Type_Definitions,_for_0.26g_versions_and_later_3."True Stop" ("Enum"), s=w2986, f=State_Type_Definitions,_for_0.26g_versions_and_later_3."Task 9G: MOVE RIGHT" ("Enum")) -> (s? t:f=w2992:T18)
                n976 = Select(t=w2992, s=w2990, f=State_Type_Definitions,_for_0.26g_versions_and_later_3."Task 9F: SCAN BOX" ("Enum")) -> (s? t:f=w2998:T18)
              }
              frame "Exit" {
                n977 = for {
                  shift-right: [w3016] -> w3013
                  shift-left: _ -> [w3017]
                  tunnel: string[] ["STOP", "RESET ENCODERS", "RESET YAW", ""] -> [w3015] mode=indexing
                  n978 = Enqueue Element(queue=w3017, element=w3015) -> (queue out=w3016:refnum<queue>)  [unwired: 2 in, 2 out]
                }
              }
            }
          }
          frame "Task 9G: MOVE RIGHT" {
            # ">>> Motor control cluster >>>"
            # ">>> yStepper command>>>"
            n979 = Dequeue Element(queue=w3029, timeout in ms (-1)=w3028, error in (no error)=w3027) -> (element=w3034:T10)  [unwired: 3 out]
            n980 = Greater?(x=w3019, y=50.0) -> (0:w3022:bool)
            n981 = And(x=w3020, y=w3022) -> (x .and. y?=w3018:bool)
            n982 = case shown="\"Start Task 1\", Default" w3034 {
              tunnel: w3018 -> [w3037 _]
              tunnel: [w3044 State_Type_Definitions,_for_0.26g_versions_and_later_3."True Stop" ("Enum")] -> w3033
              tunnel: w3026 -> [w3036 _]
              tunnel: w3030 -> [w3043 w3060]
              tunnel: [w3042 w3061] -> w3032
              tunnel: [State_Type_Definitions,_for_0.26g_versions_and_later_3."Idle" ("Enum") State_Type_Definitions,_for_0.26g_versions_and_later_3."Shutdown" ("Enum")] -> w3031
              frame "Start Task 1", Default {
                n983 = case shown="True" w3037 {
                  tunnel: w3043 -> [w3047 w3054]
                  tunnel: [w3048 w3053] -> w3042
                  frame False {
                    n984 = for {
                      tunnel: string[] ["READ LINE SENSOR", "READ NAVX", "RIGHT", "READ ENCODERS"] ("element") -> [w3049] mode=indexing
                      shift-right: [w3051] -> w3048
                      shift-left: w3047 -> [w3050]
                      n985 = Enqueue Element(queue=w3050, element=w3049) -> (queue out=w3051:refnum<queue>)  [unwired: 2 in, 2 out]
                    }
                  }
                  frame True {
                    n986 = for {
                      shift-right: [w3056] -> w3053
                      shift-left: w3054 -> [w3057]
                      tunnel: string[] ["RESET ENCODERS", "RESET YAW", "RESET FLAGS", "STOP", "BOX COLOUR"] -> [w3055] mode=indexing
                      n987 = Enqueue Element(queue=w3057, element=w3055) -> (queue out=w3056:refnum<queue>)  [unwired: 2 in, 2 out]
                    }
                  }
                }
                n988 = Or(x=w3037, y=w3036) -> (x .or. y?=w3035:bool)
                n989 = Select(t=State_Type_Definitions,_for_0.26g_versions_and_later_3."True Stop" ("Enum"), s=w3036, f=State_Type_Definitions,_for_0.26g_versions_and_later_3."Task 9H: SCAN BOX 2" ("Enum")) -> (s? t:f=w3038:T18)
                n990 = Select(t=w3038, s=w3035, f=State_Type_Definitions,_for_0.26g_versions_and_later_3."Task 9G: MOVE RIGHT" ("Enum")) -> (s? t:f=w3044:T18)
              }
              frame "Exit" {
                n991 = for {
                  shift-right: [w3064] -> w3061
                  shift-left: w3060 -> [w3065]
                  tunnel: string[] ["STOP", "RESET ENCODERS", "RESET YAW", "ARDUINO MODE 0"] -> [w3063] mode=indexing
                  n992 = Enqueue Element(queue=w3065, element=w3063) -> (queue out=w3064:refnum<queue>)  [unwired: 2 in, 2 out]
                }
              }
            }
          }
          frame "Task 9H: SCAN BOX 2" {
            # ">> Item Selection Bias >>"
            # ">>> Motor control cluster >>>"
            # ">>> yStepper command>>>"
            n993 = Dequeue Element(queue=w3075, timeout in ms (-1)=w3076, error in (no error)=w3077) -> (element=w3079:T10)  [unwired: 3 out]
            n994 = call "Box Colour FGV.vi"("Init/R/W State"=Box_Colour_FGV_States."Read") -> ("Colour to detect (output)"=w3069:T2)  [unwired: 9 in, 1 out]
            n995 = Equal?(x=w3068, y=w3069) -> (x = y?=w3067:bool)
            n996 = case shown="\"Start Task 1\", Default" w3079 {
              tunnel: w3066 -> [w3087 _]
              tunnel: [w3094 State_Type_Definitions,_for_0.26g_versions_and_later_3."True Stop" ("Enum")] -> w3072
              tunnel: w3078 -> [w3084 _]
              tunnel: w3074 -> [w3093 w3110]
              tunnel: [w3092 w3111] -> w3073
              tunnel: [State_Type_Definitions,_for_0.26g_versions_and_later_3."Idle" ("Enum") State_Type_Definitions,_for_0.26g_versions_and_later_3."Shutdown" ("Enum")] -> w3071
              tunnel: w3067 -> [w3085 _]
              frame "Start Task 1", Default {
                n997 = Or(x=w3087, y=w3084) -> (x .or. y?=w3086:bool)
                n998 = Or(x=w3085, y=w3084) -> (x .or. y?=w3083:bool)
                n999 = case shown="True" w3087 {
                  tunnel: w3093 -> [w3097 w3104]
                  tunnel: [w3098 w3103] -> w3092
                  frame False {
                    n1000 = for {
                      tunnel: string[] ["", "", "", ""] ("element") -> [w3099] mode=indexing
                      shift-right: [w3101] -> w3098
                      shift-left: w3097 -> [w3100]
                      n1001 = Enqueue Element(queue=w3100, element=w3099) -> (queue out=w3101:refnum<queue>)  [unwired: 2 in, 2 out]
                    }
                  }
                  frame True {
                    n1002 = for {
                      shift-right: [w3106] -> w3103
                      shift-left: w3104 -> [w3107]
                      tunnel: string[] ["READ NAVX", "RESET FLAGS", "RESET ENCODERS", "", "", ""] -> [w3105] mode=indexing
                      n1003 = Enqueue Element(queue=w3107, element=w3105) -> (queue out=w3106:refnum<queue>)  [unwired: 2 in, 2 out]
                    }
                  }
                }
                n1004 = Select(t=State_Type_Definitions,_for_0.26g_versions_and_later_3."True Stop" ("Enum"), s=w3083, f=State_Type_Definitions,_for_0.26g_versions_and_later_3."Task 9I: ROTATE 90 CW" ("Enum")) -> (s? t:f=w3088:T18)
                n1005 = Select(t=w3088, s=w3086, f=State_Type_Definitions,_for_0.26g_versions_and_later_3."Task 9H: SCAN BOX 2" ("Enum")) -> (s? t:f=w3094:T18)
              }
              frame "Exit" {
                n1006 = for {
                  shift-right: [w3114] -> w3111
                  shift-left: w3110 -> [w3115]
                  tunnel: string[] ["STOP", "RESET ENCODERS", "RESET YAW", "ARDUINO MODE 0"] -> [w3113] mode=indexing
                  n1007 = Enqueue Element(queue=w3115, element=w3113) -> (queue out=w3114:refnum<queue>)  [unwired: 2 in, 2 out]
                }
              }
            }
          }
          frame "Task 9I: ROTATE 90 CW" {
            # "High battery voltage: -36\nMid voltage: -38 \nLow voltage: -40"
            # ">> Item Selection Bias >>"
            n1008 = Less Or Equal?(x=w3118, y=-38.0) -> (x <= y?=w3116:bool)
            n1009 = Dequeue Element(queue=w3119, timeout in ms (-1)=w3120, error in (no error)=w3121) -> (element=w3127:T10)  [unwired: 3 out]
            n1010 = case shown="\"Start Task 1\", Default" w3127 {
              tunnel: w3116 -> [w3133 _]
              tunnel: [w3140 State_Type_Definitions,_for_0.26g_versions_and_later_3."True Stop" ("Enum")] -> w3124
              tunnel: w3122 -> [w3132 _]
              tunnel: w3126 -> [w3139 w3156]
              tunnel: [w3138 w3157] -> w3125
              tunnel: [State_Type_Definitions,_for_0.26g_versions_and_later_3."Idle" ("Enum") State_Type_Definitions,_for_0.26g_versions_and_later_3."Shutdown" ("Enum")] -> w3123
              frame "Start Task 1", Default {
                n1011 = case shown="False" w3133 {
                  tunnel: w3139 -> [w3143 w3150]
                  tunnel: [w3144 w3149] -> w3138
                  frame False {
                    n1012 = for {
                      tunnel: string[] ["R-CW", "READ ENCODERS", "READ IR", "READ NAVX"] ("element") -> [w3145] mode=indexing
                      shift-right: [w3147] -> w3144
                      shift-left: w3143 -> [w3146]
                      n1013 = Enqueue Element(queue=w3146, element=w3145) -> (queue out=w3147:refnum<queue>)  [unwired: 2 in, 2 out]
                    }
                  }
                  frame True {
                    n1014 = for {
                      shift-right: [w3152] -> w3149
                      shift-left: w3150 -> [w3153]
                      tunnel: string[] ["STOP", "RESET ENCODERS", "RESET YAW", "RESET FLAGS", "READ IR", ""] -> [w3151] mode=indexing
                      n1015 = Enqueue Element(queue=w3153, element=w3151) -> (queue out=w3152:refnum<queue>)  [unwired: 2 in, 2 out]
                    }
                  }
                }
                n1016 = Or(x=w3133, y=w3132) -> (x .or. y?=w3131:bool)
                n1017 = Select(t=State_Type_Definitions,_for_0.26g_versions_and_later_3."True Stop" ("Enum"), s=w3132, f=State_Type_Definitions,_for_0.26g_versions_and_later_3."Task 9J: FORWARD" ("Enum")) -> (s? t:f=w3134:T18)
                n1018 = Select(t=w3134, s=w3131, f=State_Type_Definitions,_for_0.26g_versions_and_later_3."Task 9I: ROTATE 90 CW" ("Enum")) -> (s? t:f=w3140:T18)
              }
              frame "Exit" {
                n1019 = for {
                  shift-right: [w3160] -> w3157
                  shift-left: w3156 -> [w3161]
                  tunnel: string[] ["STOP", "RESET ENCODERS", "RESET YAW", "ARDUINO MODE 0"] -> [w3159] mode=indexing
                  n1020 = Enqueue Element(queue=w3161, element=w3159) -> (queue out=w3160:refnum<queue>)  [unwired: 2 in, 2 out]
                }
              }
            }
          }
          frame "Task 9J: FORWARD" {
            # "Tried values: 70, 150"
            # ">>Stops if either table or wall is obstructing >>"
            # ">> Item Selection Bias >>"
            n1021 = Less?(x=w3164, y=150.0) -> (x < y?=w3167:bool)
            n1022 = Greater Than 0?(x=w3164) -> (x > 0?=w3166:bool)
            n1023 = Less Or Equal?(x=w3170, y=20.0) -> (x <= y?=w3168:bool)
            n1024 = Greater Than 0?(x=w3170) -> (x > 0?=w3169:bool)
            n1025 = And(x=w3166, y=w3167) -> ()  [unwired: 1 out]
            n1026 = Dequeue Element(queue=w3176, timeout in ms (-1)=w3177, error in (no error)=w3178) -> (element=w3180:T10)  [unwired: 3 out]
            n1027 = And(x=w3169, y=w3168) -> (x .and. y?=w3162:bool)
            n1028 = Or(x=w3162, y=w3162) -> (x .or. y?=w3163:bool)
            n1029 = case shown="\"Start Task 1\", Default" w3180 {
              tunnel: w3163 -> [w3186 _]
              tunnel: [w3193 State_Type_Definitions,_for_0.26g_versions_and_later_3."True Stop" ("Enum")] -> w3174
              tunnel: w3179 -> [w3185 _]
              tunnel: w3175 -> [w3192 w3209]
              tunnel: [w3191 w3210] -> w3173
              tunnel: [State_Type_Definitions,_for_0.26g_versions_and_later_3."Idle" ("Enum") State_Type_Definitions,_for_0.26g_versions_and_later_3."Shutdown" ("Enum")] -> w3172
              frame "Start Task 1", Default {
                n1030 = case shown="True" w3186 {
                  tunnel: w3192 -> [w3196 w3203]
                  tunnel: [w3197 w3202] -> w3191
                  frame False {
                    n1031 = for {
                      tunnel: string[] ["READ IR", "READ NAVX", "FORWARD"] ("element") -> [w3198] mode=indexing
                      shift-right: [w3200] -> w3197
                      shift-left: w3196 -> [w3199]
                      n1032 = Enqueue Element(queue=w3199, element=w3198) -> (queue out=w3200:refnum<queue>)  [unwired: 2 in, 2 out]
                    }
                  }
                  frame True {
                    n1033 = for {
                      shift-right: [w3205] -> w3202
                      shift-left: w3203 -> [w3206]
                      tunnel: string[] ["STOP", "RESET ENCODERS", "RESET YAW", "RESET FLAGS", "READ IR", ""] -> [w3204] mode=indexing
                      n1034 = Enqueue Element(queue=w3206, element=w3204) -> (queue out=w3205:refnum<queue>)  [unwired: 2 in, 2 out]
                    }
                  }
                }
                n1035 = Or(x=w3186, y=w3185) -> (x .or. y?=w3184:bool)
                n1036 = Select(t=State_Type_Definitions,_for_0.26g_versions_and_later_3."True Stop" ("Enum"), s=w3185, f=State_Type_Definitions,_for_0.26g_versions_and_later_3."Task 9K: RAM WALL" ("Enum")) -> (s? t:f=w3187:T18)
                n1037 = Select(t=w3187, s=w3184, f=State_Type_Definitions,_for_0.26g_versions_and_later_3."Task 9J: FORWARD" ("Enum")) -> (s? t:f=w3193:T18)
              }
              frame "Exit" {
                n1038 = for {
                  shift-right: [w3213] -> w3210
                  shift-left: w3209 -> [w3214]
                  tunnel: string[] ["STOP", "RESET ENCODERS", "RESET YAW", "ARDUINO MODE 0"] -> [w3212] mode=indexing
                  n1039 = Enqueue Element(queue=w3214, element=w3212) -> (queue out=w3213:refnum<queue>)  [unwired: 2 in, 2 out]
                }
              }
            }
          }
          frame "Task 9K: RAM WALL" {
            # "High battery voltage: 15"
            # ">> Item Selection Bias >>"
            # ">>Stops if either table or wall is obstructing >>"
            n1040 = Less?(x=w3215, y=15.0) -> (x < y?=w3225:bool)
            n1041 = Dequeue Element(queue=w3223, timeout in ms (-1)=w3222, error in (no error)=w3221) -> (element=w3227:T10)  [unwired: 3 out]
            n1042 = case shown="\"Start Task 1\", Default" w3227 {
              tunnel: w3225 -> [w3232 _]
              tunnel: [w3239 State_Type_Definitions,_for_0.26g_versions_and_later_3."True Stop" ("Enum")] -> w3217
              tunnel: w3220 -> [w3231 _]
              tunnel: w3224 -> [w3238 w3255]
              tunnel: [w3237 w3256] -> w3218
              tunnel: [State_Type_Definitions,_for_0.26g_versions_and_later_3."Idle" ("Enum") State_Type_Definitions,_for_0.26g_versions_and_later_3."Shutdown" ("Enum")] -> w3216
              frame "Start Task 1", Default {
                n1043 = case shown="True" w3232 {
                  tunnel: w3238 -> [w3242 w3249]
                  tunnel: [w3243 w3248] -> w3237
                  frame False {
                    n1044 = for {
                      tunnel: string[] ["LEFT", "READ NAVX", "READ IR", ""] ("element") -> [w3244] mode=indexing
                      shift-right: [w3246] -> w3243
                      shift-left: w3242 -> [w3245]
                      n1045 = Enqueue Element(queue=w3245, element=w3244) -> (queue out=w3246:refnum<queue>)  [unwired: 2 in, 2 out]
                    }
                  }
                  frame True {
                    n1046 = for {
                      shift-right: [w3251] -> w3248
                      shift-left: w3249 -> [w3252]
                      tunnel: string[] ["STOP", "RESET ENCODERS", "RESET FLAGS", "RESET YAW", "READ IR", ""] -> [w3250] mode=indexing
                      n1047 = Enqueue Element(queue=w3252, element=w3250) -> (queue out=w3251:refnum<queue>)  [unwired: 2 in, 2 out]
                    }
                  }
                }
                n1048 = Or(x=w3232, y=w3231) -> (x .or. y?=w3230:bool)
                n1049 = Select(t=State_Type_Definitions,_for_0.26g_versions_and_later_3."True Stop" ("Enum"), s=w3231, f=State_Type_Definitions,_for_0.26g_versions_and_later_3."Task 9L: MOVE RIGHT" ("Enum")) -> (s? t:f=w3233:T18)
                n1050 = Select(t=w3233, s=w3230, f=State_Type_Definitions,_for_0.26g_versions_and_later_3."Task 9K: RAM WALL" ("Enum")) -> (s? t:f=w3239:T18)
              }
              frame "Exit" {
                n1051 = for {
                  shift-right: [w3259] -> w3256
                  shift-left: w3255 -> [w3260]
                  tunnel: string[] ["STOP", "RESET ENCODERS", "RESET YAW", "ARDUINO MODE 0"] -> [w3258] mode=indexing
                  n1052 = Enqueue Element(queue=w3260, element=w3258) -> (queue out=w3259:refnum<queue>)  [unwired: 2 in, 2 out]
                }
              }
            }
          }
          frame "Task 9L: MOVE RIGHT" {
            # "High battery voltage: 15"
            # ">>> Motor control cluster >>>"
            # ">>> yStepper command>>>"
            # ">> Item Selection Bias >>"
            n1053 = Dequeue Element(queue=w3268, timeout in ms (-1)=w3267, error in (no error)=w3266) -> (element=w3270:T10)  [unwired: 3 out]
            n1054 = case shown="\"Start Task 1\", Default" w3270 {
              tunnel: w3261 -> [w3276 _]
              tunnel: [w3283 State_Type_Definitions,_for_0.26g_versions_and_later_3."True Stop" ("Enum")] -> w3264
              tunnel: w3265 -> [w3275 _]
              tunnel: w3269 -> [w3282 w3299]
              tunnel: [w3281 w3300] -> w3262
              tunnel: [State_Type_Definitions,_for_0.26g_versions_and_later_3."Idle" ("Enum") State_Type_Definitions,_for_0.26g_versions_and_later_3."Shutdown" ("Enum")] -> w3263
              frame "Start Task 1", Default {
                n1055 = case shown="True" w3276 {
                  tunnel: w3282 -> [w3286 w3293]
                  tunnel: [w3287 w3292] -> w3281
                  frame False {
                    n1056 = for {
                      tunnel: string[] ["RIGHT", "READ NAVX", "READ LINE SENSOR", ""] ("element") -> [w3288] mode=indexing
                      shift-right: [w3290] -> w3287
                      shift-left: w3286 -> [w3289]
                      n1057 = Enqueue Element(queue=w3289, element=w3288) -> (queue out=w3290:refnum<queue>)  [unwired: 2 in, 2 out]
                    }
                  }
                  frame True {
                    n1058 = for {
                      shift-right: [w3295] -> w3292
                      shift-left: w3293 -> [w3296]
                      tunnel: string[] ["STOP", "RESET ENCODERS", "RESET FLAGS", "RESET YAW", "BOX COLOUR", ""] -> [w3294] mode=indexing
                      n1059 = Enqueue Element(queue=w3296, element=w3294) -> (queue out=w3295:refnum<queue>)  [unwired: 2 in, 2 out]
                    }
                  }
                }
                n1060 = Or(x=w3276, y=w3275) -> (x .or. y?=w3274:bool)
                n1061 = Select(t=State_Type_Definitions,_for_0.26g_versions_and_later_3."True Stop" ("Enum"), s=w3275, f=State_Type_Definitions,_for_0.26g_versions_and_later_3."Task 9M: SCAN BOX 3" ("Enum")) -> (s? t:f=w3277:T18)
                n1062 = Select(t=w3277, s=w3274, f=State_Type_Definitions,_for_0.26g_versions_and_later_3."Task 9L: MOVE RIGHT" ("Enum")) -> (s? t:f=w3283:T18)
              }
              frame "Exit" {
                n1063 = for {
                  shift-right: [w3303] -> w3300
                  shift-left: w3299 -> [w3304]
                  tunnel: string[] ["STOP", "RESET ENCODERS", "RESET YAW", "ARDUINO MODE 0"] -> [w3302] mode=indexing
                  n1064 = Enqueue Element(queue=w3304, element=w3302) -> (queue out=w3303:refnum<queue>)  [unwired: 2 in, 2 out]
                }
              }
            }
          }
          frame "Task 9M: SCAN BOX 3" {
            # ">>> Motor control cluster >>>"
            # ">>> yStepper command>>>"
            # ">> Item Selection Bias >>"
            n1065 = Dequeue Element(queue=w3314, timeout in ms (-1)=w3313, error in (no error)=w3312) -> (element=w3318:T10)  [unwired: 3 out]
            n1066 = call "Box Colour FGV.vi"("Init/R/W State"=Box_Colour_FGV_States."Read") -> ("Colour to detect (output)"=w3308:T2)  [unwired: 9 in, 1 out]
            n1067 = Equal?(x=w3307, y=w3308) -> (x = y?=w3306:bool)
            n1068 = case shown="\"Start Task 1\", Default" w3318 {
              tunnel: w3305 -> [w3326 _]
              tunnel: [w3333 State_Type_Definitions,_for_0.26g_versions_and_later_3."True Stop" ("Enum")] -> w3316
              tunnel: w3311 -> [w3322 _]
              tunnel: w3315 -> [w3332 w3349]
              tunnel: [w3331 w3350] -> w3310
              tunnel: [State_Type_Definitions,_for_0.26g_versions_and_later_3."Idle" ("Enum") State_Type_Definitions,_for_0.26g_versions_and_later_3."Shutdown" ("Enum")] -> w3317
              tunnel: w3306 -> [w3324 _]
              frame "Start Task 1", Default {
                n1069 = case shown="True" w3326 {
                  tunnel: w3332 -> [w3336 w3343]
                  tunnel: [w3337 w3342] -> w3331
                  frame False {
                    n1070 = for {
                      tunnel: string[] ["", "", "", ""] ("element") -> [w3338] mode=indexing
                      shift-right: [w3340] -> w3337
                      shift-left: w3336 -> [w3339]
                      n1071 = Enqueue Element(queue=w3339, element=w3338) -> (queue out=w3340:refnum<queue>)  [unwired: 2 in, 2 out]
                    }
                  }
                  frame True {
                    n1072 = for {
                      shift-right: [w3345] -> w3342
                      shift-left: w3343 -> [w3346]
                      tunnel: string[] ["STOP", "RESET ENCODERS", "RESET FLAGS", "RESET YAW", "", ""] -> [w3344] mode=indexing
                      n1073 = Enqueue Element(queue=w3346, element=w3344) -> (queue out=w3345:refnum<queue>)  [unwired: 2 in, 2 out]
                    }
                  }
                }
                n1074 = Or(x=w3326, y=w3322) -> (x .or. y?=w3325:bool)
                n1075 = Or(x=w3324, y=w3322) -> (x .or. y?=w3323:bool)
                n1076 = Select(t=State_Type_Definitions,_for_0.26g_versions_and_later_3."True Stop" ("Enum"), s=w3323, f=State_Type_Definitions,_for_0.26g_versions_and_later_3."Task 9N: MOVE RIGHT" ("Enum")) -> (s? t:f=w3327:T18)
                n1077 = Select(t=w3327, s=w3325, f=State_Type_Definitions,_for_0.26g_versions_and_later_3."Task 9M: SCAN BOX 3" ("Enum")) -> (s? t:f=w3333:T18)
              }
              frame "Exit" {
                n1078 = for {
                  shift-right: [w3353] -> w3350
                  shift-left: w3349 -> [w3354]
                  tunnel: string[] ["STOP", "RESET ENCODERS", "RESET YAW", "ARDUINO MODE 0"] -> [w3352] mode=indexing
                  n1079 = Enqueue Element(queue=w3354, element=w3352) -> (queue out=w3353:refnum<queue>)  [unwired: 2 in, 2 out]
                }
              }
            }
          }
          frame "Task 9N: MOVE RIGHT" {
            # ">> Item Selection Bias >>"
            n1080 = Dequeue Element(queue=w3359, timeout in ms (-1)=w3358, error in (no error)=w3357) -> (element=w3364:T10)  [unwired: 3 out]
            n1081 = case shown="\"Start Task 1\", Default" w3364 {
              tunnel: w3355 -> [w3370 _]
              tunnel: [w3377 State_Type_Definitions,_for_0.26g_versions_and_later_3."True Stop" ("Enum")] -> w3362
              tunnel: w3356 -> [w3369 _]
              tunnel: w3360 -> [w3376 w3393]
              tunnel: [w3375 w3394] -> w3361
              tunnel: [State_Type_Definitions,_for_0.26g_versions_and_later_3."Idle" ("Enum") State_Type_Definitions,_for_0.26g_versions_and_later_3."Shutdown" ("Enum")] -> w3363
              frame "Start Task 1", Default {
                n1082 = case shown="True" w3370 {
                  tunnel: w3376 -> [w3380 w3387]
                  tunnel: [w3381 w3386] -> w3375
                  frame False {
                    n1083 = for {
                      tunnel: string[] ["READ LINE SENSOR", "READ NAVX", "RIGHT", "READ ENCODERS"] ("element") -> [w3382] mode=indexing
                      shift-right: [w3384] -> w3381
                      shift-left: w3380 -> [w3383]
                      n1084 = Enqueue Element(queue=w3383, element=w3382) -> (queue out=w3384:refnum<queue>)  [unwired: 2 in, 2 out]
                    }
                  }
                  frame True {
                    n1085 = for {
                      shift-right: [w3389] -> w3386
                      shift-left: w3387 -> [w3390]
                      tunnel: string[] ["STOP", "RESET ENCODERS", "RESET YAW", "RESET FLAGS", "BOX COLOUR", ""] -> [w3388] mode=indexing
                      n1086 = Enqueue Element(queue=w3390, element=w3388) -> (queue out=w3389:refnum<queue>)  [unwired: 2 in, 2 out]
                    }
                  }
                }
                n1087 = Or(x=w3370, y=w3369) -> (x .or. y?=w3368:bool)
                n1088 = Select(t=State_Type_Definitions,_for_0.26g_versions_and_later_3."True Stop" ("Enum"), s=w3369, f=State_Type_Definitions,_for_0.26g_versions_and_later_3."Task 9O: SCAN BOX 4" ("Enum")) -> (s? t:f=w3371:T18)
                n1089 = Select(t=w3371, s=w3368, f=State_Type_Definitions,_for_0.26g_versions_and_later_3."Task 9N: MOVE RIGHT" ("Enum")) -> (s? t:f=w3377:T18)
              }
              frame "Exit" {
                n1090 = for {
                  shift-right: [w3397] -> w3394
                  shift-left: w3393 -> [w3398]
                  tunnel: string[] ["STOP", "RESET ENCODERS", "RESET YAW", "ARDUINO MODE 0"] -> [w3396] mode=indexing
                  n1091 = Enqueue Element(queue=w3398, element=w3396) -> (queue out=w3397:refnum<queue>)  [unwired: 2 in, 2 out]
                }
              }
            }
          }
          frame "Task 9O: SCAN BOX 4" {
            # ">>> Motor control cluster >>>"
            # ">>> yStepper command>>>"
            # ">> Item Selection Bias >>"
            n1092 = Dequeue Element(queue=w3409, timeout in ms (-1)=w3408, error in (no error)=w3407) -> (element=w3413:T10)  [unwired: 3 out]
            n1093 = call "Box Colour FGV.vi"("Init/R/W State"=Box_Colour_FGV_States."Read") -> ("Colour to detect (output)"=w3411:T2)  [unwired: 9 in, 1 out]
            n1094 = Equal?(x=w3401, y=w3411) -> (x = y?=w3410:bool)
            n1095 = case shown="\"Start Task 1\", Default" w3413 {
              tunnel: w3399 -> [w3420 _]
              tunnel: [w3427 State_Type_Definitions,_for_0.26g_versions_and_later_3."True Stop" ("Enum")] -> w3403
              tunnel: w3406 -> [w3416 _]
              tunnel: w3400 -> [w3426 w3443]
              tunnel: [w3425 w3444] -> w3404
              tunnel: [State_Type_Definitions,_for_0.26g_versions_and_later_3."Idle" ("Enum") State_Type_Definitions,_for_0.26g_versions_and_later_3."Shutdown" ("Enum")] -> w3402
              tunnel: w3410 -> [w3418 _]
              frame "Start Task 1", Default {
                n1096 = case shown="True" w3420 {
                  tunnel: w3426 -> [w3430 w3437]
                  tunnel: [w3431 w3436] -> w3425
                  frame False {
                    n1097 = for {
                      tunnel: string[] ["", "", "", ""] ("element") -> [w3432] mode=indexing
                      shift-right: [w3434] -> w3431
                      shift-left: w3430 -> [w3433]
                      n1098 = Enqueue Element(queue=w3433, element=w3432) -> (queue out=w3434:refnum<queue>)  [unwired: 2 in, 2 out]
                    }
                  }
                  frame True {
                    n1099 = for {
                      shift-right: [w3439] -> w3436
                      shift-left: w3437 -> [w3440]
                      tunnel: string[] ["STOP", "RESET ENCODERS", "RESET FLAGS", "RESET YAW", "", ""] -> [w3438] mode=indexing
                      n1100 = Enqueue Element(queue=w3440, element=w3438) -> (queue out=w3439:refnum<queue>)  [unwired: 2 in, 2 out]
                    }
                  }
                }
                n1101 = Or(x=w3420, y=w3416) -> (x .or. y?=w3419:bool)
                n1102 = Or(x=w3418, y=w3416) -> (x .or. y?=w3417:bool)
                n1103 = Select(t=State_Type_Definitions,_for_0.26g_versions_and_later_3."True Stop" ("Enum"), s=w3417, f=State_Type_Definitions,_for_0.26g_versions_and_later_3."True Stop" ("Enum")) -> (s? t:f=w3421:T18)
                n1104 = Select(t=w3421, s=w3419, f=State_Type_Definitions,_for_0.26g_versions_and_later_3."Task 9O: SCAN BOX 4" ("Enum")) -> (s? t:f=w3427:T18)
              }
              frame "Exit" {
                n1105 = for {
                  shift-right: [w3447] -> w3444
                  shift-left: w3443 -> [w3448]
                  tunnel: string[] ["STOP", "RESET ENCODERS", "RESET YAW", "ARDUINO MODE 0"] -> [w3446] mode=indexing
                  n1106 = Enqueue Element(queue=w3448, element=w3446) -> (queue out=w3447:refnum<queue>)  [unwired: 2 in, 2 out]
                }
              }
            }
          }
          frame "Task A1: RAISE ARM" {
            # ">>> Motor control cluster >>>"
            # ">>> yStepper command>>>"
            n1107 = Dequeue Element(queue=w3460, timeout in ms (-1)=w3459, error in (no error)=w3458) -> (element=w3465:T10)  [unwired: 3 out]
            n1108 = Greater?(x=w3450, y=50.0) -> (0:w3453:bool)
            n1109 = And(x=w3451, y=w3453) -> (x .and. y?=w3449:bool)
            n1110 = case shown="\"Start Task 1\", Default" w3465 {
              tunnel: w3449 -> [w3468 _]
              tunnel: [w3475 State_Type_Definitions,_for_0.26g_versions_and_later_3."True Stop" ("Enum")] -> w3464
              tunnel: w3457 -> [w3467 _]
              tunnel: w3461 -> [w3474 w3491]
              tunnel: [w3473 w3492] -> w3463
              tunnel: [State_Type_Definitions,_for_0.26g_versions_and_later_3."Idle" ("Enum") State_Type_Definitions,_for_0.26g_versions_and_later_3."Shutdown" ("Enum")] -> w3462
              frame "Start Task 1", Default {
                n1111 = case shown="True" w3468 {
                  tunnel: w3474 -> [w3478 w3485]
                  tunnel: [w3479 w3484] -> w3473
                  frame False {
                    n1112 = for {
                      tunnel: string[] ["READ LINE SENSOR", "READ NAVX", "RIGHT", "READ ENCODERS"] ("element") -> [w3480] mode=indexing
                      shift-right: [w3482] -> w3479
                      shift-left: w3478 -> [w3481]
                      n1113 = Enqueue Element(queue=w3481, element=w3480) -> (queue out=w3482:refnum<queue>)  [unwired: 2 in, 2 out]
                    }
                  }
                  frame True {
                    n1114 = for {
                      shift-right: [w3487] -> w3484
                      shift-left: w3485 -> [w3488]
                      tunnel: string[] ["RESET ENCODERS", "RESET YAW", "RESET FLAGS", "STOP", "BOX COLOUR"] -> [w3486] mode=indexing
                      n1115 = Enqueue Element(queue=w3488, element=w3486) -> (queue out=w3487:refnum<queue>)  [unwired: 2 in, 2 out]
                    }
                  }
                }
                n1116 = Or(x=w3468, y=w3467) -> (x .or. y?=w3466:bool)
                n1117 = Select(t=State_Type_Definitions,_for_0.26g_versions_and_later_3."True Stop" ("Enum"), s=w3467, f=State_Type_Definitions,_for_0.26g_versions_and_later_3."Task 9H: SCAN BOX 2" ("Enum")) -> (s? t:f=w3469:T18)
                n1118 = Select(t=w3469, s=w3466, f=State_Type_Definitions,_for_0.26g_versions_and_later_3."Task 9G: MOVE RIGHT" ("Enum")) -> (s? t:f=w3475:T18)
              }
              frame "Exit" {
                n1119 = for {
                  shift-right: [w3495] -> w3492
                  shift-left: w3491 -> [w3496]
                  tunnel: string[] ["STOP", "RESET ENCODERS", "RESET YAW", "ARDUINO MODE 0"] -> [w3494] mode=indexing
                  n1120 = Enqueue Element(queue=w3496, element=w3494) -> (queue out=w3495:refnum<queue>)  [unwired: 2 in, 2 out]
                }
              }
            }
          }
          frame "Task A2: ROTATE TO ANGLE" {
          }
          frame "Task A3: MOVE TO BL BOX" {
          }
          frame "Task A4: MOVE FORWARD" {
          }
          frame "Task A5: ROTATE CW 90" {
          }
        }
        "Object Detection" <- w335
        "Ultrasonic sensors" <- w358
        "Encoder values" <- w347
        "Stepper position values" <- w331
        "NAVX Values" <- w329
        "IR Sensors" <- w321
        "Line sensors" <- w316
        "Time cluster" <- w327
        "Box Colour Detection" <- w309
      }
    }
    "Object recognition mode" <- w234
    "Front Ultrasonic obstruct" <- w231
    "Front IR obstruct" <- w230
    "Table IR obstruct" <- w229
    "Same colour?" <- w224
    n1121 = local write "Green LED"(w244) -> ()
  }
  n1122 = while {
    tunnel: w49 -> [w4436]
    tunnel: w48 -> [w4433]
    stop <- w4430 stop-if-true
    # "Status Loop for Action Queues"
    n1123 = Get Queue Status(queue=w4436, return elements? (F)=TRUE) -> (error out=w4432:errorcluster, # elements in queue=→"Action Queue Items":i32, elements=→"Action Queues items":string[])  [unwired: 1 in, 5 out]
    n1124 = Get Queue Status(queue=w4433, return elements? (F)=TRUE) -> (# pending remove=→"State Logic Queue Items":i32, error out=w4431:errorcluster, elements=→"elements":T10[])  [unwired: 1 in, 5 out]
    n1125 = Merge Errors(w4432, w4431) -> (w4430:errorcluster)
    n1126 = Wait (ms)(milliseconds to wait=u32 500) -> ()  [unwired: 1 out]
  }
  n1127 = while {
    stop <- w4440 stop-if-true
    n1128 = call "MOTOR CONTROL WITH PID AE.vi"("AE Mode"=MOTOR_CONTROL_WITH_PID_AE_DATA_MODE_TYPE_DEF."Read from AE") -> ("Speed & distance"=→"Speed & distance":T15)  [unwired: 3 in]
    n1129 = call "FGV Stop.vi"("Init/Read/Write State"=States_for_Action_Engine."Read") -> ("Output node"=w4440:bool)  [unwired: 2 in, 1 out]
    n1130 = Wait (ms)(milliseconds to wait=u32 5) -> ()  [unwired: 1 out]
  }
  n1131 = call <vilib>:"DIO Close.vi"("error in (no error)"=w25, "DIO Info In"=w28) -> ()  [unwired: 9 in, 1 out]
  n1132 = call <vilib>:"DIO Close.vi"("error in (no error)"=w35, "DIO Info In"=w37) -> ()  [unwired: 9 in, 1 out]
  n1133 = call <vilib>:"NavX Close.vi"("error in (no error)"=w12, "NavX Info In"=w11) -> ()  [unwired: 9 in, 1 out]
  n1134 = call <vilib>:"DIO Close.vi"("error in (no error)"=w30, "DIO Info In"=w32) -> ()  [unwired: 9 in, 1 out]
  n1135 = call <vilib>:"DIO Close.vi"("error in (no error)"=w19, "DIO Info In"=w20) -> ()  [unwired: 9 in, 1 out]
  n1136 = call <vilib>:"DIO Close.vi"("error in (no error)"=w14, "DIO Info In"=w15) -> ()  [unwired: 9 in, 1 out]
  n1137 = Merge Errors "Merge Errors"(w65, w64) -> (w47:errorcluster)
  n1138 = Merge Errors(w51, w47) -> (w46:errorcluster)
  n1139 = Destroy User Event(user event=w69, error in=w46) -> ()  [unwired: 1 out]
  n1140 = Release Queue(queue=w42, error in (no error)=w46) -> (error out=→"Queue Errors":errorcluster)  [unwired: 1 in, 2 out]
  n1141 = Release Queue(queue=w59, error in (no error)=w46) -> ()  [unwired: 1 in, 3 out]
  n1142 = Destroy User Event(user event=w68, error in=w46) -> ()  [unwired: 1 out]
  n1143 = Unregister For Events(event registration refnum=w60, error in=w46) -> ()  [unwired: 1 out]
